vi "Actor Core.vi"(8 "error in":errorcluster, 11 "Inspection Statemachine in":refnum<class "Inspection Statemachine.lvclass">) -> (0 "error out":errorcluster, 3 "Actor out":refnum<class "Actor.lvclass">)   [LabVIEW 2019, in "Inspection Statemachine.lvclass"]
doc: "(<B>Filename</B>: Actor Framework.lvlib:Actor.lvclass:Actor Core.vi)\n\nReceives messages to the actor, reacts to them, and initiates any error handling that may shut the actor down.\n\nDescendant classes may override this VI to append parallel tasks for the actor to complete while it handles messages. Overrides use the Call Parent Method node."
uses:
  Inspection Statemachine.lvclass
  Machine Interface/Machine Interface.lvclass
  <vilib>/ActorFramework/Actor/Actor.lvclass
  Rack Controller/Rack Controller.lvclass
  Inspection Statemachine Messages/ErrorMessage_SM Msg/ErrorMessage_SM Msg.lvclass
  <vilib>/vision/Image Controls.llb/IMAQ Image.ctl
  Inspection Statemachine Messages/ButtonPressed_SM Msg/ButtonPressed_SM Msg.lvclass
  DataLogger/DataLogger/DataLogger.lvclass
  Controls/Result Cluster_SM.ctl
  <vilib>/ActorFramework/Stop Msg/Stop Msg.lvclass
  Common/Controls/Pop-up Input.ctl
  Controls/Output Cluster_SM.ctl
  Common/Controls/Camera Optics Diagnostics Result.ctl
  Common/Controls/AllPartInfo.ctl
  User Interface/User Interface Actor/ZenGage v3.0 UI.lvclass
  Controls/LocalData_SM.ctl
  ZenAnalytics/Zen Analytics/Zen Analytics.lvclass
  <vilib>/event_ctls.llb/usereventprio.ctl
  C:/Program Files/National Instruments/LabVIEW 2019/vi.lib/ActorFramework/Actor/Actor.lvclass
panel:
  in  "Master SamplePass/Fail":bool
  in  "MasterSample/Inspection":bool
  in  "Diagnostics Result":string(combo)
  in  "Software Exit":bool
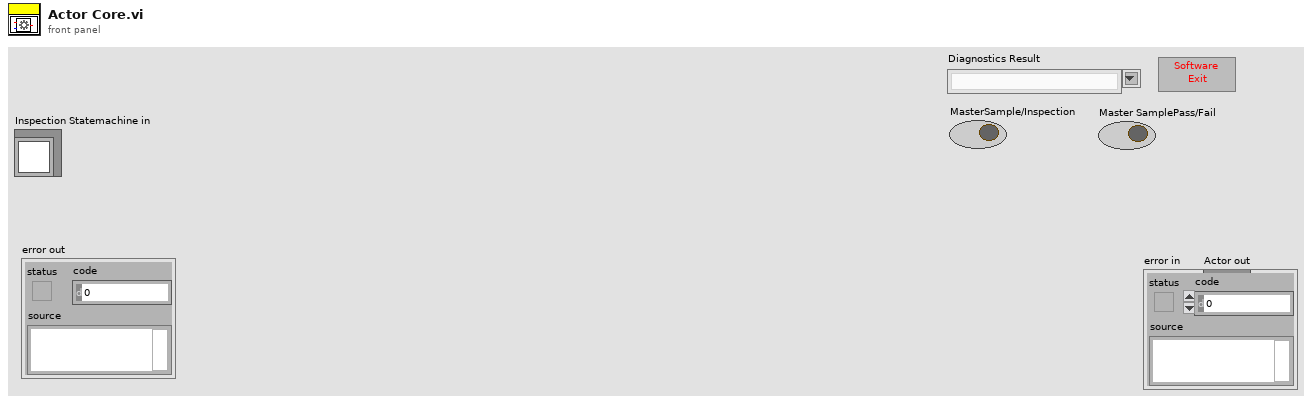
[diagram p1: front panel]
types:
  T1 = typedef "Inspection Statemachine.lvclass/LocalData_SM.ctl" = cluster{"Timeout":i32, "Core":cluster{"Current VI Reference":refnum<vi>, "Close Panel on Exit?":bool}, "Ack":u8, " CurrentState":string, "DirectExit":bool, "SoftwareExit":bool, "SensorDiagnosticsStatus":bool, "OutputCluster":T2, "SelComplete":bool, "ResultToMI":bool, "Exit":bool, "NumberOfActorsLaunched":i32, "BatchStart":bool, "LoadingBarActive":bool, "UpdateInPause":bool, " EventReason":string, "PopUpCategory":string, "PopUpActive":bool, "MasterSampleState":string, "CameraOpticsDiagnosticsStatus":bool, "CameraIndex":i32, "SensorIndex":i32}
  T2 = typedef "Inspection Statemachine.lvclass/Output Cluster_SM.ctl" = cluster{"RackID":u8, "Trigger Light Camera Sequence":cluster{"Light Sequence Trigger":string, "Status":string, "Mode":string}, "Result Cluster":T3, "Analytics VI refnum":refnum<vi>, "Statistical parameters ":string[][], "Sensor Name":string, "Camera Name":string, "PopupInput":T5, "PartInfo":cluster{"PartName":string, "NumberOfRacks":u8, "TotalCount":u64, "ReelCount":u64, "OperatorName":string, "StampingMachineID":u32, "RackID":u8, "Reinitialize":bool, "MeasurementNamesArray":string[], "MeasurementIDArray":u16[], "SpecValuesArray":cluster{"LCL":dbl, "UCL":dbl, "LSL":dbl, "USL":dbl, "Nominal Value":dbl}[], "CameraNamesArray":string[]}, "StateMsgToMI":string, "InspectionStatusToMI":string, "StateMsgToRC":string, "StateMsgToUI":string, "StateMsgToDL":string, "StateMsgToAN":string, "StateMsgToSM":string, "EventData":cluster{"EventName":string, "EventReason":string}, "CameraOpticsDiagnosticsResult":T6, "AllPartInfo":T7, "SystemParameters":cluster{"SystemName":string, "SystemID":string, "CustomerDetails":cluster{"CustomerName":string, "CustomerId":string, "Location":string, "NumberOfShifts":dbl, "ShiftDetails":cluster{"Name":string, "Timing":string}[]}, "InstallationDate":string, "NextServiceDate":string, "NumberOfRacks":u8, "TotalNumberOfCameras":u8, "SoftwareFeatures":cluster{"HardwareEmulated":bool, "PowerOnSelfTest":bool, "DiagnosticsEnable":bool, "AnalyticsEnable":bool, "DefectTrackingEnable":bool, "AutomaticGuideMovement":bool, "DoorPokayokeEnable":bool, "FailCountDisplayEnable":bool, "FailCountReversalEnable":bool, "DataLoggingEnable":bool, "PauseOnReelCountFinish":bool, "StopOnTotalCountFinish":bool, "IoTEnable":bool, "ReportEnable":bool, "DebugLevel":dbl, "PowerOnSelfTestFeatures":cluster{"TimingUnit":bool, "MachinePowerStatusCheck":bool, "GuideMotor":bool, "CameraOptics":bool, "MasterSample":bool}, "DiagnosticsFeatures":cluster{"TimingUnit":bool, "GuideMotor":bool, "CameraOptics":bool, "ReelerMotor":bool, "HardwareButtons":bool, "Sensors":bool, "TowerLamp":bool, "MasterSample":bool}, "UserInterface":cluster{"DynamicImageHandlingEnable":bool, "DoorPokaYokeButtonVisible":bool, "FailCountDisplayButtonVisible":bool, "FailCountReversalButtonVisible":bool}, "PopupOptions":cluster{"ReasonForPause":bool, "ReasonForFail":bool, "ReasonForStop":bool, "CpCpkOnReelFinish":bool}, "DataloggingFeatures":cluster{"EventData":bool, "MeasurementData":bool, "StatisticalData":bool, "ReelData":bool, "FailedMeasurementData":bool, "FailedImages":bool}, "IoT":cluster{"SMSAlertEnable":bool, "EmailAlertEnable":bool}}}, "PartsConfigured":cluster{"Name":string, "NumberOfRack":u8}[], "CameraSequenceList":cluster{"Name":string, "RackID":u8}[], "SensorList":cluster{"Name":string, "RackID":u8}[], "MasterSampleMessages":cluster{"MasterSampleMessage":string, "PartMessage":string}, "SensorDiagnosticsResult":cluster{"Image Array":T4[], "ImageCount":u64}, "IgnoredCountDetails":cluster{"ReelCount":u64, "TotalCount":u64}, "MachineStatusToDL":string, "MasterSamplePartName":string}
  T3 = typedef "Inspection Statemachine.lvclass/Result Cluster_SM.ctl" = cluster{"RackID":u8, "MeasurementValuesArray ":dbl[], "ImagesArray":T4[], "ResultPF":bool, "ProductionCountDetails":cluster{"TotalFail":u64, "TotalPass":u64, "TotalCount":u64}, "ReelCountDetails":cluster{"ReelFail":u64, "ReelPass":u64, "ReelCount":u64}, "ControlPFArray":bool[], "SpecificationPFArray":bool[], "SpecificationFail":bool, "ReelNumber":u64, "Status":string}
  T4 = typedef "IMAQ Image.ctl" = refnum<image>
  T5 = typedef "Pop-up Input.ctl" = cluster{"Pop-up Type":enum16{"Open Logo Display", "Close Logo Display", "Open Loading Bar", "Close Loading Bar", "Open Alert Display", "Close Alert Display", "One button dialog box", "Two button dialog box", "User Authentication"}, "Title":string, "Message":string, "Button 1 Text":string, "Button 2 Text":string, "Show Close? T/F":bool, "Title Blink? T/F":bool, "Title Blink Colour":u32}
  T6 = typedef "Camera Optics Diagnostics Result.ctl" = cluster{"LightCameraName":string, "DiagnosedImage":T4, "DustPercentage":dbl, "Result":bool}
  T7 = typedef "AllPartInfo.ctl" = cluster{"PartName":string, "NumberOfRacks":u8, "MeasurementIDsArray":u16[], "MeasurementNamesArray":string[], "SpecValuesArray":cluster{"LCL":dbl, "UCL":dbl, "LSL":dbl, "USL":dbl, "NominalValue":dbl}[]}[]
  T8 = enum16{"Open Logo Display", "Close Logo Display", "Open Loading Bar", "Close Loading Bar", "Open Alert Display", "Close Alert Display", "One button dialog box", "Two button dialog box", "User Authentication"}
  T9 = enum32{"invalid app kind", "Development System", "Run Time System", "Student Edition", "Embedded LabVIEW", "Evaluation", "Custom"}
  T10 = enum32{"Invalid", "Standard", "Closed", "Hidden", "Minimized", "Maximized"}
  T11 = typedef "usereventprio.ctl" = enum32{"high priority", "normal priority"}
  T12 = cluster{"TotalFail":u64, "TotalPass":u64, "TotalCount":u64}
  T13 = cluster{"ReelFail":u64, "ReelPass":u64, "ReelCount":u64}
  T14 = cluster{"LCL":dbl, "UCL":dbl, "LSL":dbl, "USL":dbl, "NominalValue":dbl}[]
  T15 = cluster{"PartName":string, "NumberOfRacks":u8, "MeasurementIDsArray":u16[], "MeasurementNamesArray":string[], "SpecValuesArray":cluster{"LCL":dbl, "UCL":dbl, "LSL":dbl, "USL":dbl, "NominalValue":dbl}[]}[]
  T16 = cluster{"Current VI Reference":refnum<vi>, "Close Panel on Exit?":bool}
  T17 = cluster{"ZenParamsSpecVersion":string, "SystemParameters":cluster{"SystemName":string, "SystemID":string, "CustomerDetails":cluster{"CustomerName":string, "CustomerId":string, "Location":string, "NumberOfShifts":dbl, "ShiftDetails":cluster{"Name":string, "Timing":string}[]}, "InstallationDate":string, "NextServiceDate":string, "NumberOfRacks":u8, "TotalNumberOfCameras":u8, "SoftwareFeatures":cluster{"HardwareEmulated":bool, "PowerOnSelfTest":bool, "DiagnosticsEnable":bool, "AnalyticsEnable":bool, "DefectTrackingEnable":bool, "AutomaticGuideMovement":bool, "DoorPokayokeEnable":bool, "FailCountDisplayEnable":bool, "FailCountReversalEnable":bool, "DataLoggingEnable":bool, "PauseOnReelCountFinish":bool, "StopOnTotalCountFinish":bool, "IoTEnable":bool, "ReportEnable":bool, "DebugLevel":dbl, "PowerOnSelfTestFeatures":cluster{"TimingUnit":bool, "MachinePowerStatusCheck":bool, "GuideMotor":bool, "CameraOptics":bool, "MasterSample":bool}, "DiagnosticsFeatures":cluster{"TimingUnit":bool, "GuideMotor":bool, "CameraOptics":bool, "ReelerMotor":bool, "HardwareButtons":bool, "Sensors":bool, "TowerLamp":bool, "MasterSample":bool}, "UserInterface":cluster{"DynamicImageHandlingEnable":bool, "DoorPokaYokeButtonVisible":bool, "FailCountDisplayButtonVisible":bool, "FailCountReversalButtonVisible":bool}, "PopupOptions":cluster{"ReasonForPause":bool, "ReasonForFail":bool, "ReasonForStop":bool, "CpCpkOnReelFinish":bool}, "DataloggingFeatures":cluster{"EventData":bool, "MeasurementData":bool, "StatisticalData":bool, "ReelData":bool, "FailedMeasurementData":bool, "FailedImages":bool}, "IoT":cluster{"SMSAlertEnable":bool, "EmailAlertEnable":bool}}}, "PartsConfigured":cluster{"Name":string, "NumberOfRack":u8}[], "CameraSequenceList":cluster{"Name":string, "RackID":u8}[], "SensorList":cluster{"Name":string, "RackID":u8}[]}
  T18 = cluster{"SystemName":string, "SystemID":string, "CustomerDetails":cluster{"CustomerName":string, "CustomerId":string, "Location":string, "NumberOfShifts":dbl, "ShiftDetails":cluster{"Name":string, "Timing":string}[]}, "InstallationDate":string, "NextServiceDate":string, "NumberOfRacks":u8, "TotalNumberOfCameras":u8, "SoftwareFeatures":cluster{"HardwareEmulated":bool, "PowerOnSelfTest":bool, "DiagnosticsEnable":bool, "AnalyticsEnable":bool, "DefectTrackingEnable":bool, "AutomaticGuideMovement":bool, "DoorPokayokeEnable":bool, "FailCountDisplayEnable":bool, "FailCountReversalEnable":bool, "DataLoggingEnable":bool, "PauseOnReelCountFinish":bool, "StopOnTotalCountFinish":bool, "IoTEnable":bool, "ReportEnable":bool, "DebugLevel":dbl, "PowerOnSelfTestFeatures":cluster{"TimingUnit":bool, "MachinePowerStatusCheck":bool, "GuideMotor":bool, "CameraOptics":bool, "MasterSample":bool}, "DiagnosticsFeatures":cluster{"TimingUnit":bool, "GuideMotor":bool, "CameraOptics":bool, "ReelerMotor":bool, "HardwareButtons":bool, "Sensors":bool, "TowerLamp":bool, "MasterSample":bool}, "UserInterface":cluster{"DynamicImageHandlingEnable":bool, "DoorPokaYokeButtonVisible":bool, "FailCountDisplayButtonVisible":bool, "FailCountReversalButtonVisible":bool}, "PopupOptions":cluster{"ReasonForPause":bool, "ReasonForFail":bool, "ReasonForStop":bool, "CpCpkOnReelFinish":bool}, "DataloggingFeatures":cluster{"EventData":bool, "MeasurementData":bool, "StatisticalData":bool, "ReelData":bool, "FailedMeasurementData":bool, "FailedImages":bool}, "IoT":cluster{"SMSAlertEnable":bool, "EmailAlertEnable":bool}}}
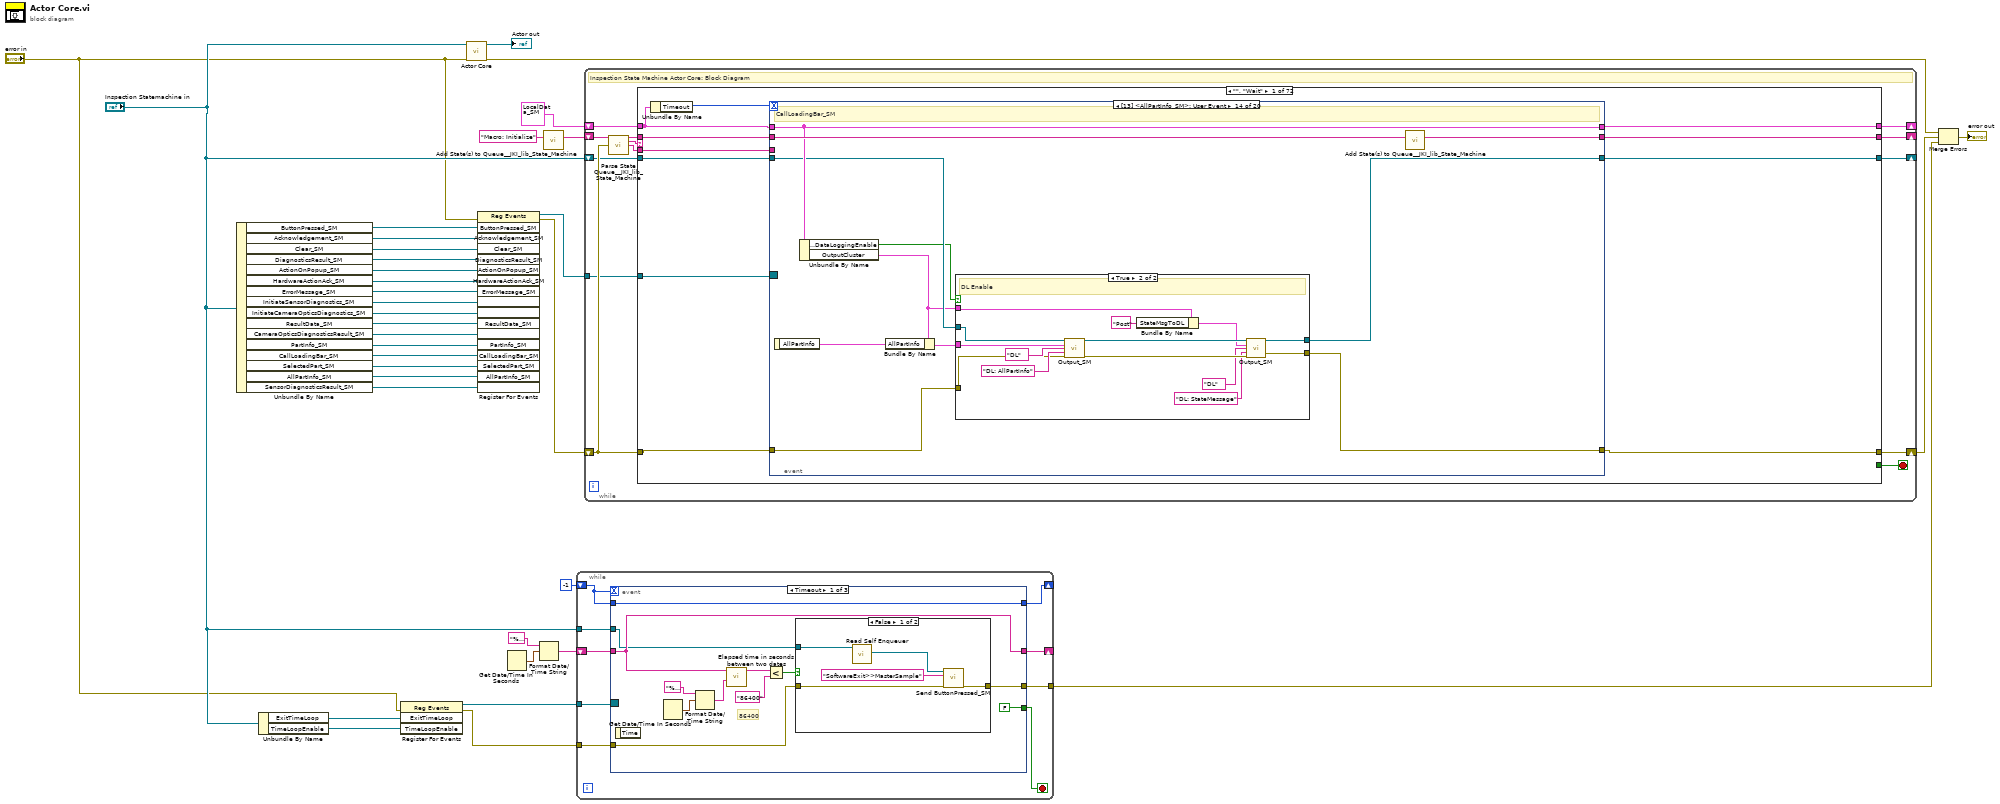
[diagram p0: block diagram]
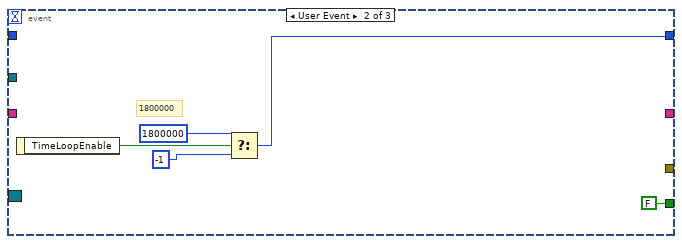
[diagram p3: hidden frame]
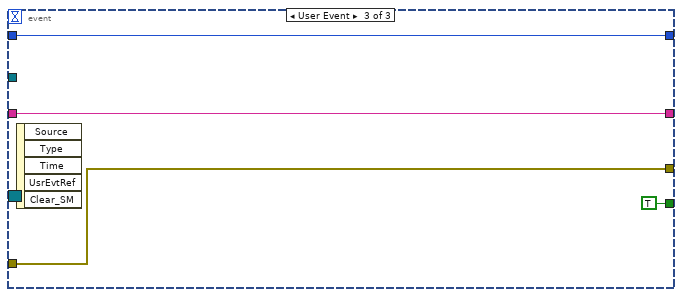
[diagram p4: hidden frame]
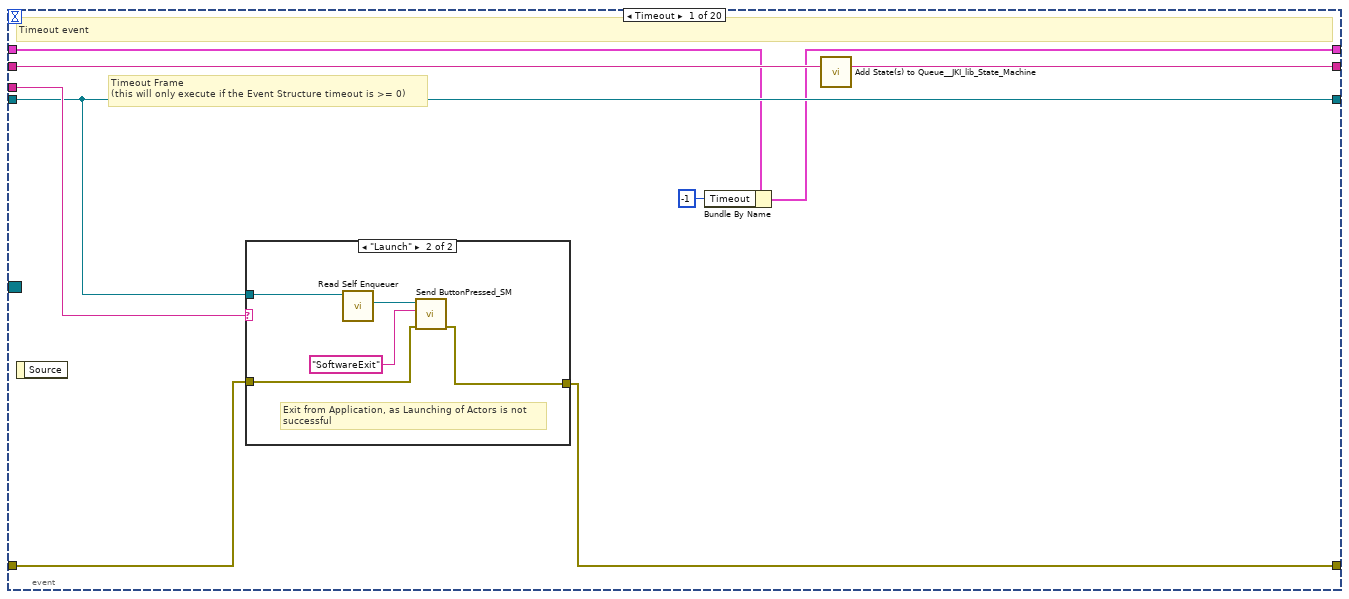
[diagram p5: hidden frame]
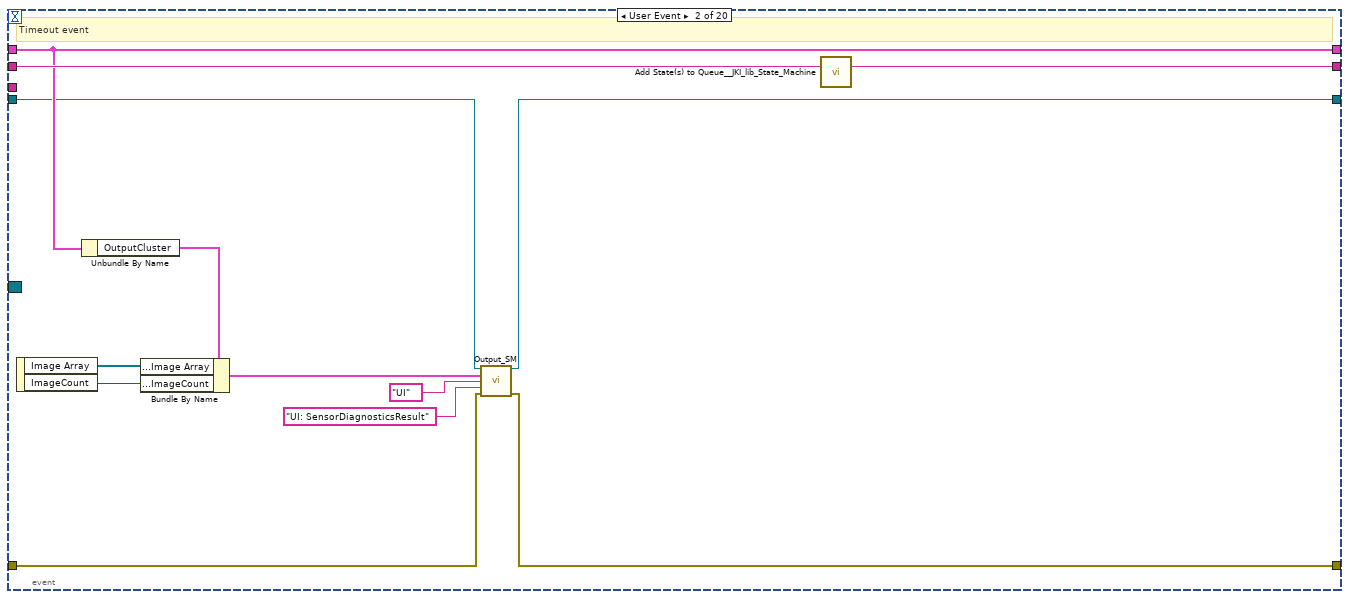
[diagram p7: hidden frame]
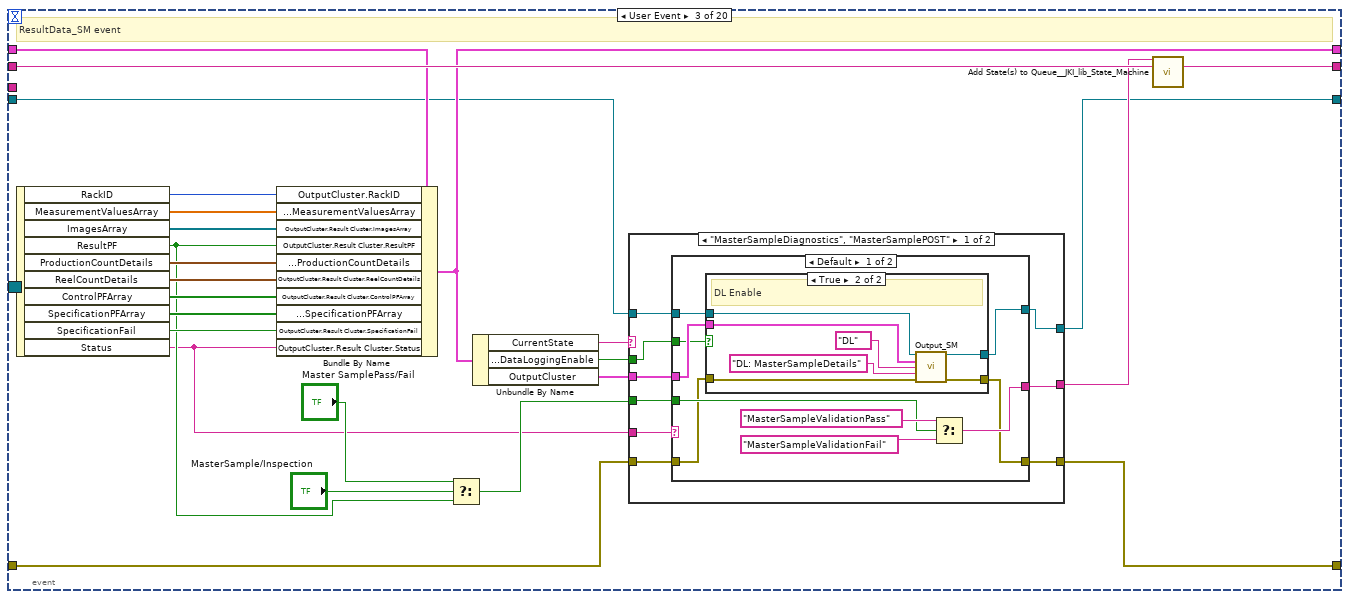
[diagram p8: hidden frame]
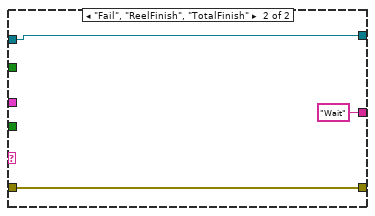
[diagram p10: hidden frame]
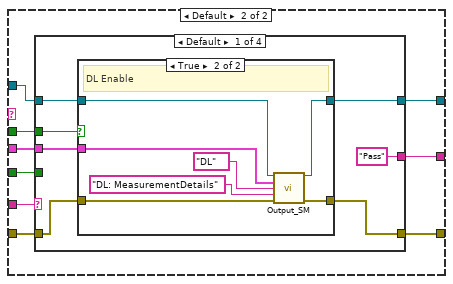
[diagram p11: hidden frame]
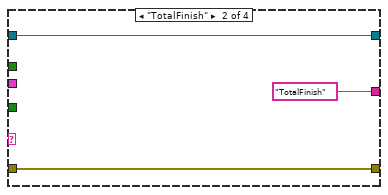
[diagram p13: hidden frame]
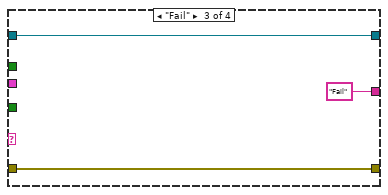
[diagram p14: hidden frame]
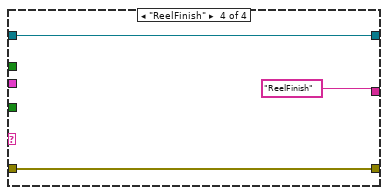
[diagram p15: hidden frame]
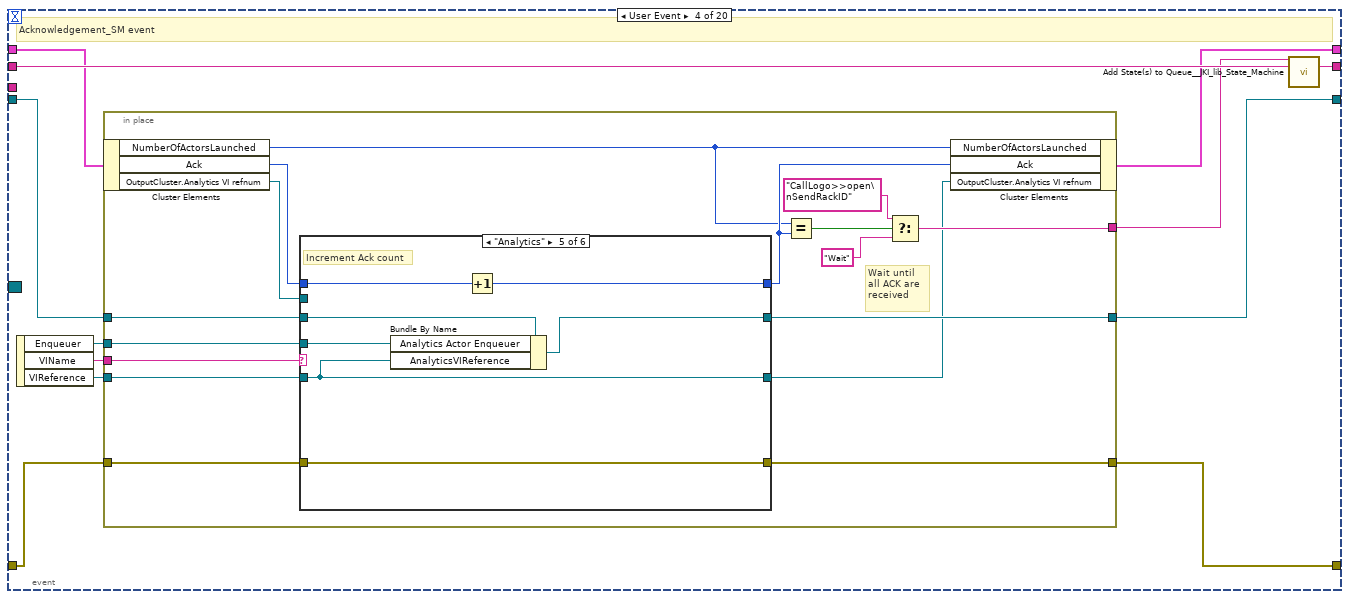
[diagram p16: hidden frame]
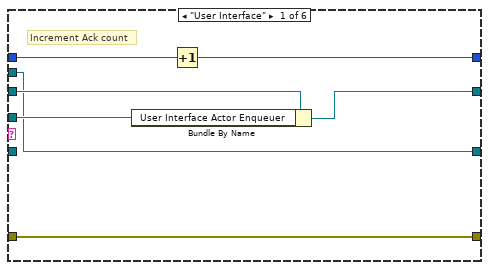
[diagram p17: hidden frame]
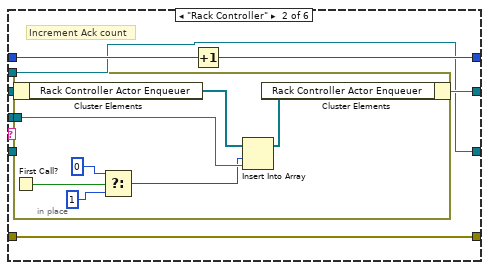
[diagram p18: hidden frame]
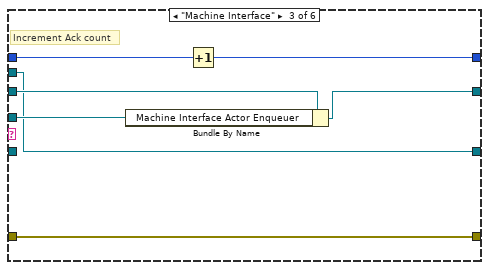
[diagram p19: hidden frame]
diagram:
  n1 = Unbundle By Name("Inspection Statemachine in") -> ("ButtonPressed_SM"=w24:refnum<user-event>, "Acknowledgement_SM"=w25:refnum<user-event>, "Clear_SM"=w26:refnum<user-event>, "DiagnosticsResult_SM"=w27:refnum<user-event>, "ActionOnPopup_SM"=w28:refnum<user-event>, "HardwareActionAck_SM"=w29:refnum<user-event>, "ErrorMessage_SM"=w23:refnum<user-event>, "InitiateSensorDiagnostics_SM"=w22:refnum<user-event>, "InitiateCameraOpticsDiagnostics_SM"=w21:refnum<user-event>, "ResultData_SM"=w20:refnum<user-event>, "CameraOpticsDiagnosticsResult_SM"=w19:refnum<user-event>, "PartInfo_SM"=w18:refnum<user-event>, "CallLoadingBar_SM"=w17:refnum<user-event>, "SelectedPart_SM"=w16:refnum<user-event>, "AllPartInfo_SM"=w14:refnum<user-event>, "SensorDiagnosticsResult_SM"=w12:refnum<user-event>)
  n2 = Unbundle By Name("Inspection Statemachine in") -> ("ExitTimeLoop"=w7:refnum<user-event>, "TimeLoopEnable"=w2:refnum<user-event>)
  n3 = register-events(error in="error in", w7, w2) -> (reference out=w6:refnum<event-registration>, error out=w3:errorcluster)  [unwired: 1 in]
  n4 = call-parent "Actor Core.vi"("error in"="error in", "Actor in"="Inspection Statemachine in") -> ("error out"=w32:errorcluster, "Actor out"=→"Actor out":refnum<class "Actor.lvclass">)  [unwired: 8 in]
  n5 = register-events(error in="error in", w24, w25, w26, w27, w28, w29, w23, w22, w21, w20, w19, w18, w17, w16, w14, w12) -> (reference out=w15:refnum<event-registration>, error out=w30:errorcluster)  [unwired: 1 in]
  n6 = Get Date/Time In Seconds() -> (seconds since 1Jan1904=w11:timestamp)
  n7 = Format Date/Time String(time format string (%c)="%d-%b-%Y %H:%M:%S", seconds (now)=w11) -> (date/time string=w9:string)  [unwired: 1 in]
  n8 = call <vilib>:"Add State(s) to Queue__JKI_lib_State_Machine.vi"("State(s) in (\"\")"="Macro: Initialize") -> ("States Out"=w35:string)  [unwired: 14 in]
  n9 = while {
    shift-right: [w44] -> _
    shift-left: w9 -> [w45]
    shift-right: [w38] -> _
    shift-left: -1 ("milliseconds to wait") -> [w37]
    tunnel: "Inspection Statemachine in" -> [w43]
    tunnel: w3 -> [w42]
    tunnel: [w41] -> w8
    tunnel: w6 -> [w39]
    stop <- w40 stop-if-true
    n10 = event shown="[0] Timeout" {
      selector: w39 -> [_ _ _]
      dyn-events: _ -> [_ _ _]
      timeout: w37 -> [_ _ _]
      tunnel: w45 -> [w57 _ w72]
      tunnel: [w57 _ w72] -> w44
      tunnel: w43 -> [w50 _ _]
      tunnel: w42 -> [w49 _ w70]
      tunnel: [w48 _ w70] -> w41
      tunnel: [FALSE FALSE TRUE] -> w40
      tunnel: [w46 w66 w69] -> w38
      tunnel: w37 -> [w46 _ w69]
      event Timeout {
        # "86400"
        n11 = event-data() -> ()  [unwired: 1 in, 1 out]
        n12 = Get Date/Time In Seconds() -> (seconds since 1Jan1904=w55:timestamp)
        n13 = Format Date/Time String(time format string (%c)="%d-%b-%Y %H:%M:%S", seconds (now)=w55) -> (date/time string=w54:string)  [unwired: 1 in]
        n14 = call "Elapsed time in seconds between two dates.vi"("Start Date/Time"=w57, "End Date/Time"=w54) -> ("Time difference in Seconds"=w53:string)  [unwired: 8 in]
        n15 = Less?(x=w53, y="86400") -> (x < y?=w51:bool)
        n16 = case shown="False" w51 {
          tunnel: w50 -> [w62 _]
          tunnel: w49 -> [w59 w63]
          tunnel: [w58 w63] -> w48
          frame False {
            n17 = call <vilib>:"Read Self Enqueuer.vi"("Actor"=w62) -> ("Self Enqueuer"=w61:refnum<class "Message Enqueuer.lvclass">)  [unwired: 10 in]
            n18 = call "Send ButtonPressed_SM.vi"("error in (no error)"=w59, "ButtonPress"="SoftwareExit>>MasterSample", "Message Enqueuer"=w61) -> ("error out"=w58:errorcluster)  [unwired: 7 in, 1 out]
          }
          frame True {
          }
        }
      }
      event User Event {
        # "1800000"
        n19 = event-data() -> ("TimeLoopEnable"=w68:bool)  [unwired: 1 in]
        n20 = Select(t=1800000 ("milliseconds to wait"), s=w68, f=-1) -> (s? t:f=w66:i32)
      }
      event User Event {
        n21 = event-data() -> ()  [unwired: 1 in, 5 out]
      }
    }
  }
  n22 = while "JKI - String-Based Queued State Machine (Basic) v1.0" {
    shift-right: [w78] -> _
    shift-left: T1 {"Timeout"=0, "Core"={"Current VI Reference"=refnum, "Close Panel on Exit?"=FALSE}, "Ack"=0, " CurrentState"="", "DirectExit"=FALSE, "SoftwareExit"=FALSE, "SensorDiagnosticsStatus"=FALSE, "OutputCluster"={"RackID"=0, "Trigger Light Camera Sequence"={"Light Sequence Trigger"="", "Status"="", "Mode"=""}, "Result Cluster"={"RackID"=0, "MeasurementValuesArray "=[], "ImagesArray"=[], "ResultPF"=FALSE, "ProductionCountDetails"={"TotalFail"=0, "TotalPass"=0, "TotalCount"=0}, "ReelCountDetails"={"ReelFail"=0, "ReelPass"=0, "ReelCount"=0}, "ControlPFArray"=[], "SpecificationPFArray"=[], "SpecificationFail"=FALSE, "ReelNumber"=0, "Status"=""}, "Analytics VI refnum"=refnum, "Statistical parameters "=[], "Sensor Name"="", "Camera Name"="", "PopupInput"={"Pop-up Type"=enum."Open Logo Display", "Title"="", "Message"="", "Button 1 Text"="", "Button 2 Text"="", "Show Close? T/F"=FALSE, "Title Blink? T/F"=FALSE, "Title Blink Colour"=0}, "PartInfo"={"PartName"="", "NumberOfRacks"=0, "TotalCount"=0, "ReelCount"=0, "OperatorName"="", "StampingMachineID"=0, "RackID"=0, "Reinitialize"=FALSE, "MeasurementNamesArray"=[], "MeasurementIDArray"=[], "SpecValuesArray"=[], "CameraNamesArray"=[]}, "StateMsgToMI"="", "InspectionStatusToMI"="", "StateMsgToRC"="", "StateMsgToUI"="", "StateMsgToDL"="", "StateMsgToAN"="", "StateMsgToSM"="", "EventData"={"EventName"="", "EventReason"=""}, "CameraOpticsDiagnosticsResult"={"LightCameraName"="", "DiagnosedImage"=refnum, "DustPercentage"=0.0, "Result"=FALSE}, "AllPartInfo"=[], "SystemParameters"={"SystemName"="", "SystemID"="", "CustomerDetails"={"CustomerName"="", "CustomerId"="", "Location"="", "NumberOfShifts"=0.0, "ShiftDetails"=[]}, "InstallationDate"="", "NextServiceDate"="", "NumberOfRacks"=0, "TotalNumberOfCameras"=0, "SoftwareFeatures"={"HardwareEmulated"=FALSE, "PowerOnSelfTest"=FALSE, "DiagnosticsEnable"=FALSE, "AnalyticsEnable"=FALSE, "DefectTrackingEnable"=FALSE, "AutomaticGuideMovement"=FALSE, "DoorPokayokeEnable"=FALSE, "FailCountDisplayEnable"=FALSE, "FailCountReversalEnable"=FALSE, "DataLoggingEnable"=FALSE, "PauseOnReelCountFinish"=FALSE, "StopOnTotalCountFinish"=FALSE, "IoTEnable"=FALSE, "ReportEnable"=FALSE, "DebugLevel"=0.0, "PowerOnSelfTestFeatures"={"TimingUnit"=FALSE, "MachinePowerStatusCheck"=FALSE, "GuideMotor"=FALSE, "CameraOptics"=FALSE, "MasterSample"=FALSE}, "DiagnosticsFeatures"={"TimingUnit"=FALSE, "GuideMotor"=FALSE, "CameraOptics"=FALSE, "ReelerMotor"=FALSE, "HardwareButtons"=FALSE, "Sensors"=FALSE, "TowerLamp"=FALSE, "MasterSample"=FALSE}, "UserInterface"={"DynamicImageHandlingEnable"=FALSE, "DoorPokaYokeButtonVisible"=FALSE, "FailCountDisplayButtonVisible"=FALSE, "FailCountReversalButtonVisible"=FALSE}, "PopupOptions"={"ReasonForPause"=FALSE, "ReasonForFail"=FALSE, "ReasonForStop"=FALSE, "CpCpkOnReelFinish"=FALSE}, "DataloggingFeatures"={"EventData"=FALSE, "MeasurementData"=FALSE, "StatisticalData"=FALSE, "ReelData"=FALSE, "FailedMeasurementData"=FALSE, "FailedImages"=FALSE}, "IoT"={"SMSAlertEnable"=FALSE, "EmailAlertEnable"=FALSE}}}, "PartsConfigured"=[], "CameraSequenceList"=[], "SensorList"=[], "MasterSampleMessages"={"MasterSampleMessage"="", "PartMessage"=""}, "SensorDiagnosticsResult"={"Image Array"=[], "ImageCount"=0}, "IgnoredCountDetails"={"ReelCount"=0, "TotalCount"=0}, "MachineStatusToDL"="", "MasterSamplePartName"=""}, "SelComplete"=FALSE, "ResultToMI"=FALSE, "Exit"=FALSE, "NumberOfActorsLaunched"=0, "BatchStart"=FALSE, "LoadingBarActive"=FALSE, "UpdateInPause"=FALSE, " EventReason"="", "PopUpCategory"="", "PopUpActive"=FALSE, "MasterSampleState"="", "CameraOpticsDiagnosticsStatus"=FALSE, "CameraIndex"=0, "SensorIndex"=0} ("LocalData_SM") -> [w77]
    shift-right: [w81] -> w31
    shift-left: w30 -> [w76]
    shift-right: [w80] -> _
    shift-left: w35 -> [w82]
    tunnel: w15 -> [w75]
    shift-right: [w73] -> _
    shift-left: "Inspection Statemachine in" -> [w74]
    stop <- w79 stop-if-true
    # "Inspection State Machine Actor Core: Block Diagram"
    n23 = call <vilib>:"Parse State Queue__JKI_lib_State_Machine.vi"("State Queue"=w82, "Error In (no error)"=w76) -> ("Remaining States"=w84:string, "Current State"=w85:string, "Arguments"=w83:string)  [unwired: 11 in]
    n24 = case shown="\"\", \"Wait\"" w85 {
      selector: w85 -> [_ _ w1573 _ _ _ _ _ _ _ _ _ _ _ _ _ _ _ _ _ _ _ _ _ _ _ _ _ _ _ _ _ _ _ _ _ _ _ _ _ _ _ _ _ _ _ _ _ _ _ _ _ _ _ _ _ _ _ _ _ _ _ w4330 _ _ _ _ _ _ _ _ _]
      tunnel: w84 -> [w96 w1571 w1577 w1596 w1611 w1617 w1622 w1663 w1673 w1678 w1683 w1691 w1718 w1724 w1735 w1740 w1751 w1829 w1858 w1889 w1895 w1907 w1930 w1960 w1997 w2124 w2197 w2257 w2276 w2354 w2376 w2440 w2482 w2595 w2636 w2665 w2726 w2787 w2847 w2861 w2902 w2939 w3000 w3029 w3065 w3198 w3206 w3290 w3314 w3352 w3447 w3488 _ w3609 w3646 w3730 w3800 w3820 w4089 w4156 w4240 w4308 w4335 w4392 w4403 w4544 w4604 w4636 w4651 w4795 w4820 w5074]
      tunnel: w83 -> [w89 _ _ _ _ _ _ _ _ _ _ w1685 _ _ _ _ _ _ _ w1881 _ _ _ _ w1995 _ _ _ _ _ _ _ _ _ _ _ _ _ _ _ _ _ _ _ _ _ _ _ _ _ _ _ _ _ _ _ _ _ _ _ _ _ _ _ _ _ _ _ _ _ w4796 _]
      tunnel: w77 -> [w87 w1568 w1575 w1587 w1599 w1615 w1619 _ w1669 w1675 w1681 w1687 w1715 w1721 w1732 w1737 w1742 w1821 w1854 w1880 w1892 w1899 w1926 w1957 w1988 w2119 w2193 w2253 w2273 w2346 w2371 w2438 w2474 w2577 w2630 w2662 w2723 w2784 w2844 w2855 w2890 w2938 w2999 w3018 w3050 w3195 w3202 w3284 w3310 w3349 w3445 w3490 w3497 w3607 w3644 w3729 w3797 w3806 w4086 w4155 w4239 w4301 w4334 w4389 w4401 w4535 w4599 w4629 w4645 w4792 w4806 w5072]
      tunnel: [w88 w1569 w1579 w1593 errorcluster {"status"=FALSE, "code"=0, "source"=""} ("error out") w1614 w1620 w1655 w1670 w1676 w1680 w1688 w1716 w1722 w1733 w1738 w1747 w1811 w1846 w1888 w1893 w1904 w1927 w1954 w1992 w2122 w2195 w2255 w2275 w2347 w2372 w2429 w2471 w2586 w2631 w2664 w2725 w2786 w2845 w2851 w2900 w2935 w2998 w3022 w3052 w3196 w3203 w3286 w3311 w3350 w3441 w3486 w3499 w3605 w3640 w3724 w3798 w3816 w4087 w4151 w4234 w4306 w4331 w4390 w4397 w4539 w4600 w4631 w4642 w4793 w4803 w5058] -> w81
      tunnel: w76 -> [w94 w1569 w1578 w1593 w1606 w1614 w1620 w1659 w1667 w1676 w1680 w1689 w1716 w1722 w1733 w1738 w1748 w1827 w1853 w1878 w1893 w1905 w1928 w1955 w1993 w2120 w2194 w2254 w2274 w2344 w2361 w2424 w2469 w2587 w2635 w2663 w2724 w2785 w2845 w2858 w2898 w2936 w2997 w3026 w3059 w3196 w3204 w3289 w3313 w3351 w3449 w3486 w3500 w3601 w3648 w3727 w3798 w3801 w4088 w4152 w4237 w4307 w4332 w4390 w4396 w4540 w4601 w4630 w4643 w4793 w4804 w5071]
      tunnel: [w95 w1570 w1576 w1595 w1610 w1616 w1621 w1662 w1672 w1677 w1682 w1690 w1717 w1723 w1734 w1739 w1750 w1828 w1857 w1890 w1894 w1906 w1929 w1959 w1996 w2123 w2196 w2258 w2278 w2353 w2378 w2441 w2481 w2594 w2638 w2667 w2728 w2789 w2846 w2862 w2903 w2940 w3002 w3030 w3066 w3197 w3207 w3291 w3315 w3353 w3450 w3489 w3503 w3610 w3649 w3731 w3799 w3821 w4091 w4158 w4241 w4309 w4336 w4391 w4405 w4545 w4605 w4638 w4652 w4794 w4819 w5075] -> w80
      tunnel: [_ _ _ _ _ TRUE _ _ _ _ _ _ _ _ _ _ _ _ _ _ _ _ _ _ _ _ _ _ _ _ _ _ _ _ _ _ _ _ _ _ _ _ _ _ _ _ _ _ _ _ _ _ _ _ _ _ _ _ _ _ _ _ _ _ _ _ _ _ _ _ _ _] -> w79
      tunnel: [w93 w1568 w1575 w1594 w1598 w1615 w1619 w1661 w1669 w1675 w1681 w1687 w1715 w1721 w1732 w1737 w1741 w1822 w1854 w1880 w1892 w1898 w1926 w1957 w1987 w2118 w2192 w2253 w2272 w2349 w2369 w2427 w2473 w2590 w2621 w2661 w2722 w2783 w2844 w2860 w2896 w2938 w2999 w3019 w3049 w3195 w3201 w3284 w3310 w3348 w3434 w3490 w3496 w3607 w3632 w3718 w3797 w3807 w4085 w4150 w4229 w4300 w4334 w4389 w4400 w4534 w4599 w4629 w4644 w4792 w4805 w5072] -> w78
      tunnel: w75 -> [w92 _ _ _ _ _ _ _ w1668 _ _ _ _ _ _ _ _ _ _ _ _ _ _ _ _ _ _ _ _ _ _ _ _ _ _ _ _ _ _ _ _ _ _ _ _ _ _ _ _ _ _ _ _ _ _ _ _ w3814 _ _ _ _ _ _ _ _ _ _ _ _ w4818 _]
      tunnel: w74 -> [w91 w1567 w1572 w1584 w1609 w1612 w1618 w1658 w1665 w1674 w1679 w1684 w1714 w1719 w1725 w1736 w1749 w1816 w1849 w1877 w1891 w1897 w1922 w1953 w1990 w2117 w2191 w2251 w2271 w2345 w2363 w2423 w2468 w2585 w2633 w2660 w2721 w2782 w2843 w2856 w2892 w2931 w2994 w3015 w3058 w3194 w3200 w3283 w3306 w3347 w3436 w3487 w3494 w3602 w3635 w3722 w3796 w3802 w4084 w4154 w4232 w4303 w4329 w4388 w4394 w4538 w4598 w4627 w4641 w4791 w4799 w5056]
      tunnel: [w90 w1567 w1572 w1584 w1609 w1612 w1618 w1658 w1665 w1674 w1679 w1684 w1714 w1719 w1725 w1736 w1746 w1812 w1844 w1884 w1891 w1896 w1921 w1952 w1989 w2116 w2190 w2250 w2270 w2345 w2373 w2428 w2472 w2584 w2632 w2659 w2720 w2781 w2843 w2853 w2891 w2930 w2993 w3016 w3051 w3194 w3199 w3282 w3305 w3346 w3435 w3487 w3495 w3606 w3634 w3721 w3796 w3813 w4083 w4153 w4231 w4302 w4328 w4388 w4393 w4537 w4597 w4626 w4640 w4791 w4802 w5056] -> w73
      frame "", "Wait" {
        n25 = Unbundle By Name(w87) -> ("Timeout"=w86:i32)
        n26 = event shown="[13] <AllPartInfo_SM>: User Event" {
          selector: w92 -> [_ _ _ _ _ _ _ _ _ _ _ _ _ _ _ w1431 _ _ _ _]
          dyn-events: _ -> [_ _ _ _ _ _ _ _ _ _ _ _ _ _ _ _ _ _ _ _]
          timeout: w86 -> [_ _ _ _ _ _ _ _ _ _ _ _ _ _ _ _ _ _ _ _]
          tunnel: w96 -> [w105 w124 w149 w222 w297 w322 w642 w909 w923 w1203 w1326 w1344 w1388 w1399 w1427 w1444 w1450 w1466 w1558 w1566]
          tunnel: [w104 w123 w148 w223 w298 w323 w643 w908 w924 w1204 w1327 w1345 w1389 w1400 w1428 w1445 w1449 w1465 w1557 w1565] -> w95
          tunnel: w87 -> [w99 w116 w147 w215 w293 w318 w638 w904 w915 w1201 w1313 w1335 w1387 w1398 w1419 w1442 w1451 w1461 w1559 w1564]
          tunnel: w94 -> [w102 w120 w136 w226 w295 w321 w641 w906 w922 w1200 w1324 w1337 w1374 w1397 w1420 w1433 w1446 w1459 w1554 w1560]
          tunnel: [w98 w116 w138 w216 w293 w319 w639 w903 w921 w1201 w1316 w1342 w1387 w1398 w1418 w1441 w1451 w1462 w1559 w1564] -> w93
          tunnel: w91 -> [w101 w115 w132 w225 w290 w314 w634 w907 w913 w1196 w1325 w1339 w1372 w1394 w1421 w1443 w1448 w1456 w1556 w1561]
          tunnel: [w101 w114 w131 w224 w289 w312 w628 w907 w912 w1195 w1325 w1338 w1371 w1393 w1421 w1443 w1448 w1455 w1556 w1561] -> w90
          tunnel: w89 -> [w103 _ _ _ _ _ _ _ _ _ _ _ _ _ _ _ _ _ _ _]
          tunnel: [w100 w119 w135 w221 w294 w313 w627 w906 w917 w1199 w1324 w1336 w1373 w1391 w1420 w1432 w1446 w1458 w1554 w1560] -> w88
          event Timeout {
            # "Timeout Frame\n(this will only execute if the Event Structure timeout is >= 0)"
            # "Timeout event"
            n27 = event-data() -> ()  [unwired: 1 in, 1 out]
            n28 = case shown="\"Launch\"" w103 {
              tunnel: w102 -> [w106 w109]
              tunnel: [w106 w108] -> w100
              tunnel: w101 -> [_ w107]
              frame Default {
              }
              frame "Launch" {
                # "Exit from Application, as Launching of Actors is not\nsuccessful"
                n29 = call <vilib>:"Read Self Enqueuer.vi"("Actor"=w107) -> ("Self Enqueuer"=w111:refnum<class "Message Enqueuer.lvclass">)  [unwired: 10 in]
                n30 = call "Send ButtonPressed_SM.vi"("error in (no error)"=w109, "ButtonPress"="SoftwareExit" ("Button Press"), "Message Enqueuer"=w111) -> ("error out"=w108:errorcluster)  [unwired: 7 in, 1 out]
              }
            }
            n31 = Bundle By Name(cluster=w99, "Timeout"=-1) -> (w98:T1)
            n32 = call <vilib>:"Add State(s) to Queue__JKI_lib_State_Machine.vi"("State(s) in (\"\")"=w105) -> ("States Out"=w104:string)  [unwired: 14 in]
          }
          event User Event {
            # "Timeout event"
            n33 = event-data() -> ("Image Array"=w122:T4[], "ImageCount"=w121:u64)  [unwired: 1 in]
            n34 = Unbundle By Name(w116) -> ("OutputCluster"=w118:T2)
            n35 = Bundle By Name(cluster=w118, "SensorDiagnosticsResult.Image Array"=w122, "SensorDiagnosticsResult.ImageCount"=w121) -> (w117:T2)
            n36 = call "Output_SM.vi"("SM Private Data in"=w115, "Output Cluster"=w117, "Receiver Name"="UI", "State"="UI: SensorDiagnosticsResult", "error in (no error)"=w120) -> ("SM Private Data out"=w114:refnum<class "Inspection Statemachine.lvclass">, "error out"=w119:errorcluster)  [unwired: 9 in]
            n37 = call <vilib>:"Add State(s) to Queue__JKI_lib_State_Machine.vi"("State(s) in (\"\")"=w124) -> ("States Out"=w123:string)  [unwired: 14 in]
          }
          event User Event {
            # "ResultData_SM event"
            n38 = event-data() -> ("RackID"=w145:u8, "MeasurementValuesArray"=w144:dbl[], "ImagesArray"=w143:T4[], "ResultPF"=w128:bool, "ProductionCountDetails"=w142:T12, "ReelCountDetails"=w141:T13, "ControlPFArray"=w140:bool[], "SpecificationPFArray"=w130:bool[], "SpecificationFail"=w139:bool, "Status"=w125:string)  [unwired: 1 in]
            n39 = Bundle By Name(cluster=w147, "OutputCluster.RackID"=w145, "OutputCluster.Result Cluster.MeasurementValuesArray"=w144, "OutputCluster.Result Cluster.ImagesArray"=w143, "OutputCluster.Result Cluster.ResultPF"=w128, "OutputCluster.Result Cluster.ProductionCountDetails"=w142, "OutputCluster.Result Cluster.ReelCountDetails"=w141, "OutputCluster.Result Cluster.ControlPFArray"=w140, "OutputCluster.Result Cluster.SpecificationPFArray"=w130, "OutputCluster.Result Cluster.SpecificationFail"=w139, "OutputCluster.Result Cluster.Status"=w125) -> (w138:T1)
            n40 = Select(t="Master SamplePass/Fail", s="MasterSample/Inspection", f=w128) -> (s? t:f=w127:bool)
            n41 = Unbundle By Name(w138) -> ("CurrentState"=w137:string, "OutputCluster.SystemParameters.SoftwareFeatures.DataLoggingEnable"=w134:bool, "OutputCluster"=w133:T2)
            n42 = case shown="\"MasterSampleDiagnostics\", \"MasterSamplePOST\"" w137 {
              tunnel: [w158 w189] -> w146
              tunnel: w125 -> [w156 w188]
              tunnel: w127 -> [w157 w187]
              tunnel: w136 -> [w155 w186]
              tunnel: [w154 w185] -> w135
              tunnel: w132 -> [w153 w184]
              tunnel: w134 -> [w150 w183]
              tunnel: w133 -> [w151 w182]
              tunnel: [w152 w181] -> w131
              frame "MasterSampleDiagnostics", "MasterSamplePOST" {
                n43 = case shown="Default" w156 {
                  tunnel: [w166 "Wait"] -> w158
                  tunnel: w157 -> [w165 _]
                  tunnel: w155 -> [w161 w179]
                  tunnel: [w160 w179] -> w154
                  tunnel: w153 -> [w164 w178]
                  tunnel: [w163 w178] -> w152
                  tunnel: w151 -> [w162 _]
                  tunnel: w150 -> [w159 _]
                  frame Default {
                    n44 = case shown="True" w159 {
                      tunnel: w164 -> [w170 w175]
                      tunnel: [w170 w174] -> w163
                      tunnel: w162 -> [_ w173]
                      tunnel: w161 -> [w169 w172]
                      tunnel: [w169 w171] -> w160
                      frame False {
                        # "DL Disable"
                      }
                      frame True {
                        # "DL Enable"
                        n45 = call "Output_SM.vi"("SM Private Data in"=w175, "Output Cluster"=w173, "Receiver Name"="DL", "State"="DL: MasterSampleDetails", "error in (no error)"=w172) -> ("SM Private Data out"=w174:refnum<class "Inspection Statemachine.lvclass">, "error out"=w171:errorcluster)  [unwired: 9 in]
                      }
                    }
                    n46 = Select(t="MasterSampleValidationPass", s=w165, f="MasterSampleValidationFail") -> (s? t:f=w166:string)
                  }
                  frame "Fail", "ReelFinish", "TotalFinish" {
                  }
                }
              }
              frame Default {
                n47 = case shown="Default" w188 {
                  tunnel: ["Pass" "TotalFinish" "Fail" "ReelFinish"] -> w189
                  tunnel: w187 -> [_ _ _ _]
                  tunnel: w186 -> [w195 w207 w210 w213]
                  tunnel: [w194 w207 w210 w213] -> w185
                  tunnel: w184 -> [w193 w206 w209 w212]
                  tunnel: w183 -> [w192 _ _ _]
                  tunnel: w182 -> [w191 _ _ _]
                  tunnel: [w190 w206 w209 w212] -> w181
                  frame Default {
                    n48 = case shown="True" w192 {
                      tunnel: w195 -> [w198 w205]
                      tunnel: [w198 w204] -> w194
                      tunnel: w193 -> [w197 w203]
                      tunnel: w191 -> [_ w200]
                      tunnel: [w197 w199] -> w190
                      frame False {
                        # "DL Disable"
                      }
                      frame True {
                        # "DL Enable"
                        n49 = call "Output_SM.vi"("SM Private Data in"=w203, "Output Cluster"=w200, "Receiver Name"="DL", "State"="DL: MeasurementDetails", "error in (no error)"=w205) -> ("SM Private Data out"=w199:refnum<class "Inspection Statemachine.lvclass">, "error out"=w204:errorcluster)  [unwired: 9 in]
                      }
                    }
                  }
                  frame "TotalFinish" {
                  }
                  frame "Fail" {
                  }
                  frame "ReelFinish" {
                  }
                }
              }
            }
            n50 = call <vilib>:"Add State(s) to Queue__JKI_lib_State_Machine.vi"("State(s) in Front (\"\")"=w146, "State(s) in (\"\")"=w149) -> ("States Out"=w148:string)  [unwired: 13 in]
          }
          event User Event {
            # "Acknowledgement_SM event"
            n51 = event-data() -> ("Enqueuer"=w219:refnum<class "Message Enqueuer.lvclass">, "VIName"=w218:string, "VIReference"=w217:refnum<vi>)  [unwired: 1 in]
            n52 = in-place {
              in-place-border: w226 -> [w242]
              in-place-border: w225 -> [w241]
              in-place-border: [w240] -> w224
              in-place-border: [w239] -> w221
              in-place-border: [w235] -> w220
              in-place-border: w219 -> [w234]
              in-place-border: w218 -> [w233]
              in-place-border: w217 -> [w232]
              # "Wait until\nall ACK are \nreceived"
              n53 = in-place-cluster #1(w215) -> ("NumberOfActorsLaunched"=w229:i32, "Ack"=w231:u8, "OutputCluster.Analytics VI refnum"=w228:refnum<vi>)
              n54 = case shown="\"Analytics\"" w233 {
                tunnel: w234 -> [w244 w255 w268 _ w279 w286]
                tunnel: w241 -> [w246 w252 w269 w274 w280 w287]
                tunnel: w242 -> [w249 w256 w270 w272 w281 w288]
                tunnel: [w249 w256 w270 w272 w281 w288] -> w239
                tunnel: [w245 w251 w267 w274 w278 w285] -> w240
                tunnel: w231 -> [w248 w254 w266 w273 w277 w284]
                tunnel: [w247 w253 w265 w273 w276 w283] -> w230
                tunnel: w232 -> [_ _ _ _ w275 _]
                tunnel: w228 -> [w243 w250 w264 w271 _ w282]
                tunnel: [w243 w250 w264 w271 w275 w282] -> w227
                frame "User Interface" {
                  # "Increment Ack count"
                  n55 = Bundle By Name(cluster=w246, "User Interface Actor Enqueuer"=w244) -> (w245:refnum<class "Inspection Statemachine.lvclass">)
                  n56 = Increment(x=w248) -> (x+1=w247:u8)
                }
                frame "Rack Controller" {
                  # "Increment Ack count"
                  n57 = in-place {
                    in-place-border: w255 -> [w263]
                    n58 = First Call?() -> (First Call?: T/F=w260:bool)
                    n59 = in-place-cluster #2(w252) -> ("Rack Controller Actor Enqueuer"=w258:refnum<class "Message Enqueuer.lvclass">[])
                    n60 = Select(t=0, s=w260, f=1) -> (s? t:f=w259:i32)
                    n61 = Insert Into Array(array=w258, index=w259, new element=w263) -> (w257:refnum<class "Message Enqueuer.lvclass">[])
                    n62 = in-place-cluster #2("Rack Controller Actor Enqueuer"=w257) -> (w251:refnum<class "Inspection Statemachine.lvclass">)
                  }
                  n63 = Increment(x=w254) -> (x+1=w253:u8)
                }
                frame "Machine Interface" {
                  # "Increment Ack count"
                  n64 = Bundle By Name(cluster=w269, "Machine Interface Actor Enqueuer"=w268) -> (w267:refnum<class "Inspection Statemachine.lvclass">)
                  n65 = Increment(x=w266) -> (x+1=w265:u8)
                }
                frame Default {
                }
                frame "Analytics" {
                  # "Increment Ack count"
                  n66 = Bundle By Name(cluster=w280, "Analytics Actor Enqueuer"=w279, "AnalyticsVIReference"=w275) -> (w278:refnum<class "Inspection Statemachine.lvclass">)
                  n67 = Increment(x=w277) -> (x+1=w276:u8)
                }
                frame "Data Logger" {
                  # "Increment Ack count"
                  n68 = Bundle By Name(cluster=w287, "Data Logger Actor Enqueuer"=w286) -> (w285:refnum<class "Inspection Statemachine.lvclass">)
                  n69 = Increment(x=w284) -> (x+1=w283:u8)
                }
              }
              n70 = Equal?(x=w229, y=w230) -> (x = y?=w238:bool)
              n71 = Select(t="CallLogo>>open\nSendRackID" ("State(s) in Front (\"\")"), s=w238, f="Wait" ("State(s) in Front (\"\")")) -> (s? t:f=w235:string)
              n72 = in-place-cluster #1("NumberOfActorsLaunched"=w229, "Ack"=w230, "OutputCluster.Analytics VI refnum"=w227) -> (w216:T1)
            }
            n73 = call <vilib>:"Add State(s) to Queue__JKI_lib_State_Machine.vi"("State(s) in Front (\"\")"=w220, "State(s) in (\"\")"=w222) -> ("States Out"=w223:string)  [unwired: 13 in]
          }
          event User Event {
            # "Clear_SM event"
            n74 = event-data() -> ("Clear_SM"=w291:bool)  [unwired: 1 in]
            n75 = Unbundle By Name(w293) -> ("OutputCluster"=w292:T2)
            n76 = case shown="False" w291 {
              tunnel: ["Wait" "SendInit"] -> w296
              tunnel: w290 -> [w302 w309]
              tunnel: w295 -> [w304 w311]
              tunnel: [w303 w311] -> w294
              tunnel: w292 -> [w300 _]
              tunnel: [w299 w309] -> w289
              frame False {
                # "Launch not clear"
                n77 = Bundle By Name(cluster=w300, "StateMsgToSM"="SoftwareExit" ("Button Press")) -> (w305:T2)
                n78 = call "Output_SM.vi"("SM Private Data in"=w302, "Output Cluster"=w305, "Receiver Name"="SM", "State"="SM: StateMessage", "error in (no error)"=w304) -> ("SM Private Data out"=w299:refnum<class "Inspection Statemachine.lvclass">, "error out"=w303:errorcluster)  [unwired: 9 in]
              }
              frame True {
                # "Launch clear"
              }
            }
            n79 = call <vilib>:"Add State(s) to Queue__JKI_lib_State_Machine.vi"("State(s) in Front (\"\")"=w296, "State(s) in (\"\")"=w297) -> ("States Out"=w298:string)  [unwired: 13 in]
          }
          event User Event {
            # "DiagnosticsResult_SM"
            n80 = event-data() -> ("Result"=w316:bool, "StateMessage"=w315:string)  [unwired: 1 in]
            n81 = Unbundle By Name(w318) -> ("OutputCluster"=w317:T2)
            n82 = case shown="False" w316 {
              selector: w316 -> [w334 _]
              tunnel: w314 -> [w332 w406]
              tunnel: w321 -> [w333 w414]
              tunnel: [w327 w403] -> w313
              tunnel: [w331 ""] -> w320
              tunnel: w318 -> [w330 w413]
              tunnel: [w330 w412] -> w319
              tunnel: w315 -> [w329 w407]
              tunnel: w317 -> [w324 w405]
              tunnel: [w326 w404] -> w312
              frame True {
                # "Diagnostics Successful"
                n83 = case shown="\"DoorLocked\"" w329 {
                  selector: w329 -> [_ w359 _ w370 w382 _ w397]
                  tunnel: w334 -> [_ _ _ _ _ _ _]
                  tunnel: w333 -> [w348 w351 w363 w375 w385 w390 w400]
                  tunnel: [w348 w350 w363 w374 w386 w390 w401] -> w328
                  tunnel: w332 -> [w346 w353 w361 w373 w384 w388 w399]
                  tunnel: ["StartDiagnostics" ("State(s) at Back (\"\")") w358 "Wait" ("State with Arguments") w369 w381 "EnableSensors" ("State with Arguments") w396] -> w331
                  tunnel: w324 -> [_ w352 _ w367 w378 _ w394]
                  tunnel: [w346 w349 w361 w364 w376 w388 w391] -> w325
                  frame "ComPortAvailable" {
                    # "Start Power ON Disagnostics \nif COM Port available"
                  }
                  frame "MachinePoweredOn" {
                    n84 = Bundle By Name(cluster=w352, "StateMsgToUI"="DiagnosticsPass") -> (w354:T2)
                    n85 = call "Output_SM.vi"("SM Private Data in"=w353, "Output Cluster"=w354, "Receiver Name"="UI", "State"="UI: StateMessage", "error in (no error)"=w351) -> ("SM Private Data out"=w349:refnum<class "Inspection Statemachine.lvclass">, "error out"=w350:errorcluster)  [unwired: 9 in]
                    n86 = call <vilib>:"Build State String with Arguments__JKI_lib_State_Machine.vi"("Arguments (\"\")"=w359, "State"="NextDiagnostics") -> ("State with Arguments"=w358:string)  [unwired: 4 in]
                  }
                  frame Default {
                  }
                  frame "DeviceReady" {
                    n87 = Bundle By Name(cluster=w367, "StateMsgToUI"="DiagnosticsPass") -> (w365:T2)
                    n88 = call "Output_SM.vi"("SM Private Data in"=w373, "Output Cluster"=w365, "Receiver Name"="UI", "State"="UI: StateMessage", "error in (no error)"=w375) -> ("SM Private Data out"=w364:refnum<class "Inspection Statemachine.lvclass">, "error out"=w374:errorcluster)  [unwired: 9 in]
                    n89 = call <vilib>:"Build State String with Arguments__JKI_lib_State_Machine.vi"("Arguments (\"\")"=w370, "State"="NextDiagnostics") -> ("State with Arguments"=w369:string)  [unwired: 4 in]
                  }
                  frame "MotorDiagnosticsDone" {
                    n90 = Bundle By Name(cluster=w378, "StateMsgToUI"="DiagnosticsPass") -> (w377:T2)
                    n91 = call "Output_SM.vi"("SM Private Data in"=w384, "Output Cluster"=w377, "Receiver Name"="UI", "State"="UI: StateMessage", "error in (no error)"=w385) -> ("SM Private Data out"=w376:refnum<class "Inspection Statemachine.lvclass">, "error out"=w386:errorcluster)  [unwired: 9 in]
                    n92 = call <vilib>:"Build State String with Arguments__JKI_lib_State_Machine.vi"("Arguments (\"\")"=w382, "State"="NextDiagnostics") -> ("State with Arguments"=w381:string)  [unwired: 4 in]
                  }
                  frame "DoorLocked" {
                  }
                  frame "AllCamera", "CameraOpticsDiagnosticsDone" {
                    # "DiagnosticsPass"
                    n93 = Bundle By Name(cluster=w394, "StateMsgToUI"="DiagnosticsPass") -> (w393:T2)
                    n94 = call <vilib>:"Build State String with Arguments__JKI_lib_State_Machine.vi"("Arguments (\"\")"=w397, "State"="NextDiagnostics") -> ("State with Arguments"=w396:string)  [unwired: 4 in]
                    n95 = call "Output_SM.vi"("SM Private Data in"=w399, "Output Cluster"=w393, "Receiver Name"="UI", "State"="UI: StateMessage", "error in (no error)"=w400) -> ("SM Private Data out"=w391:refnum<class "Inspection Statemachine.lvclass">, "error out"=w401:errorcluster)  [unwired: 9 in]
                  }
                }
                n96 = case shown="Default" w329 {
                  tunnel: w328 -> [w336 w341]
                  tunnel: [w336 w340] -> w327
                  tunnel: [w335 w338] -> w326
                  tunnel: w325 -> [w335 w339]
                  tunnel: w324 -> [_ w337]
                  frame "DoorLocked" {
                  }
                  frame Default {
                    n97 = Bundle By Name(cluster=w337, "PopupInput.Pop-up Type"=T8."Close Loading Bar") -> (w342:T2)
                    n98 = call "Output_SM.vi"("SM Private Data in"=w339, "Output Cluster"=w342, "Receiver Name"="UI", "State"="UI: DisplayPopup", "error in (no error)"=w341) -> ("SM Private Data out"=w338:refnum<class "Inspection Statemachine.lvclass">, "error out"=w340:errorcluster)  [unwired: 9 in]
                  }
                }
              }
              frame False {
                # "Diagnostics Failed"
                n99 = Match Pattern(string=w407, regular expression="_") -> (before substring=w408:string, after substring=w409:string)  [unwired: 1 in, 2 out]
                n100 = case shown="\"MotorDiagnosticsFailed\"" w408 {
                  tunnel: w406 -> [w425 w457 w489 w521 w538 w618]
                  tunnel: w414 -> [w435 w469 w491 w523 w541 w617]
                  tunnel: w413 -> [w446 w479 w511 w513 w544 w624]
                  tunnel: [w434 w468 w501 w522 w545 w624] -> w412
                  tunnel: w409 -> [w441 w475 w507 _ w540 _]
                  tunnel: w405 -> [w415 w448 w480 w514 w539 w619]
                  tunnel: [w416 w449 w481 w515 w530 w616] -> w403
                  tunnel: [w417 w450 w482 w512 w529 w615] -> w404
                  tunnel: [w415 w448 w480 w514 w533 w619] -> _
                  frame "ComPortNotAvailable" {
                    n101 = Concatenate Strings("Hardware Unavailable!\nCheck Hardware Connection and Restart the System" ("string"), "\n" ("string"), "Error Code: " ("string"), w441) -> (w438:string)
                    n102 = Bundle By Name(cluster=w446, "DirectExit"=TRUE ("Direct Exit")) -> (w434:T1)
                    n103 = Bundle By Name(cluster=w415, "PopupInput.Title"="ALERT!" ("title"), "PopupInput.Message"=w438, "PopupInput.Title Blink? T/F"=TRUE ("title blink?"), "PopupInput.Button 1 Text"="OK", "PopupInput.Pop-up Type"=T8."One button dialog box") -> (w437:T2)
                    n104 = call "Output_SM.vi"("SM Private Data in"=w425, "Output Cluster"=w437, "Receiver Name"="UI", "State"="UI: DisplayPopup ", "error in (no error)"=w435) -> ("SM Private Data out"=w424:refnum<class "Inspection Statemachine.lvclass">, "error out"=w433:errorcluster)  [unwired: 9 in]
                    n105 = Bundle By Name(cluster=w415, "StateMsgToUI"="DiagnosticsFail") -> (w427:T2)
                    n106 = call "Output_SM.vi"("SM Private Data in"=w424, "Output Cluster"=w427, "Receiver Name"="UI", "State"="UI: StateMessage", "error in (no error)"=w433) -> ("SM Private Data out"=w419:refnum<class "Inspection Statemachine.lvclass">, "error out"=w418:errorcluster)  [unwired: 9 in]
                    n107 = Bundle By Name(cluster=w415, "PopupInput.Pop-up Type"=T8."Close Loading Bar") -> (w420:T2)
                    n108 = call "Output_SM.vi"("SM Private Data in"=w419, "Output Cluster"=w420, "Receiver Name"="UI", "State"="UI: DisplayPopup", "error in (no error)"=w418) -> ("SM Private Data out"=w417:refnum<class "Inspection Statemachine.lvclass">, "error out"=w416:errorcluster)  [unwired: 9 in]
                  }
                  frame "DeviceNotReady", Default {
                    n109 = Concatenate Strings("Hardware Unavailable!\nCheck Hardware and Restart the System" ("string"), "\n" ("string"), "Error Code: " ("string"), w475) -> (w472:string)
                    n110 = Bundle By Name(cluster=w479, "DirectExit"=TRUE ("Direct Exit"), "SoftwareExit"=TRUE) -> (w468:T1)
                    n111 = Bundle By Name(cluster=w448, "PopupInput.Title"="ALERT!" ("title"), "PopupInput.Message"=w472, "PopupInput.Title Blink? T/F"=TRUE ("title blink?"), "PopupInput.Button 1 Text"="OK", "PopupInput.Pop-up Type"=T8."One button dialog box") -> (w471:T2)
                    n112 = call "Output_SM.vi"("SM Private Data in"=w457, "Output Cluster"=w471, "Receiver Name"="UI", "State"="UI: DisplayPopup", "error in (no error)"=w469) -> ("SM Private Data out"=w456:refnum<class "Inspection Statemachine.lvclass">, "error out"=w467:errorcluster)  [unwired: 9 in]
                    n113 = Bundle By Name(cluster=w448, "StateMsgToUI"="DiagnosticsFail") -> (w461:T2)
                    n114 = call "Output_SM.vi"("SM Private Data in"=w456, "Output Cluster"=w461, "Receiver Name"="UI", "State"="UI: StateMessage", "error in (no error)"=w467) -> ("SM Private Data out"=w452:refnum<class "Inspection Statemachine.lvclass">, "error out"=w451:errorcluster)  [unwired: 9 in]
                    n115 = Bundle By Name(cluster=w448, "PopupInput.Pop-up Type"=T8."Close Loading Bar") -> (w453:T2)
                    n116 = call "Output_SM.vi"("SM Private Data in"=w452, "Output Cluster"=w453, "Receiver Name"="UI", "State"="UI: DisplayPopup", "error in (no error)"=w451) -> ("SM Private Data out"=w450:refnum<class "Inspection Statemachine.lvclass">, "error out"=w449:errorcluster)  [unwired: 9 in]
                  }
                  frame "MachineNotPoweredOn" {
                    n117 = Bundle By Name(cluster=w511, "DirectExit"=TRUE ("Direct Exit"), "SoftwareExit"=TRUE) -> (w501:T1)
                    n118 = Bundle By Name(cluster=w480, "StateMsgToUI"="DiagnosticsFail") -> (w493:T2)
                    n119 = call "Output_SM.vi"("SM Private Data in"=w489, "Output Cluster"=w493, "Receiver Name"="UI", "State"="UI: StateMessage", "error in (no error)"=w491) -> ("error out"=w490:errorcluster)  [unwired: 9 in, 1 out]
                    n120 = Concatenate Strings("Machine is not powered ON!\nPower ON the system" ("string"), "\n" ("string"), "Error Code: " ("string"), w507) -> (w504:string)
                    n121 = Bundle By Name(cluster=w480, "PopupInput.Title"="ALERT!" ("title"), "PopupInput.Message"=w504, "PopupInput.Title Blink? T/F"=TRUE ("title blink?"), "PopupInput.Button 1 Text"="OK", "PopupInput.Pop-up Type"=T8."One button dialog box") -> (w503:T2)
                    n122 = call "Output_SM.vi"("SM Private Data in"=w489, "Output Cluster"=w503, "Receiver Name"="UI", "State"="UI: DisplayPopup", "error in (no error)"=w490) -> ("SM Private Data out"=w483:refnum<class "Inspection Statemachine.lvclass">, "error out"=w484:errorcluster)  [unwired: 9 in]
                    n123 = Bundle By Name(cluster=w480, "PopupInput.Pop-up Type"=T8."Close Loading Bar") -> (w485:T2)
                    n124 = call "Output_SM.vi"("SM Private Data in"=w483, "Output Cluster"=w485, "Receiver Name"="UI", "State"="UI: DisplayPopup", "error in (no error)"=w484) -> ("SM Private Data out"=w482:refnum<class "Inspection Statemachine.lvclass">, "error out"=w481:errorcluster)  [unwired: 9 in]
                  }
                  frame "DoorNotLocked" {
                    n125 = Bundle By Name(cluster=w513, "DirectExit"=FALSE ("Direct Exit"), "SoftwareExit"=FALSE ("Software Exit?")) -> (w522:T1)
                    n126 = Bundle By Name(cluster=w514, "PopupInput.Title"="ALERT!" ("title"), "PopupInput.Message"="Please close the door and press OK" ("string"), "PopupInput.Title Blink? T/F"=TRUE ("title blink?"), "PopupInput.Button 1 Text"="OK", "PopupInput.Pop-up Type"=T8."One button dialog box") -> (w525:T2)
                    n127 = call "Output_SM.vi"("SM Private Data in"=w521, "Output Cluster"=w525, "Receiver Name"="UI", "State"="UI: DisplayPopup", "error in (no error)"=w523) -> ("SM Private Data out"=w512:refnum<class "Inspection Statemachine.lvclass">, "error out"=w515:errorcluster)  [unwired: 9 in]
                  }
                  frame "MotorDiagnosticsFailed" {
                    n128 = case shown="Default" w540 {
                      selector: w540 -> [w556 w579 w603]
                      tunnel: [w559 w582 w605] -> w531
                      tunnel: w538 -> [w557 w580 w595]
                      tunnel: w541 -> [w558 w581 w604]
                      tunnel: w539 -> [w546 w569 w592]
                      tunnel: [w548 w570 w593] -> w532
                      tunnel: [w546 w569 w592] -> w533
                      frame "0x03000200" {
                        # "Guides failed to open"
                        n129 = Concatenate Strings("Guides Failed to Open!\nCheck Motor" ("string"), "\n" ("string"), "Error Code: " ("string"), w556) -> (w563:string)
                        n130 = Bundle By Name(cluster=w546, "PopupInput.Title"="ALERT!" ("title"), "PopupInput.Message"=w563, "PopupInput.Title Blink? T/F"=TRUE ("title blink?"), "PopupInput.Button 1 Text"="OK", "PopupInput.Pop-up Type"=T8."One button dialog box") -> (w566:T2)
                        n131 = call "Output_SM.vi"("SM Private Data in"=w557, "Output Cluster"=w566, "Receiver Name"="UI", "State"="UI: DisplayPopup", "error in (no error)"=w558) -> ("SM Private Data out"=w547:refnum<class "Inspection Statemachine.lvclass">, "error out"=w561:errorcluster)  [unwired: 9 in]
                        n132 = Bundle By Name(cluster=w546, "StateMsgToUI"="DiagnosticsFail") -> (w551:T2)
                        n133 = call "Output_SM.vi"("SM Private Data in"=w547, "Output Cluster"=w551, "Receiver Name"="UI", "State"="UI: StateMessage", "error in (no error)"=w561) -> ("SM Private Data out"=w548:refnum<class "Inspection Statemachine.lvclass">, "error out"=w559:errorcluster)  [unwired: 9 in]
                      }
                      frame "0x03000300" {
                        # "Guides failed to open"
                        n134 = Concatenate Strings("Guides Failed to Close!\nCheck Motor" ("string"), "\n" ("string"), "Error Code: " ("string"), w579) -> (w586:string)
                        n135 = Bundle By Name(cluster=w569, "PopupInput.Title"="ALERT!" ("title"), "PopupInput.Message"=w586, "PopupInput.Title Blink? T/F"=TRUE ("title blink?"), "PopupInput.Button 1 Text"="OK", "PopupInput.Pop-up Type"=T8."One button dialog box") -> (w589:T2)
                        n136 = call "Output_SM.vi"("SM Private Data in"=w580, "Output Cluster"=w589, "Receiver Name"="UI", "State"="UI: DisplayPopup", "error in (no error)"=w581) -> ("SM Private Data out"=w571:refnum<class "Inspection Statemachine.lvclass">, "error out"=w584:errorcluster)  [unwired: 9 in]
                        n137 = Bundle By Name(cluster=w569, "StateMsgToUI"="DiagnosticsFail") -> (w575:T2)
                        n138 = call "Output_SM.vi"("SM Private Data in"=w571, "Output Cluster"=w575, "Receiver Name"="UI", "State"="UI: StateMessage", "error in (no error)"=w584) -> ("SM Private Data out"=w570:refnum<class "Inspection Statemachine.lvclass">, "error out"=w582:errorcluster)  [unwired: 9 in]
                      }
                      frame Default {
                        n139 = Concatenate Strings("Motor Diagnostics Failed!\nRestart the System" ("string"), "\n" ("string"), "Error Code: " ("string"), w603) -> (w609:string)
                        n140 = Bundle By Name(cluster=w592, "PopupInput.Title"="ALERT!" ("title"), "PopupInput.Message"=w609, "PopupInput.Title Blink? T/F"=TRUE ("title blink?"), "PopupInput.Button 1 Text"="OK", "PopupInput.Pop-up Type"=T8."One button dialog box") -> (w612:T2)
                        n141 = call "Output_SM.vi"("SM Private Data in"=w595, "Output Cluster"=w612, "Receiver Name"="UI", "State"="UI: DisplayPopup", "error in (no error)"=w604) -> ("SM Private Data out"=w594:refnum<class "Inspection Statemachine.lvclass">, "error out"=w607:errorcluster)  [unwired: 9 in]
                        n142 = Bundle By Name(cluster=w592, "StateMsgToUI"="DiagnosticsFail") -> (w599:T2)
                        n143 = call "Output_SM.vi"("SM Private Data in"=w594, "Output Cluster"=w599, "Receiver Name"="UI", "State"="UI: StateMessage", "error in (no error)"=w607) -> ("SM Private Data out"=w593:refnum<class "Inspection Statemachine.lvclass">, "error out"=w605:errorcluster)  [unwired: 9 in]
                      }
                    }
                    n144 = Bundle By Name(cluster=w544, "DirectExit"=TRUE ("Direct Exit"), "SoftwareExit"=TRUE ("Software Exit?")) -> (w545:T1)
                    n145 = Bundle By Name(cluster=w533, "PopupInput.Pop-up Type"=T8."Close Loading Bar") -> (w534:T2)
                    n146 = call "Output_SM.vi"("SM Private Data in"=w532, "Output Cluster"=w534, "Receiver Name"="UI", "State"="UI: DisplayPopup", "error in (no error)"=w531) -> ("SM Private Data out"=w529:refnum<class "Inspection Statemachine.lvclass">, "error out"=w530:errorcluster)  [unwired: 9 in]
                  }
                  frame "AllCameraFailed", "CameraOpticsDiagnosticsFailed" {
                    n147 = Bundle By Name(cluster=w619, "PopupInput.Pop-up Type"=T8."Close Loading Bar") -> (w620:T2)
                    n148 = call "Output_SM.vi"("SM Private Data in"=w618, "Output Cluster"=w620, "Receiver Name"="UI", "State"="UI: DisplayPopup", "error in (no error)"=w617) -> ("SM Private Data out"=w615:refnum<class "Inspection Statemachine.lvclass">, "error out"=w616:errorcluster)  [unwired: 9 in]
                  }
                }
              }
            }
            n149 = call <vilib>:"Add State(s) to Queue__JKI_lib_State_Machine.vi"("State(s) in Front (\"\")"=w320, "State(s) in (\"\")"=w322) -> ("States Out"=w323:string)  [unwired: 13 in]
          }
          event "Diagnostics Result": Value Change {
            # "DiagnosticsResult_SM"
            n150 = event-data() -> ("NewVal"=w636:string)  [unwired: 1 in, 1 out]
            n151 = Unbundle By Name(w638) -> ("OutputCluster"=w637:T2)
            n152 = case shown="False" TRUE {
              selector: TRUE -> [w653 _]
              tunnel: w634 -> [w646 w712]
              tunnel: w641 -> [w652 w720]
              tunnel: [w651 w710] -> w626
              tunnel: [w650 ""] -> w640
              tunnel: w638 -> [w649 w719]
              tunnel: [w649 w718] -> w639
              tunnel: w636 -> [w648 w713]
              tunnel: w637 -> [w647 w711]
              tunnel: [w645 w709] -> w629
              tunnel: [w644 w708] -> w625
              frame True {
                # "Diagnostics Successful"
                n153 = case shown="\"DoorLocked\"" w648 {
                  selector: w648 -> [_ w661 _ w674 w686 _ w702]
                  tunnel: w653 -> [_ _ _ _ _ _ _]
                  tunnel: w652 -> [w657 w663 w667 w679 w689 w695 w705]
                  tunnel: [w657 w663 w667 w678 w690 w695 w706] -> w651
                  tunnel: w646 -> [w655 w659 w665 w677 w688 w693 w704]
                  tunnel: ["StartDiagnostics" ("State(s) at Back (\"\")") w660 "Wait" ("State with Arguments") w673 w685 "EnableSensors" ("State with Arguments") w701] -> w650
                  tunnel: w647 -> [w654 w658 w664 w668 w680 w692 w696]
                  tunnel: [w655 w659 w665 w669 w681 w693 w697] -> w645
                  tunnel: [w654 w658 w664 w668 w680 w692 w696] -> w644
                  frame "ComPortAvailable" {
                    # "Start Power ON Disagnostics \nif COM Port available"
                  }
                  frame "MachinePoweredOn" {
                    n154 = call <vilib>:"Build State String with Arguments__JKI_lib_State_Machine.vi"("Arguments (\"\")"=w661, "State"="NextDiagnostics") -> ("State with Arguments"=w660:string)  [unwired: 4 in]
                  }
                  frame Default {
                  }
                  frame "DeviceReady" {
                    n155 = Bundle By Name(cluster=w668, "StateMsgToUI"="DiagnosticsPass") -> (w670:T2)
                    n156 = call "Output_SM.vi"("SM Private Data in"=w677, "Output Cluster"=w670, "Receiver Name"="UI", "State"="UI: StateMessage", "error in (no error)"=w679) -> ("SM Private Data out"=w669:refnum<class "Inspection Statemachine.lvclass">, "error out"=w678:errorcluster)  [unwired: 9 in]
                    n157 = call <vilib>:"Build State String with Arguments__JKI_lib_State_Machine.vi"("Arguments (\"\")"=w674, "State"="NextDiagnostics") -> ("State with Arguments"=w673:string)  [unwired: 4 in]
                  }
                  frame "MotorDiagnosticsDone" {
                    n158 = Bundle By Name(cluster=w680, "StateMsgToUI"="DiagnosticsPass") -> (w682:T2)
                    n159 = call "Output_SM.vi"("SM Private Data in"=w688, "Output Cluster"=w682, "Receiver Name"="UI", "State"="UI: StateMessage", "error in (no error)"=w689) -> ("SM Private Data out"=w681:refnum<class "Inspection Statemachine.lvclass">, "error out"=w690:errorcluster)  [unwired: 9 in]
                    n160 = call <vilib>:"Build State String with Arguments__JKI_lib_State_Machine.vi"("Arguments (\"\")"=w686, "State"="NextDiagnostics") -> ("State with Arguments"=w685:string)  [unwired: 4 in]
                  }
                  frame "DoorLocked" {
                  }
                  frame "AllCamera", "CameraOpticsDiagnosticsDone" {
                    # "DiagnosticsPass"
                    n161 = Bundle By Name(cluster=w696, "StateMsgToUI"="DiagnosticsPass") -> (w699:T2)
                    n162 = call <vilib>:"Build State String with Arguments__JKI_lib_State_Machine.vi"("Arguments (\"\")"=w702, "State"="NextDiagnostics") -> ("State with Arguments"=w701:string)  [unwired: 4 in]
                    n163 = call "Output_SM.vi"("SM Private Data in"=w704, "Output Cluster"=w699, "Receiver Name"="UI", "State"="UI: StateMessage", "error in (no error)"=w705) -> ("SM Private Data out"=w697:refnum<class "Inspection Statemachine.lvclass">, "error out"=w706:errorcluster)  [unwired: 9 in]
                  }
                }
              }
              frame False {
                # "Diagnostics Failed"
                n164 = Match Pattern(string=w713, regular expression="_") -> (before substring=w714:string, after substring=w715:string)  [unwired: 1 in, 2 out]
                n165 = case shown="\"MotorDiagnosticsFailed\"" w714 {
                  tunnel: w712 -> [w724 w750 w777 w809 w821 w899]
                  tunnel: w720 -> [w735 w763 w790 w811 w824 w900]
                  tunnel: w719 -> [w746 w773 w800 w817 w827 w901]
                  tunnel: [w734 w762 w789 w810 w828 w901] -> w718
                  tunnel: w715 -> [w741 w769 w796 _ w823 _]
                  tunnel: w711 -> [w721 w747 w774 w801 w822 w898]
                  tunnel: [w732 w760 w787 w805 w820 w900] -> w710
                  tunnel: [w722 w748 w775 w802 w819 w899] -> w709
                  tunnel: [w721 w747 w774 w801 w818 w898] -> w708
                  frame "ComPortNotAvailable" {
                    n166 = Concatenate Strings("Hardware Unavailable!\nCheck Hardware Connection and Restart the System" ("string"), "\n" ("string"), "Error Code: " ("string"), w741) -> (w738:string)
                    n167 = Bundle By Name(cluster=w746, "DirectExit"=TRUE ("Direct Exit")) -> (w734:T1)
                    n168 = Bundle By Name(cluster=w721, "PopupInput.Title"="ALERT!" ("title"), "PopupInput.Message"=w738, "PopupInput.Title Blink? T/F"=TRUE ("title blink?"), "PopupInput.Button 1 Text"="OK", "PopupInput.Pop-up Type"=T8."One button dialog box") -> (w737:T2)
                    n169 = call "Output_SM.vi"("SM Private Data in"=w724, "Output Cluster"=w737, "Receiver Name"="UI", "State"=" UI: DisplayPopup ", "error in (no error)"=w735) -> ("SM Private Data out"=w723:refnum<class "Inspection Statemachine.lvclass">, "error out"=w733:errorcluster)  [unwired: 9 in]
                    n170 = Bundle By Name(cluster=w721, "StateMsgToUI"="DiagnosticsFail") -> (w726:T2)
                    n171 = call "Output_SM.vi"("SM Private Data in"=w723, "Output Cluster"=w726, "Receiver Name"="UI", "State"="UI: StateMessage", "error in (no error)"=w733) -> ("SM Private Data out"=w722:refnum<class "Inspection Statemachine.lvclass">, "error out"=w732:errorcluster)  [unwired: 9 in]
                  }
                  frame "DeviceNotReady", Default {
                    n172 = Concatenate Strings("Hardware Unavailable!\nCheck Hardware and Restart the System" ("string"), "\n" ("string"), "Error Code: " ("string"), w769) -> (w766:string)
                    n173 = Bundle By Name(cluster=w773, "DirectExit"=TRUE ("Direct Exit"), "SoftwareExit"=TRUE) -> (w762:T1)
                    n174 = Bundle By Name(cluster=w747, "PopupInput.Title"="ALERT!" ("title"), "PopupInput.Message"=w766, "PopupInput.Title Blink? T/F"=TRUE ("title blink?"), "PopupInput.Button 1 Text"="OK", "PopupInput.Pop-up Type"=T8."One button dialog box") -> (w765:T2)
                    n175 = call "Output_SM.vi"("SM Private Data in"=w750, "Output Cluster"=w765, "Receiver Name"="UI", "State"=" UI: DisplayPopup ", "error in (no error)"=w763) -> ("SM Private Data out"=w749:refnum<class "Inspection Statemachine.lvclass">, "error out"=w761:errorcluster)  [unwired: 9 in]
                    n176 = Bundle By Name(cluster=w747, "StateMsgToUI"="DiagnosticsFail") -> (w754:T2)
                    n177 = call "Output_SM.vi"("SM Private Data in"=w749, "Output Cluster"=w754, "Receiver Name"="UI", "State"="UI: StateMessage", "error in (no error)"=w761) -> ("SM Private Data out"=w748:refnum<class "Inspection Statemachine.lvclass">, "error out"=w760:errorcluster)  [unwired: 9 in]
                  }
                  frame "MachineNotPoweredOn" {
                    n178 = Concatenate Strings("Machine is not powered ON!\nPower ON the system" ("string"), "\n" ("string"), "Error Code: " ("string"), w796) -> (w793:string)
                    n179 = Bundle By Name(cluster=w800, "DirectExit"=TRUE ("Direct Exit"), "SoftwareExit"=TRUE) -> (w789:T1)
                    n180 = Bundle By Name(cluster=w774, "PopupInput.Title"="ALERT!" ("title"), "PopupInput.Message"=w793, "PopupInput.Title Blink? T/F"=TRUE ("title blink?"), "PopupInput.Button 1 Text"="OK", "PopupInput.Pop-up Type"=T8."One button dialog box") -> (w792:T2)
                    n181 = call "Output_SM.vi"("SM Private Data in"=w777, "Output Cluster"=w792, "Receiver Name"="UI", "State"=" UI: DisplayPopup ", "error in (no error)"=w790) -> ("SM Private Data out"=w776:refnum<class "Inspection Statemachine.lvclass">, "error out"=w788:errorcluster)  [unwired: 9 in]
                    n182 = Bundle By Name(cluster=w774, "StateMsgToUI"="DiagnosticsFail") -> (w781:T2)
                    n183 = call "Output_SM.vi"("SM Private Data in"=w776, "Output Cluster"=w781, "Receiver Name"="UI", "State"="UI: StateMessage", "error in (no error)"=w788) -> ("SM Private Data out"=w775:refnum<class "Inspection Statemachine.lvclass">, "error out"=w787:errorcluster)  [unwired: 9 in]
                  }
                  frame "DoorNotLocked" {
                    n184 = Bundle By Name(cluster=w817, "DirectExit"=FALSE ("Direct Exit"), "SoftwareExit"=FALSE ("Software Exit?")) -> (w810:T1)
                    n185 = Bundle By Name(cluster=w801, "PopupInput.Title"="ALERT!" ("title"), "PopupInput.Message"="Please close the door and press OK" ("string"), "PopupInput.Title Blink? T/F"=TRUE ("title blink?"), "PopupInput.Button 1 Text"="OK", "PopupInput.Pop-up Type"=T8."One button dialog box") -> (w813:T2)
                    n186 = call "Output_SM.vi"("SM Private Data in"=w809, "Output Cluster"=w813, "Receiver Name"="UI", "State"=" UI: DisplayPopup ", "error in (no error)"=w811) -> ("SM Private Data out"=w802:refnum<class "Inspection Statemachine.lvclass">, "error out"=w805:errorcluster)  [unwired: 9 in]
                  }
                  frame "MotorDiagnosticsFailed" {
                    n187 = case shown="\"0x03000300\"" w823 {
                      selector: w823 -> [w840 w863 w886]
                      tunnel: [w842 w865 w888] -> w820
                      tunnel: w821 -> [w832 w855 w878]
                      tunnel: w824 -> [w841 w864 w887]
                      tunnel: w822 -> [w829 w852 w875]
                      tunnel: [w830 w853 w876] -> w819
                      tunnel: [w829 w852 w875] -> w818
                      frame "0x03000200" {
                        # "Guides failed to open"
                        n188 = Concatenate Strings("Guides Failed to Open!\nCheck Motor" ("string"), "\n" ("string"), "Error Code: " ("string"), w840) -> (w846:string)
                        n189 = Bundle By Name(cluster=w829, "PopupInput.Title"="ALERT!" ("title"), "PopupInput.Message"=w846, "PopupInput.Title Blink? T/F"=TRUE ("title blink?"), "PopupInput.Button 1 Text"="OK", "PopupInput.Pop-up Type"=T8."One button dialog box") -> (w849:T2)
                        n190 = call "Output_SM.vi"("SM Private Data in"=w832, "Output Cluster"=w849, "Receiver Name"="UI", "State"="UI: DisplayPopup", "error in (no error)"=w841) -> ("SM Private Data out"=w831:refnum<class "Inspection Statemachine.lvclass">, "error out"=w844:errorcluster)  [unwired: 9 in]
                        n191 = Bundle By Name(cluster=w829, "StateMsgToUI"="DiagnosticsFail") -> (w835:T2)
                        n192 = call "Output_SM.vi"("SM Private Data in"=w831, "Output Cluster"=w835, "Receiver Name"="UI", "State"="UI: StateMessage", "error in (no error)"=w844) -> ("SM Private Data out"=w830:refnum<class "Inspection Statemachine.lvclass">, "error out"=w842:errorcluster)  [unwired: 9 in]
                      }
                      frame "0x03000300" {
                        # "Guides failed to open"
                        n193 = Concatenate Strings("Guides Failed to Close!\nCheck Motor" ("string"), "\n" ("string"), "Error Code: " ("string"), w863) -> (w869:string)
                        n194 = Bundle By Name(cluster=w852, "PopupInput.Title"="ALERT!" ("title"), "PopupInput.Message"=w869, "PopupInput.Title Blink? T/F"=TRUE ("title blink?"), "PopupInput.Button 1 Text"="OK", "PopupInput.Pop-up Type"=T8."One button dialog box") -> (w872:T2)
                        n195 = call "Output_SM.vi"("SM Private Data in"=w855, "Output Cluster"=w872, "Receiver Name"="UI", "State"="UI: DisplayPopup", "error in (no error)"=w864) -> ("SM Private Data out"=w854:refnum<class "Inspection Statemachine.lvclass">, "error out"=w867:errorcluster)  [unwired: 9 in]
                        n196 = Bundle By Name(cluster=w852, "StateMsgToUI"="DiagnosticsFail") -> (w859:T2)
                        n197 = call "Output_SM.vi"("SM Private Data in"=w854, "Output Cluster"=w859, "Receiver Name"="UI", "State"="UI: StateMessage", "error in (no error)"=w867) -> ("SM Private Data out"=w853:refnum<class "Inspection Statemachine.lvclass">, "error out"=w865:errorcluster)  [unwired: 9 in]
                      }
                      frame Default {
                        n198 = Concatenate Strings("Motor Diagnostics Failed!\nRestart the System" ("string"), "\n" ("string"), "Error Code: " ("string"), w886) -> (w892:string)
                        n199 = Bundle By Name(cluster=w875, "PopupInput.Title"="ALERT!" ("title"), "PopupInput.Message"=w892, "PopupInput.Title Blink? T/F"=TRUE ("title blink?"), "PopupInput.Button 1 Text"="OK", "PopupInput.Pop-up Type"=T8."One button dialog box") -> (w895:T2)
                        n200 = call "Output_SM.vi"("SM Private Data in"=w878, "Output Cluster"=w895, "Receiver Name"="UI", "State"="UI: DisplayPopup", "error in (no error)"=w887) -> ("SM Private Data out"=w877:refnum<class "Inspection Statemachine.lvclass">, "error out"=w890:errorcluster)  [unwired: 9 in]
                        n201 = Bundle By Name(cluster=w875, "StateMsgToUI"="DiagnosticsFail") -> (w882:T2)
                        n202 = call "Output_SM.vi"("SM Private Data in"=w877, "Output Cluster"=w882, "Receiver Name"="UI", "State"="UI: StateMessage", "error in (no error)"=w890) -> ("SM Private Data out"=w876:refnum<class "Inspection Statemachine.lvclass">, "error out"=w888:errorcluster)  [unwired: 9 in]
                      }
                    }
                    n203 = Bundle By Name(cluster=w827, "DirectExit"=TRUE ("Direct Exit"), "SoftwareExit"=TRUE ("Software Exit?")) -> (w828:T1)
                  }
                  frame "AllCameraFailed", "CameraOpticsDiagnosticsFailed" {
                  }
                }
              }
            }
            n204 = call <vilib>:"Add State(s) to Queue__JKI_lib_State_Machine.vi"("State(s) in Front (\"\")"=w640, "State(s) in (\"\")"=w642) -> ("States Out"=w643:string)  [unwired: 13 in]
            n205 = Bundle By Name(cluster=w625, "PopupInput.Pop-up Type"=T8."Close Loading Bar") -> (w631:T2)
            n206 = call "Output_SM.vi"("SM Private Data in"=w629, "Output Cluster"=w631, "Receiver Name"="UI", "State"="UI: DisplayPopup", "error in (no error)"=w626) -> ("SM Private Data out"=w628:refnum<class "Inspection Statemachine.lvclass">, "error out"=w627:errorcluster)  [unwired: 9 in]
          }
          event User Event {
            # "InitiateSensorDiagnostics_EM event"
            n207 = event-data() -> ("SensorName"=w905:string)  [unwired: 1 in]
            n208 = Bundle By Name(cluster=w904, "OutputCluster.Sensor Name"=w905) -> (w903:T1)
            n209 = call <vilib>:"Add State(s) to Queue__JKI_lib_State_Machine.vi"("State(s) in Front (\"\")"="ObtainSensorIndex" ("State(s) in Front (\"\")"), "State(s) in (\"\")"=w909) -> ("States Out"=w908:string)  [unwired: 13 in]
          }
          event User Event {
            # "DataLogger_FileOpen"
            # "ErrorMessage_SM event"
            n210 = event-data() -> ("ErrorMessage"=w916:string)  [unwired: 1 in]
            n211 = Unbundle By Name(w915) -> ("OutputCluster"=w914:T2, "CurrentState"=w911:string, "OutputCluster.SystemParameters.SoftwareFeatures.PopupOptions.ReasonForStop"=w910:bool)
            n212 = Match Pattern(string=w916, regular expression="_") -> (before substring=w918:string, after substring=w919:string)  [unwired: 1 in, 2 out]
            n213 = case shown="\"Algorithm\"" w918 {
              tunnel: [w933 w953 w1030 w1079 w1100 w1121] -> w917
              tunnel: w922 -> [w934 w951 w1029 w1080 w1101 w1120]
              tunnel: w915 -> [w945 w947 w1027 w1090 w1111 w1112]
              tunnel: [w943 w955 w1028 w1088 w1109 w1113] -> w921
              tunnel: w919 -> [w939 w946 _ w1085 w1106 w1119]
              tunnel: w913 -> [w932 w950 w1025 w1078 w1099 w1117]
              tunnel: w914 -> [w931 w949 w1023 w1077 w1098 w1118]
              tunnel: [w925 w952 w1026 w1070 w1091 w1116] -> w912
              tunnel: w911 -> [_ _ w1024 _ _ _]
              tunnel: w910 -> [_ _ w1022 _ _ _]
              frame "ArduinoDisconnection", "ArduinoError", "TMConfigurationError", Default {
                n214 = Bundle By Name(cluster=w945, "DirectExit"=TRUE ("Direct Exit"), "SoftwareExit"=TRUE ("Software Exit?")) -> (w943:T1)
                n215 = Concatenate Strings("Hardware Error! \nRestart the System" ("string"), "\n" ("string"), "Error Code: " ("string"), w939) -> (w935:string)
                n216 = Bundle By Name(cluster=w931, "PopupInput.Title"="ALERT!" ("title"), "PopupInput.Message"=w935, "PopupInput.Title Blink? T/F"=TRUE ("title blink?"), "PopupInput.Button 1 Text"="OK", "PopupInput.Pop-up Type"=T8."One button dialog box") -> (w928:T2)
                n217 = call "Output_SM.vi"("SM Private Data in"=w932, "Output Cluster"=w928, "Receiver Name"="UI", "State"="UI: DisplayPopup", "error in (no error)"=w934) -> ("SM Private Data out"=w925:refnum<class "Inspection Statemachine.lvclass">, "error out"=w933:errorcluster)  [unwired: 9 in]
              }
              frame "Algorithm" {
                # "0x0700F002=PartNotFound(JSON Error during part selection or inspection)\n0x0700F003=Incorrect Calibaration File Path(JSON Error)\n0x0700F001=Read JSON SubVI Error"
                n218 = case shown="\"0x0700F001\"" w946 {
                  tunnel: [w962 w985] -> w953
                  tunnel: [w963 w984] -> w952
                  tunnel: w951 -> [w961 w978]
                  tunnel: w950 -> [w960 w977]
                  tunnel: w949 -> [w959 w975]
                  tunnel: w946 -> [w958 w974]
                  frame "0x0700F001" {
                    n219 = Concatenate Strings("Error!\nRestart the System" ("string"), "\n" ("string"), "Error Code: " ("string"), w958) -> (w970:string)
                    n220 = Bundle By Name(cluster=w959, "PopupInput.Title"="ALERT!" ("title"), "PopupInput.Message"=w970, "PopupInput.Title Blink? T/F"=TRUE ("title blink?"), "PopupInput.Button 1 Text"="OK", "PopupInput.Pop-up Type"=T8."One button dialog box") -> (w967:T2)
                    n221 = call "Output_SM.vi"("SM Private Data in"=w960, "Output Cluster"=w967, "Receiver Name"="UI", "State"="UI: DisplayPopup", "error in (no error)"=w961) -> ("SM Private Data out"=w963:refnum<class "Inspection Statemachine.lvclass">, "error out"=w962:errorcluster)  [unwired: 9 in]
                  }
                  frame Default {
                    n222 = Bundle By Name(cluster=w975, "PopupInput.Pop-up Type"=T8."Close Loading Bar" ("LoadingBarInput.Pop-up Type")) -> (w982:T2)
                    n223 = call "Output_SM.vi"("SM Private Data in"=w977, "Output Cluster"=w982, "Receiver Name"="UI", "State"="UI: DisplayPopup", "error in (no error)"=w978) -> ("SM Private Data out"=w976:refnum<class "Inspection Statemachine.lvclass">, "error out"=w979:errorcluster)  [unwired: 9 in]
                    n224 = case shown="\"0x0700F002\"" w974 {
                      tunnel: w974 -> [_ w1003 w1020]
                      tunnel: [w986 w999 w1016] -> w985
                      tunnel: [w987 w993 w1010] -> w984
                      tunnel: w979 -> [w986 w991 w1008]
                      tunnel: w976 -> [w987 w990 w1007]
                      tunnel: w975 -> [_ w989 w1006]
                      frame "False", Default {
                      }
                      frame "0x0700F002" {
                        n225 = Concatenate Strings("Error!\nRestart the System" ("string"), "\n" ("string"), "Error Code: " ("string"), w1003) -> (w1000:string)
                        n226 = Bundle By Name(cluster=w989, "PopupInput.Title"="ALERT!" ("title"), "PopupInput.Message"=w1000, "PopupInput.Title Blink? T/F"=TRUE ("title blink?"), "PopupInput.Button 1 Text"="OK", "PopupInput.Pop-up Type"=T8."One button dialog box") -> (w996:T2)
                        n227 = call "Output_SM.vi"("SM Private Data in"=w990, "Output Cluster"=w996, "Receiver Name"="UI", "State"="UI: DisplayPopup", "error in (no error)"=w991) -> ("SM Private Data out"=w993:refnum<class "Inspection Statemachine.lvclass">, "error out"=w999:errorcluster)  [unwired: 9 in]
                      }
                      frame "0x0700F003" {
                        n228 = Concatenate Strings("Error!\nRestart the System" ("string"), "\n" ("string"), "Error Code: " ("string"), w1020) -> (w1017:string)
                        n229 = Bundle By Name(cluster=w1006, "PopupInput.Title"="ALERT!" ("title"), "PopupInput.Message"=w1017, "PopupInput.Title Blink? T/F"=TRUE ("title blink?"), "PopupInput.Button 1 Text"="OK", "PopupInput.Pop-up Type"=T8."One button dialog box") -> (w1013:T2)
                        n230 = call "Output_SM.vi"("SM Private Data in"=w1007, "Output Cluster"=w1013, "Receiver Name"="UI", "State"="UI: DisplayPopup", "error in (no error)"=w1008) -> ("SM Private Data out"=w1010:refnum<class "Inspection Statemachine.lvclass">, "error out"=w1016:errorcluster)  [unwired: 9 in]
                      }
                    }
                  }
                }
                n231 = Bundle By Name(cluster=w947, "DirectExit"=FALSE ("Direct Exit"), "SoftwareExit"=TRUE ("Software Exit?"), "CurrentState"="Error") -> (w955:T1)
              }
              frame "DataLogger" {
                n232 = case shown="Default" w1024 {
                  tunnel: [w1031 w1037 w1052] -> w1030
                  tunnel: w1029 -> [w1031 w1038 w1053]
                  tunnel: [w1032 w1047 w1054] -> w1028
                  tunnel: w1027 -> [w1032 w1047 w1054]
                  tunnel: [w1033 w1035 w1050] -> w1026
                  tunnel: w1025 -> [w1033 w1036 w1051]
                  tunnel: w1023 -> [_ w1034 w1049]
                  tunnel: w1022 -> [_ _ w1048]
                  frame Default {
                  }
                  frame "SoftwareExit" {
                    n233 = Bundle By Name(cluster=w1034, "PopupInput.Title"="ALERT!" ("title"), "PopupInput.Message"="File Open!\nUnable To Write.Please Close Data File." ("string"), "PopupInput.Title Blink? T/F"=TRUE ("title blink?"), "PopupInput.Button 1 Text"="OK", "PopupInput.Pop-up Type"=T8."One button dialog box") -> (w1041:T2)
                    n234 = call "Output_SM.vi"("SM Private Data in"=w1036, "Output Cluster"=w1041, "Receiver Name"="UI", "State"="UI: DisplayPopup", "error in (no error)"=w1038) -> ("SM Private Data out"=w1035:refnum<class "Inspection Statemachine.lvclass">, "error out"=w1037:errorcluster)  [unwired: 9 in]
                  }
                  frame "Stop" {
                    n235 = case shown="True" w1048 {
                      tunnel: w1053 -> [w1059 w1069]
                      tunnel: [w1058 w1069] -> w1052
                      tunnel: w1051 -> [w1057 w1068]
                      tunnel: [w1056 w1068] -> w1050
                      tunnel: w1049 -> [w1055 _]
                      frame False {
                        # "If reason for stop is disabled,then SM will come \nout the Pause subVI.So error handling has to be done outside"
                        # "ReasonForStop Disabled"
                        n236 = Bundle By Name(cluster=w1055, "PopupInput.Title"="ALERT!" ("title"), "PopupInput.Message"="File Open!\nUnable To Write.Please Close Data File." ("string"), "PopupInput.Title Blink? T/F"=TRUE ("title blink?"), "PopupInput.Button 1 Text"="OK", "PopupInput.Pop-up Type"=T8."One button dialog box") -> (w1062:T2)
                        n237 = call "Output_SM.vi"("SM Private Data in"=w1057, "Output Cluster"=w1062, "Receiver Name"="UI", "State"="UI: DisplayPopup", "error in (no error)"=w1059) -> ("SM Private Data out"=w1056:refnum<class "Inspection Statemachine.lvclass">, "error out"=w1058:errorcluster)  [unwired: 9 in]
                      }
                      frame True {
                        # "If reason for stop is enabled,then SM will stay\ninside the Pause subVI.So error handling is done inside pause SubVI."
                        # "ReasonForStop Enabled"
                      }
                    }
                  }
                }
              }
              frame "InspectionSMError", "InspectionUIError", "RackControllerError" {
                # "RackControllerError_0xF500"
                n238 = Bundle By Name(cluster=w1090, "DirectExit"=FALSE ("Direct Exit"), "SoftwareExit"=TRUE ("Software Exit?")) -> (w1088:T1)
                n239 = Concatenate Strings("Error! \nRestart the System" ("string"), "\n" ("string"), "Error Code: " ("string"), w1085) -> (w1081:string)
                n240 = Bundle By Name(cluster=w1077, "PopupInput.Title"="ALERT!" ("title"), "PopupInput.Message"=w1081, "PopupInput.Title Blink? T/F"=TRUE ("title blink?"), "PopupInput.Button 1 Text"="OK", "PopupInput.Pop-up Type"=T8."One button dialog box") -> (w1072:T2)
                n241 = call "Output_SM.vi"("SM Private Data in"=w1078, "Output Cluster"=w1072, "Receiver Name"="UI", "State"="UI: DisplayPopup", "error in (no error)"=w1080) -> ("SM Private Data out"=w1070:refnum<class "Inspection Statemachine.lvclass">, "error out"=w1079:errorcluster)  [unwired: 9 in]
              }
              frame "CameraError", "CameraFailed" {
                n242 = Bundle By Name(cluster=w1111, "DirectExit"=FALSE ("Direct Exit"), "SoftwareExit"=TRUE ("Software Exit?")) -> (w1109:T1)
                n243 = Concatenate Strings("Hardware Error!\nRestart the System" ("string"), "\n" ("string"), "Error Code: " ("string"), w1106) -> (w1102:string)
                n244 = Bundle By Name(cluster=w1098, "PopupInput.Title"="ALERT!" ("title"), "PopupInput.Message"=w1102, "PopupInput.Title Blink? T/F"=TRUE ("title blink?"), "PopupInput.Button 1 Text"="OK", "PopupInput.Pop-up Type"=T8."One button dialog box") -> (w1094:T2)
                n245 = call "Output_SM.vi"("SM Private Data in"=w1099, "Output Cluster"=w1094, "Receiver Name"="UI", "State"="UI: DisplayPopup", "error in (no error)"=w1101) -> ("SM Private Data out"=w1091:refnum<class "Inspection Statemachine.lvclass">, "error out"=w1100:errorcluster)  [unwired: 9 in]
              }
              frame "Motor" {
                n246 = case shown="\"0x03000401\"" w1119 {
                  selector: w1119 -> [w1137 w1154 w1171 w1188]
                  tunnel: [w1127 w1145 w1162 w1179] -> w1121
                  tunnel: w1120 -> [w1128 w1146 w1163 w1180]
                  tunnel: w1118 -> [w1131 w1149 w1166 w1183]
                  tunnel: w1117 -> [w1123 w1141 w1158 w1175]
                  tunnel: [w1122 w1139 w1156 w1173] -> w1116
                  frame "0x03000401" {
                    n247 = Concatenate Strings("Guides Failed to reach 'Inspection' Position!\nRestart the System" ("string"), "\n" ("string"), "Error Code: " ("string"), w1137) -> (w1132:string)
                    n248 = Bundle By Name(cluster=w1131, "PopupInput.Title"="ALERT!" ("title"), "PopupInput.Message"=w1132, "PopupInput.Title Blink? T/F"=TRUE ("title blink?"), "PopupInput.Button 1 Text"="OK", "PopupInput.Pop-up Type"=T8."One button dialog box") -> (w1124:T2)
                    n249 = call "Output_SM.vi"("SM Private Data in"=w1123, "Output Cluster"=w1124, "Receiver Name"="UI", "State"="UI: DisplayPopup", "error in (no error)"=w1128) -> ("SM Private Data out"=w1122:refnum<class "Inspection Statemachine.lvclass">, "error out"=w1127:errorcluster)  [unwired: 9 in]
                  }
                  frame "0x03000201", "0x03000202", "0x03000203" {
                    n250 = Concatenate Strings("Guides Failed to Open!\nCheck Motor" ("string"), "\n" ("string"), "Error Code: " ("string"), w1154) -> (w1150:string)
                    n251 = Bundle By Name(cluster=w1149, "PopupInput.Title"="ALERT!" ("title"), "PopupInput.Message"=w1150, "PopupInput.Title Blink? T/F"=TRUE ("title blink?"), "PopupInput.Button 1 Text"="OK", "PopupInput.Pop-up Type"=T8."One button dialog box") -> (w1142:T2)
                    n252 = call "Output_SM.vi"("SM Private Data in"=w1141, "Output Cluster"=w1142, "Receiver Name"="UI", "State"="UI: DisplayPopup", "error in (no error)"=w1146) -> ("SM Private Data out"=w1139:refnum<class "Inspection Statemachine.lvclass">, "error out"=w1145:errorcluster)  [unwired: 9 in]
                  }
                  frame "0x03000400" {
                    n253 = Concatenate Strings("Guides Failed to reach 'Insert' Position!\nRestart the System" ("string"), "\n" ("string"), "Error Code: " ("string"), w1171) -> (w1167:string)
                    n254 = Bundle By Name(cluster=w1166, "PopupInput.Title"="ALERT!" ("title"), "PopupInput.Message"=w1167, "PopupInput.Title Blink? T/F"=TRUE ("title blink?"), "PopupInput.Button 1 Text"="OK", "PopupInput.Pop-up Type"=T8."One button dialog box") -> (w1159:T2)
                    n255 = call "Output_SM.vi"("SM Private Data in"=w1158, "Output Cluster"=w1159, "Receiver Name"="UI", "State"="UI: DisplayPopup", "error in (no error)"=w1163) -> ("SM Private Data out"=w1156:refnum<class "Inspection Statemachine.lvclass">, "error out"=w1162:errorcluster)  [unwired: 9 in]
                  }
                  frame Default {
                    n256 = Concatenate Strings("Hardware Error!\nRestart the System" ("string"), "\n" ("string"), "Error Code: " ("string"), w1188) -> (w1184:string)
                    n257 = Bundle By Name(cluster=w1183, "PopupInput.Title"="ALERT!" ("title"), "PopupInput.Message"=w1184, "PopupInput.Title Blink? T/F"=TRUE ("title blink?"), "PopupInput.Button 1 Text"="OK", "PopupInput.Pop-up Type"=T8."One button dialog box") -> (w1176:T2)
                    n258 = call "Output_SM.vi"("SM Private Data in"=w1175, "Output Cluster"=w1176, "Receiver Name"="UI", "State"="UI: DisplayPopup", "error in (no error)"=w1180) -> ("SM Private Data out"=w1173:refnum<class "Inspection Statemachine.lvclass">, "error out"=w1179:errorcluster)  [unwired: 9 in]
                  }
                }
                n259 = Bundle By Name(cluster=w1112, "DirectExit"=TRUE ("Direct Exit"), "SoftwareExit"=TRUE ("Software Exit?")) -> (w1113:T1)
              }
            }
            n260 = call <vilib>:"Add State(s) to Queue__JKI_lib_State_Machine.vi"("State(s) in (\"\")"=w923) -> ("States Out"=w924:string)  [unwired: 14 in]
          }
          event User Event {
            # "ActionOnPopup_SM event"
            n261 = event-data() -> ("ActionOnPopup_SM"=w1194:string)  [unwired: 1 in]
            n262 = Unbundle By Name(w1201) -> ("OutputCluster"=w1192:T2, "OutputCluster.SystemParameters.SoftwareFeatures.HardwareEmulated"=w1193:bool, "DirectExit"=w1197:bool, "CurrentState"=w1198:string, "OutputCluster.SystemParameters.SoftwareFeatures.DataLoggingEnable"=w1191:bool, "OutputCluster.SystemParameters.SoftwareFeatures.PopupOptions.ReasonForStop"=w1190:bool)
            n263 = case shown="\"Error\"" w1198 {
              tunnel: [w1207 w1216 w1245 "" "" "MoveToHomePosition" ""] -> w1202
              tunnel: w1196 -> [w1205 w1212 w1241 w1273 w1275 w1295 w1312]
              tunnel: w1200 -> [w1208 w1214 w1243 w1271 w1279 w1297 w1310]
              tunnel: [w1208 w1215 w1244 w1271 w1278 w1296 w1310] -> w1199
              tunnel: w1197 -> [w1206 _ _ _ _ _ _]
              tunnel: [w1205 w1212 w1241 w1273 w1274 w1294 w1312] -> w1195
              tunnel: w1194 -> [_ w1217 w1246 _ _ _ _]
              tunnel: w1193 -> [_ _ _ _ w1277 w1293 _]
              tunnel: w1192 -> [_ w1213 w1242 _ w1276 w1292 _]
              tunnel: w1191 -> [_ w1211 w1240 _ _ _ _]
              tunnel: w1190 -> [_ _ w1239 _ _ _ _]
              frame "Diagnostics" {
                n264 = case shown="True" w1206 {
                  tunnel: ["" "SoftwareExit"] -> w1207
                  frame False {
                    # "DirectExit FALSE"
                  }
                  frame True {
                    # "DirectExit TRUE"
                  }
                }
              }
              frame "SoftwareExit" {
                n265 = case shown="\"Exit Application\"" w1217 {
                  tunnel: ["" "CloseConfirm" "" "HomeReached"] -> w1216
                  tunnel: [w1218 w1220 w1226 w1237] -> w1215
                  tunnel: w1214 -> [w1218 w1220 w1227 w1237]
                  tunnel: w1213 -> [_ _ w1225 _]
                  tunnel: w1212 -> [_ _ w1223 _]
                  tunnel: w1211 -> [_ _ w1222 _]
                  frame "Cancel" {
                  }
                  frame "Continue", Default {
                  }
                  frame "OK" {
                    n266 = case shown="True" w1222 {
                      tunnel: w1227 -> [w1228 w1233]
                      tunnel: [w1228 w1232] -> w1226
                      tunnel: w1225 -> [_ w1230]
                      tunnel: w1223 -> [_ w1229]
                      frame False {
                        # "DL Disable"
                      }
                      frame True {
                        # "OK reply comes for\nerror pop up from DL\nwhen save is sent and \nfile is open during SoftwareExit"
                        # "DL Enable"
                        n267 = Bundle By Name(cluster=w1230, "StateMsgToDL"="Save" ("StateMsgToRC")) -> (w1236:T2)
                        n268 = call "Output_SM.vi"("SM Private Data in"=w1229, "Output Cluster"=w1236, "Receiver Name"="DL", "State"="DL: StateMessage", "error in (no error)"=w1233) -> ("error out"=w1232:errorcluster)  [unwired: 9 in, 1 out]
                      }
                    }
                  }
                  frame "Exit Application" {
                  }
                }
              }
              frame "Stop" {
                n269 = case shown="\"OK\"" w1246 {
                  tunnel: ["" ""] -> w1245
                  tunnel: [w1248 w1254] -> w1244
                  tunnel: w1243 -> [w1248 w1255]
                  tunnel: w1242 -> [_ w1253]
                  tunnel: w1241 -> [_ w1251]
                  tunnel: w1240 -> [_ w1250]
                  tunnel: w1239 -> [_ w1249]
                  frame Default {
                  }
                  frame "OK" {
                    n270 = case shown="False" w1249 {
                      tunnel: w1255 -> [w1260 w1270]
                      tunnel: [w1259 w1270] -> w1254
                      tunnel: w1253 -> [w1258 _]
                      tunnel: w1251 -> [w1257 _]
                      tunnel: w1250 -> [w1256 _]
                      frame False {
                        # "StopReasonDisabled"
                        n271 = case shown="False" w1256 {
                          tunnel: w1260 -> [w1261 w1266]
                          tunnel: [w1261 w1265] -> w1259
                          tunnel: w1258 -> [_ w1263]
                          tunnel: w1257 -> [_ w1262]
                          frame False {
                            # "DL Disable"
                          }
                          frame True {
                            # "OK reply comes for\nerror pop up from DL\nwhen Post is sent and \nfile is open during stop"
                            # "DL Enable"
                            n272 = Bundle By Name(cluster=w1263, "StateMsgToDL"="Post" ("StateMsgToRC")) -> (w1269:T2)
                            n273 = call "Output_SM.vi"("SM Private Data in"=w1262, "Output Cluster"=w1269, "Receiver Name"="DL", "State"="DL: StateMessage", "error in (no error)"=w1266) -> ("error out"=w1265:errorcluster)  [unwired: 9 in, 1 out]
                          }
                        }
                      }
                      frame True {
                        # "StopResaonEnabled"
                      }
                    }
                  }
                }
              }
              frame Default {
              }
              frame "Run" {
                n274 = case shown="False" w1277 {
                  tunnel: w1279 -> [w1289 w1290]
                  tunnel: [w1288 w1290] -> w1278
                  tunnel: w1275 -> [w1287 w1291]
                  tunnel: [w1286 w1291] -> w1274
                  tunnel: w1276 -> [w1285 _]
                  frame False {
                    # "Online"
                    n275 = Bundle By Name(cluster=w1285, "StateMsgToMI"="SelectionComplete") -> (w1284:T2)
                    n276 = call "Output_SM.vi"("SM Private Data in"=w1287, "Output Cluster"=w1284, "Receiver Name"="MI", "State"="MI: StateMessage", "error in (no error)"=w1289) -> ("SM Private Data out"=w1286:refnum<class "Inspection Statemachine.lvclass">, "error out"=w1288:errorcluster)  [unwired: 9 in]
                  }
                  frame True {
                  }
                }
              }
              frame "MasterSampleDiagnostics", "MasterSamplePOST" {
                n277 = case shown="False" w1293 {
                  tunnel: w1297 -> [w1304 w1309]
                  tunnel: w1292 -> [w1302 _]
                  tunnel: [w1299 w1308] -> w1294
                  tunnel: [w1303 w1309] -> w1296
                  tunnel: w1295 -> [w1300 w1308]
                  frame False {
                    # "Online execution"
                    n278 = Bundle By Name(cluster=w1302, "StateMsgToMI"="MasterSample") -> (w1305:T2)
                    n279 = call "Output_SM.vi"("SM Private Data in"=w1300, "Output Cluster"=w1305, "Receiver Name"="MI", "State"="MI: StateMessage", "error in (no error)"=w1304) -> ("SM Private Data out"=w1299:refnum<class "Inspection Statemachine.lvclass">, "error out"=w1303:errorcluster)  [unwired: 9 in]
                  }
                  frame True {
                    # "Offline execution"
                  }
                }
              }
              frame "Error" {
              }
            }
            n280 = call <vilib>:"Add State(s) to Queue__JKI_lib_State_Machine.vi"("State(s) in Front (\"\")"=w1202, "State(s) in (\"\")"=w1203) -> ("States Out"=w1204:string)  [unwired: 13 in]
          }
          event User Event {
            # "PartInfo_SM"
            n281 = event-data() -> ("RackID"=w1322:u8, "MeasurementIDsArray"=w1321:u16[], "MeasurementNamesArray"=w1320:string[], "SpecValuesArray"=w1319:T14, "CameraNamesArray"=w1318:string[])  [unwired: 1 in, 1 out]
            n282 = Unbundle By Name(w1313) -> ("UpdateInPause"=w1315:bool)
            n283 = Not(x=w1315) -> (.not. x?=w1314:bool)
            n284 = Bundle By Name(cluster=w1313, "OutputCluster.RackID"=w1322, "OutputCluster.PartInfo.Reinitialize"=w1314, "OutputCluster.PartInfo.MeasurementIDArray"=w1321, "OutputCluster.PartInfo.MeasurementNamesArray"=w1320, "OutputCluster.PartInfo.SpecValuesArray"=w1319, "OutputCluster.PartInfo.CameraNamesArray"=w1318) -> (w1317:T1)
            n285 = in-place {
              in-place-border: [w1330] -> w1323
              n286 = in-place-cluster #3(w1317) -> ("SelComplete"=w1328:bool)
              n287 = Select(t=w1328, s=w1328, f=TRUE ("SelComplete")) -> (s? t:f=w1329:bool)
              n288 = Select(t="SendPartDetails" ("State(s) in Front (\"\")"), s=w1328, f="Wait" ("State(s) in Front (\"\")")) -> (s? t:f=w1330:string)
              n289 = in-place-cluster #3("SelComplete"=w1329) -> (w1316:T1)
            }
            n290 = call <vilib>:"Add State(s) to Queue__JKI_lib_State_Machine.vi"("State(s) in Front (\"\")"=w1323, "State(s) in (\"\")"=w1326) -> ("States Out"=w1327:string)  [unwired: 13 in]
          }
          event User Event {
            # "InitiateCameraOpticsDiagnostics_SM event"
            n291 = event-data() -> ("CameraName"=w1343:string)  [unwired: 1 in]
            n292 = Bundle By Name(cluster=w1335, "OutputCluster.Camera Name"=w1343, "CurrentState"="CameraOpticsDiagnostics") -> (w1342:T1)
            n293 = Unbundle By Name(w1335) -> ("OutputCluster.Trigger Light Camera Sequence.Status"=w1334:string)
            n294 = case "To Turn Off the Status of Previous Camera" shown="\"On\"" w1334 {
              tunnel: [w1346 w1356] -> w1336
              tunnel: w1337 -> [w1346 w1355]
              tunnel: w1339 -> [w1347 w1354]
              tunnel: [w1347 w1353] -> w1338
              tunnel: w1335 -> [_ w1350]
              frame "Off", Default {
              }
              frame "On" {
                # "Turn Off If the Status is ON"
                n295 = Bundle By Name(cluster=w1350, "OutputCluster.Trigger Light Camera Sequence.Status"="Off", "OutputCluster.Trigger Light Camera Sequence.Mode"="") -> (w1357:T1)
                n296 = Unbundle By Name(w1357) -> ("OutputCluster.SystemParameters.SoftwareFeatures.HardwareEmulated"=w1352:bool, "OutputCluster"=w1351:T2)
                n297 = call "Output_SM.vi"("SM Private Data in"=w1354, "Output Cluster"=w1351, "Receiver Name"="SingleRack", "State"="RC: CameraOpticsDiagnostics", "error in (no error)"=w1355) -> ("SM Private Data out"=w1361:refnum<class "Inspection Statemachine.lvclass">, "error out"=w1360:errorcluster)  [unwired: 9 in]
                n298 = case shown="False" w1352 {
                  tunnel: w1361 -> [w1363 w1370]
                  tunnel: w1360 -> [w1362 w1369]
                  tunnel: [w1362 w1366] -> w1356
                  tunnel: [w1363 w1365] -> w1353
                  tunnel: w1351 -> [_ w1364]
                  frame True {
                    # "Offline execution"
                  }
                  frame False {
                    # "Online execution"
                    n299 = call "Output_SM.vi"("SM Private Data in"=w1370, "Output Cluster"=w1364, "Receiver Name"="MI", "State"="MI: CameraOpticsDiagnostics", "error in (no error)"=w1369) -> ("SM Private Data out"=w1365:refnum<class "Inspection Statemachine.lvclass">, "error out"=w1366:errorcluster)  [unwired: 9 in]
                  }
                }
              }
            }
            n300 = call <vilib>:"Add State(s) to Queue__JKI_lib_State_Machine.vi"("State(s) in Front (\"\")"="ObtainCameraIndex" ("State(s) in Front (\"\")"), "State(s) in (\"\")"=w1344) -> ("States Out"=w1345:string)  [unwired: 13 in]
          }
          event User Event {
            # "CallLoadingBar_SM"
            n301 = event-data() -> ("Pop-up Type"=w1385:T8, "Title"=w1384:string, "Message"=w1383:string, "Button 1 Text"=w1382:string, "Button 2 Text"=w1381:string, "Show Close? T/F"=w1380:bool, "Title Blink? T/F"=w1379:bool, "Title Blink Colour"=w1378:u32)  [unwired: 1 in]
            n302 = Unbundle By Name(w1387) -> ("OutputCluster"=w1386:T2)
            n303 = Bundle By Name(cluster=w1386, "PopupInput.Pop-up Type"=w1385, "PopupInput.Title"=w1384, "PopupInput.Message"=w1383, "PopupInput.Button 1 Text"=w1382, "PopupInput.Button 2 Text"=w1381, "PopupInput.Show Close? T/F"=w1380, "PopupInput.Title Blink? T/F"=w1379, "PopupInput.Title Blink Colour"=w1378) -> (w1377:T2)
            n304 = call "Output_SM.vi"("SM Private Data in"=w1372, "Output Cluster"=w1377, "Receiver Name"="UI", "State"="UI: DisplayPopup", "error in (no error)"=w1374) -> ("SM Private Data out"=w1371:refnum<class "Inspection Statemachine.lvclass">, "error out"=w1373:errorcluster)  [unwired: 9 in]
            n305 = call <vilib>:"Add State(s) to Queue__JKI_lib_State_Machine.vi"("State(s) in (\"\")"=w1388) -> ("States Out"=w1389:string)  [unwired: 14 in]
          }
          event User Event {
            # "CallLoadingBar_SM"
            n306 = event-data() -> ("AllPartInfo"=w1396:T15)  [unwired: 1 in]
            n307 = Unbundle By Name(w1398) -> ("OutputCluster.SystemParameters.SoftwareFeatures.DataLoggingEnable"=w1390:bool, "OutputCluster"=w1392:T2)
            n308 = Bundle By Name(cluster=w1392, "AllPartInfo"=w1396) -> (w1395:T2)
            n309 = case shown="True" w1390 {
              tunnel: w1397 -> [w1402 w1414]
              tunnel: w1395 -> [_ w1413]
              tunnel: w1394 -> [w1401 w1412]
              tunnel: [w1402 w1410] -> w1391
              tunnel: [w1401 w1408] -> w1393
              tunnel: w1392 -> [_ w1407]
              frame False {
                # "DL Disable"
              }
              frame True {
                # "DL Enable"
                n310 = call "Output_SM.vi"("SM Private Data in"=w1412, "Output Cluster"=w1413, "Receiver Name"="DL", "State"="DL: AllPartInfo", "error in (no error)"=w1414) -> ("SM Private Data out"=w1409:refnum<class "Inspection Statemachine.lvclass">, "error out"=w1411:errorcluster)  [unwired: 9 in]
                n311 = Bundle By Name(cluster=w1407, "StateMsgToDL"="Post") -> (w1404:T2)
                n312 = call "Output_SM.vi"("SM Private Data in"=w1409, "Output Cluster"=w1404, "Receiver Name"="DL", "State"="DL: StateMessage", "error in (no error)"=w1411) -> ("SM Private Data out"=w1408:refnum<class "Inspection Statemachine.lvclass">, "error out"=w1410:errorcluster)  [unwired: 9 in]
              }
            }
            n313 = call <vilib>:"Add State(s) to Queue__JKI_lib_State_Machine.vi"("State(s) in (\"\")"=w1399) -> ("States Out"=w1400:string)  [unwired: 14 in]
          }
          event User Event {
            # "CameraOpticsDiagnosticsResult_SM event"
            n314 = event-data() -> ("LightCameraName"=w1423:string, "DiagnosedImage"=w1424:T4, "DustPercentage"=w1425:dbl, "Result"=w1426:bool)  [unwired: 1 in]
            n315 = Bundle By Name(cluster=w1419, "OutputCluster.CameraOpticsDiagnosticsResult.LightCameraName"=w1423, "OutputCluster.CameraOpticsDiagnosticsResult.DiagnosedImage"=w1424, "OutputCluster.CameraOpticsDiagnosticsResult.DustPercentage"=w1425, "OutputCluster.CameraOpticsDiagnosticsResult.Result"=w1426) -> (w1418:T1)
            n316 = Unbundle By Name(w1418) -> ("CameraOpticsDiagnosticsStatus"=w1417:bool)
            n317 = case shown="False" w1417 {
              tunnel: ["" "CameraOpticsAnalysis" ("State(s) in Front (\"\")")] -> w1422
              frame False {
              }
              frame True {
              }
            }
            n318 = call <vilib>:"Add State(s) to Queue__JKI_lib_State_Machine.vi"("State(s) in Front (\"\")"=w1422, "State(s) in (\"\")"=w1427) -> ("States Out"=w1428:string)  [unwired: 13 in]
          }
          event User Event {
            # "SelectedPart_SM event"
            n319 = event-data() -> ("PartName"=w1434:string, "ConnectorsInReel"=w1435:u64, "TotalCount"=w1436:u64, "OperatorName"=w1437:string, "StampingMachineID"=w1438:u8)  [unwired: 1 in]
            n320 = Flush Event Queue(0:w1431, 3:w1433) -> (11:w1432:errorcluster)  [unwired: 4 in, 2 out]
            n321 = Bundle By Name(cluster=w1442, "CurrentState"="Select" ("Previous State"), "OutputCluster.PartInfo.PartName"=w1434, "OutputCluster.PartInfo.ReelCount"=w1435, "OutputCluster.PartInfo.TotalCount"=w1436, "OutputCluster.PartInfo.OperatorName"=w1437, "OutputCluster.PartInfo.StampingMachineID"=w1438) -> (w1441:T1)
            n322 = call <vilib>:"Add State(s) to Queue__JKI_lib_State_Machine.vi"("State(s) in Front (\"\")"="SendPartName" ("State(s) in Front (\"\")"), "State(s) in (\"\")"=w1444) -> ("States Out"=w1445:string)  [unwired: 13 in]
          }
          event User Event {
            # "HardwareActionAck_SM event"
            n323 = event-data() -> ("HardwareActionAck"=w1447:string)  [unwired: 1 in]
            n324 = call <vilib>:"Add State(s) to Queue__JKI_lib_State_Machine.vi"("State(s) in Front (\"\")"=w1447, "State(s) in (\"\")"=w1450) -> ("States Out"=w1449:string)  [unwired: 13 in]
          }
          event User Event {
            # "ButtonPressed_SM event"
            n325 = event-data() -> ("ButtonPress"=w1457:string)  [unwired: 1 in]
            n326 = Unbundle By Name(w1461) -> ("OutputCluster.SystemParameters.SoftwareFeatures.DataLoggingEnable"=w1453:bool, "Exit"=w1463:bool, "LoadingBarActive"=w1460:bool, "OutputCluster"=w1454:T2, "OutputCluster.SystemParameters.SoftwareFeatures.HardwareEmulated"=w1452:bool)
            n327 = case shown="\"SaveAck\"" w1457 {
              selector: w1457 -> [w1470 _ w1487 w1510 _]
              tunnel: [w1470 "" w1488 w1511 "SendPartName"] -> w1464
              tunnel: w1463 -> [_ _ w1489 w1512 _]
              tunnel: [w1469 w1472 w1486 w1509 w1543] -> w1462
              tunnel: w1461 -> [w1469 w1472 w1485 w1508 w1544]
              tunnel: w1460 -> [_ _ _ w1507 _]
              tunnel: w1459 -> [w1468 w1478 w1484 w1506 w1548]
              tunnel: [w1468 w1477 w1484 w1505 w1541] -> w1458
              tunnel: w1456 -> [w1467 w1476 w1483 w1504 w1545]
              tunnel: [w1467 w1475 w1483 w1503 w1540] -> w1455
              tunnel: w1454 -> [_ w1473 _ _ w1546]
              tunnel: w1453 -> [_ _ w1482 _ _]
              tunnel: w1452 -> [_ _ _ _ _]
              frame Default {
              }
              frame "DisableUIButtons" {
                n328 = Bundle By Name(cluster=w1473, "StateMsgToUI"="DisableAllButtons") -> (w1480:T2)
                n329 = call "Output_SM.vi"("SM Private Data in"=w1476, "Output Cluster"=w1480, "Receiver Name"="UI", "State"="UI: StateMessage", "error in (no error)"=w1478) -> ("SM Private Data out"=w1475:refnum<class "Inspection Statemachine.lvclass">, "error out"=w1477:errorcluster)  [unwired: 9 in]
              }
              frame "ExitApplication" {
                n330 = case shown="True" w1482 {
                  tunnel: w1489 -> [_ w1496]
                  tunnel: ["ExitApplication" w1495] -> w1488
                  tunnel: w1487 -> [_ w1494]
                  tunnel: [w1490 w1493] -> w1486
                  tunnel: w1485 -> [w1490 w1492]
                  frame False {
                    # "Dont wait for SaveACK from DL"
                    # "DL Disabled"
                  }
                  frame True {
                    # "DL Enabled"
                    n331 = case shown="True" w1496 {
                      tunnel: ["Wait" "ExitApplication"] -> w1495
                      tunnel: w1494 -> [_ _]
                      tunnel: [w1499 w1502] -> w1493
                      tunnel: w1492 -> [w1498 w1502]
                      frame False {
                        # "SaveAck not received yet"
                        n332 = Bundle By Name(cluster=w1498, "Exit"=TRUE) -> (w1499:T1)
                      }
                      frame True {
                        # "SaveAck received"
                      }
                    }
                  }
                }
              }
              frame "SaveAck" {
                n333 = case shown="True" w1512 {
                  tunnel: ["Wait" "ExitApplication"] -> w1511
                  tunnel: w1510 -> [_ _]
                  tunnel: [w1517 w1520] -> w1509
                  tunnel: w1508 -> [w1516 w1523]
                  tunnel: w1507 -> [_ w1526]
                  tunnel: w1506 -> [w1514 w1525]
                  tunnel: [w1514 w1524] -> w1505
                  tunnel: w1504 -> [w1513 w1522]
                  tunnel: [w1513 w1519] -> w1503
                  frame False {
                    # "ExitApplication is not received yet"
                    n334 = Bundle By Name(cluster=w1516, "Exit"=TRUE) -> (w1517:T1)
                  }
                  frame True {
                    # "ExitApplication received"
                    n335 = case shown="True" w1526 {
                      tunnel: w1525 -> [w1528 w1536]
                      tunnel: [w1528 w1535] -> w1524
                      tunnel: w1523 -> [w1529 w1532]
                      tunnel: w1522 -> [w1527 w1533]
                      tunnel: [w1529 w1532] -> w1520
                      tunnel: [w1527 w1530] -> w1519
                      frame False {
                      }
                      frame True {
                        n336 = Unbundle By Name(w1532) -> ("OutputCluster"=w1534:T2)
                        n337 = Bundle By Name(cluster=w1534, "PopupInput.Pop-up Type"=T8."Close Loading Bar" ("LoadingBarInput.Pop-up Type")) -> (w1538:T2)
                        n338 = call "Output_SM.vi"("SM Private Data in"=w1533, "Output Cluster"=w1538, "Receiver Name"="UI", "State"="UI: DisplayPopup", "error in (no error)"=w1536) -> ("SM Private Data out"=w1530:refnum<class "Inspection Statemachine.lvclass">, "error out"=w1535:errorcluster)  [unwired: 9 in]
                      }
                    }
                  }
                }
              }
              frame "MasterSampleDiagnostics" {
                n339 = Bundle By Name(cluster=w1546, "StateMsgToUI"="InitializeMasterSample") -> (w1542:T2)
                n340 = Bundle By Name(cluster=w1544, "CurrentState"="MasterSampleDiagnostics", "MasterSampleState"="MS:OkValidation" ("CurrentState")) -> (w1543:T1)
                n341 = call "Output_SM.vi"("SM Private Data in"=w1545, "Output Cluster"=w1542, "Receiver Name"="UI", "State"="UI: StateMessage", "error in (no error)"=w1548) -> ("SM Private Data out"=w1540:refnum<class "Inspection Statemachine.lvclass">, "error out"=w1541:errorcluster)  [unwired: 9 in]
              }
            }
            n342 = call <vilib>:"Add State(s) to Queue__JKI_lib_State_Machine.vi"("State(s) in Front (\"\")"=w1464, "State(s) in (\"\")"=w1466) -> ("States Out"=w1465:string)  [unwired: 13 in]
          }
          event "Software Exit": Value Change {
            # "Software Exit Button press from\nInspection Statemachine Front Panel"
            # "Software Exit Value change event"
            n343 = event-data() -> ()  [unwired: 1 in, 6 out]
            n344 = call <vilib>:"Add State(s) to Queue__JKI_lib_State_Machine.vi"("State(s) in Front (\"\")"="ExitApplication" ("State(s) in Front (\"\")"), "State(s) in (\"\")"=w1558) -> ("States Out"=w1557:string)  [unwired: 13 in]
          }
          event Panel Close? {
            # "Discard the event because we'll close the front panel ourselves in Macro: Exit"
            # "Close Panel button (pressed) Event\n(this executes Macro: Exit to terminate the VI)"
            # "Panel Close?"
            n345 = event-data() -> ()  [unwired: 1 in, 1 out]
            n346 = call <vilib>:"Add State(s) to Queue__JKI_lib_State_Machine.vi"("State(s) in Front (\"\")"="Macro: Exit", "State(s) in (\"\")"=w1566) -> ("States Out"=w1565:string)  [unwired: 13 in]
            n347 = event-data("Discard?"=TRUE) -> ()  [unwired: 1 in, 1 out]
          }
        }
      }
      frame "---------- Core ----------" {
        # "Do not put any code in this frame.\n(it is a separator no-op)"
        n348 = call <vilib>:"Add State(s) to Queue__JKI_lib_State_Machine.vi"("State(s) in (\"\")"=w1571) -> ("States Out"=w1570:string)  [unwired: 14 in]
      }
      frame Default {
        w1582 = 42 items=["No error", "Argument error", "Memory is full", "Out of zone", "End of file", "File already open", "Generic file I/O error", "File not found", "File permission error", "Disk is full", "Duplicate path", "Too many files open", "System feature not enabled", "Resource file not found", "Cannot add resource", "Resource not found", "Image not found", "Image memory error", "Pen does not exist", "Config type invalid", "Config token not found", "Config parse error", "Config memory error", "Bad external code format", "Bad external code offset", "External code not present", "Null window", "Destroy window error", "Null menu", "Print aborted", "Bad print record", "Print driver error", "Windows error during printing", "Memory error during printing", "Print dialog error", "Generic print error", "Invalid device refnum", "Device not found", "Device parameter error", "Device unit error", "Cannot open device", "Device call aborted", "Generic error", "Cancelled by user", "Object ID too low", "Object ID too high", "Object not in heap", "Unknown heap", "Unknown object (invalid DefProc)", "Unknown object (DefProc not in table)", "Message out of range", "Invalid (null) method", "Unknown message", "Manager call not supported", "Bad address", "Network operation in progress", "Network operation timed out", "Connection is busy", "Network attribute not supported", "Network error", "Address in use", "System out of memory", "Connection aborted", "Connection refused", "Not connected", "Already connected", "Connection closed", "Initialization error (interapplication manager)", "Bad occurrence", "Wait on unbound occurrence handler", "Occurrence queue overflow", "Datalog type conflict", "Unused", "Unrecognized type (interapplication manager)", "Memory corrupt", "Failed to make temporary DLL", "Old CIN version", "Drag socket not found", "Failed to load drop-object", "Failed to register OLE object", "Failed to release OLE object", "Format specifier type mismatch", "Unknown format specifier", "Too few format specifiers", "Too many format specifiers", "Scan failed", "Newer CIN version", "Error converting to variant", "Runtime menu error", "Password tampered", "Variant attribute not found", "Incompatible variant data type", "Event data is not available", "Event Store is not present", "Occurrence is not found", "Event Queue is not created", "Event info is not available", "Refnum passed is NULL", "Error retrieving Class GUID", "Error retrieving CoClass GUID", "Error retrieving TypeLib GUID.", "Bad built application magic bytes.", "Specific driver is different from the specific driver associated with the Logical Name.", "There is no session opened to the class driver.", "Max Error", "MAX - Error with config objects", "MAX - Error loading configuration", "MAX - Group not supported"]
        # "Current State"
        # "Do not delete, rename, or modify this frame.\n(this is used to capture unhandled states and typos)"
        # "Handle mistyped state name (developer tool)"
        n349 = Format Into String(format string="Software Exception: Unhandled State \"%s\"." ("message"), error in=w1578, w1573) -> (resulting string=w1581:string, error out=w1580:errorcluster)  [unwired: 1 in]
        n350 = call <vilib>:"Error Cluster From Error Code.vi"("show call chain? (False)"=TRUE, "error in (no error)"=w1580, "error message (\"\")"=w1581, "error code (0)"=w1582) -> ("error out"=w1579:errorcluster)  [unwired: 5 in]
        n351 = call <vilib>:"Add State(s) to Queue__JKI_lib_State_Machine.vi"("State(s) in (\"\")"=w1577) -> ("States Out"=w1576:string)  [unwired: 14 in]
      }
      frame "Initialize Core Data" {
        # "Do not delete, rename, or modify this frame.\n(this is used to determine panel behavior on exit)"
        # "originally closed?"
        # "exe?"
        # "If panel starts closed or is an EXE, then close it when we exit"
        n352 = property class="VI"() -> ("Front Panel.Open"=w1592:bool)  [unwired: 2 in, 2 out]
        n353 = property class="App"() -> ("App.Kind"=w1591:T9)  [unwired: 2 in, 2 out]
        n354 = control-ref of="Current VI Reference"() -> (w1585:refnum<vi>)
        n355 = Not(x=w1592) -> (.not. x?=w1589:bool)
        n356 = Equal?(x=w1591, y=T9."Run Time System" ("Application:Kind")) -> (x = y?=w1588:bool)
        n357 = Or(x=w1589, y=w1588) -> (x .or. y?=w1586:bool)
        n358 = Bundle By Name(cluster=w1587, "Core.Current VI Reference"=w1585, "Core.Close Panel on Exit?"=w1586) -> (w1594:T1)
        n359 = call <vilib>:"Add State(s) to Queue__JKI_lib_State_Machine.vi"("State(s) in (\"\")"=w1596) -> ("States Out"=w1595:string)  [unwired: 14 in]
      }
      frame "Error Handler" {
        # "Handle any errors here.\nYou can also output any states to clean-up after errors occur"
        # "Clear error"
        n360 = Unbundle By Name(w1606) -> ("code"=w1605:i32)
        n361 = Number To Decimal String(number=w1605) -> (decimal integer string=w1604:string)  [unwired: 1 in]
        n362 = call <vilib>:"Read Self Enqueuer.vi"("Actor"=w1609) -> ("Self Enqueuer"=w1608:refnum<class "Message Enqueuer.lvclass">)  [unwired: 10 in]
        n363 = Concatenate Strings("InspectionSMError_0xF000" ("Error Message"), w1604) -> (w1603:string)
        n364 = call "Send ErrorMessage_SM.vi"("Error Message"=w1603, "Message Enqueuer"=w1608) -> ()  [unwired: 8 in, 2 out]
        n365 = Bundle By Name(cluster=w1599, "CurrentState"="Error handler" ("Previous State"), "SoftwareExit"=TRUE ("Software Exit?")) -> (w1598:T1)
        n366 = call <vilib>:"Add State(s) to Queue__JKI_lib_State_Machine.vi"("State(s) in Front (\"\")"="/* Post Error States", "State(s) in (\"\")"=w1611) -> ("States Out"=w1610:string)  [unwired: 13 in]
      }
      frame "Exit" {
        # "Do not put any code in this frame.\n(No errors that occur here will be handled.)"
        n367 = call <vilib>:"Add State(s) to Queue__JKI_lib_State_Machine.vi"("State(s) in (\"\")"=w1617) -> ("States Out"=w1616:string)  [unwired: 14 in]
      }
      frame "---------- Data ----------" {
        # "Do not put any code in this frame.\n(It is a separator no-op. You can make a copy of this frame to create a new Data frame)"
        n368 = call <vilib>:"Add State(s) to Queue__JKI_lib_State_Machine.vi"("State(s) in (\"\")"=w1622) -> ("States Out"=w1621:string)  [unwired: 14 in]
      }
      frame "Data: Initialize" {
        w1625 = 0  # SensorIndex
        w1630 = 0  # CameraIndex
        w1631 = FALSE  # CameraOpticsDiagnosticsStatus
        w1634 = FALSE  # PopUpActive
        w1635 = ""  # PopUpCategory
        w1636 = ""  # EventReason
        w1637 = FALSE  # UpdateInPause
        w1639 = TRUE  # LoadingBarActive
        w1640 = TRUE  # BatchStart
        w1641 = u8 1  # NumberOfActorsLaunched
        w1623 = FALSE  # Exit
        w1642 = FALSE  # ResultToMI
        w1643 = FALSE  # SelComplete
        w1649 = T2 {"RackID"=0, "Trigger Light Camera Sequence"={"Light Sequence Trigger"="", "Status"="", "Mode"=""}, "Result Cluster"={"RackID"=0, "MeasurementValuesArray "=[], "ImagesArray"=[], "ResultPF"=FALSE, "ProductionCountDetails"={"TotalFail"=0, "TotalPass"=0, "TotalCount"=0}, "ReelCountDetails"={"ReelFail"=0, "ReelPass"=0, "ReelCount"=0}, "ControlPFArray"=[], "SpecificationPFArray"=[], "SpecificationFail"=FALSE, "ReelNumber"=1, "Status"=""}, "Analytics VI refnum"=refnum, "Statistical parameters "=[], "Sensor Name"="", "Camera Name"="", "PopupInput"={"Pop-up Type"=enum."Open Logo Display", "Title"="", "Message"="", "Button 1 Text"="", "Button 2 Text"="", "Show Close? T/F"=FALSE, "Title Blink? T/F"=FALSE, "Title Blink Colour"=0}, "PartInfo"={"PartName"="", "NumberOfRacks"=0, "TotalCount"=0, "ReelCount"=0, "OperatorName"="", "StampingMachineID"=0, "RackID"=0, "Reinitialize"=FALSE, "MeasurementNamesArray"=[], "MeasurementIDArray"=[], "SpecValuesArray"=[], "CameraNamesArray"=[]}, "StateMsgToMI"="", "InspectionStatusToMI"="", "StateMsgToRC"="", "StateMsgToUI"="", "StateMsgToDL"="", "StateMsgToAN"="", "StateMsgToSM"="", "EventData"={"EventName"="", "EventReason"=""}, "CameraOpticsDiagnosticsResult"={"LightCameraName"="", "DiagnosedImage"=refnum, "DustPercentage"=0.0, "Result"=TRUE}, "AllPartInfo"=[{"PartName"="", "NumberOfRacks"=0, "MeasurementIDsArray"=[], "MeasurementNamesArray"=[], "SpecValuesArray"=[]}], "SystemParameters"={"SystemName"="", "SystemID"="", "CustomerDetails"={"CustomerName"="", "CustomerId"="", "Location"="", "NumberOfShifts"=0.0, "ShiftDetails"=[]}, "InstallationDate"="", "NextServiceDate"="", "NumberOfRacks"=0, "TotalNumberOfCameras"=0, "SoftwareFeatures"={"HardwareEmulated"=FALSE, "PowerOnSelfTest"=FALSE, "DiagnosticsEnable"=FALSE, "AnalyticsEnable"=FALSE, "DefectTrackingEnable"=FALSE, "AutomaticGuideMovement"=FALSE, "DoorPokayokeEnable"=FALSE, "FailCountDisplayEnable"=FALSE, "FailCountReversalEnable"=FALSE, "DataLoggingEnable"=FALSE, "PauseOnReelCountFinish"=FALSE, "StopOnTotalCountFinish"=FALSE, "IoTEnable"=FALSE, "ReportEnable"=FALSE, "DebugLevel"=0.0, "PowerOnSelfTestFeatures"={"TimingUnit"=FALSE, "MachinePowerStatusCheck"=FALSE, "GuideMotor"=FALSE, "CameraOptics"=FALSE, "MasterSample"=FALSE}, "DiagnosticsFeatures"={"TimingUnit"=FALSE, "GuideMotor"=FALSE, "CameraOptics"=FALSE, "ReelerMotor"=FALSE, "HardwareButtons"=FALSE, "Sensors"=FALSE, "TowerLamp"=FALSE, "MasterSample"=FALSE}, "UserInterface"={"DynamicImageHandlingEnable"=FALSE, "DoorPokaYokeButtonVisible"=FALSE, "FailCountDisplayButtonVisible"=FALSE, "FailCountReversalButtonVisible"=FALSE}, "PopupOptions"={"ReasonForPause"=FALSE, "ReasonForFail"=FALSE, "ReasonForStop"=FALSE, "CpCpkOnReelFinish"=FALSE}, "DataloggingFeatures"={"EventData"=FALSE, "MeasurementData"=FALSE, "StatisticalData"=FALSE, "ReelData"=FALSE, "FailedMeasurementData"=FALSE, "FailedImages"=FALSE}, "IoT"={"SMSAlertEnable"=FALSE, "EmailAlertEnable"=FALSE}}}, "PartsConfigured"=[], "CameraSequenceList"=[], "SensorList"=[], "MasterSampleMessages"={"MasterSampleMessage"="", "PartMessage"=""}, "SensorDiagnosticsResult"={"Image Array"=[], "ImageCount"=0}, "IgnoredCountDetails"={"ReelCount"=0, "TotalCount"=0}, "MachineStatusToDL"="", "MasterSamplePartName"=""}  # OutputCluster
        w1644 = FALSE  # SensorDiagnosticsStatus
        w1645 = FALSE  # SoftwareExit
        w1646 = FALSE  # DirectExit
        w1647 = ""  # CurrentState
        w1651 = -1  # Timeout
        w1648 = u8 0  # Ack
        w1660 = T16 {"Current VI Reference"=refnum, "Close Panel on Exit?"=FALSE}  # Core
        # "PopUpCategory: Name of the PopUp dislayed."
        # "PopUpActive:\nTrue: PopUp Active on UI.\nFalse: No PopUp being displayed currently."
        # "Exits the SM only when it receives Ack from both MI and DL.\nTrue=Both ack received.\nFalse=Either one or no Ack received."
        # "Checks whether the previous result was pass or fail.\nTrue=Pass\nFalse=Fail"
        # "Initialize the shift-register data, here.\n(data names are defined by what you wire into the bundle function)"
        n369 = Unbundle By Name(w1658) -> ("GtronSystemJSONDefault"=w1657:path, "GtronSystemJSONOverride"=w1656:path)
        n370 = call "ReadSystemParameters_SM.vi"("error in (no error)"=w1659, "Override File Path"=w1656, "Default File Path"=w1657) -> ("error out"=w1655:errorcluster, "System Parameters"=w1627:T17)  [unwired: 6 in]
        n371 = Unbundle(w1627) -> ("SystemParameters"=w1629:T18, "PartsConfigured"=w1632:cluster{"Name":string, "NumberOfRack":u8}[], "CameraSequenceList"=w1628:cluster{"Name":string, "RackID":u8}[], "SensorList"=w1626:cluster{"Name":string, "RackID":u8}[])  [unwired: 1 out]
        n372 = Unbundle By Name(w1629) -> ("SoftwareFeatures.HardwareEmulated"=w1633:bool)
        n373 = Bundle By Name(cluster=w1649, "SystemParameters"=w1629, "PartsConfigured"=w1632, "Result Cluster.ReelNumber"=u64 1, "CameraSequenceList"=w1628, "SensorList"=w1626) -> (w1624:T2)
        n374 = Select(t="UI: Front Panel State >> Open\nLaunchChildActors" ("State(s) in Front (\"\")"), s=w1633, f="UI: Front Panel State >> Close\nLaunchChildActors" ("State(s) in Front (\"\")")) -> (s? t:f=w1652:string)
        n375 = call <vilib>:"Add State(s) to Queue__JKI_lib_State_Machine.vi"("State(s) in (\"\")"=w1663, "State(s) at Back (\"\")"=w1652) -> ("States Out"=w1662:string)  [unwired: 13 in]
        n376 = Bundle(cluster=T1 {"Timeout"=0, "Core"={"Current VI Reference"=refnum, "Close Panel on Exit?"=FALSE}, "Ack"=0, " CurrentState"="", "DirectExit"=FALSE, "SoftwareExit"=FALSE, "SensorDiagnosticsStatus"=FALSE, "OutputCluster"={"RackID"=0, "Trigger Light Camera Sequence"={"Light Sequence Trigger"="", "Status"="", "Mode"=""}, "Result Cluster"={"RackID"=0, "MeasurementValuesArray "=[], "ImagesArray"=[], "ResultPF"=FALSE, "ProductionCountDetails"={"TotalFail"=0, "TotalPass"=0, "TotalCount"=0}, "ReelCountDetails"={"ReelFail"=0, "ReelPass"=0, "ReelCount"=0}, "ControlPFArray"=[], "SpecificationPFArray"=[], "SpecificationFail"=FALSE, "ReelNumber"=0, "Status"=""}, "Analytics VI refnum"=refnum, "Statistical parameters "=[], "Sensor Name"="", "Camera Name"="", "PopupInput"={"Pop-up Type"=enum."Open Logo Display", "Title"="", "Message"="", "Button 1 Text"="", "Button 2 Text"="", "Show Close? T/F"=FALSE, "Title Blink? T/F"=FALSE, "Title Blink Colour"=0}, "PartInfo"={"PartName"="", "NumberOfRacks"=0, "TotalCount"=0, "ReelCount"=0, "OperatorName"="", "StampingMachineID"=0, "RackID"=0, "Reinitialize"=FALSE, "MeasurementNamesArray"=[], "MeasurementIDArray"=[], "SpecValuesArray"=[], "CameraNamesArray"=[]}, "StateMsgToMI"="", "InspectionStatusToMI"="", "StateMsgToRC"="", "StateMsgToUI"="", "StateMsgToDL"="", "StateMsgToAN"="", "StateMsgToSM"="", "EventData"={"EventName"="", "EventReason"=""}, "CameraOpticsDiagnosticsResult"={"LightCameraName"="", "DiagnosedImage"=refnum, "DustPercentage"=0.0, "Result"=FALSE}, "AllPartInfo"=[], "SystemParameters"={"SystemName"="", "SystemID"="", "CustomerDetails"={"CustomerName"="", "CustomerId"="", "Location"="", "NumberOfShifts"=0.0, "ShiftDetails"=[]}, "InstallationDate"="", "NextServiceDate"="", "NumberOfRacks"=0, "TotalNumberOfCameras"=0, "SoftwareFeatures"={"HardwareEmulated"=FALSE, "PowerOnSelfTest"=FALSE, "DiagnosticsEnable"=FALSE, "AnalyticsEnable"=FALSE, "DefectTrackingEnable"=FALSE, "AutomaticGuideMovement"=FALSE, "DoorPokayokeEnable"=FALSE, "FailCountDisplayEnable"=FALSE, "FailCountReversalEnable"=FALSE, "DataLoggingEnable"=FALSE, "PauseOnReelCountFinish"=FALSE, "StopOnTotalCountFinish"=FALSE, "IoTEnable"=FALSE, "ReportEnable"=FALSE, "DebugLevel"=0.0, "PowerOnSelfTestFeatures"={"TimingUnit"=FALSE, "MachinePowerStatusCheck"=FALSE, "GuideMotor"=FALSE, "CameraOptics"=FALSE, "MasterSample"=FALSE}, "DiagnosticsFeatures"={"TimingUnit"=FALSE, "GuideMotor"=FALSE, "CameraOptics"=FALSE, "ReelerMotor"=FALSE, "HardwareButtons"=FALSE, "Sensors"=FALSE, "TowerLamp"=FALSE, "MasterSample"=FALSE}, "UserInterface"={"DynamicImageHandlingEnable"=FALSE, "DoorPokaYokeButtonVisible"=FALSE, "FailCountDisplayButtonVisible"=FALSE, "FailCountReversalButtonVisible"=FALSE}, "PopupOptions"={"ReasonForPause"=FALSE, "ReasonForFail"=FALSE, "ReasonForStop"=FALSE, "CpCpkOnReelFinish"=FALSE}, "DataloggingFeatures"={"EventData"=FALSE, "MeasurementData"=FALSE, "StatisticalData"=FALSE, "ReelData"=FALSE, "FailedMeasurementData"=FALSE, "FailedImages"=FALSE}, "IoT"={"SMSAlertEnable"=FALSE, "EmailAlertEnable"=FALSE}}}, "PartsConfigured"=[], "CameraSequenceList"=[], "SensorList"=[], "MasterSampleMessages"={"MasterSampleMessage"="", "PartMessage"=""}, "SensorDiagnosticsResult"={"Image Array"=[], "ImageCount"=0}, "IgnoredCountDetails"={"ReelCount"=0, "TotalCount"=0}, "MachineStatusToDL"="", "MasterSamplePartName"=""}, "SelComplete"=FALSE, "ResultToMI"=FALSE, "Exit"=FALSE, "NumberOfActorsLaunched"=0, "BatchStart"=FALSE, "LoadingBarActive"=FALSE, "UpdateInPause"=FALSE, " EventReason"="", "PopUpCategory"="", "PopUpActive"=FALSE, "MasterSampleState"="", "CameraOpticsDiagnosticsStatus"=FALSE, "CameraIndex"=0, "SensorIndex"=0} ("LocalData_SM"), "Timeout"=w1651, "Core"=w1660, "Ack"=w1648, "CurrentState"=w1647, "DirectExit"=w1646, "SoftwareExit"=w1645, "SensorDiagnosticsStatus"=w1644, "OutputCluster"=w1624, "SelComplete"=w1643, "ResultToMI"=w1642, "Exit"=w1623, "NumberOfActorsLaunched"=w1641, "BatchStart"=w1640, "LoadingBarActive"=w1639, "UpdateInPause"=w1637, "EventReason"=w1636, "PopUpCategory"=w1635, "PopUpActive"=w1634, "CameraOpticsDiagnosticsStatus"=w1631, "CameraIndex"=w1630, "SensorIndex"=w1625) -> (w1661:T1)  [unwired: 1 in]
      }
      frame "Data: Cleanup" {
        # "Cleanup any data and references, here.\n(this is called automatically, by the Macro: Exit)"
        n377 = Unbundle By Name(w1669) -> ("Core.Current VI Reference"=w1671:refnum<vi>)
        n378 = Unregister For Events(event registration refnum=w1668, error in=w1667) -> (error out=w1666:errorcluster)
        n379 = call "Destroy User Events_SM.vi"("error in (no error)"=w1666, "Inspection Statemachine in"=w1665) -> ("error out"=w1664:errorcluster)  [unwired: 9 in]
        n380 = Close Reference(reference=w1671, error in (no error)=w1664) -> (error out=w1670:errorcluster)
        n381 = call <vilib>:"Add State(s) to Queue__JKI_lib_State_Machine.vi"("State(s) in (\"\")"=w1673) -> ("States Out"=w1672:string)  [unwired: 14 in]
      }
      frame "---------- UI ----------" {
        # "Do not put any code in this frame.\n(It is a separator no-op. You can make a copy of this frame to create a new UI frame)"
        n382 = call <vilib>:"Add State(s) to Queue__JKI_lib_State_Machine.vi"("State(s) in (\"\")"=w1678) -> ("States Out"=w1677:string)  [unwired: 14 in]
      }
      frame "UI: Initialize" {
        # "Initialize the User Interface, here.\n(this is called automatically, by the Macro: Init)"
        n383 = call <vilib>:"Add State(s) to Queue__JKI_lib_State_Machine.vi"("State(s) in (\"\")"=w1683) -> ("States Out"=w1682:string)  [unwired: 14 in]
      }
      frame "UI: Front Panel State" {
        # "Argument Open/Close"
        # "Set Front Panel Open or Closed\n(Usage: \"UI: Front Panel State >> Open|Close\")"
        n384 = Unbundle By Name(w1687) -> ("Core.Current VI Reference"=w1686:refnum<vi>)
        n385 = case shown="\"Close\"" w1685 {
          tunnel: w1689 -> [w1695 w1708]
          tunnel: [w1697 w1709] -> w1688
          tunnel: w1686 -> [w1696 w1706]
          frame "Open", Default {
            n386 = property class="VI"(reference=w1696, error in=w1695) -> (reference out=w1693:refnum<vi>, error out=w1694:errorcluster, "Front Panel.Open"=w1692:bool)
            n387 = case shown="False" w1692 {
              tunnel: [w1700 w1703] -> w1697
              tunnel: w1694 -> [w1699 w1703]
              tunnel: w1693 -> [w1698 _]
              frame False {
                n388 = invoke class="VI" method="FP.Open"(reference=w1698, error in=w1699, "Activate"=TRUE, "State"=T10."Standard") -> (error out=w1700:errorcluster)  [unwired: 1 in, 4 out]
              }
              frame True {
              }
            }
          }
          frame "Close" {
            n389 = property class="VI"(reference=w1706, error in=w1708) -> (reference out=w1705:refnum<vi>, error out=w1707:errorcluster, "Front Panel.Open"=w1704:bool)
            n390 = case shown="True" w1704 {
              tunnel: [w1710 w1713] -> w1709
              tunnel: w1707 -> [w1710 w1712]
              tunnel: w1705 -> [_ w1711]
              frame False {
              }
              frame True {
                n391 = invoke class="VI" method="FP.Close"(reference=w1711, error in=w1712) -> (error out=w1713:errorcluster)  [unwired: 1 in, 2 out]
              }
            }
          }
        }
        n392 = call <vilib>:"Add State(s) to Queue__JKI_lib_State_Machine.vi"("State(s) in (\"\")"=w1691) -> ("States Out"=w1690:string)  [unwired: 14 in]
      }
      frame "---------- Macro ----------" {
        # "Do not put any code in this frame.\n(It is a separator no-op. You can make a copy of this frame to create a new Macro frame)"
        n393 = call <vilib>:"Add State(s) to Queue__JKI_lib_State_Machine.vi"("State(s) in (\"\")"=w1718) -> ("States Out"=w1717:string)  [unwired: 14 in]
      }
      frame "Macro: Initialize" {
        # "Initialization Macro\n(This is called once, when the VI starts)"
        n394 = call <vilib>:"Add State(s) to Queue__JKI_lib_State_Machine.vi"("State(s) in Front (\"\")"="Data: Initialize\nInitialize Core Data\nUI: Initialize", "State(s) in (\"\")"=w1724) -> ("States Out"=w1723:string)  [unwired: 13 in]
      }
      frame "Macro: Exit" {
        # "Exit Macro\n(This is called once, when the VI exits)"
        n395 = Unbundle By Name(w1732) -> ("Core.Close Panel on Exit?"=w1731:bool)
        n396 = Select(t="UI: Front Panel State >> Close", s=w1731, f="") -> (s? t:f=w1728:string)
        n397 = call <vilib>:"Add State(s) to Queue__JKI_lib_State_Machine.vi"("State(s) in (\"\")"=w1728, "State(s) at Back (\"\")"="Data: Cleanup\nExit") -> ("States Out"=w1726:string)  [unwired: 13 in]
        n398 = call <vilib>:"Add State(s) to Queue__JKI_lib_State_Machine.vi"("State(s) in Front (\"\")"=w1726, "State(s) in (\"\")"=w1735) -> ("States Out"=w1734:string)  [unwired: 13 in]
      }
      frame "---------- Launch ----------" {
        # "Do not put any code in this frame.\n(It is a separator no-op. You can make a copy of this frame to create a new UI frame)"
        n399 = call <vilib>:"Add State(s) to Queue__JKI_lib_State_Machine.vi"("State(s) in (\"\")"=w1740) -> ("States Out"=w1739:string)  [unwired: 14 in]
      }
      frame "LaunchChildActors" {
        # "Wait for Ack"
        n400 = in-place {
          in-place-border: w1749 -> [w1773]
          in-place-border: w1748 -> [w1771]
          in-place-border: [w1761] -> w1747
          in-place-border: [w1760] -> w1746
          # "Launch UI"
          n401 = in-place-cluster #4(w1742) -> ("OutputCluster.SystemParameters.NumberOfRacks"=w1752:u8, "OutputCluster.SystemParameters.SoftwareFeatures.HardwareEmulated"=w1753:bool, "OutputCluster.SystemParameters.SoftwareFeatures.AnalyticsEnable"=w1754:bool, "OutputCluster.SystemParameters.SoftwareFeatures.DataLoggingEnable"=w1755:bool, "NumberOfActorsLaunched"=w1758:i32)  [unwired: 1 out]
          n402 = case shown="True" w1753 {
            tunnel: w1771 -> [w1800 w1804]
            tunnel: [w1799 w1804] -> w1774
            tunnel: w1773 -> [w1798 w1803]
            tunnel: [w1797 w1803] -> w1772
            tunnel: w1758 -> [w1796 w1802]
            tunnel: [w1795 w1802] -> w1768
            frame False {
              # "Online Execution"
              n403 = Increment(x=w1796) -> (x+1=w1795:i32)
              n404 = call <vilib>:"Launch Nested Actor.vi"("error in (no error)"=w1800, "Nested Actor"=refnum<class "Machine Interface.lvclass"> refnum ("Machine Interface Actor.lvclass"), "Caller Actor in"=w1798) -> ("error out"=w1799:errorcluster, "Caller Actor out"=w1797:refnum<class "Inspection Statemachine.lvclass">)  [unwired: 6 in, 1 out]
            }
            frame True {
              # "In offline execution,\nMI actor\nis not launched"
              # "Offline"
            }
          }
          n405 = Add(x=w1752, y=w1768) -> (x+y=w1767:i32)
          n406 = for {
            N: w1752 -> [_]
            tunnel: w1772 -> [w1809]
            tunnel: w1774 -> [w1807]
            tunnel: [w1806] -> w1765
            tunnel: [w1805] -> w1764
            # "Number of Racks times \nlaunch Rack controller Actor.\nNumberOfRacks \nparameter is read from \nSystem Configuration JSON"
            # "This loop iterates \"Number of Racks\" number of times"
            n407 = call <vilib>:"Launch Nested Actor.vi"("error in (no error)"=w1807, "Nested Actor"=refnum<class "Rack Controller.lvclass"> refnum ("Rack Controller.lvclass"), "Caller Actor in"=w1809) -> ("error out"=w1806:errorcluster, "Caller Actor out"=w1805:refnum<class "Inspection Statemachine.lvclass">)  [unwired: 6 in, 1 out]
          }
          n408 = case shown="False" w1754 {
            tunnel: w1764 -> [w1786 w1794]
            tunnel: w1765 -> [w1787 w1793]
            tunnel: [w1787 w1792] -> w1770
            tunnel: [w1786 w1791] -> w1769
            tunnel: w1767 -> [w1785 w1790]
            tunnel: [w1785 w1789] -> w1766
            frame False {
              # "Analytics Disabled"
            }
            frame True {
              # "Analytics Enabled"
              n409 = Increment(x=w1790) -> (x+1=w1789:i32)
              n410 = call <vilib>:"Launch Nested Actor.vi"("error in (no error)"=w1793, "Nested Actor"=refnum<class "Zen Analytics.lvclass"> refnum ("Zen Analytics.lvlib:Zen Analytics.lvclass"), "Caller Actor in"=w1794) -> ("error out"=w1792:errorcluster, "Caller Actor out"=w1791:refnum<class "Inspection Statemachine.lvclass">)  [unwired: 6 in, 1 out]
            }
          }
          n411 = case shown="True" w1755 {
            tunnel: w1770 -> [w1776 w1784]
            tunnel: [w1776 w1783] -> w1763
            tunnel: w1769 -> [w1777 w1782]
            tunnel: [w1777 w1781] -> w1762
            tunnel: w1766 -> [w1775 w1779]
            tunnel: [w1775 w1778] -> w1756
            frame False {
              # "Datalogger disabled"
            }
            frame True {
              # "DataLogger Enabled"
              n412 = Increment(x=w1779) -> (x+1=w1778:i32)
              n413 = call <vilib>:"Launch Nested Actor.vi"("error in (no error)"=w1784, "Nested Actor"=refnum<class "DataLogger.lvclass"> refnum ("DataLogger.lvclass"), "Caller Actor in"=w1782) -> ("error out"=w1783:errorcluster, "Caller Actor out"=w1781:refnum<class "Inspection Statemachine.lvclass">)  [unwired: 6 in, 1 out]
            }
          }
          n414 = in-place-cluster #4("Timeout"=10000, "OutputCluster.SystemParameters.NumberOfRacks"=w1752, "OutputCluster.SystemParameters.SoftwareFeatures.HardwareEmulated"=w1753, "OutputCluster.SystemParameters.SoftwareFeatures.AnalyticsEnable"=w1754, "OutputCluster.SystemParameters.SoftwareFeatures.DataLoggingEnable"=w1755, "NumberOfActorsLaunched"=w1756) -> (w1741:T1)
          n415 = call <vilib>:"Launch Nested Actor.vi"("error in (no error)"=w1763, "Nested Actor"=refnum<class "ZenGage v3.0 UI.lvclass"> refnum ("ZenGage v3.0 UI.lvclass"), "Caller Actor in"=w1762) -> ("error out"=w1761:errorcluster, "Caller Actor out"=w1760:refnum<class "Inspection Statemachine.lvclass">)  [unwired: 6 in, 1 out]
        }
        n416 = call <vilib>:"Build State String with Arguments__JKI_lib_State_Machine.vi"("Arguments (\"\")"="Launch", "State"="Wait" ("State(s) in Front (\"\")")) -> ("State with Arguments"=w1743:string)  [unwired: 4 in]
        n417 = call <vilib>:"Add State(s) to Queue__JKI_lib_State_Machine.vi"("State(s) in Front (\"\")"=w1743, "State(s) in (\"\")"=w1751) -> ("States Out"=w1750:string)  [unwired: 13 in]
      }
      frame "SendRackID" {
        # "Wait for Clear Message from \nRack Controller Actor"
        n418 = Unbundle By Name(w1821) -> ("OutputCluster.SystemParameters.NumberOfRacks"=w1825:u8, "OutputCluster.SystemParameters.SoftwareFeatures.DataLoggingEnable"=w1810:bool)
        n419 = Bundle By Name(cluster=w1821, "OutputCluster.PartInfo.NumberOfRacks"=w1825) -> (w1823:T1)
        n420 = Unbundle By Name(w1823) -> ("OutputCluster"=w1813:T2)
        n421 = Bundle By Name(cluster=w1823, "Timeout"=20000) -> (w1822:T1)
        n422 = call "Output_SM.vi"("SM Private Data in"=w1816, "Output Cluster"=w1813, "Receiver Name"="RC", "State"="RC: RackID", "error in (no error)"=w1827) -> ("SM Private Data out"=w1814:refnum<class "Inspection Statemachine.lvclass">, "error out"=w1815:errorcluster)  [unwired: 9 in]
        n423 = call <vilib>:"Build State String with Arguments__JKI_lib_State_Machine.vi"("Arguments (\"\")"="Launch", "State"="Wait" ("State(s) in Front (\"\")")) -> ("State with Arguments"=w1818:string)  [unwired: 4 in]
        n424 = case shown="False" w1810 {
          tunnel: w1815 -> [w1831 w1836]
          tunnel: w1814 -> [w1830 w1835]
          tunnel: w1813 -> [_ w1834]
          tunnel: [w1830 w1833] -> w1812
          tunnel: [w1831 w1832] -> w1811
          frame False {
            # "DL Disable"
          }
          frame True {
            # "DL Enable"
            n425 = Bundle By Name(cluster=w1834, "EventData.EventName"="Start" ("DataLogger.EventDetails.EventName"), "EventData.EventReason"="Machine Start" ("DataLogger.EventDetails.EventReason")) -> (w1838:T2)
            n426 = call "Output_SM.vi"("SM Private Data in"=w1835, "Output Cluster"=w1838, "Receiver Name"="DL", "State"="DL: EventDetails", "error in (no error)"=w1836) -> ("SM Private Data out"=w1833:refnum<class "Inspection Statemachine.lvclass">, "error out"=w1832:errorcluster)  [unwired: 9 in]
          }
        }
        n427 = call <vilib>:"Add State(s) to Queue__JKI_lib_State_Machine.vi"("State(s) in Front (\"\")"=w1818, "State(s) in (\"\")"=w1829) -> ("States Out"=w1828:string)  [unwired: 13 in]
      }
      frame "SendInit" {
        n428 = Unbundle By Name(w1854) -> ("OutputCluster.SystemParameters.SoftwareFeatures.DataLoggingEnable"=w1842:bool, "OutputCluster"=w1843:T2, "OutputCluster.SystemParameters.SoftwareFeatures.AnalyticsEnable"=w1855:bool)
        n429 = case shown="True" w1855 {
          tunnel: w1853 -> [w1869 w1873]
          tunnel: w1849 -> [w1868 w1876]
          tunnel: w1843 -> [_ w1875]
          tunnel: [w1869 w1872] -> w1852
          tunnel: [w1868 w1870] -> w1848
          frame False {
            # "Analytics Disabled"
          }
          frame True {
            # "Analytics Enabled"
            n430 = call "Output_SM.vi"("SM Private Data in"=w1876, "Output Cluster"=w1875, "Receiver Name"="UI", "State"="UI: AnalyticsRef", "error in (no error)"=w1873) -> ("SM Private Data out"=w1870:refnum<class "Inspection Statemachine.lvclass">, "error out"=w1872:errorcluster)  [unwired: 9 in]
          }
        }
        n431 = call "Output_SM.vi"("SM Private Data in"=w1848, "Output Cluster"=w1843, "Receiver Name"="UI", "State"="UI: SystemInfo", "error in (no error)"=w1852) -> ("SM Private Data out"=w1845:refnum<class "Inspection Statemachine.lvclass">, "error out"=w1847:errorcluster)  [unwired: 9 in]
        n432 = call <vilib>:"Add State(s) to Queue__JKI_lib_State_Machine.vi"("State(s) in Front (\"\")"="CallLogo>>close\nCheckHardware" ("State(s) in Front (\"\")"), "State(s) in (\"\")"=w1858) -> ("States Out"=w1857:string)  [unwired: 13 in]
        n433 = case shown="True" w1842 {
          tunnel: w1847 -> [w1859 w1866]
          tunnel: [w1859 w1865] -> w1846
          tunnel: w1845 -> [w1860 w1863]
          tunnel: [w1860 w1862] -> w1844
          tunnel: w1843 -> [_ w1861]
          frame False {
            # "DL Disable"
          }
          frame True {
            # "DL Enable"
            n434 = call "Output_SM.vi"("SM Private Data in"=w1863, "Output Cluster"=w1861, "Receiver Name"="DL", "State"="DL: SystemInfo", "error in (no error)"=w1866) -> ("SM Private Data out"=w1862:refnum<class "Inspection Statemachine.lvclass">, "error out"=w1865:errorcluster)  [unwired: 9 in]
          }
        }
      }
      frame "CallLogo" {
        (unwired) T2 {"RackID"=0, "Trigger Light Camera Sequence"={"Light Sequence Trigger"="", "Status"="", "Mode"=""}, "Result Cluster"={"RackID"=0, "MeasurementValuesArray "=[], "ImagesArray"=[], "ResultPF"=FALSE, "ProductionCountDetails"={"TotalFail"=0, "TotalPass"=0, "TotalCount"=0}, "ReelCountDetails"={"ReelFail"=0, "ReelPass"=0, "ReelCount"=0}, "ControlPFArray"=[], "SpecificationPFArray"=[], "SpecificationFail"=FALSE, "ReelNumber"=0, "Status"=""}, "Analytics VI refnum"=refnum, "Statistical parameters "=[], "Sensor Name"="", "Camera Name"="", "PopupInput"={"Pop-up Type"=enum."Open Logo Display", "Title"="", "Message"="", "Button 1 Text"="", "Button 2 Text"="", "Show Close? T/F"=FALSE, "Title Blink? T/F"=FALSE, "Title Blink Colour"=0}, "PartInfo"={"PartName"="", "NumberOfRacks"=0, "TotalCount"=0, "ReelCount"=0, "OperatorName"="", "StampingMachineID"=0, "RackID"=0, "Reinitialize"=FALSE, "MeasurementNamesArray"=[], "MeasurementIDArray"=[], "SpecValuesArray"=[], "CameraNamesArray"=[]}, "StateMsgToMI"="", "InspectionStatusToMI"="", "StateMsgToRC"="", "StateMsgToUI"="", "StateMsgToDL"="", "StateMsgToAN"="", "StateMsgToSM"="", "EventData"={"EventName"="", "EventReason"=""}, "CameraOpticsDiagnosticsResult"={"LightCameraName"="", "DiagnosedImage"=refnum, "DustPercentage"=0.0, "Result"=TRUE}, "AllPartInfo"=[{"PartName"="", "NumberOfRacks"=0, "MeasurementIDsArray"=[], "MeasurementNamesArray"=[], "SpecValuesArray"=[]}], "SystemParameters"={"SystemName"="", "SystemID"="", "CustomerDetails"={"CustomerName"="", "CustomerId"="", "Location"="", "NumberOfShifts"=0.0, "ShiftDetails"=[]}, "InstallationDate"="", "NextServiceDate"="", "NumberOfRacks"=0, "TotalNumberOfCameras"=0, "SoftwareFeatures"={"HardwareEmulated"=FALSE, "PowerOnSelfTest"=FALSE, "DiagnosticsEnable"=FALSE, "AnalyticsEnable"=FALSE, "DefectTrackingEnable"=FALSE, "AutomaticGuideMovement"=FALSE, "DoorPokayokeEnable"=FALSE, "FailCountDisplayEnable"=FALSE, "FailCountReversalEnable"=FALSE, "DataLoggingEnable"=FALSE, "PauseOnReelCountFinish"=FALSE, "StopOnTotalCountFinish"=FALSE, "IoTEnable"=FALSE, "ReportEnable"=FALSE, "DebugLevel"=0.0, "PowerOnSelfTestFeatures"={"TimingUnit"=FALSE, "MachinePowerStatusCheck"=FALSE, "GuideMotor"=FALSE, "CameraOptics"=FALSE, "MasterSample"=FALSE}, "DiagnosticsFeatures"={"TimingUnit"=FALSE, "GuideMotor"=FALSE, "CameraOptics"=FALSE, "ReelerMotor"=FALSE, "HardwareButtons"=FALSE, "Sensors"=FALSE, "TowerLamp"=FALSE, "MasterSample"=FALSE}, "UserInterface"={"DynamicImageHandlingEnable"=FALSE, "DoorPokaYokeButtonVisible"=FALSE, "FailCountDisplayButtonVisible"=FALSE, "FailCountReversalButtonVisible"=FALSE}, "PopupOptions"={"ReasonForPause"=FALSE, "ReasonForFail"=FALSE, "ReasonForStop"=FALSE, "CpCpkOnReelFinish"=FALSE}, "DataloggingFeatures"={"EventData"=FALSE, "MeasurementData"=FALSE, "StatisticalData"=FALSE, "ReelData"=FALSE, "FailedMeasurementData"=FALSE, "FailedImages"=FALSE}, "IoT"={"SMSAlertEnable"=FALSE, "EmailAlertEnable"=FALSE}}}, "PartsConfigured"=[], "CameraSequenceList"=[], "SensorList"=[], "MasterSampleMessages"={"MasterSampleMessage"="", "PartMessage"=""}, "SensorDiagnosticsResult"={"Image Array"=[], "ImageCount"=0}, "IgnoredCountDetails"={"ReelCount"=0, "TotalCount"=0}, "MachineStatusToDL"="", "MasterSamplePartName"=""} ("Output Cluster")
        n435 = Unbundle By Name(w1880) -> ("OutputCluster"=w1879:T2)
        n436 = Concatenate Strings("Display zentron stratuplogo>>" ("string"), w1881) -> (w1883:string)
        n437 = Bundle By Name(cluster=w1879, "StateMsgToUI"=w1883) -> (w1885:T2)
        n438 = call "Output_SM.vi"("SM Private Data in"=w1877, "Output Cluster"=w1885, "Receiver Name"="UI", "State"="UI: StateMessage", "error in (no error)"=w1878) -> ("SM Private Data out"=w1884:refnum<class "Inspection Statemachine.lvclass">, "error out"=w1888:errorcluster)  [unwired: 9 in]
        n439 = call <vilib>:"Add State(s) to Queue__JKI_lib_State_Machine.vi"("State(s) in (\"\")"=w1889) -> ("States Out"=w1890:string)  [unwired: 14 in]
      }
      frame "---------- Diagnostics ----------" {
        # "Do not put any code in this frame.\n(It is a separator no-op. You can make a copy of this frame to create a new UI frame)"
        n440 = call <vilib>:"Add State(s) to Queue__JKI_lib_State_Machine.vi"("State(s) in (\"\")"=w1895) -> ("States Out"=w1894:string)  [unwired: 14 in]
      }
      frame "CheckHardware" {
        n441 = Unbundle By Name(w1899) -> ("OutputCluster.SystemParameters.SoftwareFeatures.HardwareEmulated"=w1903:bool, "OutputCluster"=w1901:T2)
        n442 = case shown="True" w1903 {
          tunnel: w1897 -> [w1916 w1918]
          tunnel: w1905 -> [w1914 w1920]
          tunnel: [w1913 w1920] -> w1904
          tunnel: ["Wait" ("State(s) in Front (\"\")") "StartDiagnostics" ("State(s) at Back (\"\")")] -> w1902
          tunnel: w1901 -> [w1912 _]
          tunnel: [w1908 w1918] -> w1896
          frame False {
            # "Wait for COM port \navailability response"
            # "This case is for identifying Arduino Port"
            # "Online Execution"
            n443 = Bundle By Name(cluster=w1912, "StateMsgToMI"="CheckArduinoPort" ("StateMessageToMI")) -> (w1911:T2)
            n444 = call "Output_SM.vi"("SM Private Data in"=w1916, "Output Cluster"=w1911, "Receiver Name"="MI", "State"="MI: StateMessage", "error in (no error)"=w1914) -> ("SM Private Data out"=w1908:refnum<class "Inspection Statemachine.lvclass">, "error out"=w1913:errorcluster)  [unwired: 9 in]
          }
          frame True {
            # "Offline Execution"
          }
        }
        n445 = Bundle By Name(cluster=w1899, "CurrentState"="Diagnostics") -> (w1898:T1)
        n446 = call <vilib>:"Add State(s) to Queue__JKI_lib_State_Machine.vi"("State(s) in Front (\"\")"=w1902, "State(s) in (\"\")"=w1907) -> ("States Out"=w1906:string)  [unwired: 13 in]
      }
      frame "CheckMachinePower" {
        n447 = Unbundle By Name(w1926) -> ("OutputCluster.SystemParameters.SoftwareFeatures.HardwareEmulated"=w1925:bool, "OutputCluster"=w1923:T2)
        n448 = case shown="False" w1925 {
          tunnel: w1922 -> [w1944 w1947]
          tunnel: w1928 -> [w1943 w1951]
          tunnel: [w1938 w1951] -> w1927
          tunnel: ["Wait" ("State(s) in Front (\"\")") w1948] -> w1924
          tunnel: w1923 -> [w1935 _]
          tunnel: [w1936 w1947] -> w1921
          frame False {
            # "Wait for Machine Power \nStatus response"
            # "Online Execution"
            n449 = Bundle By Name(cluster=w1935, "StateMsgToMI"="MachinePowerStatusCheck" ("StateMessageToMI")) -> (w1940:T2)
            n450 = call "Output_SM.vi"("SM Private Data in"=w1944, "Output Cluster"=w1940, "Receiver Name"="MI", "State"="MI: StateMessage", "error in (no error)"=w1943) -> ("SM Private Data out"=w1937:refnum<class "Inspection Statemachine.lvclass">, "error out"=w1939:errorcluster)  [unwired: 9 in]
            n451 = Bundle By Name(cluster=w1935, "StateMsgToUI"="UpdateDiagnosticsStatusString>>Machine Power Status") -> (w1934:T2)
            n452 = call "Output_SM.vi"("SM Private Data in"=w1937, "Output Cluster"=w1934, "Receiver Name"="UI", "State"="UI: StateMessage", "error in (no error)"=w1939) -> ("SM Private Data out"=w1936:refnum<class "Inspection Statemachine.lvclass">, "error out"=w1938:errorcluster)  [unwired: 9 in]
          }
          frame True {
            # "Offline Execution"
            n453 = call <vilib>:"Build State String with Arguments__JKI_lib_State_Machine.vi"("Arguments (\"\")"="MachinePoweredOn" ("Arguments (\"\")"), "State"="NextDiagnostics") -> ("State with Arguments"=w1948:string)  [unwired: 4 in]
          }
        }
        n454 = call <vilib>:"Add State(s) to Queue__JKI_lib_State_Machine.vi"("State(s) in Front (\"\")"=w1924, "State(s) in (\"\")"=w1930) -> ("States Out"=w1929:string)  [unwired: 13 in]
      }
      frame "StartDiagnostics" {
        n455 = Unbundle By Name(w1957) -> ("OutputCluster.SystemParameters.SoftwareFeatures.PowerOnSelfTest"=w1956:bool)
        n456 = case shown="False" w1956 {
          tunnel: [w1961 w1977] -> w1958
          tunnel: w1957 -> [w1965 w1976]
          tunnel: w1955 -> [w1969 w1975]
          tunnel: [w1968 w1975] -> w1954
          tunnel: w1953 -> [w1967 w1974]
          tunnel: [w1966 w1974] -> w1952
          frame False {
            # "POST Disabled"
            n457 = Unbundle By Name(w1965) -> ("OutputCluster"=w1964:T2)
            n458 = Bundle By Name(cluster=w1964, "StateMsgToUI"="DisplayInspectionPage") -> (w1971:T2)
            n459 = call "Output_SM.vi"("SM Private Data in"=w1967, "Output Cluster"=w1971, "Receiver Name"="UI", "State"="UI: StateMessage", "error in (no error)"=w1969) -> ("SM Private Data out"=w1966:refnum<class "Inspection Statemachine.lvclass">, "error out"=w1968:errorcluster)  [unwired: 9 in]
            n460 = call <vilib>:"Build State String with Arguments__JKI_lib_State_Machine.vi"("Arguments (\"\")"="DeviceReady", "State"="NextDiagnostics") -> ("State with Arguments"=w1961:string)  [unwired: 4 in]
          }
          frame True {
            # "Check ArduinoDiagnosticsEnableOnPowerOn parameter from JSON"
            # "POST Enabled"
            n461 = Unbundle By Name(w1976) -> ("OutputCluster.SystemParameters.SoftwareFeatures.PowerOnSelfTestFeatures.TimingUnit"=w1981:bool)
            n462 = call <vilib>:"Build State String with Arguments__JKI_lib_State_Machine.vi"("Arguments (\"\")"="DeviceReady", "State"="NextDiagnostics") -> ("State with Arguments"=w1978:string)  [unwired: 4 in]
            n463 = Select(t="ArduinoDiagnostics", s=w1981, f=w1978) -> (s? t:f=w1977:string)
          }
        }
        n464 = call <vilib>:"Add State(s) to Queue__JKI_lib_State_Machine.vi"("State(s) in Front (\"\")"=w1958, "State(s) in (\"\")"=w1960) -> ("States Out"=w1959:string)  [unwired: 13 in]
      }
      frame "NextDiagnostics" {
        n465 = Unbundle By Name(w1988) -> ("OutputCluster.SystemParameters.SoftwareFeatures.PowerOnSelfTest"=w1983:bool, "CurrentState"=w1986:string, "OutputCluster"=w1991:T2, "OutputCluster.SystemParameters.SoftwareFeatures.PowerOnSelfTestFeatures.MasterSample"=w1985:bool, "OutputCluster.SystemParameters.SoftwareFeatures.HardwareEmulated"=w1984:bool)
        n466 = case shown="\"CameraOpticsDiagnosticsDone\"" w1995 {
          tunnel: ["Wait" w2009 w2037 w2054 w2069] -> w1994
          tunnel: w1991 -> [_ w2003 _ _ w2070]
          tunnel: w1993 -> [w2000 w2004 w2035 w2052 w2073]
          tunnel: [w2000 w2005 w2035 w2052 w2072] -> w1992
          tunnel: w1990 -> [w1999 w2002 w2034 w2051 w2071]
          tunnel: w1988 -> [w1998 w2007 w2033 w2050 w2067]
          tunnel: [w1999 w2002 w2034 w2051 w2068] -> w1989
          tunnel: [w1998 w2007 w2033 w2050 w2066] -> w1987
          tunnel: w1986 -> [_ _ _ _ w2065]
          tunnel: w1985 -> [_ _ _ _ w2064]
          tunnel: w1984 -> [_ _ _ _ w2063]
          tunnel: w1983 -> [_ w2006 _ _ _]
          frame Default {
          }
          frame "DeviceReady" {
            # "If Arduino is connected, move to Motor Diagnostics in case of Power ON.\nOtherwise move to Wait state"
            n467 = First Call?() -> (First Call?: T/F=w2008:bool)
            n468 = case shown="True" w2008 {
              tunnel: ["Wait" w2018] -> w2009
              tunnel: w2007 -> [_ w2023]
              tunnel: w2006 -> [_ w2012]
              tunnel: [w2010 w2016] -> w2005
              tunnel: w2004 -> [w2010 w2015]
              tunnel: w2003 -> [_ w2014]
              tunnel: w2002 -> [_ w2013]
              frame False {
                # "Diagnostics"
              }
              frame True {
                # "POST"
                n469 = Unbundle By Name(w2023) -> ("OutputCluster.SystemParameters.SoftwareFeatures.PowerOnSelfTestFeatures.MachinePowerStatusCheck"=w2022:bool)
                n470 = case shown="True" w2012 {
                  tunnel: [w2027 w2032] -> w2016
                  tunnel: w2015 -> [w2026 w2032]
                  tunnel: w2014 -> [w2025 _]
                  tunnel: w2013 -> [w2024 _]
                  frame False {
                    n471 = Bundle By Name(cluster=w2025, "StateMsgToUI"="DisplayInspectionPage>>Reset") -> (w2029:T2)
                    n472 = call "Output_SM.vi"("SM Private Data in"=w2024, "Output Cluster"=w2029, "Receiver Name"="UI", "State"="UI: StateMessage", "error in (no error)"=w2026) -> ("error out"=w2027:errorcluster)  [unwired: 9 in, 1 out]
                  }
                  frame True {
                    # "POST enabled"
                  }
                }
                n473 = Select(t="Initialization\nCheckMachinePower", s=w2022, f="Initialization\nNextDiagnostics >> MachinePoweredOn") -> (s? t:f=w2019:string)
                n474 = Select(t=w2019, s=w2012, f="Initialization\nSelect") -> (s? t:f=w2018:string)
              }
            }
          }
          frame "MachinePoweredOn" {
            # "If Arduino is connected, move to Motor Diagnostics in case of Power ON.\nOtherwise move to Wait state"
            n475 = First Call?() -> (First Call?: T/F=w2036:bool)
            n476 = case shown="True" w2036 {
              tunnel: ["Wait" w2040] -> w2037
              tunnel: w2033 -> [_ w2042]
              frame False {
                # "Diagnostics"
              }
              frame True {
                # "POST"
                n477 = Unbundle By Name(w2042) -> ("OutputCluster.SystemParameters.SoftwareFeatures.PowerOnSelfTestFeatures.GuideMotor"=w2041:bool, "OutputCluster.SystemParameters.SoftwareFeatures.AutomaticGuideMovement"=w2039:bool)
                n478 = case shown="True" w2041 {
                  tunnel: ["NextDiagnostics >> MotorDiagnosticsDone" w2044] -> w2040
                  tunnel: w2039 -> [_ w2049]
                  frame False {
                    # "Motor POST disabled"
                  }
                  frame True {
                    # "Motor POST enabled"
                    n479 = call <vilib>:"Build State String with Arguments__JKI_lib_State_Machine.vi"("Arguments (\"\")"="MotorDiagnosticsDone" ("Arguments (\"\")"), "State"="NextDiagnostics") -> ("State with Arguments"=w2045:string)  [unwired: 4 in]
                    n480 = Select(t="MotorDiagnostics", s=w2049, f=w2045) -> (s? t:f=w2044:string)
                  }
                }
              }
            }
          }
          frame "MotorDiagnosticsDone" {
            # "If Motor Diagnostics is successfully done, move to Camera Optics Diagnostics in case of Power ON.\nOtherwise move to Wait state."
            n481 = First Call?() -> (First Call?: T/F=w2053:bool)
            n482 = case shown="True" w2053 {
              tunnel: ["Wait" w2056] -> w2054
              tunnel: w2050 -> [_ w2062]
              frame False {
              }
              frame True {
                n483 = Unbundle By Name(w2062) -> ("OutputCluster.SystemParameters.SoftwareFeatures.PowerOnSelfTestFeatures.CameraOptics"=w2061:bool)
                n484 = call <vilib>:"Build State String with Arguments__JKI_lib_State_Machine.vi"("Arguments (\"\")"=" CameraOpticsDiagnosticsDone " ("Arguments (\"\")"), "State"="NextDiagnostics") -> ("State with Arguments"=w2057:string)  [unwired: 4 in]
                n485 = Select(t="CameraOpticsDiagnostics\nStartCameraDiagnostics", s=w2061, f=w2057) -> (s? t:f=w2056:string)
              }
            }
          }
          frame "CameraOpticsDiagnosticsDone" {
            n486 = First Call?() -> (First Call?: T/F=w2074:bool)
            n487 = case shown="True" w2074 {
              tunnel: w2073 -> [w2078 w2081]
              tunnel: [w2078 w2090] -> w2072
              tunnel: w2071 -> [w2076 w2084]
              tunnel: w2070 -> [_ w2089]
              tunnel: ["" w2088] -> w2069
              tunnel: [w2076 w2087] -> w2068
              tunnel: w2067 -> [w2075 w2086]
              tunnel: [w2075 w2085] -> w2066
              tunnel: w2065 -> [_ _]
              tunnel: w2064 -> [_ w2079]
              tunnel: w2063 -> [_ w2082]
              frame False {
                # "Diagnostics"
              }
              frame True {
                # "POST"
                n488 = Unbundle By Name(w2084) -> ("TimeLoopEnable"=w2083:refnum<user-event>)
                n489 = Generate User Event(user event=w2083, event data cluster=w2079, error in=w2081) -> (error out=w2080:errorcluster)  [unwired: 1 in, 1 out]
                n490 = case shown="True" w2079 {
                  tunnel: w2080 -> [w2103 w2114]
                  tunnel: [w2091 w2113] -> w2090
                  tunnel: w2084 -> [w2102 w2112]
                  tunnel: w2089 -> [w2100 w2110]
                  tunnel: ["SendPartName" "Select"] -> w2088
                  tunnel: [w2092 w2106] -> w2087
                  tunnel: w2086 -> [w2097 w2105]
                  tunnel: [w2096 w2105] -> w2085
                  tunnel: w2082 -> [_ _]
                  frame True {
                    # "Master Sample Enabled"
                    n491 = Bundle By Name(cluster=w2100, "StateMsgToUI"="InitializeMasterSample") -> (w2093:T2)
                    n492 = Bundle By Name(cluster=w2097, "CurrentState"="MasterSamplePOST", "MasterSampleState"="MS:OkValidation" ("CurrentState")) -> (w2096:T1)
                    n493 = call "Output_SM.vi"("SM Private Data in"=w2102, "Output Cluster"=w2093, "Receiver Name"="UI", "State"="UI: StateMessage", "error in (no error)"=w2103) -> ("SM Private Data out"=w2092:refnum<class "Inspection Statemachine.lvclass">, "error out"=w2091:errorcluster)  [unwired: 9 in]
                  }
                  frame False {
                    # "Master Sample Not Enabled"
                    n494 = Bundle By Name(cluster=w2110, "StateMsgToUI"="DisplayInspectionPage>>Reset") -> (w2109:T2)
                    n495 = call "Output_SM.vi"("SM Private Data in"=w2112, "Output Cluster"=w2109, "Receiver Name"="UI", "State"="UI: StateMessage", "error in (no error)"=w2114) -> ("SM Private Data out"=w2106:refnum<class "Inspection Statemachine.lvclass">, "error out"=w2113:errorcluster)  [unwired: 9 in]
                  }
                }
              }
            }
          }
        }
        n496 = call <vilib>:"Add State(s) to Queue__JKI_lib_State_Machine.vi"("State(s) in Front (\"\")"=w1994, "State(s) in (\"\")"=w1997) -> ("States Out"=w1996:string)  [unwired: 13 in]
      }
      frame "ArduinoDiagnostics" {
        # "Wait for Diagnostic Result"
        n497 = in-place {
          in-place-border: [w2151] -> w2122
          in-place-border: w2120 -> [w2149]
          in-place-border: w2117 -> [w2133]
          in-place-border: [w2132] -> w2116
          n498 = in-place-cluster #5(w2119) -> ("SensorDiagnosticsStatus"=w2138:bool, "OutputCluster"=w2129:T2, "CameraOpticsDiagnosticsStatus"=w2126:bool)
          n499 = case shown="True" w2138 {
            tunnel: w2133 -> [w2163 w2176]
            tunnel: w2149 -> [w2164 w2177]
            tunnel: [w2164 w2169] -> w2128
            tunnel: w2129 -> [_ w2173]
            tunnel: [w2163 w2171] -> w2130
            frame False {
            }
            frame True {
              # "Stop to Cam Controller"
              n500 = Bundle By Name(cluster=w2173, "StateMsgToRC"="StopSensorDiagnostics", "StateMsgToMI"="HardwareReset") -> (w2165:T2)
              n501 = call "Output_SM.vi"("SM Private Data in"=w2176, "Output Cluster"=w2165, "Receiver Name"="RC", "State"="RC: StateMessge", "error in (no error)"=w2177) -> ("SM Private Data out"=w2172:refnum<class "Inspection Statemachine.lvclass">, "error out"=w2170:errorcluster)  [unwired: 9 in]
              n502 = call "Output_SM.vi"("SM Private Data in"=w2172, "Output Cluster"=w2165, "Receiver Name"="MI", "State"="MI: StateMessage", "error in (no error)"=w2170) -> ("SM Private Data out"=w2171:refnum<class "Inspection Statemachine.lvclass">, "error out"=w2169:errorcluster)  [unwired: 9 in]
            }
          }
          n503 = Unbundle By Name(w2129) -> ("SystemParameters.SoftwareFeatures.HardwareEmulated"=w2136:bool)
          n504 = case shown="True" w2126 {
            tunnel: w2130 -> [w2152 w2160]
            tunnel: w2128 -> [w2153 w2154]
            tunnel: [w2153 w2161] -> w2127
            tunnel: w2129 -> [_ w2157]
            tunnel: [w2152 w2155] -> w2125
            frame False {
            }
            frame True {
              # "Stop to Cam Controller"
              n505 = Bundle By Name(cluster=w2157, "StateMsgToRC"="StopCameraDiagnostics") -> (w2156:T2)
              n506 = call "Output_SM.vi"("SM Private Data in"=w2160, "Output Cluster"=w2156, "Receiver Name"="RC", "State"="RC: StateMessge", "error in (no error)"=w2154) -> ("SM Private Data out"=w2155:refnum<class "Inspection Statemachine.lvclass">, "error out"=w2161:errorcluster)  [unwired: 9 in]
            }
          }
          n507 = Bundle By Name(cluster=w2129, "PopupInput.Pop-up Type"=T8."Open Loading Bar" ("LoadingBarInput.Pop-up Type"), "PopupInput.Message"="Checking Timing Unit..." ("event data")) -> (w2148:T2)
          n508 = call "Output_SM.vi"("SM Private Data in"=w2125, "Output Cluster"=w2148, "Receiver Name"="UI", "State"="UI: DisplayPopup", "error in (no error)"=w2127) -> ("SM Private Data out"=w2134:refnum<class "Inspection Statemachine.lvclass">, "error out"=w2145:errorcluster)  [unwired: 9 in]
          n509 = Bundle By Name(cluster=w2129, "StateMsgToUI"="DisableAllButtons\nUpdateDiagnosticsStatusString>>Timing Unit Status") -> (w2141:T2)
          n510 = call "Output_SM.vi"("SM Private Data in"=w2134, "Output Cluster"=w2141, "Receiver Name"="UI", "State"="UI: StateMessage", "error in (no error)"=w2145) -> ("SM Private Data out"=w2135:refnum<class "Inspection Statemachine.lvclass">, "error out"=w2144:errorcluster)  [unwired: 9 in]
          n511 = case shown="False" w2136 {
            tunnel: [w2184 w2189] -> w2151
            tunnel: w2144 -> [w2186 w2189]
            tunnel: w2135 -> [w2185 w2188]
            tunnel: w2129 -> [w2181 _]
            tunnel: [w2179 w2188] -> w2132
            frame False {
              # "Online Execution"
              n512 = Bundle By Name(cluster=w2181, "StateMsgToMI"="DeviceReadiness" ("StateMessageToMI")) -> (w2180:T2)
              n513 = call "Output_SM.vi"("SM Private Data in"=w2185, "Output Cluster"=w2180, "Receiver Name"="MI", "State"="MI: StateMessage", "error in (no error)"=w2186) -> ("SM Private Data out"=w2179:refnum<class "Inspection Statemachine.lvclass">, "error out"=w2184:errorcluster)  [unwired: 9 in]
            }
            frame True {
              # "Offline Execution"
            }
          }
          n514 = in-place-cluster #5("SensorDiagnosticsStatus"=FALSE, "OutputCluster"=w2129, "CameraOpticsDiagnosticsStatus"=FALSE) -> (w2118:T1)
        }
        n515 = call <vilib>:"Add State(s) to Queue__JKI_lib_State_Machine.vi"("State(s) in Front (\"\")"="Wait" ("State(s) in Front (\"\")"), "State(s) in (\"\")"=w2124) -> ("States Out"=w2123:string)  [unwired: 13 in]
      }
      frame "Logout" {
        n516 = in-place {
          in-place-border: [w2205] -> w2195
          in-place-border: w2194 -> [w2203]
          in-place-border: w2191 -> [w2200]
          in-place-border: [w2204] -> w2190
          # "Sensor Diagnostics"
          n517 = in-place-cluster #6(w2193) -> ("SensorDiagnosticsStatus"=w2198:bool, "OutputCluster"=w2199:T2, "CameraOpticsDiagnosticsStatus"=w2206:bool)
          n518 = case shown="True" w2198 {
            tunnel: w2200 -> [w2209 w2222]
            tunnel: w2203 -> [w2210 w2223]
            tunnel: [w2210 w2215] -> w2202
            tunnel: w2199 -> [_ w2219]
            tunnel: [w2209 w2217] -> w2201
            frame False {
            }
            frame True {
              # "Stop to Cam Controller"
              n519 = Bundle By Name(cluster=w2219, "StateMsgToRC"="StopSensorDiagnostics", "StateMsgToMI"="HardwareReset") -> (w2211:T2)
              n520 = call "Output_SM.vi"("SM Private Data in"=w2222, "Output Cluster"=w2211, "Receiver Name"="RC", "State"="RC: StateMessge", "error in (no error)"=w2223) -> ("SM Private Data out"=w2218:refnum<class "Inspection Statemachine.lvclass">, "error out"=w2216:errorcluster)  [unwired: 9 in]
              n521 = call "Output_SM.vi"("SM Private Data in"=w2218, "Output Cluster"=w2211, "Receiver Name"="MI", "State"="MI: StateMessage", "error in (no error)"=w2216) -> ("SM Private Data out"=w2217:refnum<class "Inspection Statemachine.lvclass">, "error out"=w2215:errorcluster)  [unwired: 9 in]
            }
          }
          n522 = case shown="True" w2206 {
            tunnel: w2201 -> [w2225 w2239]
            tunnel: w2202 -> [w2226 w2235]
            tunnel: [w2226 w2231] -> w2205
            tunnel: w2199 -> [_ w2228]
            tunnel: [w2225 w2232] -> w2204
            frame False {
            }
            frame True {
              # "Stop to Cam Controller"
              n523 = Bundle By Name(cluster=w2228, "StateMsgToRC"="StopCameraDiagnostics") -> (w2236:T2)
              n524 = Bundle By Name(cluster=w2228, "Trigger Light Camera Sequence.Status"="Off") -> (w2229:T2)
              n525 = call "Output_SM.vi"("SM Private Data in"=w2239, "Output Cluster"=w2236, "Receiver Name"="RC", "State"="RC: StateMessge", "error in (no error)"=w2235) -> ("SM Private Data out"=w2234:refnum<class "Inspection Statemachine.lvclass">, "error out"=w2233:errorcluster)  [unwired: 9 in]
              n526 = Unbundle By Name(w2228) -> ("SystemParameters.SoftwareFeatures.HardwareEmulated"=w2227:bool)
              n527 = case shown="False" w2227 {
                tunnel: [w2245 w2249] -> w2231
                tunnel: w2233 -> [w2243 w2249]
                tunnel: w2234 -> [w2244 w2248]
                tunnel: [w2242 w2248] -> w2232
                tunnel: w2229 -> [w2241 _]
                frame False {
                  # "Online Execution"
                  n528 = call "Output_SM.vi"("SM Private Data in"=w2244, "Output Cluster"=w2241, "Receiver Name"="MI", "State"="MI: CameraOpticsDiagnostics", "error in (no error)"=w2243) -> ("SM Private Data out"=w2242:refnum<class "Inspection Statemachine.lvclass">, "error out"=w2245:errorcluster)  [unwired: 9 in]
                }
                frame True {
                  # "Offline Execution"
                }
              }
            }
          }
          n529 = in-place-cluster #6("SensorDiagnosticsStatus"=FALSE, "OutputCluster"=w2199, "CameraOpticsDiagnosticsStatus"=FALSE) -> (w2192:T1)
        }
        n530 = call <vilib>:"Add State(s) to Queue__JKI_lib_State_Machine.vi"("State(s) in (\"\")"=w2197) -> ("States Out"=w2196:string)  [unwired: 14 in]
      }
      frame "Initialization" {
        n531 = Unbundle By Name(w2253) -> ("OutputCluster.SystemParameters.SoftwareFeatures.HardwareEmulated"=w2256:bool, "OutputCluster"=w2252:T2)
        n532 = case shown="False" w2256 {
          tunnel: w2254 -> [w2264 w2269]
          tunnel: [w2265 w2269] -> w2255
          tunnel: w2251 -> [w2266 w2268]
          tunnel: w2252 -> [w2261 _]
          tunnel: [w2259 w2268] -> w2250
          frame False {
            # "Online Execution"
            n533 = Bundle By Name(cluster=w2261, "StateMsgToMI"="Initialization" ("StateMessageToMI")) -> (w2260:T2)
            n534 = call "Output_SM.vi"("SM Private Data in"=w2266, "Output Cluster"=w2260, "Receiver Name"="MI", "State"="MI: StateMessage", "error in (no error)"=w2264) -> ("SM Private Data out"=w2259:refnum<class "Inspection Statemachine.lvclass">, "error out"=w2265:errorcluster)  [unwired: 9 in]
          }
          frame True {
            # "Offline Execution"
          }
        }
        n535 = call <vilib>:"Add State(s) to Queue__JKI_lib_State_Machine.vi"("State(s) in (\"\")"=w2257) -> ("States Out"=w2258:string)  [unwired: 14 in]
      }
      frame "MotorDiagnostics" {
        n536 = in-place {
          in-place-border: [w2305] -> w2275
          in-place-border: w2274 -> [w2282]
          in-place-border: w2271 -> [w2281]
          in-place-border: [w2289] -> w2270
          # "Camera Diagnostics"
          # "Sensor Diagnostics"
          n537 = in-place-cluster #7(w2273) -> ("SensorDiagnosticsStatus"=w2279:bool, "OutputCluster"=w2280:T2, "CameraOpticsDiagnosticsStatus"=w2285:bool)
          n538 = case shown="True" w2279 {
            tunnel: w2281 -> [w2306 w2319]
            tunnel: w2282 -> [w2307 w2320]
            tunnel: [w2307 w2312] -> w2284
            tunnel: w2280 -> [_ w2316]
            tunnel: [w2306 w2314] -> w2283
            frame False {
            }
            frame True {
              # "Stop to Cam Controller"
              n539 = Bundle By Name(cluster=w2316, "StateMsgToRC"="StopSensorDiagnostics", "StateMsgToMI"="HardwareReset") -> (w2308:T2)
              n540 = call "Output_SM.vi"("SM Private Data in"=w2319, "Output Cluster"=w2308, "Receiver Name"="RC", "State"="RC: StateMessge", "error in (no error)"=w2320) -> ("SM Private Data out"=w2315:refnum<class "Inspection Statemachine.lvclass">, "error out"=w2313:errorcluster)  [unwired: 9 in]
              n541 = call "Output_SM.vi"("SM Private Data in"=w2315, "Output Cluster"=w2308, "Receiver Name"="MI", "State"="MI: StateMessage", "error in (no error)"=w2313) -> ("SM Private Data out"=w2314:refnum<class "Inspection Statemachine.lvclass">, "error out"=w2312:errorcluster)  [unwired: 9 in]
            }
          }
          n542 = Unbundle By Name(w2280) -> ("SystemParameters.SoftwareFeatures.HardwareEmulated"=w2292:bool)
          n543 = case shown="True" w2285 {
            tunnel: w2283 -> [w2322 w2329]
            tunnel: w2284 -> [w2323 w2330]
            tunnel: [w2323 w2331] -> w2286
            tunnel: w2280 -> [_ w2326]
            tunnel: [w2322 w2324] -> w2287
            frame False {
            }
            frame True {
              # "Stop to Cam Controller"
              n544 = Bundle By Name(cluster=w2326, "StateMsgToRC"="StopCameraDiagnostics") -> (w2325:T2)
              n545 = call "Output_SM.vi"("SM Private Data in"=w2329, "Output Cluster"=w2325, "Receiver Name"="RC", "State"="RC: StateMessge", "error in (no error)"=w2330) -> ("SM Private Data out"=w2324:refnum<class "Inspection Statemachine.lvclass">, "error out"=w2331:errorcluster)  [unwired: 9 in]
            }
          }
          n546 = Bundle By Name(cluster=w2280, "PopupInput.Pop-up Type"=T8."Open Loading Bar" ("LoadingBarInput.Pop-up Type"), "PopupInput.Message"="Checking Motor..." ("event data")) -> (w2304:T2)
          n547 = call "Output_SM.vi"("SM Private Data in"=w2287, "Output Cluster"=w2304, "Receiver Name"="UI", "State"="UI: DisplayPopup", "error in (no error)"=w2286) -> ("SM Private Data out"=w2291:refnum<class "Inspection Statemachine.lvclass">, "error out"=w2300:errorcluster)  [unwired: 9 in]
          n548 = Bundle By Name(cluster=w2280, "StateMsgToUI"="DisableAllButtons\nUpdateDiagnosticsStatusString>>Guide Motor Status") -> (w2295:T2)
          n549 = call "Output_SM.vi"("SM Private Data in"=w2291, "Output Cluster"=w2295, "Receiver Name"="UI", "State"="UI: StateMessage", "error in (no error)"=w2300) -> ("SM Private Data out"=w2290:refnum<class "Inspection Statemachine.lvclass">, "error out"=w2299:errorcluster)  [unwired: 9 in]
          n550 = case shown="False" w2292 {
            tunnel: [w2340 w2343] -> w2305
            tunnel: w2299 -> [w2339 w2343]
            tunnel: w2290 -> [w2338 w2342]
            tunnel: w2280 -> [w2335 _]
            tunnel: [w2333 w2342] -> w2289
            frame False {
              # "Online Execution"
              n551 = Bundle By Name(cluster=w2335, "StateMsgToMI"="MotorDiagnostics" ("StateMessageToMI")) -> (w2334:T2)
              n552 = call "Output_SM.vi"("SM Private Data in"=w2338, "Output Cluster"=w2334, "Receiver Name"="MI", "State"="MI: StateMessage", "error in (no error)"=w2339) -> ("SM Private Data out"=w2333:refnum<class "Inspection Statemachine.lvclass">, "error out"=w2340:errorcluster)  [unwired: 9 in]
            }
            frame True {
              # "Offline Execution"
            }
          }
          n553 = in-place-cluster #7("SensorDiagnosticsStatus"=FALSE, "OutputCluster"=w2280, "CameraOpticsDiagnosticsStatus"=FALSE) -> (w2272:T1)
        }
        n554 = call <vilib>:"Add State(s) to Queue__JKI_lib_State_Machine.vi"("State(s) in Front (\"\")"="Wait" ("State(s) in Front (\"\")"), "State(s) in (\"\")"=w2276) -> ("States Out"=w2278:string)  [unwired: 13 in]
      }
      frame "ObtainCameraIndex" {
        # "Do not put any code in this frame.\n(It is a separator no-op. You can make a copy of this frame to create a new UI frame)"
        # "Used Only During User Initiated Diagnostics"
        n555 = Unbundle By Name(w2346) -> ("OutputCluster.Camera Name"=w2350:string, "OutputCluster.CameraSequenceList"=w2351:cluster{"Name":string, "RackID":u8}[])
        n556 = for {
          tunnel: w2350 -> [w2357]
          tunnel: [w2360] -> w2352 if=w2359
          tunnel: w2351 -> [w2358] mode=indexing
          tunnel: w2344 -> [w2355]
          tunnel: [w2355] -> w2347
          i -> [w2360]
          stop <- w2359 stop-if-true
          # "Obtain Camera Index Value Based On User Input"
          n557 = Unbundle By Name(w2358) -> ("Name"=w2356:string)
          n558 = Equal?(x=w2357, y=w2356) -> (x = y?=w2359:bool)
        }
        n559 = Bundle By Name(cluster=w2346, "CameraIndex"=w2352) -> (w2349:T1)
        n560 = call <vilib>:"Add State(s) to Queue__JKI_lib_State_Machine.vi"("State(s) in Front (\"\")"="StartCameraDiagnostics" ("State(s) in Front (\"\")"), "State(s) in (\"\")"=w2354) -> ("States Out"=w2353:string)  [unwired: 13 in]
      }
      frame "StartCameraDiagnostics" {
        # "Wait for Diagnostic Result"
        # "Send Camera Details To UI, MI and RC"
        n561 = Unbundle By Name(w2371) -> ("OutputCluster.CameraSequenceList"=w2368:cluster{"Name":string, "RackID":u8}[], "CameraIndex"=w2365:i32, "OutputCluster.SystemParameters.SoftwareFeatures.HardwareEmulated"=w2367:bool, "OutputCluster"=w2364:T2)
        n562 = flat-sequence {
          tunnel: [w2380] -> w2362
          tunnel: w2361 -> [w2380]
          frame #0 {
            n563 = Wait (ms)(milliseconds to wait=1000) -> ()  [unwired: 1 out]
          }
        }
        n564 = Bundle By Name(cluster=w2371, "SensorDiagnosticsStatus"=FALSE) -> (w2370:T1)
        n565 = Array Size(array=w2368) -> (size(s)=w2366:i32)
        n566 = Equal?(x=w2366, y=w2365) -> (x = y?=w2374:bool)
        n567 = case shown="False" w2374 {
          tunnel: [w2384 w2411] -> w2372
          tunnel: [w2386 w2410] -> w2373
          tunnel: w2363 -> [w2387 w2392]
          tunnel: w2362 -> [w2385 w2393]
          tunnel: w2368 -> [_ w2402]
          tunnel: w2367 -> [_ w2401]
          tunnel: w2365 -> [_ w2400]
          tunnel: w2364 -> [w2383 w2398]
          tunnel: w2370 -> [w2390 w2397]
          tunnel: [w2388 w2395] -> w2369
          frame True {
            # "Camera Optics Diagnostics Done\nmessage to State message"
            # "Last Element of Camera Sequence List"
            n568 = call "Output_SM.vi"("SM Private Data in"=w2387, "Output Cluster"=w2383, "Receiver Name"="SM", "State"="SM: CamOpticsDiagnosticsResult", "error in (no error)"=w2385) -> ("SM Private Data out"=w2386:refnum<class "Inspection Statemachine.lvclass">, "error out"=w2384:errorcluster)  [unwired: 9 in]
            n569 = Bundle By Name(cluster=w2390, "CameraOpticsDiagnosticsStatus"=FALSE) -> (w2388:T1)
          }
          frame False {
            # "Have to Include a state for Sending Cam details to UI"
            # "Not the Last Element of Camera Sequence List"
            n570 = Index Array(array=w2402, index=w2400) -> (element=w2399:cluster{"Name":string, "RackID":u8})
            n571 = Unbundle By Name(w2399) -> ("Name"=w2406:string, "RackID"=w2405:u8)
            n572 = Bundle By Name(cluster=w2398, "Trigger Light Camera Sequence.Light Sequence Trigger"=w2406, "RackID"=w2405, "Trigger Light Camera Sequence.Status"="On", "Trigger Light Camera Sequence.Mode"="Continuous") -> (w2391:T2)
            n573 = case shown="False" w2401 {
              tunnel: [w2416 w2420] -> w2407
              tunnel: w2393 -> [w2414 w2420]
              tunnel: w2392 -> [w2415 w2419]
              tunnel: [w2413 w2419] -> w2408
              tunnel: w2391 -> [w2412 _]
              frame False {
                # "Online Execution"
                n574 = call "Output_SM.vi"("SM Private Data in"=w2415, "Output Cluster"=w2412, "Receiver Name"="MI", "State"="MI: CameraOpticsDiagnostics", "error in (no error)"=w2414) -> ("SM Private Data out"=w2413:refnum<class "Inspection Statemachine.lvclass">, "error out"=w2416:errorcluster)  [unwired: 9 in]
              }
              frame True {
                # "Offline Execution"
              }
            }
            n575 = Bundle By Name(cluster=w2397, "CameraOpticsDiagnosticsStatus"=TRUE, "OutputCluster"=w2391) -> (w2395:T1)
            n576 = call "Output_SM.vi"("SM Private Data in"=w2408, "Output Cluster"=w2391, "Receiver Name"="SingleRack", "State"="RC: CameraOpticsDiagnostics", "error in (no error)"=w2407) -> ("SM Private Data out"=w2410:refnum<class "Inspection Statemachine.lvclass">, "error out"=w2411:errorcluster)  [unwired: 9 in]
          }
        }
        n577 = call <vilib>:"Add State(s) to Queue__JKI_lib_State_Machine.vi"("State(s) in Front (\"\")"="Wait" ("State(s) in Front (\"\")"), "State(s) in (\"\")"=w2376) -> ("States Out"=w2378:string)  [unwired: 13 in]
      }
      frame "CameraOpticsDiagnostics" {
        # "Have to Include a state for Sending Cam details to UI"
        # "Send Camera Details To UI, MI and RC"
        n578 = Unbundle By Name(w2438) -> ("OutputCluster.SystemParameters.SoftwareFeatures.HardwareEmulated"=w2437:bool, "SensorDiagnosticsStatus"=w2421:bool, "OutputCluster"=w2422:T2)
        n579 = case shown="True" w2421 {
          tunnel: w2423 -> [w2442 w2455]
          tunnel: w2424 -> [w2443 w2456]
          tunnel: [w2443 w2448] -> w2426
          tunnel: w2422 -> [_ w2452]
          tunnel: [w2442 w2450] -> w2425
          frame False {
          }
          frame True {
            # "Stop to Cam Controller"
            n580 = Bundle By Name(cluster=w2452, "StateMsgToRC"="StopSensorDiagnostics", "StateMsgToMI"="HardwareReset") -> (w2444:T2)
            n581 = call "Output_SM.vi"("SM Private Data in"=w2455, "Output Cluster"=w2444, "Receiver Name"="RC", "State"="RC: StateMessge", "error in (no error)"=w2456) -> ("SM Private Data out"=w2451:refnum<class "Inspection Statemachine.lvclass">, "error out"=w2449:errorcluster)  [unwired: 9 in]
            n582 = call "Output_SM.vi"("SM Private Data in"=w2451, "Output Cluster"=w2444, "Receiver Name"="MI", "State"="MI: StateMessage", "error in (no error)"=w2449) -> ("SM Private Data out"=w2450:refnum<class "Inspection Statemachine.lvclass">, "error out"=w2448:errorcluster)  [unwired: 9 in]
          }
        }
        n583 = Bundle By Name(cluster=w2438, "SensorDiagnosticsStatus"=FALSE) -> (w2427:T1)
        n584 = Bundle By Name(cluster=w2422, "StateMsgToMI"="CameraOpticsDiagnostics", "StateMsgToUI"="UpdateDiagnosticsStatusString>>Camera Optics Diagnostics Status") -> (w2432:T2)
        n585 = call "Output_SM.vi"("SM Private Data in"=w2425, "Output Cluster"=w2432, "Receiver Name"="UI", "State"="UI: StateMessage", "error in (no error)"=w2426) -> ("SM Private Data out"=w2434:refnum<class "Inspection Statemachine.lvclass">, "error out"=w2435:errorcluster)  [unwired: 9 in]
        n586 = case shown="False" w2437 {
          tunnel: [w2462 w2466] -> w2429
          tunnel: w2435 -> [w2460 w2466]
          tunnel: w2434 -> [w2461 w2465]
          tunnel: [w2459 w2465] -> w2428
          tunnel: w2432 -> [w2458 _]
          frame False {
            # "Online Execution"
            n587 = call "Output_SM.vi"("SM Private Data in"=w2461, "Output Cluster"=w2458, "Receiver Name"="MI", "State"="MI: StateMessage", "error in (no error)"=w2460) -> ("SM Private Data out"=w2459:refnum<class "Inspection Statemachine.lvclass">, "error out"=w2462:errorcluster)  [unwired: 9 in]
          }
          frame True {
            # "Offline Execution"
          }
        }
        n588 = call <vilib>:"Add State(s) to Queue__JKI_lib_State_Machine.vi"("State(s) in (\"\")"=w2440) -> ("States Out"=w2441:string)  [unwired: 14 in]
      }
      frame "CameraOpticsAnalysis" {
        # "Display The Diagnostics Result"
        n589 = Unbundle By Name(w2474) -> ("OutputCluster.SystemParameters.SoftwareFeatures.HardwareEmulated"=w2470:bool, "CameraIndex"=w2477:i32, "OutputCluster.CameraOpticsDiagnosticsResult.Result"=w2476:bool, "CurrentState"=w2480:string, "OutputCluster"=w2467:T2)
        n590 = case shown="\"POST\", Default" w2480 {
          tunnel: w2476 -> [w2484 w2532]
          tunnel: w2477 -> [w2493 w2539]
          tunnel: [w2492 w2531] -> w2478
          tunnel: ["StartCameraDiagnostics" w2538] -> w2475
          tunnel: w2467 -> [w2490 w2536]
          tunnel: w2468 -> [w2489 w2537]
          tunnel: [w2488 w2535] -> w2472
          tunnel: w2469 -> [w2487 w2534]
          tunnel: [w2486 w2533] -> w2471
          tunnel: [w2485 w2530] -> w2479
          tunnel: w2470 -> [w2483 w2529]
          frame "POST", Default {
            n591 = case shown="False" w2484 {
              tunnel: w2493 -> [w2495 w2510]
              tunnel: [w2495 w2519] -> w2492
              tunnel: w2490 -> [w2494 w2509]
              tunnel: w2489 -> [w2499 w2518]
              tunnel: [w2498 w2507] -> w2488
              tunnel: w2487 -> [w2497 w2515]
              tunnel: [w2496 w2505] -> w2486
              tunnel: [w2494 w2504] -> w2485
              tunnel: w2483 -> [_ w2503]
              frame False {
                # "The same Camera is Triggered"
                n592 = call "Output_SM.vi"("SM Private Data in"=w2499, "Output Cluster"=w2494, "Receiver Name"="UI", "State"="UI: CameraOpticsDiagnosticsResult", "error in (no error)"=w2497) -> ("SM Private Data out"=w2498:refnum<class "Inspection Statemachine.lvclass">, "error out"=w2496:errorcluster)  [unwired: 9 in]
              }
              frame True {
                # "Goes to Next Camera in the Camera Sequence List"
                n593 = Bundle By Name(cluster=w2509, "Trigger Light Camera Sequence.Status"="Off" ("Status")) -> (w2504:T2)
                n594 = call "Output_SM.vi"("SM Private Data in"=w2518, "Output Cluster"=w2504, "Receiver Name"="UI", "State"="UI: CameraOpticsDiagnosticsResult", "error in (no error)"=w2515) -> ("SM Private Data out"=w2514:refnum<class "Inspection Statemachine.lvclass">, "error out"=w2513:errorcluster)  [unwired: 9 in]
                n595 = Increment(x=w2510) -> (x+1=w2519:i32)
                n596 = call "Output_SM.vi"("SM Private Data in"=w2514, "Output Cluster"=w2504, "Receiver Name"="SingleRack", "State"="RC: CameraOpticsDiagnostics", "error in (no error)"=w2513) -> ("SM Private Data out"=w2508:refnum<class "Inspection Statemachine.lvclass">, "error out"=w2506:errorcluster)  [unwired: 9 in]
                n597 = case shown="False" w2503 {
                  tunnel: w2508 -> [w2521 w2528]
                  tunnel: [w2521 w2527] -> w2507
                  tunnel: w2506 -> [w2520 w2526]
                  tunnel: [w2520 w2525] -> w2505
                  tunnel: w2504 -> [_ w2524]
                  frame True {
                    # "Offline Execution"
                  }
                  frame False {
                    # "Online Execution"
                    n598 = call "Output_SM.vi"("SM Private Data in"=w2528, "Output Cluster"=w2524, "Receiver Name"="MI", "State"="MI: CameraOpticsDiagnostics", "error in (no error)"=w2526) -> ("SM Private Data out"=w2527:refnum<class "Inspection Statemachine.lvclass">, "error out"=w2525:errorcluster)  [unwired: 9 in]
                  }
                }
              }
            }
          }
          frame "CameraOpticsDiagnostics" {
            n599 = case shown="True" w2532 {
              tunnel: w2539 -> [w2548 w2567]
              tunnel: [w2548 w2567] -> w2531
              tunnel: ["Wait" "Wait"] -> w2538
              tunnel: w2537 -> [w2546 w2557]
              tunnel: w2536 -> [w2540 w2558]
              tunnel: [w2543 w2554] -> w2535
              tunnel: w2534 -> [w2542 w2563]
              tunnel: [w2541 w2555] -> w2533
              tunnel: [w2540 w2551] -> w2530
              tunnel: w2529 -> [_ w2552]
              frame False {
                # "Triggers the Same Camera"
                n600 = call "Output_SM.vi"("SM Private Data in"=w2546, "Output Cluster"=w2540, "Receiver Name"="UI", "State"="UI: CameraOpticsDiagnosticsResult", "error in (no error)"=w2542) -> ("SM Private Data out"=w2543:refnum<class "Inspection Statemachine.lvclass">, "error out"=w2541:errorcluster)  [unwired: 9 in]
              }
              frame True {
                # "Waits For User To Choose the Next Camera"
                n601 = Bundle By Name(cluster=w2558, "Trigger Light Camera Sequence.Status"="Off" ("Status"), "Trigger Light Camera Sequence.Mode"="") -> (w2551:T2)
                n602 = call "Output_SM.vi"("SM Private Data in"=w2557, "Output Cluster"=w2551, "Receiver Name"="UI", "State"="UI: CameraOpticsDiagnosticsResult", "error in (no error)"=w2563) -> ("SM Private Data out"=w2562:refnum<class "Inspection Statemachine.lvclass">, "error out"=w2561:errorcluster)  [unwired: 9 in]
                n603 = call "Output_SM.vi"("SM Private Data in"=w2562, "Output Cluster"=w2551, "Receiver Name"="SingleRack", "State"="RC: CameraOpticsDiagnostics", "error in (no error)"=w2561) -> ("SM Private Data out"=w2556:refnum<class "Inspection Statemachine.lvclass">, "error out"=w2553:errorcluster)  [unwired: 9 in]
                n604 = case shown="False" w2552 {
                  tunnel: w2556 -> [w2569 w2576]
                  tunnel: [w2568 w2575] -> w2555
                  tunnel: [w2569 w2574] -> w2554
                  tunnel: w2553 -> [w2568 w2573]
                  tunnel: w2551 -> [_ w2572]
                  frame True {
                    # "Offline Execution"
                  }
                  frame False {
                    # "Online Execution"
                    n605 = call "Output_SM.vi"("SM Private Data in"=w2576, "Output Cluster"=w2572, "Receiver Name"="MI", "State"="MI: CameraOpticsDiagnostics", "error in (no error)"=w2573) -> ("SM Private Data out"=w2574:refnum<class "Inspection Statemachine.lvclass">, "error out"=w2575:errorcluster)  [unwired: 9 in]
                  }
                }
              }
            }
          }
        }
        n606 = Bundle By Name(cluster=w2474, "CameraIndex"=w2478, "OutputCluster"=w2479) -> (w2473:T1)
        n607 = call <vilib>:"Add State(s) to Queue__JKI_lib_State_Machine.vi"("State(s) in Front (\"\")"=w2475, "State(s) in (\"\")"=w2482) -> ("States Out"=w2481:string)  [unwired: 13 in]
      }
      frame "ObtainSensorIndex" {
        n608 = Unbundle By Name(w2577) -> ("OutputCluster.SystemParameters.SoftwareFeatures.HardwareEmulated"=w2579:bool, "OutputCluster"=w2578:T2)
        n609 = call "Output_SM.vi"("SM Private Data in"=w2585, "Output Cluster"=w2578, "Receiver Name"="RC", "State"="RC: SensorDiagnostics", "error in (no error)"=w2587) -> ("SM Private Data out"=w2583:refnum<class "Inspection Statemachine.lvclass">, "error out"=w2582:errorcluster)  [unwired: 9 in]
        n610 = case shown="False" w2579 {
          tunnel: w2583 -> [w2597 w2604]
          tunnel: w2582 -> [w2596 w2603]
          tunnel: [w2596 w2600] -> w2588
          tunnel: [w2597 w2599] -> w2584
          tunnel: w2578 -> [_ w2598]
          frame True {
            # "Offline execution"
          }
          frame False {
            # "Online execution"
            n611 = call "Output_SM.vi"("SM Private Data in"=w2604, "Output Cluster"=w2598, "Receiver Name"="MI", "State"="MI: SensorDiagnostics", "error in (no error)"=w2603) -> ("SM Private Data out"=w2599:refnum<class "Inspection Statemachine.lvclass">, "error out"=w2600:errorcluster)  [unwired: 9 in]
          }
        }
        n612 = Unbundle By Name(w2577) -> ("OutputCluster.Sensor Name"=w2591:string, "OutputCluster.SensorList"=w2592:cluster{"Name":string, "RackID":u8}[])
        n613 = for {
          tunnel: w2591 -> [w2607]
          tunnel: [w2610] -> w2593 if=w2609
          tunnel: w2592 -> [w2608] mode=indexing
          shift-right: [w2605] -> w2586
          shift-left: w2588 -> [w2605]
          i -> [w2610]
          stop <- w2609 stop-if-true
          # "Obtain Sensor Index Value Based On User Input"
          n614 = Unbundle By Name(w2608) -> ("Name"=w2606:string)
          n615 = Equal?(x=w2607, y=w2606) -> (x = y?=w2609:bool)
        }
        n616 = Bundle By Name(cluster=w2577, "SensorIndex"=w2593) -> (w2590:T1)
        n617 = call <vilib>:"Add State(s) to Queue__JKI_lib_State_Machine.vi"("State(s) in Front (\"\")"="StartSensorDiagnostics" ("State(s) in Front (\"\")"), "State(s) in (\"\")"=w2595) -> ("States Out"=w2594:string)  [unwired: 13 in]
      }
      frame "StartSensorDiagnostics" {
        # "Wait for Diagnostic Result"
        # "Send Sensor Details To UI, MI and RC"
        n618 = Unbundle By Name(w2630) -> ("OutputCluster.SystemParameters.SoftwareFeatures.HardwareEmulated"=w2619:bool, "OutputCluster.SensorList"=w2618:cluster{"Name":string, "RackID":u8}[], "SensorIndex"=w2617:i32, "CameraOpticsDiagnosticsStatus"=w2629:bool, "OutputCluster"=w2613:T2)
        n619 = case shown="True" w2629 {
          tunnel: w2635 -> [w2649 w2657]
          tunnel: [w2649 w2656] -> w2611
          tunnel: w2633 -> [w2648 w2658]
          tunnel: w2613 -> [_ w2651]
          tunnel: [w2648 w2655] -> w2612
          frame False {
          }
          frame True {
            # "Stop to Cam Controller"
            n620 = Bundle By Name(cluster=w2651, "StateMsgToRC"="StopCameraDiagnostics") -> (w2652:T2)
            n621 = call "Output_SM.vi"("SM Private Data in"=w2658, "Output Cluster"=w2652, "Receiver Name"="SingleRack", "State"="RC: StateMessage", "error in (no error)"=w2657) -> ("SM Private Data out"=w2655:refnum<class "Inspection Statemachine.lvclass">, "error out"=w2656:errorcluster)  [unwired: 9 in]
          }
        }
        n622 = Index Array(array=w2618, index=w2617) -> (element=w2616:cluster{"Name":string, "RackID":u8})
        n623 = Bundle By Name(cluster=w2630, "CameraOpticsDiagnosticsStatus"=FALSE ("SensorDiagnosticsStatus"), "SensorDiagnosticsStatus"=TRUE ("CameraOpticsDiagnosticsStatus")) -> (w2621:T1)
        n624 = Unbundle By Name(w2616) -> ("Name"=w2615:string, "RackID"=w2614:u8)
        n625 = Bundle By Name(cluster=w2613, "Sensor Name"=w2615, "RackID"=w2614) -> (w2620:T2)
        n626 = case shown="False" w2619 {
          tunnel: [w2643 w2647] -> w2626
          tunnel: w2611 -> [w2641 w2647]
          tunnel: w2612 -> [w2642 w2646]
          tunnel: [w2640 w2646] -> w2627
          tunnel: w2620 -> [w2639 _]
          frame False {
            # "Online Execution"
            n627 = call "Output_SM.vi"("SM Private Data in"=w2642, "Output Cluster"=w2639, "Receiver Name"="MI", "State"="MI: SensorDiagnostics", "error in (no error)"=w2641) -> ("SM Private Data out"=w2640:refnum<class "Inspection Statemachine.lvclass">, "error out"=w2643:errorcluster)  [unwired: 9 in]
          }
          frame True {
            # "Offline Execution"
          }
        }
        n628 = call <vilib>:"Add State(s) to Queue__JKI_lib_State_Machine.vi"("State(s) in Front (\"\")"="Wait" ("State(s) in Front (\"\")"), "State(s) in (\"\")"=w2636) -> ("States Out"=w2638:string)  [unwired: 13 in]
        n629 = Bundle By Name(cluster=w2620, "StateMsgToRC"="SensorDiagnostics" ("StateMessageToMI")) -> (w2624:T2)
        n630 = call "Output_SM.vi"("SM Private Data in"=w2627, "Output Cluster"=w2624, "Receiver Name"="SingleRack", "State"="RC: StateMessage", "error in (no error)"=w2626) -> ("SM Private Data out"=w2632:refnum<class "Inspection Statemachine.lvclass">, "error out"=w2631:errorcluster)  [unwired: 9 in]
      }
      frame "ReelerMotor" {
        n631 = in-place {
          in-place-border: [w2681] -> w2664
          in-place-border: w2663 -> [w2671]
          in-place-border: w2660 -> [w2670]
          in-place-border: [w2678] -> w2659
          n632 = in-place-cluster #8(w2662) -> ("SensorDiagnosticsStatus"=w2668:bool, "OutputCluster"=w2669:T2, "CameraOpticsDiagnosticsStatus"=w2675:bool)
          n633 = case shown="True" w2668 {
            tunnel: w2670 -> [w2682 w2695]
            tunnel: w2671 -> [w2683 w2696]
            tunnel: [w2683 w2688] -> w2673
            tunnel: w2669 -> [_ w2692]
            tunnel: [w2682 w2690] -> w2672
            frame False {
            }
            frame True {
              # "Stop to Cam Controller"
              n634 = Bundle By Name(cluster=w2692, "StateMsgToRC"="StopSensorDiagnostics", "StateMsgToMI"="HardwareReset") -> (w2684:T2)
              n635 = call "Output_SM.vi"("SM Private Data in"=w2695, "Output Cluster"=w2684, "Receiver Name"="RC", "State"="RC: StateMessge", "error in (no error)"=w2696) -> ("SM Private Data out"=w2691:refnum<class "Inspection Statemachine.lvclass">, "error out"=w2689:errorcluster)  [unwired: 9 in]
              n636 = call "Output_SM.vi"("SM Private Data in"=w2691, "Output Cluster"=w2684, "Receiver Name"="MI", "State"="MI: StateMessage", "error in (no error)"=w2689) -> ("SM Private Data out"=w2690:refnum<class "Inspection Statemachine.lvclass">, "error out"=w2688:errorcluster)  [unwired: 9 in]
            }
          }
          n637 = Unbundle By Name(w2669) -> ("SystemParameters.SoftwareFeatures.HardwareEmulated"=w2679:bool)
          n638 = case shown="True" w2675 {
            tunnel: w2672 -> [w2698 w2705]
            tunnel: w2673 -> [w2699 w2706]
            tunnel: [w2699 w2707] -> w2676
            tunnel: w2669 -> [_ w2702]
            tunnel: [w2698 w2700] -> w2677
            frame False {
            }
            frame True {
              # "Stop to Cam Controller"
              n639 = Bundle By Name(cluster=w2702, "StateMsgToRC"="StopCameraDiagnostics") -> (w2701:T2)
              n640 = call "Output_SM.vi"("SM Private Data in"=w2705, "Output Cluster"=w2701, "Receiver Name"="RC", "State"="RC: StateMessge", "error in (no error)"=w2706) -> ("SM Private Data out"=w2700:refnum<class "Inspection Statemachine.lvclass">, "error out"=w2707:errorcluster)  [unwired: 9 in]
            }
          }
          n641 = case shown="False" w2679 {
            tunnel: [w2710 w2719] -> w2681
            tunnel: w2676 -> [w2713 w2719]
            tunnel: w2677 -> [w2711 w2718]
            tunnel: w2669 -> [w2712 _]
            tunnel: [w2709 w2718] -> w2678
            frame False {
              # "Online Execution"
              n642 = Bundle By Name(cluster=w2712, "StateMsgToMI"="RotateReelerMotor" ("StateMessageToMI")) -> (w2714:T2)
              n643 = call "Output_SM.vi"("SM Private Data in"=w2711, "Output Cluster"=w2714, "Receiver Name"="MI", "State"="MI: StateMessage", "error in (no error)"=w2713) -> ("SM Private Data out"=w2709:refnum<class "Inspection Statemachine.lvclass">, "error out"=w2710:errorcluster)  [unwired: 9 in]
            }
            frame True {
              # "Offline Execution"
            }
          }
          n644 = in-place-cluster #8("SensorDiagnosticsStatus"=FALSE, "OutputCluster"=w2669, "CameraOpticsDiagnosticsStatus"=FALSE) -> (w2661:T1)
        }
        n645 = call <vilib>:"Add State(s) to Queue__JKI_lib_State_Machine.vi"("State(s) in Front (\"\")"="Wait" ("State(s) in Front (\"\")"), "State(s) in (\"\")"=w2665) -> ("States Out"=w2667:string)  [unwired: 13 in]
      }
      frame "TowerLampDiagnostics" {
        n646 = in-place {
          in-place-border: [w2742] -> w2725
          in-place-border: w2724 -> [w2731]
          in-place-border: w2721 -> [w2732]
          in-place-border: [w2739] -> w2720
          # "Camera Diagnostics"
          n647 = in-place-cluster #9(w2723) -> ("SensorDiagnosticsStatus"=w2729:bool, "OutputCluster"=w2730:T2, "CameraOpticsDiagnosticsStatus"=w2735:bool)
          n648 = case shown="True" w2729 {
            tunnel: w2732 -> [w2743 w2756]
            tunnel: w2731 -> [w2744 w2757]
            tunnel: [w2744 w2749] -> w2733
            tunnel: w2730 -> [_ w2753]
            tunnel: [w2743 w2751] -> w2734
            frame False {
            }
            frame True {
              # "Stop to Cam Controller"
              n649 = Bundle By Name(cluster=w2753, "StateMsgToRC"="StopSensorDiagnostics", "StateMsgToMI"="HardwareReset") -> (w2745:T2)
              n650 = call "Output_SM.vi"("SM Private Data in"=w2756, "Output Cluster"=w2745, "Receiver Name"="RC", "State"="RC: StateMessge", "error in (no error)"=w2757) -> ("SM Private Data out"=w2752:refnum<class "Inspection Statemachine.lvclass">, "error out"=w2750:errorcluster)  [unwired: 9 in]
              n651 = call "Output_SM.vi"("SM Private Data in"=w2752, "Output Cluster"=w2745, "Receiver Name"="MI", "State"="MI: StateMessage", "error in (no error)"=w2750) -> ("SM Private Data out"=w2751:refnum<class "Inspection Statemachine.lvclass">, "error out"=w2749:errorcluster)  [unwired: 9 in]
            }
          }
          n652 = Unbundle By Name(w2730) -> ("SystemParameters.SoftwareFeatures.HardwareEmulated"=w2740:bool)
          n653 = case shown="True" w2735 {
            tunnel: w2734 -> [w2759 w2766]
            tunnel: w2733 -> [w2760 w2767]
            tunnel: [w2760 w2768] -> w2736
            tunnel: w2730 -> [_ w2763]
            tunnel: [w2759 w2761] -> w2737
            frame False {
            }
            frame True {
              # "Stop to Cam Controller"
              n654 = Bundle By Name(cluster=w2763, "StateMsgToRC"="StopCameraDiagnostics") -> (w2762:T2)
              n655 = call "Output_SM.vi"("SM Private Data in"=w2766, "Output Cluster"=w2762, "Receiver Name"="RC", "State"="RC: StateMessge", "error in (no error)"=w2767) -> ("SM Private Data out"=w2761:refnum<class "Inspection Statemachine.lvclass">, "error out"=w2768:errorcluster)  [unwired: 9 in]
            }
          }
          n656 = case shown="False" w2740 {
            tunnel: [w2774 w2780] -> w2742
            tunnel: w2736 -> [w2773 w2780]
            tunnel: w2737 -> [w2771 w2779]
            tunnel: w2730 -> [w2772 _]
            tunnel: [w2770 w2779] -> w2739
            frame False {
              # "Online Execution"
              n657 = Bundle By Name(cluster=w2772, "StateMsgToMI"="TowerLampDiagnostics" ("StateMessageToMI")) -> (w2775:T2)
              n658 = call "Output_SM.vi"("SM Private Data in"=w2771, "Output Cluster"=w2775, "Receiver Name"="MI", "State"="MI: StateMessage", "error in (no error)"=w2773) -> ("SM Private Data out"=w2770:refnum<class "Inspection Statemachine.lvclass">, "error out"=w2774:errorcluster)  [unwired: 9 in]
            }
            frame True {
              # "Offline Execution"
            }
          }
          n659 = in-place-cluster #9("SensorDiagnosticsStatus"=FALSE, "OutputCluster"=w2730, "CameraOpticsDiagnosticsStatus"=FALSE) -> (w2722:T1)
        }
        n660 = call <vilib>:"Add State(s) to Queue__JKI_lib_State_Machine.vi"("State(s) in Front (\"\")"="Wait" ("State(s) in Front (\"\")"), "State(s) in (\"\")"=w2726) -> ("States Out"=w2728:string)  [unwired: 13 in]
      }
      frame "HardwareButtonDiagnostics" {
        n661 = in-place {
          in-place-border: [w2804] -> w2786
          in-place-border: w2785 -> [w2794]
          in-place-border: w2782 -> [w2793]
          in-place-border: [w2800] -> w2781
          n662 = in-place-cluster #10(w2784) -> ("SensorDiagnosticsStatus"=w2791:bool, "OutputCluster"=w2792:T2, "CameraOpticsDiagnosticsStatus"=w2796:bool)  [unwired: 1 out]
          n663 = Unbundle By Name(w2792) -> ("SystemParameters.SoftwareFeatures.HardwareEmulated"=w2801:bool)
          n664 = case shown="True" w2791 {
            tunnel: w2793 -> [w2805 w2818]
            tunnel: w2794 -> [w2806 w2819]
            tunnel: [w2806 w2811] -> w2790
            tunnel: w2792 -> [_ w2815]
            tunnel: [w2805 w2813] -> w2795
            frame False {
            }
            frame True {
              # "Stop to Cam Controller"
              n665 = Bundle By Name(cluster=w2815, "StateMsgToRC"="StopSensorDiagnostics", "StateMsgToMI"="HardwareReset") -> (w2807:T2)
              n666 = call "Output_SM.vi"("SM Private Data in"=w2818, "Output Cluster"=w2807, "Receiver Name"="RC", "State"="RC: StateMessge", "error in (no error)"=w2819) -> ("SM Private Data out"=w2814:refnum<class "Inspection Statemachine.lvclass">, "error out"=w2812:errorcluster)  [unwired: 9 in]
              n667 = call "Output_SM.vi"("SM Private Data in"=w2814, "Output Cluster"=w2807, "Receiver Name"="MI", "State"="MI: StateMessage", "error in (no error)"=w2812) -> ("SM Private Data out"=w2813:refnum<class "Inspection Statemachine.lvclass">, "error out"=w2811:errorcluster)  [unwired: 9 in]
            }
          }
          n668 = case shown="True" w2796 {
            tunnel: w2795 -> [w2821 w2828]
            tunnel: w2790 -> [w2822 w2829]
            tunnel: [w2822 w2830] -> w2797
            tunnel: w2792 -> [_ w2825]
            tunnel: [w2821 w2823] -> w2798
            frame False {
            }
            frame True {
              # "Stop to Cam Controller"
              n669 = Bundle By Name(cluster=w2825, "StateMsgToRC"="StopCameraDiagnostics") -> (w2824:T2)
              n670 = call "Output_SM.vi"("SM Private Data in"=w2828, "Output Cluster"=w2824, "Receiver Name"="RC", "State"="RC: StateMessge", "error in (no error)"=w2829) -> ("SM Private Data out"=w2823:refnum<class "Inspection Statemachine.lvclass">, "error out"=w2830:errorcluster)  [unwired: 9 in]
            }
          }
          n671 = case shown="False" w2801 {
            tunnel: [w2836 w2842] -> w2804
            tunnel: w2797 -> [w2835 w2842]
            tunnel: w2798 -> [w2834 w2841]
            tunnel: w2792 -> [w2833 _]
            tunnel: [w2832 w2841] -> w2800
            frame False {
              # "Online Execution"
              n672 = Bundle By Name(cluster=w2833, "StateMsgToMI"="HardwareButtonDiagnostics" ("StateMessageToMI")) -> (w2837:T2)
              n673 = call "Output_SM.vi"("SM Private Data in"=w2834, "Output Cluster"=w2837, "Receiver Name"="MI", "State"="MI: StateMessage", "error in (no error)"=w2835) -> ("SM Private Data out"=w2832:refnum<class "Inspection Statemachine.lvclass">, "error out"=w2836:errorcluster)  [unwired: 9 in]
            }
            frame True {
              # "Offline Execution"
            }
          }
          n674 = in-place-cluster #10("SensorDiagnosticsStatus"=FALSE, "OutputCluster"=w2792, "CurrentState"="HardwareButtonDiagnostics" ("Previous State"), "CameraOpticsDiagnosticsStatus"=FALSE) -> (w2783:T1)
        }
        n675 = call <vilib>:"Add State(s) to Queue__JKI_lib_State_Machine.vi"("State(s) in Front (\"\")"="Wait" ("State(s) in Front (\"\")"), "State(s) in (\"\")"=w2787) -> ("States Out"=w2789:string)  [unwired: 13 in]
      }
      frame "---------- Select State ----------" {
        # "Do not put any code in this frame.\n(It is a separator no-op. You can make a copy of this frame to create a new UI frame)"
        n676 = call <vilib>:"Add State(s) to Queue__JKI_lib_State_Machine.vi"("State(s) in (\"\")"=w2847) -> ("States Out"=w2846:string)  [unwired: 14 in]
      }
      frame "Select" {
        n677 = Unbundle By Name(w2855) -> ("OutputCluster.SystemParameters.SoftwareFeatures.DataLoggingEnable"=w2848:bool, "OutputCluster.SystemParameters.SoftwareFeatures.HardwareEmulated"=w2857:bool, "OutputCluster"=w2850:T2)
        n678 = case shown="False" w2857 {
          tunnel: w2858 -> [w2877 w2885]
          tunnel: [w2876 w2885] -> w2852
          tunnel: w2856 -> [w2879 w2884]
          tunnel: w2850 -> [w2878 _]
          tunnel: [w2875 w2884] -> w2854
          frame False {
            # "Online Execution"
            n679 = Bundle By Name(cluster=w2878, "StateMsgToMI"="Select" ("StateMessageToMI")) -> (w2880:T2)
            n680 = call "Output_SM.vi"("SM Private Data in"=w2879, "Output Cluster"=w2880, "Receiver Name"="MI", "State"="MI: StateMessage", "error in (no error)"=w2877) -> ("SM Private Data out"=w2875:refnum<class "Inspection Statemachine.lvclass">, "error out"=w2876:errorcluster)  [unwired: 9 in]
          }
          frame True {
            # "Offline Execution"
          }
        }
        n681 = case shown="True" w2848 {
          tunnel: w2854 -> [w2863 w2870]
          tunnel: [w2863 w2869] -> w2853
          tunnel: w2852 -> [w2864 w2868]
          tunnel: [w2864 w2867] -> w2851
          tunnel: w2850 -> [_ w2865]
          frame False {
            # "DL Disable"
          }
          frame True {
            # "DL Enable"
            n682 = Bundle By Name(cluster=w2865, "EventData.EventName"="Ready" ("DataLogger.EventDetails.EventName"), "EventData.EventReason"="Inspection Ready" ("DataLogger.EventDetails.EventReason")) -> (w2866:T2)
            n683 = call "Output_SM.vi"("SM Private Data in"=w2870, "Output Cluster"=w2866, "Receiver Name"="DL", "State"="DL: EventDetails", "error in (no error)"=w2868) -> ("SM Private Data out"=w2869:refnum<class "Inspection Statemachine.lvclass">, "error out"=w2867:errorcluster)  [unwired: 9 in]
          }
        }
        n684 = Bundle By Name(cluster=w2855, "CurrentState"="Select" ("Previous State"), "OutputCluster.PartInfo.PartName"="") -> (w2860:T1)
        n685 = call <vilib>:"Add State(s) to Queue__JKI_lib_State_Machine.vi"("State(s) in (\"\")"=w2861) -> ("States Out"=w2862:string)  [unwired: 14 in]
      }
      frame "SendPartName" {
        n686 = Unbundle By Name(w2890) -> ("CurrentState"=w2889:string, "OutputCluster.SystemParameters.SoftwareFeatures.HardwareEmulated"=w2886:bool)
        n687 = case shown="Default" w2889 {
          tunnel: ["Master Sample" ("PartName") w2906] -> w2888
          tunnel: w2890 -> [_ w2911]
          tunnel: [u8 1 w2907] -> w2887
          frame "MasterSampleDiagnostics", "MasterSamplePOST" {
            # "Master Sample"
          }
          frame Default {
            n688 = Unbundle By Name(w2911) -> ("OutputCluster.PartsConfigured"=w2909:cluster{"Name":string, "NumberOfRack":u8}[], "OutputCluster.PartInfo.PartName"=w2908:string)
            n689 = for {
              tunnel: w2909 -> [w2920] mode=indexing
              tunnel: w2908 -> [w2918]
              tunnel: w2909 -> [w2916]
              tunnel: [w2913] -> w2910
              i -> [w2915]
              stop <- w2912 stop-if-true
              n690 = Unbundle By Name(w2920) -> ("Name"=w2919:string)
              n691 = Equal?(x=w2919, y=w2918) -> (x = y?=w2912:bool)
              n692 = Index Array(array=w2916, index=w2915) -> (element=w2914:cluster{"Name":string, "NumberOfRack":u8})
              n693 = Select(t=w2914, s=w2912, f=cluster{"Name":string, "NumberOfRack":i32} {"Name"="", "NumberOfRack"=0} ("Cluster")) -> (s? t:f=w2913:cluster{"Name":string, "NumberOfRack":i32})
            }
            n694 = Unbundle By Name(w2910) -> ("Name"=w2906:string, "NumberOfRack"=w2907:i32)
          }
        }
        n695 = Bundle By Name(cluster=w2890, "OutputCluster.PartInfo.PartName"=w2888, "OutputCluster.PartInfo.NumberOfRacks"=w2887) -> (w2896:T1)
        n696 = Unbundle By Name(w2896) -> ("OutputCluster"=w2895:T2)
        n697 = case shown="True" w2886 {
          tunnel: w2895 -> [w2923 _]
          tunnel: w2898 -> [w2927 w2929]
          tunnel: [w2926 w2929] -> w2897
          tunnel: w2892 -> [w2925 w2928]
          tunnel: [w2921 w2928] -> w2893
          frame False {
            # "Online Execution"
            n698 = call "Output_SM.vi"("SM Private Data in"=w2925, "Output Cluster"=w2923, "Receiver Name"="MI", "State"="MI: PartName", "error in (no error)"=w2927) -> ("SM Private Data out"=w2921:refnum<class "Inspection Statemachine.lvclass">, "error out"=w2926:errorcluster)  [unwired: 9 in]
          }
          frame True {
            # "Offline Execution"
          }
        }
        n699 = call "Output_SM.vi"("SM Private Data in"=w2893, "Output Cluster"=w2895, "Receiver Name"="RC", "State"="RC: SelectedPartInfo", "error in (no error)"=w2897) -> ("SM Private Data out"=w2891:refnum<class "Inspection Statemachine.lvclass">, "error out"=w2900:errorcluster)  [unwired: 9 in]
        n700 = call <vilib>:"Add State(s) to Queue__JKI_lib_State_Machine.vi"("State(s) in Front (\"\")"="MoveGuides" ("State(s) in Front (\"\")"), "State(s) in (\"\")"=w2902) -> ("States Out"=w2903:string)  [unwired: 13 in]
      }
      frame "MoveGuides" {
        n701 = Unbundle By Name(w2938) -> ("OutputCluster.SystemParameters.SoftwareFeatures.HardwareEmulated"=w2934:bool, "OutputCluster.SystemParameters.SoftwareFeatures.AutomaticGuideMovement"=w2937:bool, "OutputCluster"=w2932:T2)
        n702 = case shown="False" w2937 {
          tunnel: w2936 -> [w2947 w2978]
          tunnel: [w2946 w2972] -> w2935
          tunnel: w2934 -> [w2944 w2970]
          tunnel: [w2945 w2971] -> w2933
          tunnel: w2931 -> [w2943 w2962]
          tunnel: w2932 -> [w2942 w2969]
          tunnel: [w2941 w2963] -> w2930
          frame False {
            # "No Automatic Guide Movement"
            n703 = case shown="True" w2944 {
              tunnel: w2947 -> [w2952 w2960]
              tunnel: [w2951 w2960] -> w2946
              tunnel: w2943 -> [w2950 w2958]
              tunnel: ["Wait" ("State(s) in Front (\"\")") "SelectDone" ("State(s) in Front (\"\")")] -> w2945
              tunnel: w2942 -> [w2949 _]
              tunnel: [w2948 w2958] -> w2941
              frame False {
                # "Online Execution"
                n704 = Bundle By Name(cluster=w2949, "StateMsgToMI"="SetIndex" ("StateMessageToMI")) -> (w2953:T2)
                n705 = call "Output_SM.vi"("SM Private Data in"=w2950, "Output Cluster"=w2953, "Receiver Name"="MI", "State"="MI: StateMessage", "error in (no error)"=w2952) -> ("SM Private Data out"=w2948:refnum<class "Inspection Statemachine.lvclass">, "error out"=w2951:errorcluster)  [unwired: 9 in]
              }
              frame True {
                # "Offline Execution"
              }
            }
          }
          frame True {
            # "Automatic Guide Movement Enabled"
            n706 = Bundle By Name(cluster=w2969, "StateMsgToUI"="DisableAllButtons") -> (w2968:T2)
            n707 = call "Output_SM.vi"("SM Private Data in"=w2962, "Output Cluster"=w2968, "Receiver Name"="UI", "State"="UI: StateMessage" ("Functionality name"), "error in (no error)"=w2978) -> ("error out"=w2976:errorcluster)  [unwired: 9 in, 1 out]
            n708 = Bundle By Name(cluster=w2969, "PopupInput.Pop-up Type"=T8."Open Loading Bar" ("LoadingBarInput.Pop-up Type"), "PopupInput.Message"="Moving guides...Please wait..." ("Loading Bar Display")) -> (w2975:T2)
            n709 = call "Output_SM.vi"("SM Private Data in"=w2962, "Output Cluster"=w2975, "Receiver Name"="UI", "State"="UI: DisplayPopup", "error in (no error)"=w2976) -> ("SM Private Data out"=w2961:refnum<class "Inspection Statemachine.lvclass">, "error out"=w2973:errorcluster)  [unwired: 9 in]
            n710 = case shown="False" w2970 {
              tunnel: w2973 -> [w2984 w2992]
              tunnel: [w2983 w2992] -> w2972
              tunnel: w2961 -> [w2981 w2990]
              tunnel: ["Wait" ("State(s) in Front (\"\")") "SelectDone" ("State(s) in Front (\"\")")] -> w2971
              tunnel: w2969 -> [w2982 _]
              tunnel: [w2980 w2990] -> w2963
              frame False {
                # "Online Execution"
                n711 = Bundle By Name(cluster=w2982, "StateMsgToMI"="StartMotorReadyToInsert" ("StateMessageToMI")) -> (w2985:T2)
                n712 = call "Output_SM.vi"("SM Private Data in"=w2981, "Output Cluster"=w2985, "Receiver Name"="MI", "State"="MI: StateMessage", "error in (no error)"=w2984) -> ("SM Private Data out"=w2980:refnum<class "Inspection Statemachine.lvclass">, "error out"=w2983:errorcluster)  [unwired: 9 in]
              }
              frame True {
                # "Offline Execution"
              }
            }
          }
        }
        n713 = call <vilib>:"Add State(s) to Queue__JKI_lib_State_Machine.vi"("State(s) in Front (\"\")"=w2933, "State(s) in (\"\")"=w2939) -> ("States Out"=w2940:string)  [unwired: 13 in]
      }
      frame "ReadyToInsert" {
        # "Wait for SelectDone"
        n714 = Unbundle By Name(w2999) -> ("OutputCluster.SystemParameters.SoftwareFeatures.HardwareEmulated"=w2996:bool, "OutputCluster"=w2995:T2)
        n715 = case shown="True" w2996 {
          tunnel: w2997 -> [w3005 w3013]
          tunnel: [w3004 w3013] -> w2998
          tunnel: w2994 -> [w3007 w3012]
          tunnel: w2995 -> [w3006 _]
          tunnel: [w3003 w3012] -> w2993
          frame False {
            # "Online Execution"
            n716 = Bundle By Name(cluster=w3006, "StateMsgToMI"="SetIndex" ("StateMessageToMI")) -> (w3008:T2)
            n717 = call "Output_SM.vi"("SM Private Data in"=w3007, "Output Cluster"=w3008, "Receiver Name"="MI", "State"="MI: StateMessage", "error in (no error)"=w3005) -> ("SM Private Data out"=w3003:refnum<class "Inspection Statemachine.lvclass">, "error out"=w3004:errorcluster)  [unwired: 9 in]
          }
          frame True {
            # "Offline Execution"
          }
        }
        n718 = call <vilib>:"Add State(s) to Queue__JKI_lib_State_Machine.vi"("State(s) in Front (\"\")"="Wait" ("State(s) in Front (\"\")"), "State(s) in (\"\")"=w3000) -> ("States Out"=w3002:string)  [unwired: 13 in]
      }
      frame "SelectDone" {
        n719 = Unbundle By Name(w3018) -> ("OutputCluster"=w3017:T2)
        n720 = in-place {
          in-place-border: [w3033] -> w3025
          in-place-border: [w3031] -> w3021
          n721 = in-place-cluster #11(w3018) -> ("SelComplete"=w3031:bool)
          n722 = Select(t=w3031, s=w3031, f=TRUE ("SelComplete")) -> (s? t:f=w3032:bool)
          n723 = Select(t="SendPartDetails" ("State(s) in Front (\"\")"), s=w3031, f="Wait" ("State(s) in Front (\"\")")) -> (s? t:f=w3033:string)
          n724 = in-place-cluster #11("SelComplete"=w3032) -> (w3019:T1)
        }
        n725 = Bundle By Name(cluster=w3017, "PopupInput.Pop-up Type"=T8."Close Loading Bar" ("LoadingBarInput.Pop-up Type")) -> (w3027:T2)
        n726 = call "Output_SM.vi"("SM Private Data in"=w3015, "Output Cluster"=w3027, "Receiver Name"="UI", "State"="UI: DisplayPopup", "error in (no error)"=w3026) -> ("SM Private Data out"=w3014:refnum<class "Inspection Statemachine.lvclass">, "error out"=w3023:errorcluster)  [unwired: 9 in]
        n727 = case shown="False" w3021 {
          tunnel: w3023 -> [w3043 w3048]
          tunnel: [w3042 w3048] -> w3022
          tunnel: w3017 -> [w3041 _]
          tunnel: w3014 -> [w3040 w3047]
          tunnel: [w3037 w3047] -> w3016
          frame False {
            # "Selection completed"
            n728 = Bundle By Name(cluster=w3041, "PopupInput.Pop-up Type"=T8."Open Loading Bar" ("LoadingBarInput.Pop-up Type"), "PopupInput.Message"="Loading Part Details..." ("LoadingBarInput.LoadingString")) -> (w3045:T2)
            n729 = call "Output_SM.vi"("SM Private Data in"=w3040, "Output Cluster"=w3045, "Receiver Name"="UI", "State"="UI: DisplayPopup", "error in (no error)"=w3043) -> ("SM Private Data out"=w3037:refnum<class "Inspection Statemachine.lvclass">, "error out"=w3042:errorcluster)  [unwired: 9 in]
          }
          frame True {
            # "Selection not completed"
          }
        }
        n730 = call <vilib>:"Add State(s) to Queue__JKI_lib_State_Machine.vi"("State(s) in Front (\"\")"=w3025, "State(s) in (\"\")"=w3029) -> ("States Out"=w3030:string)  [unwired: 13 in]
      }
      frame "SendPartDetails" {
        n731 = Unbundle By Name(w3050) -> ("UpdateInPause"=w3057:bool, "OutputCluster.SystemParameters.SoftwareFeatures.HardwareEmulated"=w3053:bool, "OutputCluster"=w3061:T2, "CurrentState"=w3056:string, "OutputCluster.SystemParameters.SoftwareFeatures.AnalyticsEnable"=w3055:bool, "OutputCluster.SystemParameters.SoftwareFeatures.DataLoggingEnable"=w3054:bool)
        n732 = call "Output_SM.vi"("SM Private Data in"=w3058, "Output Cluster"=w3061, "Receiver Name"="UI", "State"="UI: PartInfo", "error in (no error)"=w3059) -> ("SM Private Data out"=w3060:refnum<class "Inspection Statemachine.lvclass">, "error out"=w3063:errorcluster)  [unwired: 9 in]
        n733 = case shown="Default" w3056 {
          tunnel: w3063 -> [w3092 w3132]
          tunnel: w3061 -> [w3077 w3119]
          tunnel: w3060 -> [w3091 w3127]
          tunnel: [w3100 w3121] -> w3051
          tunnel: [w3099 w3122] -> w3052
          tunnel: w3057 -> [_ w3126]
          tunnel: w3055 -> [_ w3125]
          tunnel: w3054 -> [_ w3124]
          tunnel: w3053 -> [w3070 w3118]
          tunnel: w3050 -> [w3069 w3117]
          tunnel: [w3067 w3117] -> w3049
          frame "MasterSampleDiagnostics", "MasterSamplePOST" {
            # "Disable hardware buttons during master sample validation"
            n734 = Bundle By Name(cluster=w3077, "PopupInput.Pop-up Type"=T8."Close Loading Bar" ("LoadingBarInput.Pop-up Type")) -> (w3094:T2)
            n735 = Bundle By Name(cluster=w3077, "StateMsgToUI"="ReadyToInsert") -> (w3106:T2)
            n736 = call "Output_SM.vi"("SM Private Data in"=w3091, "Output Cluster"=w3094, "Receiver Name"="UI", "State"="UI: DisplayPopup", "error in (no error)"=w3092) -> ("SM Private Data out"=w3090:refnum<class "Inspection Statemachine.lvclass">, "error out"=w3089:errorcluster)  [unwired: 9 in]
            n737 = call "Output_SM.vi"("SM Private Data in"=w3090, "Output Cluster"=w3106, "Receiver Name"="UI", "State"="UI: StateMessage", "error in (no error)"=w3089) -> ("SM Private Data out"=w3083:refnum<class "Inspection Statemachine.lvclass">, "error out"=w3084:errorcluster)  [unwired: 9 in]
            n738 = Bundle By Name(cluster=w3077, "StateMsgToUI"="ReadyToRun" ("StateMsgToRC")) -> (w3085:T2)
            n739 = call "Output_SM.vi"("SM Private Data in"=w3083, "Output Cluster"=w3085, "Receiver Name"="UI", "State"="UI: StateMessage", "error in (no error)"=w3084) -> ("SM Private Data out"=w3079:refnum<class "Inspection Statemachine.lvclass">, "error out"=w3078:errorcluster)  [unwired: 9 in]
            n740 = Bundle By Name(cluster=w3077, "StateMsgToMI"="SelectionComplete\nHardwareReset", "StateMsgToUI"="MoveToNextSample") -> (w3071:T2)
            n741 = call "Output_SM.vi"("SM Private Data in"=w3079, "Output Cluster"=w3071, "Receiver Name"="UI", "State"="UI: StateMessage", "error in (no error)"=w3078) -> ("SM Private Data out"=w3072:refnum<class "Inspection Statemachine.lvclass">, "error out"=w3075:errorcluster)  [unwired: 9 in]
            n742 = case shown="False" w3070 {
              tunnel: [w3110 w3116] -> w3074
              tunnel: w3075 -> [w3112 w3116]
              tunnel: w3072 -> [w3111 w3115]
              tunnel: w3071 -> [w3108 _]
              tunnel: [w3109 w3115] -> w3073
              frame False {
                # "Online Execution"
                n743 = call "Output_SM.vi"("SM Private Data in"=w3111, "Output Cluster"=w3108, "Receiver Name"="MI", "State"="MI: StateMessage", "error in (no error)"=w3112) -> ("SM Private Data out"=w3109:refnum<class "Inspection Statemachine.lvclass">, "error out"=w3110:errorcluster)  [unwired: 9 in]
              }
              frame True {
                # "Offline Execution"
              }
            }
            n744 = Bundle By Name(cluster=w3077, "MasterSampleMessages.MasterSampleMessage"="Please place the OK sample and press NEXT button for validation" ("StateMsgToUI"), "MasterSampleMessages.PartMessage"="OK\nSAMPLE\nVALIDATION") -> (w3101:T2)
            n745 = call "Output_SM.vi"("SM Private Data in"=w3073, "Output Cluster"=w3101, "Receiver Name"="UI", "State"="UI: MasterSampleMessages", "error in (no error)"=w3074) -> ("SM Private Data out"=w3100:refnum<class "Inspection Statemachine.lvclass">, "error out"=w3099:errorcluster)  [unwired: 9 in]
            n746 = Bundle By Name(cluster=w3069, "OutputCluster.MasterSamplePartName"="MasterSample: Ok Sample") -> (w3067:T1)
          }
          frame Default {
            n747 = case shown="True" w3125 {
              tunnel: w3132 -> [w3153 w3160]
              tunnel: [w3153 w3159] -> w3131
              tunnel: w3119 -> [_ w3157]
              tunnel: [w3154 w3156] -> w3128
              tunnel: w3127 -> [w3154 w3155]
              frame False {
              }
              frame True {
                n748 = call "Output_SM.vi"("SM Private Data in"=w3155, "Output Cluster"=w3157, "Receiver Name"="AN", "State"="AN: PartInfo", "error in (no error)"=w3160) -> ("SM Private Data out"=w3156:refnum<class "Inspection Statemachine.lvclass">, "error out"=w3159:errorcluster)  [unwired: 9 in]
              }
            }
            n749 = case shown="True" w3124 {
              tunnel: w3131 -> [w3145 w3151]
              tunnel: [w3145 w3150] -> w3130
              tunnel: w3119 -> [_ w3148]
              tunnel: [w3144 w3147] -> w3129
              tunnel: w3128 -> [w3144 w3146]
              frame False {
                # "DL Disable"
              }
              frame True {
                # "DL Enable"
                n750 = call "Output_SM.vi"("SM Private Data in"=w3146, "Output Cluster"=w3148, "Receiver Name"="DL", "State"="DL: PartInfo", "error in (no error)"=w3151) -> ("SM Private Data out"=w3147:refnum<class "Inspection Statemachine.lvclass">, "error out"=w3150:errorcluster)  [unwired: 9 in]
              }
            }
            n751 = case shown="False" w3126 {
              tunnel: w3130 -> [w3162 w3165]
              tunnel: [w3162 w3175] -> w3123
              tunnel: w3119 -> [_ w3166]
              tunnel: [w3163 w3177] -> w3120
              tunnel: w3129 -> [w3163 w3167]
              tunnel: w3124 -> [_ w3164]
              frame True {
              }
              frame False {
                n752 = Bundle By Name(cluster=w3166, "PopupInput.Pop-up Type"=T8."Close Loading Bar" ("LoadingBarInput.Pop-up Type")) -> (w3171:T2)
                n753 = call "Output_SM.vi"("SM Private Data in"=w3167, "Output Cluster"=w3171, "Receiver Name"="UI", "State"="UI: DisplayPopup", "error in (no error)"=w3165) -> ("SM Private Data out"=w3168:refnum<class "Inspection Statemachine.lvclass">, "error out"=w3169:errorcluster)  [unwired: 9 in]
                n754 = case shown="True" w3164 {
                  tunnel: [w3183 w3188] -> w3176
                  tunnel: [w3182 w3187] -> w3174
                  tunnel: w3169 -> [w3182 w3186]
                  tunnel: w3168 -> [w3183 w3185]
                  tunnel: w3166 -> [_ w3184]
                  frame False {
                    # "DL Disable"
                  }
                  frame True {
                    # "DL Enable"
                    n755 = Bundle By Name(cluster=w3184, "EventData.EventName"="Select" ("DataLogger.EventDetails.EventName"), "EventData.EventReason"="Part Select" ("DataLogger.EventDetails.EventReason")) -> (w3191:T2)
                    n756 = call "Output_SM.vi"("SM Private Data in"=w3185, "Output Cluster"=w3191, "Receiver Name"="DL", "State"="DL: EventDetails", "error in (no error)"=w3186) -> ("SM Private Data out"=w3188:refnum<class "Inspection Statemachine.lvclass">, "error out"=w3187:errorcluster)  [unwired: 9 in]
                  }
                }
                n757 = Bundle By Name(cluster=w3166, "StateMsgToUI"="ReadyToInsert") -> (w3180:T2)
                n758 = call "Output_SM.vi"("SM Private Data in"=w3176, "Output Cluster"=w3180, "Receiver Name"="UI", "State"="UI: StateMessage", "error in (no error)"=w3174) -> ("SM Private Data out"=w3177:refnum<class "Inspection Statemachine.lvclass">, "error out"=w3175:errorcluster)  [unwired: 9 in]
              }
            }
            n759 = case shown="False" w3118 {
              tunnel: [w3134 w3143] -> w3122
              tunnel: w3123 -> [w3137 w3143]
              tunnel: w3120 -> [w3135 w3142]
              tunnel: w3119 -> [w3136 _]
              tunnel: [w3133 w3142] -> w3121
              frame False {
                # "Online Execution"
                n760 = Bundle By Name(cluster=w3136, "StateMsgToMI"="SelectionComplete" ("StateMessageToMI")) -> (w3138:T2)
                n761 = call "Output_SM.vi"("SM Private Data in"=w3135, "Output Cluster"=w3138, "Receiver Name"="MI", "State"="MI: StateMessage", "error in (no error)"=w3137) -> ("SM Private Data out"=w3133:refnum<class "Inspection Statemachine.lvclass">, "error out"=w3134:errorcluster)  [unwired: 9 in]
              }
              frame True {
                # "Offline Execution"
              }
            }
          }
        }
        n762 = call <vilib>:"Add State(s) to Queue__JKI_lib_State_Machine.vi"("State(s) in (\"\")"=w3065) -> ("States Out"=w3066:string)  [unwired: 14 in]
      }
      frame "---------- Run State ----------" {
        # "Do not put any code in this frame.\n(It is a separator no-op. You can make a copy of this frame to create a new UI frame)"
        n763 = call <vilib>:"Add State(s) to Queue__JKI_lib_State_Machine.vi"("State(s) in (\"\")"=w3198) -> ("States Out"=w3197:string)  [unwired: 14 in]
      }
      frame "Run" {
        n764 = in-place {
          in-place-border: [w3217] -> w3205
          in-place-border: w3200 -> [w3216]
          in-place-border: w3204 -> [w3215]
          in-place-border: [w3214] -> w3203
          in-place-border: [w3210] -> w3199
          n765 = in-place-cluster #12(w3202) -> ("CurrentState"=w3213:string, "OutputCluster"=w3208:T2)
          n766 = Unbundle By Name(w3208) -> ("SystemParameters.SoftwareFeatures.HardwareEmulated"=w3211:bool, "SystemParameters.SoftwareFeatures.AutomaticGuideMovement"=w3212:bool)
          n767 = case shown="\"HardwareButtonDiagnostics\"" w3213 {
            selector: w3213 -> [_ _ w3271]
            tunnel: w3216 -> [w3228 w3260 w3278]
            tunnel: w3215 -> [w3233 w3264 w3280]
            tunnel: [w3218 w3261 w3279] -> w3214
            tunnel: w3211 -> [w3232 w3263 _]
            tunnel: [w3230 w3262 "" ("State(s) in Front (\"\")")] -> w3217
            tunnel: w3212 -> [w3231 _ _]
            tunnel: w3208 -> [w3229 w3259 w3275]
            tunnel: [w3220 w3258 w3272] -> w3210
            tunnel: ["Run" ("Previous State") "Run" ("Previous State") w3271] -> w3209
            tunnel: w3208 -> [w3222 _ _]
            frame "Select", Default {
              n768 = case shown="False" w3232 {
                tunnel: w3233 -> [w3240 w3256]
                tunnel: [w3239 w3256] -> w3219
                tunnel: w3231 -> [w3238 _]
                tunnel: [w3237 "RunPositionReached" ("State(s) in Front (\"\")")] -> w3230
                tunnel: w3228 -> [w3236 w3254]
                tunnel: w3229 -> [w3235 _]
                tunnel: [w3234 w3254] -> w3221
                frame False {
                  # "Online execution"
                  n769 = case shown="True" w3238 {
                    tunnel: w3240 -> [w3243 w3249]
                    tunnel: [w3243 w3244] -> w3239
                    tunnel: ["RunPositionReached" ("State(s) in Front (\"\")") "" ("State(s) in Front (\"\")")] -> w3237
                    tunnel: w3236 -> [w3241 w3247]
                    tunnel: w3235 -> [_ w3248]
                    tunnel: [w3241 w3245] -> w3234
                    frame False {
                      # "Automatic Guide Movement disabled"
                    }
                    frame True {
                      # "Automatic Guide Movement Enabled"
                      n770 = Bundle By Name(cluster=w3248, "StateMsgToMI"="StartMotorReadyToRun" ("StateMessageToMI")) -> (w3246:T2)
                      n771 = call "Output_SM.vi"("SM Private Data in"=w3247, "Output Cluster"=w3246, "Receiver Name"="MI", "State"="MI: StateMessage", "error in (no error)"=w3249) -> ("SM Private Data out"=w3245:refnum<class "Inspection Statemachine.lvclass">, "error out"=w3244:errorcluster)  [unwired: 9 in]
                    }
                  }
                }
                frame True {
                }
              }
              n772 = Bundle By Name(cluster=w3222, "StateMsgToUI"="DisplayInspectionPage>>Images" ("StateMsgToRC")) -> (w3223:T2)
              n773 = call "Output_SM.vi"("SM Private Data in"=w3221, "Output Cluster"=w3223, "Receiver Name"="UI", "State"="UI: StateMessage", "error in (no error)"=w3219) -> ("SM Private Data out"=w3220:refnum<class "Inspection Statemachine.lvclass">, "error out"=w3218:errorcluster)  [unwired: 9 in]
            }
            frame "Pause", "PauseOnFail", "PauseOnReelFinish", "Run" {
              n774 = case shown="False" w3263 {
                tunnel: w3264 -> [w3266 w3270]
                tunnel: [w3266 w3270] -> w3261
                tunnel: ["RunPositionReached" ("State(s) in Front (\"\")") "ReadyToRun" ("State(s) in Front (\"\")")] -> w3262
                tunnel: w3260 -> [w3265 w3268]
                tunnel: w3259 -> [_ _]
                tunnel: [w3265 w3268] -> w3258
                frame False {
                  # "Online Execution"
                }
                frame True {
                  # "Offline Execution"
                }
              }
            }
            frame "HardwareButtonDiagnostics" {
              n775 = Bundle By Name(cluster=w3275, "StateMsgToUI"="Run") -> (w3274:T2)
              n776 = call "Output_SM.vi"("SM Private Data in"=w3278, "Output Cluster"=w3274, "Receiver Name"="UI", "State"="UI: StateMessage", "error in (no error)"=w3280) -> ("SM Private Data out"=w3272:refnum<class "Inspection Statemachine.lvclass">, "error out"=w3279:errorcluster)  [unwired: 9 in]
            }
          }
          n777 = in-place-cluster #12("CurrentState"=w3209, "OutputCluster"=w3208) -> (w3201:T1)
        }
        n778 = call <vilib>:"Add State(s) to Queue__JKI_lib_State_Machine.vi"("State(s) in Front (\"\")"=w3205, "State(s) in (\"\")"=w3206) -> ("States Out"=w3207:string)  [unwired: 13 in]
      }
      frame "EnableSensors" {
        n779 = Unbundle By Name(w3284) -> ("OutputCluster.SystemParameters.SoftwareFeatures.HardwareEmulated"=w3288:bool, "OutputCluster"=w3285:T2)
        n780 = case shown="False" w3288 {
          tunnel: w3289 -> [w3296 w3304]
          tunnel: [w3295 w3304] -> w3286
          tunnel: ["" ("State(s) in Front (\"\")") "ReadyToRun" ("State(s) in Front (\"\")")] -> w3287
          tunnel: w3283 -> [w3294 w3302]
          tunnel: w3285 -> [w3293 _]
          tunnel: [w3292 w3302] -> w3282
          frame False {
            # "Online Execution"
            n781 = Bundle By Name(cluster=w3293, "StateMsgToMI"="EnableSensor" ("StateMessageToMI")) -> (w3297:T2)
            n782 = call "Output_SM.vi"("SM Private Data in"=w3294, "Output Cluster"=w3297, "Receiver Name"="MI", "State"="MI: StateMessage", "error in (no error)"=w3296) -> ("SM Private Data out"=w3292:refnum<class "Inspection Statemachine.lvclass">, "error out"=w3295:errorcluster)  [unwired: 9 in]
          }
          frame True {
            # "Offline Execution"
          }
        }
        n783 = call <vilib>:"Add State(s) to Queue__JKI_lib_State_Machine.vi"("State(s) in Front (\"\")"=w3287, "State(s) in (\"\")"=w3290) -> ("States Out"=w3291:string)  [unwired: 13 in]
      }
      frame "RunPositionReached" {
        # "DisableDoorLimitSwitch"
        n784 = Unbundle By Name(w3310) -> ("OutputCluster.SystemParameters.SoftwareFeatures.HardwareEmulated"=w3309:bool, "OutputCluster.SystemParameters.SoftwareFeatures.DoorPokayokeEnable"=w3307:bool, "OutputCluster"=w3308:T2)
        n785 = case shown="False" w3309 {
          tunnel: w3313 -> [w3322 w3344]
          tunnel: [w3321 "ReadyToRun" ("State(s) in Front (\"\")")] -> w3312
          tunnel: [w3320 w3344] -> w3311
          tunnel: w3306 -> [w3319 w3343]
          tunnel: w3308 -> [w3318 _]
          tunnel: w3307 -> [w3317 _]
          tunnel: [w3316 w3343] -> w3305
          frame False {
            # "Online execution"
            n786 = case shown="True" w3317 {
              tunnel: w3322 -> [w3327 w3338]
              tunnel: [w3326 w3337] -> w3320
              tunnel: ["Wait" ("State(s) in Front (\"\")") "EnableSensors" ("State(s) in Front (\"\")")] -> w3321
              tunnel: w3319 -> [w3325 w3336]
              tunnel: w3318 -> [w3324 w3335]
              tunnel: [w3323 w3334] -> w3316
              frame True {
                # "Door Pokayoke enabled"
                n787 = Bundle By Name(cluster=w3324, "StateMsgToMI"="PreRun\nHardwareReset\nDisableDoorLimitSwitch\nEnableDoorLimitSwitch\nDoorLockStatusCheck" ("StateMessageToMI")) -> (w3328:T2)
                n788 = call "Output_SM.vi"("SM Private Data in"=w3325, "Output Cluster"=w3328, "Receiver Name"="MI", "State"="MI: StateMessage", "error in (no error)"=w3327) -> ("SM Private Data out"=w3323:refnum<class "Inspection Statemachine.lvclass">, "error out"=w3326:errorcluster)  [unwired: 9 in]
              }
              frame False {
                # "Door Pokayoke disabled"
                n789 = Bundle By Name(cluster=w3335, "StateMsgToMI"="DisableDoorLimitSwitch" ("StateMessageToMI")) -> (w3339:T2)
                n790 = call "Output_SM.vi"("SM Private Data in"=w3336, "Output Cluster"=w3339, "Receiver Name"="MI", "State"="MI: StateMessage", "error in (no error)"=w3338) -> ("SM Private Data out"=w3334:refnum<class "Inspection Statemachine.lvclass">, "error out"=w3337:errorcluster)  [unwired: 9 in]
              }
            }
          }
          frame True {
            # "Offline execution"
          }
        }
        n791 = call <vilib>:"Add State(s) to Queue__JKI_lib_State_Machine.vi"("State(s) in Front (\"\")"=w3312, "State(s) in (\"\")"=w3314) -> ("States Out"=w3315:string)  [unwired: 13 in]
      }
      frame "ReadyToRun" {
        n792 = in-place {
          in-place-border: w3351 -> [w3363]
          in-place-border: [w3354] -> w3350
          in-place-border: w3347 -> [w3361]
          in-place-border: [w3355] -> w3346
          n793 = in-place-cluster #13(w3349) -> ("EventReason"=w3360:string, "CurrentState"=w3359:string, "BatchStart"=w3362:bool, "OutputCluster"=w3357:T2)
          n794 = Unbundle By Name(w3357) -> ("SystemParameters.SoftwareFeatures.DataLoggingEnable"=w3358:bool)
          n795 = case shown="Default" w3359 {
            tunnel: w3363 -> [w3365 w3383]
            tunnel: [w3365 w3370] -> w3354
            tunnel: w3362 -> [w3364 w3387]
            tunnel: [w3366 w3371] -> w3355
            tunnel: w3361 -> [w3366 w3384]
            tunnel: w3357 -> [_ w3368]
            tunnel: w3360 -> [_ w3386]
            tunnel: w3358 -> [_ w3385]
            tunnel: [w3364 FALSE ("ReelInfo.BatchStartOrNot")] -> w3356
            frame "MS:NotOkValidated", "MS:NotOkValidation", "MS:OkValidated", "MS:OkValidation" {
            }
            frame Default {
              n796 = case shown="True" w3385 {
                tunnel: [w3389 w3405] -> w3372
                tunnel: w3387 -> [_ w3401]
                tunnel: [w3388 w3399] -> w3367
                tunnel: w3386 -> [_ w3398]
                tunnel: w3383 -> [w3389 _]
                tunnel: w3384 -> [w3388 w3391]
                tunnel: w3368 -> [_ w3390]
                frame False {
                  # "DL Disable"
                }
                frame True {
                  # "DL Enable"
                  n797 = Bundle By Name(cluster=w3390, "MachineStatusToDL"="Inspection" ("StateMsgToDL")) -> (w3394:T2)
                  n798 = call "Output_SM.vi"("SM Private Data in"=w3391, "Output Cluster"=w3394, "Receiver Name"="DL", "State"="DL: MachineStatus") -> ("SM Private Data out"=w3392:refnum<class "Inspection Statemachine.lvclass">, "error out"=w3393:errorcluster)  [unwired: 10 in]
                  n799 = Bundle By Name(cluster=w3390, "StateMsgToDL"="StopPost") -> (w3403:T2)
                  n800 = call "Output_SM.vi"("SM Private Data in"=w3392, "Output Cluster"=w3403, "Receiver Name"="DL", "State"="DL: StateMessage", "error in (no error)"=w3393) -> ("SM Private Data out"=w3400:refnum<class "Inspection Statemachine.lvclass">, "error out"=w3406:errorcluster)  [unwired: 9 in]
                  n801 = case shown="False" w3401 {
                    tunnel: w3400 -> [w3417 w3419]
                    tunnel: w3406 -> [w3415 w3431]
                    tunnel: w3390 -> [w3416 w3422]
                    tunnel: [w3414 w3424] -> w3405
                    tunnel: [w3413 w3420] -> w3399
                    tunnel: w3398 -> [w3412 _]
                    frame False {
                      # "Not Batch start"
                      n802 = Bundle By Name(cluster=w3416, "EventData.EventName"="Run" ("DataLogger.EventDetails.EventName"), "EventData.EventReason"=w3412) -> (w3409:T2)
                      n803 = call "Output_SM.vi"("SM Private Data in"=w3417, "Output Cluster"=w3409, "Receiver Name"="DL", "State"="DL: EventDetails", "error in (no error)"=w3415) -> ("SM Private Data out"=w3413:refnum<class "Inspection Statemachine.lvclass">, "error out"=w3414:errorcluster)  [unwired: 9 in]
                    }
                    frame True {
                      # "Batch Start"
                      n804 = call "Output_SM.vi"("SM Private Data in"=w3419, "Output Cluster"=w3422, "Receiver Name"="DL", "State"="DL: ReelInfo", "error in (no error)"=w3431) -> ("SM Private Data out"=w3418:refnum<class "Inspection Statemachine.lvclass">, "error out"=w3430:errorcluster)  [unwired: 9 in]
                      n805 = Bundle By Name(cluster=w3422, "EventData.EventName"="BatchStart" ("DataLogger.EventDetails.EventName"), "EventData.EventReason"="Batch Start" ("DataLogger.EventDetails.EventReason")) -> (w3425:T2)
                      n806 = call "Output_SM.vi"("SM Private Data in"=w3418, "Output Cluster"=w3425, "Receiver Name"="DL", "State"="DL: EventDetails", "error in (no error)"=w3430) -> ("SM Private Data out"=w3420:refnum<class "Inspection Statemachine.lvclass">, "error out"=w3424:errorcluster)  [unwired: 9 in]
                    }
                  }
                }
              }
              n807 = Bundle By Name(cluster=w3368, "StateMsgToRC"="Run") -> (w3375:T2)
              n808 = call "Output_SM.vi"("SM Private Data in"=w3367, "Output Cluster"=w3375, "Receiver Name"="RC", "State"="RC: StateMessage", "error in (no error)"=w3372) -> ("SM Private Data out"=w3381:refnum<class "Inspection Statemachine.lvclass">, "error out"=w3369:errorcluster)  [unwired: 9 in]
              n809 = Bundle By Name(cluster=w3368, "StateMsgToUI"="ReadyToRun" ("StateMsgToRC")) -> (w3380:T2)
              n810 = call "Output_SM.vi"("SM Private Data in"=w3381, "Output Cluster"=w3380, "Receiver Name"="UI", "State"="UI: StateMessage", "error in (no error)"=w3369) -> ("SM Private Data out"=w3371:refnum<class "Inspection Statemachine.lvclass">, "error out"=w3370:errorcluster)  [unwired: 9 in]
            }
          }
          n811 = in-place-cluster #13("EventReason"=w3360, "CurrentState"=w3359, "BatchStart"=w3356, "OutputCluster"=w3357) -> (w3348:T1)
        }
        n812 = call <vilib>:"Add State(s) to Queue__JKI_lib_State_Machine.vi"("State(s) in (\"\")"=w3352) -> ("States Out"=w3353:string)  [unwired: 14 in]
      }
      frame "Pass" {
        n813 = Unbundle By Name(w3445) -> ("OutputCluster.SystemParameters.SoftwareFeatures.AnalyticsEnable"=w3432:bool, "CurrentState"=w3433:string, "OutputCluster.SystemParameters.SoftwareFeatures.HardwareEmulated"=w3448:bool, "ResultToMI"=w3446:bool, "OutputCluster"=w3440:T2)
        n814 = case shown="False" w3448 {
          tunnel: w3449 -> [w3465 w3485]
          tunnel: [w3466 w3485] -> w3442
          tunnel: w3446 -> [w3467 _]
          tunnel: w3445 -> [w3464 w3484]
          tunnel: [w3463 w3484] -> w3434
          tunnel: w3436 -> [w3462 w3483]
          tunnel: w3440 -> [w3461 _]
          tunnel: [w3460 w3483] -> w3437
          tunnel: w3433 -> [_ _]
          frame False {
            # "Online Execution"
            n815 = case shown="False" w3467 {
              tunnel: [w3470 w3471] -> w3466
              tunnel: w3465 -> [w3470 w3481]
              tunnel: w3464 -> [w3469 w3480]
              tunnel: [w3469 w3478] -> w3463
              tunnel: w3462 -> [w3468 w3477]
              tunnel: w3461 -> [_ w3475]
              tunnel: [w3468 w3472] -> w3460
              frame True {
                # "Result status is already sent to MI"
              }
              frame False {
                # "Result status sent to MI"
                n816 = Bundle By Name(cluster=w3475, "InspectionStatusToMI"="Pass") -> (w3473:T2)
                n817 = Bundle By Name(cluster=w3480, "ResultToMI"=TRUE ("PrevResultStatus")) -> (w3478:T1)
                n818 = call "Output_SM.vi"("SM Private Data in"=w3477, "Output Cluster"=w3473, "Receiver Name"="MI", "State"="MI: InspectionStatus", "error in (no error)"=w3481) -> ("SM Private Data out"=w3472:refnum<class "Inspection Statemachine.lvclass">, "error out"=w3471:errorcluster)  [unwired: 9 in]
              }
            }
          }
          frame True {
            # "Offline Execution"
          }
        }
        n819 = call "Output_SM.vi"("SM Private Data in"=w3437, "Output Cluster"=w3440, "Receiver Name"="UI", "State"="UI: ResultData", "error in (no error)"=w3442) -> ("SM Private Data out"=w3438:refnum<class "Inspection Statemachine.lvclass">, "error out"=w3443:errorcluster)  [unwired: 9 in]
        n820 = case shown="True" w3432 {
          tunnel: w3443 -> [w3451 w3459]
          tunnel: [w3451 w3458] -> w3441
          tunnel: w3440 -> [_ w3457]
          tunnel: w3438 -> [w3452 w3456]
          tunnel: [w3452 w3455] -> w3435
          frame False {
          }
          frame True {
            n821 = call "Output_SM.vi"("SM Private Data in"=w3456, "Output Cluster"=w3457, "Receiver Name"="AN", "State"="AN: ResultData", "error in (no error)"=w3459) -> ("SM Private Data out"=w3455:refnum<class "Inspection Statemachine.lvclass">, "error out"=w3458:errorcluster)  [unwired: 9 in]
          }
        }
        n822 = call <vilib>:"Add State(s) to Queue__JKI_lib_State_Machine.vi"("State(s) in (\"\")"=w3447) -> ("States Out"=w3450:string)  [unwired: 14 in]
      }
      frame "----------MasterSampleValidation----------" {
        n823 = call <vilib>:"Add State(s) to Queue__JKI_lib_State_Machine.vi"("State(s) in (\"\")"=w3488) -> ("States Out"=w3489:string)  [unwired: 14 in]
      }
      frame "Next" {
        n824 = Unbundle By Name(w3497) -> ("OutputCluster"=w3501:T2, "MasterSampleState"=w3502:string, "OutputCluster.SystemParameters.SoftwareFeatures.HardwareEmulated"=w3493:bool, "CurrentState"=w3492:string, "OutputCluster.SystemParameters.SoftwareFeatures.AutomaticGuideMovement"=w3491:bool)
        n825 = case shown="\"MS:NotOkValidated\"" w3502 {
          tunnel: w3501 -> [w3516 w3550 w3579 _]
          tunnel: w3500 -> [w3523 w3554 w3581 w3600]
          tunnel: [w3511 w3553 w3588 w3600] -> w3499
          tunnel: ["" "Wait" "Wait" ""] -> w3498
          tunnel: w3497 -> [w3506 w3556 w3596 w3598]
          tunnel: [w3505 w3556 w3594 w3598] -> w3496
          tunnel: [w3512 w3552 w3587 w3599] -> w3495
          tunnel: w3494 -> [w3522 w3551 w3580 w3599]
          tunnel: w3493 -> [_ w3549 _ _]
          tunnel: w3492 -> [_ _ _ _]
          tunnel: w3491 -> [w3521 _ _ _]
          frame "MS:NotOkValidated" {
            n826 = case shown="False" w3521 {
              tunnel: [w3532 w3545] -> w3518
              tunnel: w3523 -> [w3533 w3543]
              tunnel: w3522 -> [w3534 w3544]
              tunnel: w3516 -> [w3529 w3541]
              tunnel: [w3525 w3537] -> w3517
              frame True {
                # "Automatic Guide Movement Enabled"
                n827 = Bundle By Name(cluster=w3529, "PopupInput.Title"="MESSAGE" ("Dialog Box Input"), "PopupInput.Message"="Please remove the Master Sample before the guides are opened" ("Message Input"), "PopupInput.Button 1 Text"="Continue" ("Boolean Text.Text"), "PopupInput.Pop-up Type"=T8."One button dialog box") -> (w3531:T2)
                n828 = call "Output_SM.vi"("SM Private Data in"=w3534, "Output Cluster"=w3531, "Receiver Name"="UI", "State"="UI: DisplayPopup", "error in (no error)"=w3533) -> ("SM Private Data out"=w3525:refnum<class "Inspection Statemachine.lvclass">, "error out"=w3532:errorcluster)  [unwired: 9 in]
              }
              frame False {
                # "Automatic Guide Movement disabled"
                n829 = Bundle By Name(cluster=w3541, "PopupInput.Title"="MESSAGE" ("Dialog Box Input"), "PopupInput.Message"="Please remove the Master Sample" ("Message Input"), "PopupInput.Button 1 Text"="Continue" ("Boolean Text.Text"), "PopupInput.Pop-up Type"=T8."One button dialog box") -> (w3547:T2)
                n830 = call "Output_SM.vi"("SM Private Data in"=w3544, "Output Cluster"=w3547, "Receiver Name"="UI", "State"="UI: DisplayPopup", "error in (no error)"=w3543) -> ("SM Private Data out"=w3537:refnum<class "Inspection Statemachine.lvclass">, "error out"=w3545:errorcluster)  [unwired: 9 in]
              }
            }
            n831 = Bundle By Name(cluster=w3516, "StateMsgToUI"="Initialize images", "StateMsgToRC"="Stop") -> (w3508:T2)
            n832 = call "Output_SM.vi"("SM Private Data in"=w3517, "Output Cluster"=w3508, "Receiver Name"="RC", "State"="RC: StateMessage", "error in (no error)"=w3518) -> ("SM Private Data out"=w3510:refnum<class "Inspection Statemachine.lvclass">, "error out"=w3509:errorcluster)  [unwired: 9 in]
            n833 = Bundle By Name(cluster=w3506, "SelComplete"=FALSE) -> (w3505:T1)
            n834 = call "Output_SM.vi"("SM Private Data in"=w3510, "Output Cluster"=w3508, "Receiver Name"="UI", "State"="UI: StateMessage", "error in (no error)"=w3509) -> ("SM Private Data out"=w3512:refnum<class "Inspection Statemachine.lvclass">, "error out"=w3511:errorcluster)  [unwired: 9 in]
          }
          frame "MS:NotOkValidation", "MS:OkValidation" {
            n835 = case shown="False" w3549 {
              tunnel: w3554 -> [w3557 w3574]
              tunnel: [w3562 w3574] -> w3553
              tunnel: [w3563 w3575] -> w3552
              tunnel: w3551 -> [w3558 w3575]
              tunnel: w3550 -> [w3559 _]
              frame False {
                # "Online execution"
                n836 = Bundle By Name(cluster=w3559, "Trigger Light Camera Sequence.Light Sequence Trigger"="AllLightCameraSequence" ("Light Camera Info.Light Camera Name"), "Trigger Light Camera Sequence.Status"="On" ("Light Camera Info.State"), "Trigger Light Camera Sequence.Mode"="OneShot") -> (w3571:T2)
                n837 = call "Output_SM.vi"("SM Private Data in"=w3558, "Output Cluster"=w3571, "Receiver Name"="MI", "State"="MI: CameraOpticsDiagnostics", "error in (no error)"=w3557) -> ("SM Private Data out"=w3561:refnum<class "Inspection Statemachine.lvclass">, "error out"=w3560:errorcluster)  [unwired: 9 in]
                n838 = Bundle By Name(cluster=w3559, "StateMsgToRC"="Run") -> (w3565:T2)
                n839 = call "Output_SM.vi"("SM Private Data in"=w3561, "Output Cluster"=w3565, "Receiver Name"="RC", "State"="RC: StateMessage", "error in (no error)"=w3560) -> ("SM Private Data out"=w3563:refnum<class "Inspection Statemachine.lvclass">, "error out"=w3562:errorcluster)  [unwired: 9 in]
              }
              frame True {
                # "Offline execution"
              }
            }
          }
          frame "MS:OkValidated" {
            n840 = Bundle By Name(cluster=w3579, "StateMsgToUI"="MoveToNextSample") -> (w3583:T2)
            n841 = call "Output_SM.vi"("SM Private Data in"=w3580, "Output Cluster"=w3583, "Receiver Name"="UI", "State"="UI: StateMessage", "error in (no error)"=w3581) -> ("SM Private Data out"=w3577:refnum<class "Inspection Statemachine.lvclass">, "error out"=w3578:errorcluster)  [unwired: 9 in]
            n842 = Bundle By Name(cluster=w3579, "MasterSampleMessages.MasterSampleMessage"="Please place the NOT OK sample and press NEXT button for validation" ("StateMsgToUI"), "MasterSampleMessages.PartMessage"="NOT OK\nSAMPLE\nVALIDATION") -> (w3590:T2)
            n843 = call "Output_SM.vi"("SM Private Data in"=w3577, "Output Cluster"=w3590, "Receiver Name"="UI", "State"="UI: MasterSampleMessages", "error in (no error)"=w3578) -> ("SM Private Data out"=w3587:refnum<class "Inspection Statemachine.lvclass">, "error out"=w3588:errorcluster)  [unwired: 9 in]
            n844 = Bundle By Name(cluster=w3596, "MasterSampleState"="MS:NotOkValidation" ("CurrentState"), "OutputCluster.MasterSamplePartName"="MasterSample: NotOk Sample") -> (w3594:T1)
          }
          frame Default {
          }
        }
        n845 = call <vilib>:"Add State(s) to Queue__JKI_lib_State_Machine.vi"("State(s) in (\"\")"=w3498) -> ("States Out"=w3503:string)  [unwired: 14 in]
      }
      frame "Repeat" {
        n846 = Unbundle By Name(w3607) -> ("OutputCluster"=w3604:T2, "OutputCluster.SystemParameters.SoftwareFeatures.HardwareEmulated"=w3603:bool)
        n847 = case shown="False" w3603 {
          tunnel: w3601 -> [w3627 w3628]
          tunnel: [w3614 w3628] -> w3605
          tunnel: [w3615 w3629] -> w3606
          tunnel: w3602 -> [w3626 w3629]
          tunnel: w3604 -> [w3611 _]
          frame False {
            # "Online execution"
            n848 = Bundle By Name(cluster=w3611, "Trigger Light Camera Sequence.Light Sequence Trigger"="AllLightCameraSequence" ("Light Camera Info.Light Camera Name"), "Trigger Light Camera Sequence.Status"="On" ("Light Camera Info.State"), "Trigger Light Camera Sequence.Mode"="OneShot") -> (w3623:T2)
            n849 = call "Output_SM.vi"("SM Private Data in"=w3626, "Output Cluster"=w3623, "Receiver Name"="MI", "State"="MI: CameraOpticsDiagnostics", "error in (no error)"=w3627) -> ("SM Private Data out"=w3613:refnum<class "Inspection Statemachine.lvclass">, "error out"=w3612:errorcluster)  [unwired: 9 in]
            n850 = Bundle By Name(cluster=w3611, "StateMsgToRC"="Run") -> (w3617:T2)
            n851 = call "Output_SM.vi"("SM Private Data in"=w3613, "Output Cluster"=w3617, "Receiver Name"="RC", "State"="RC: StateMessage", "error in (no error)"=w3612) -> ("SM Private Data out"=w3615:refnum<class "Inspection Statemachine.lvclass">, "error out"=w3614:errorcluster)  [unwired: 9 in]
          }
          frame True {
            # "Offline execution"
          }
        }
        n852 = call <vilib>:"Add State(s) to Queue__JKI_lib_State_Machine.vi"("State(s) in Front (\"\")"="Wait" ("State(s) in Front (\"\")"), "State(s) in (\"\")"=w3609) -> ("States Out"=w3610:string)  [unwired: 13 in]
      }
      frame "MasterSampleValidationPass" {
        n853 = Unbundle By Name(w3644) -> ("MasterSampleState"=w3631:string, "OutputCluster.SystemParameters.SoftwareFeatures.HardwareEmulated"=w3647:bool, "ResultToMI"=w3645:bool, "OutputCluster"=w3639:T2)
        n854 = case shown="False" w3647 {
          tunnel: w3648 -> [w3694 w3714]
          tunnel: [w3695 w3714] -> w3641
          tunnel: w3645 -> [w3696 _]
          tunnel: w3644 -> [w3693 w3713]
          tunnel: [w3692 w3713] -> w3633
          tunnel: w3635 -> [w3691 w3712]
          tunnel: w3639 -> [w3690 _]
          tunnel: [w3689 w3712] -> w3636
          frame False {
            # "Online Execution"
            n855 = case shown="False" w3696 {
              tunnel: [w3699 w3700] -> w3695
              tunnel: w3694 -> [w3699 w3710]
              tunnel: w3693 -> [w3698 w3709]
              tunnel: [w3698 w3707] -> w3692
              tunnel: w3691 -> [w3697 w3706]
              tunnel: w3690 -> [_ w3704]
              tunnel: [w3697 w3701] -> w3689
              frame True {
                # "Result status is already sent to MI"
              }
              frame False {
                # "Result status sent to MI"
                n856 = Bundle By Name(cluster=w3704, "InspectionStatusToMI"="Pass") -> (w3702:T2)
                n857 = Bundle By Name(cluster=w3709, "ResultToMI"=TRUE ("PrevResultStatus")) -> (w3707:T1)
                n858 = call "Output_SM.vi"("SM Private Data in"=w3706, "Output Cluster"=w3702, "Receiver Name"="MI", "State"="MI: InspectionStatus", "error in (no error)"=w3710) -> ("SM Private Data out"=w3701:refnum<class "Inspection Statemachine.lvclass">, "error out"=w3700:errorcluster)  [unwired: 9 in]
              }
            }
          }
          frame True {
            # "Offline Execution"
          }
        }
        n859 = call "Output_SM.vi"("SM Private Data in"=w3636, "Output Cluster"=w3639, "Receiver Name"="UI", "State"="UI: ResultData", "error in (no error)"=w3641) -> ("SM Private Data out"=w3637:refnum<class "Inspection Statemachine.lvclass">, "error out"=w3642:errorcluster)  [unwired: 9 in]
        n860 = case shown="\"MS:NotOkValidated\", \"MS:NotOkValidation\"" w3631 {
          tunnel: w3642 -> [w3668 w3685 w3686]
          tunnel: [w3661 w3678 w3686] -> w3640
          tunnel: w3639 -> [w3654 w3673 _]
          tunnel: w3637 -> [w3667 w3684 w3687]
          tunnel: [w3659 w3676 w3687] -> w3634
          tunnel: w3633 -> [w3658 w3675 w3688]
          tunnel: [w3657 w3675 w3688] -> w3632
          frame "MS:OkValidated", "MS:OkValidation" {
            n861 = Bundle By Name(cluster=w3654, "StateMsgToUI"="MasterSampleValidationPass" ("State")) -> (w3653:T2)
            n862 = call "Output_SM.vi"("SM Private Data in"=w3667, "Output Cluster"=w3653, "Receiver Name"="UI", "State"="UI: StateMessage", "error in (no error)"=w3668) -> ("SM Private Data out"=w3660:refnum<class "Inspection Statemachine.lvclass">, "error out"=w3662:errorcluster)  [unwired: 9 in]
            n863 = Bundle By Name(cluster=w3658, "MasterSampleState"="MS:OkValidated" ("CurrentState")) -> (w3657:T1)
            n864 = Bundle By Name(cluster=w3654, "MasterSampleMessages.MasterSampleMessage"="OK sample validation is successful.\nPress NEXT button for NOT OK sample validation or press REPEAT button to repeat OK sample validation." ("StateMsgToUI"), "MasterSampleMessages.PartMessage"="OK\nSAMPLE\nVALIDATION") -> (w3663:T2)
            n865 = call "Output_SM.vi"("SM Private Data in"=w3660, "Output Cluster"=w3663, "Receiver Name"="UI", "State"="UI: MasterSampleMessages", "error in (no error)"=w3662) -> ("SM Private Data out"=w3659:refnum<class "Inspection Statemachine.lvclass">, "error out"=w3661:errorcluster)  [unwired: 9 in]
          }
          frame "MS:NotOkValidated", "MS:NotOkValidation" {
            n866 = Bundle By Name(cluster=w3673, "StateMsgToUI"="MasterSampleValidationFail" ("State")) -> (w3672:T2)
            n867 = call "Output_SM.vi"("SM Private Data in"=w3684, "Output Cluster"=w3672, "Receiver Name"="UI", "State"="UI: StateMessage", "error in (no error)"=w3685) -> ("SM Private Data out"=w3677:refnum<class "Inspection Statemachine.lvclass">, "error out"=w3679:errorcluster)  [unwired: 9 in]
            n868 = Bundle By Name(cluster=w3673, "MasterSampleMessages.MasterSampleMessage"="NOT OK sample validation has failed.\nPress REPEAT button to repeat NOT OK sample validation or contact Zentron Labs." ("StateMsgToUI"), "MasterSampleMessages.PartMessage"="NOT OK\nSAMPLE\nVALIDATION") -> (w3680:T2)
            n869 = call "Output_SM.vi"("SM Private Data in"=w3677, "Output Cluster"=w3680, "Receiver Name"="UI", "State"="UI: MasterSampleMessages", "error in (no error)"=w3679) -> ("SM Private Data out"=w3676:refnum<class "Inspection Statemachine.lvclass">, "error out"=w3678:errorcluster)  [unwired: 9 in]
          }
          frame Default {
          }
        }
        n870 = call <vilib>:"Add State(s) to Queue__JKI_lib_State_Machine.vi"("State(s) in Front (\"\")"="Wait" ("State(s) in Front (\"\")"), "State(s) in (\"\")"=w3646) -> ("States Out"=w3649:string)  [unwired: 13 in]
      }
      frame "MasterSampleValidationFail" {
        n871 = Unbundle By Name(w3729) -> ("MasterSampleState"=w3716:string, "OutputCluster.SystemParameters.SoftwareFeatures.PopupOptions.ReasonForFail"=w3719:bool, "OutputCluster.SystemParameters.SoftwareFeatures.HardwareEmulated"=w3726:bool, "ResultToMI"=w3728:bool, "OutputCluster"=w3720:T2)
        n872 = case shown="False" w3726 {
          tunnel: w3727 -> [w3790 w3795]
          tunnel: [w3786 w3795] -> w3725
          tunnel: w3729 -> [w3782 w3794]
          tunnel: [w3781 w3794] -> w3717
          tunnel: w3728 -> [w3785 _]
          tunnel: w3722 -> [w3792 w3793]
          tunnel: w3720 -> [w3791 _]
          tunnel: [w3780 w3793] -> w3723
          tunnel: w3719 -> [_ _]
          tunnel: w3716 -> [_ _]
          frame False {
            # "Online Execution"
            n873 = Bundle By Name(cluster=w3791, "InspectionStatusToMI"="Fail_T") -> (w3788:T2)
            n874 = Bundle By Name(cluster=w3782, "ResultToMI"=FALSE ("PrevResultStatus")) -> (w3783:T1)
            n875 = Select(t=w3783, s=w3785, f=w3782) -> (s? t:f=w3781:T1)
            n876 = call "Output_SM.vi"("SM Private Data in"=w3792, "Output Cluster"=w3788, "Receiver Name"="MI", "State"="MI: InspectionStatus", "error in (no error)"=w3790) -> ("SM Private Data out"=w3780:refnum<class "Inspection Statemachine.lvclass">, "error out"=w3786:errorcluster)  [unwired: 9 in]
          }
          frame True {
            # "Offline Execution"
          }
        }
        n877 = case shown="\"MS:NotOkValidated\", \"MS:NotOkValidation\"" w3716 {
          tunnel: w3725 -> [w3752 w3773 w3777]
          tunnel: [w3743 w3766 w3777] -> w3724
          tunnel: w3723 -> [w3751 w3772 w3776]
          tunnel: [w3744 w3767 w3776] -> w3721
          tunnel: w3720 -> [w3735 w3757 _]
          tunnel: w3719 -> [_ _ _]
          tunnel: [w3739 w3771 w3778] -> w3718
          tunnel: w3717 -> [w3740 w3771 w3778]
          frame "MS:NotOkValidated", "MS:NotOkValidation" {
            n878 = call "Output_SM.vi"("SM Private Data in"=w3751, "Output Cluster"=w3735, "Receiver Name"="UI", "State"="UI: ResultData", "error in (no error)"=w3752) -> ("SM Private Data out"=w3748:refnum<class "Inspection Statemachine.lvclass">, "error out"=w3749:errorcluster)  [unwired: 9 in]
            n879 = Bundle By Name(cluster=w3740, "MasterSampleState"="MS:NotOkValidated" ("CurrentState")) -> (w3739:T1)
            n880 = Bundle By Name(cluster=w3735, "StateMsgToUI"="MasterSampleValidationPass" ("State")) -> (w3734:T2)
            n881 = call "Output_SM.vi"("SM Private Data in"=w3748, "Output Cluster"=w3734, "Receiver Name"="UI", "State"="UI: StateMessage", "error in (no error)"=w3749) -> ("SM Private Data out"=w3741:refnum<class "Inspection Statemachine.lvclass">, "error out"=w3742:errorcluster)  [unwired: 9 in]
            n882 = Bundle By Name(cluster=w3735, "MasterSampleMessages.PartMessage"="NOT OK\nSAMPLE\nVALIDATION", "MasterSampleMessages.MasterSampleMessage"="NOT OK sample validation is successful.\nPress NEXT button to start terminal inspection or press REPEAT button to repeat NOT OK sample validation." ("StateMsgToUI")) -> (w3745:T2)
            n883 = call "Output_SM.vi"("SM Private Data in"=w3741, "Output Cluster"=w3745, "Receiver Name"="UI", "State"="UI: MasterSampleMessages", "error in (no error)"=w3742) -> ("SM Private Data out"=w3744:refnum<class "Inspection Statemachine.lvclass">, "error out"=w3743:errorcluster)  [unwired: 9 in]
          }
          frame "MS:OkValidated", "MS:OkValidation" {
            n884 = call "Output_SM.vi"("SM Private Data in"=w3772, "Output Cluster"=w3757, "Receiver Name"="UI", "State"="UI: ResultData", "error in (no error)"=w3773) -> ("SM Private Data out"=w3759:refnum<class "Inspection Statemachine.lvclass">, "error out"=w3758:errorcluster)  [unwired: 9 in]
            n885 = Bundle By Name(cluster=w3757, "StateMsgToUI"="MasterSampleValidationFail" ("State")) -> (w3764:T2)
            n886 = call "Output_SM.vi"("SM Private Data in"=w3759, "Output Cluster"=w3764, "Receiver Name"="UI", "State"="UI: StateMessage", "error in (no error)"=w3758) -> ("SM Private Data out"=w3761:refnum<class "Inspection Statemachine.lvclass">, "error out"=w3760:errorcluster)  [unwired: 9 in]
            n887 = Bundle By Name(cluster=w3757, "MasterSampleMessages.PartMessage"="OK\nSAMPLE\nVALIDATION", "MasterSampleMessages.MasterSampleMessage"="OK sample validation has failed.\nPress REPEAT button to repeat OK sample validation or contact Zentron Labs." ("StateMsgToUI")) -> (w3768:T2)
            n888 = call "Output_SM.vi"("SM Private Data in"=w3761, "Output Cluster"=w3768, "Receiver Name"="UI", "State"="UI: MasterSampleMessages", "error in (no error)"=w3760) -> ("SM Private Data out"=w3767:refnum<class "Inspection Statemachine.lvclass">, "error out"=w3766:errorcluster)  [unwired: 9 in]
          }
          frame Default {
          }
        }
        n889 = call <vilib>:"Add State(s) to Queue__JKI_lib_State_Machine.vi"("State(s) in Front (\"\")"="Wait" ("State(s) in Front (\"\")"), "State(s) in (\"\")"=w3730) -> ("States Out"=w3731:string)  [unwired: 13 in]
      }
      frame "---------- Pause State ----------" {
        # "Do not put any code in this frame.\n(It is a separator no-op. You can make a copy of this frame to create a new UI frame)"
        n890 = call <vilib>:"Add State(s) to Queue__JKI_lib_State_Machine.vi"("State(s) in (\"\")"=w3800) -> ("States Out"=w3799:string)  [unwired: 14 in]
      }
      frame "Pause" {
        n891 = Unbundle By Name(w3806) -> ("OutputCluster.SystemParameters.SoftwareFeatures.PopupOptions.ReasonForPause"=w3809:bool, "OutputCluster.SystemParameters.SoftwareFeatures.HardwareEmulated"=w3817:bool, "CurrentState"=w3812:string, "OutputCluster"=w3804:T2, "OutputCluster.SystemParameters.SoftwareFeatures.DataLoggingEnable"=w3803:bool)
        n892 = case shown="Default" w3812 {
          selector: w3812 -> [w3836 _ w3959 w3986 w4026 w4055]
          tunnel: w3801 -> [w3838 w3870 w3954 w3985 w4025 w4050]
          tunnel: [w3837 w3857 w3949 w3983 w4024 w4054] -> w3819
          tunnel: [w3836 "Pause" ("Previous State") w3959 w3986 w4026 w4055] -> w3815
          tunnel: w3804 -> [w3839 w3864 w3957 w3981 w4023 w4044]
          tunnel: w3802 -> [w3840 w3869 w3955 w3982 w4022 w4047]
          tunnel: w3817 -> [_ w3846 w3952 w3984 _ w4046]
          tunnel: [w3835 w3856 w3950 w3978 w4021 w4053] -> w3813
          tunnel: w3809 -> [_ w3849 _ _ _ _]
          tunnel: w3806 -> [w3834 w3848 w3958 w3977 w4020 w4052]
          tunnel: [w3834 w3847 w3958 w3977 w4020 w4052] -> w3805
          tunnel: w3803 -> [_ w3845 _ w3976 w4019 w4045]
          frame "HardwareButtonDiagnostics" {
            n893 = Bundle By Name(cluster=w3839, "StateMsgToUI"="Pause") -> (w3841:T2)
            n894 = call "Output_SM.vi"("SM Private Data in"=w3840, "Output Cluster"=w3841, "Receiver Name"="UI", "State"="UI: StateMessage", "error in (no error)"=w3838) -> ("SM Private Data out"=w3835:refnum<class "Inspection Statemachine.lvclass">, "error out"=w3837:errorcluster)  [unwired: 9 in]
          }
          frame Default {
            n895 = Bundle By Name(cluster=w3864, "StateMsgToRC"="Pause") -> (w3863:T2)
            n896 = call "Output_SM.vi"("SM Private Data in"=w3869, "Output Cluster"=w3863, "Receiver Name"="RC", "State"="RC: StateMessage", "error in (no error)"=w3870) -> ("SM Private Data out"=w3855:refnum<class "Inspection Statemachine.lvclass">, "error out"=w3868:errorcluster)  [unwired: 9 in]
            n897 = case shown="False" w3846 {
              tunnel: w3868 -> [w3942 w3948]
              tunnel: w3864 -> [w3940 w3947]
              tunnel: [w3937 w3946] -> w3858
              tunnel: [w3941 w3948] -> w3866
              tunnel: [w3940 w3947] -> w3859
              tunnel: w3855 -> [w3938 w3946]
              frame False {
                # "Online execution"
                n898 = Bundle By Name(cluster=w3940, "StateMsgToMI"="Pause") -> (w3943:T2)
                n899 = call "Output_SM.vi"("SM Private Data in"=w3938, "Output Cluster"=w3943, "Receiver Name"="MI", "State"="MI: StateMessage", "error in (no error)"=w3942) -> ("SM Private Data out"=w3937:refnum<class "Inspection Statemachine.lvclass">, "error out"=w3941:errorcluster)  [unwired: 9 in]
              }
              frame True {
                # "Offline execution"
              }
            }
            n900 = Bundle By Name(cluster=w3859, "StateMsgToUI"="Pause") -> (w3850:T2)
            n901 = call "Output_SM.vi"("SM Private Data in"=w3858, "Output Cluster"=w3850, "Receiver Name"="UI", "State"="UI: StateMessage", "error in (no error)"=w3866) -> ("SM Private Data out"=w3852:refnum<class "Inspection Statemachine.lvclass">, "error out"=w3851:errorcluster)  [unwired: 9 in]
            n902 = case shown="False" w3849 {
              tunnel: w3851 -> [w3894 w3915]
              tunnel: [w3895 w3924] -> w3854
              tunnel: w3850 -> [w3893 w3916]
              tunnel: w3852 -> [w3897 w3917]
              tunnel: [w3896 w3920] -> w3853
              tunnel: w3848 -> [w3891 w3919]
              tunnel: [w3890 w3919] -> w3847
              tunnel: w3846 -> [_ w3918]
              tunnel: w3845 -> [w3892 _]
              frame False {
                n903 = case shown="True" w3892 {
                  tunnel: w3897 -> [w3899 w3908]
                  tunnel: [w3899 w3907] -> w3896
                  tunnel: [w3900 w3906] -> w3895
                  tunnel: w3894 -> [w3900 w3905]
                  tunnel: w3893 -> [_ w3904]
                  tunnel: w3891 -> [w3898 w3902]
                  tunnel: [w3898 w3901] -> w3890
                  frame False {
                    # "DL Disable"
                  }
                  frame True {
                    w3903 = "Not Listed: Pause" ("EventData.EventReason")
                    # "DL Enable"
                    n904 = Bundle By Name(cluster=w3904, "EventData.EventName"="Pause" ("DataLogger.EventDetails.EventName"), "EventData.EventReason"=w3903) -> (w3910:T2)
                    n905 = Bundle By Name(cluster=w3902, "EventReason"=w3903) -> (w3901:T1)
                    n906 = call "Output_SM.vi"("SM Private Data in"=w3908, "Output Cluster"=w3910, "Receiver Name"="DL", "State"="DL: EventDetails", "error in (no error)"=w3905) -> ("SM Private Data out"=w3907:refnum<class "Inspection Statemachine.lvclass">, "error out"=w3906:errorcluster)  [unwired: 9 in]
                  }
                }
              }
              frame True {
                n907 = case shown="True" w3918 {
                  tunnel: w3917 -> [w3931 w3935]
                  tunnel: w3916 -> [w3929 _]
                  tunnel: w3915 -> [w3928 w3936]
                  tunnel: [w3927 w3936] -> w3914
                  tunnel: [w3926 w3935] -> w3913
                  frame False {
                    n908 = Bundle By Name(cluster=w3929, "StateMsgToMI"="HardwareReset") -> (w3930:T2)
                    n909 = call "Output_SM.vi"("SM Private Data in"=w3931, "Output Cluster"=w3930, "Receiver Name"="MI", "State"="MI: StateMessage", "error in (no error)"=w3928) -> ("SM Private Data out"=w3926:refnum<class "Inspection Statemachine.lvclass">, "error out"=w3927:errorcluster)  [unwired: 9 in]
                  }
                  frame True {
                  }
                }
                n910 = Bundle By Name(cluster=w3916, "StateMsgToUI"="Pause") -> (w3922:T2)
                n911 = call "Output_SM.vi"("SM Private Data in"=w3913, "Output Cluster"=w3922, "Receiver Name"="UI", "State"="UI: AskEventReason", "error in (no error)"=w3914) -> ("SM Private Data out"=w3920:refnum<class "Inspection Statemachine.lvclass">, "error out"=w3924:errorcluster)  [unwired: 9 in]
              }
            }
            n912 = case shown="True" w3845 {
              tunnel: [w3873 w3889] -> w3857
              tunnel: [w3874 w3888] -> w3856
              tunnel: w3854 -> [w3873 w3881]
              tunnel: w3853 -> [w3874 w3879]
              tunnel: w3850 -> [_ w3880]
              frame False {
                # "DL Disable"
              }
              frame True {
                # "DL Enable"
                n913 = Bundle By Name(cluster=w3880, "MachineStatusToDL"="Pause" ("StateMsgToDL")) -> (w3885:T2)
                n914 = call "Output_SM.vi"("SM Private Data in"=w3879, "Output Cluster"=w3885, "Receiver Name"="DL", "State"="DL: MachineStatus", "error in (no error)"=w3881) -> ("SM Private Data out"=w3883:refnum<class "Inspection Statemachine.lvclass">, "error out"=w3882:errorcluster)  [unwired: 9 in]
                n915 = Bundle By Name(cluster=w3880, "StateMsgToDL"="Post") -> (w3876:T2)
                n916 = call "Output_SM.vi"("SM Private Data in"=w3883, "Output Cluster"=w3876, "Receiver Name"="DL", "State"="DL: StateMessage", "error in (no error)"=w3882) -> ("SM Private Data out"=w3888:refnum<class "Inspection Statemachine.lvclass">, "error out"=w3889:errorcluster)  [unwired: 9 in]
              }
            }
          }
          frame "Stop" {
            n917 = case shown="False" w3952 {
              tunnel: w3957 -> [w3965 w3975]
              tunnel: [w3968 w3974] -> w3956
              tunnel: w3955 -> [w3964 w3974]
              tunnel: w3954 -> [w3967 w3973]
              tunnel: [w3966 w3973] -> w3953
              tunnel: [w3965 w3975] -> w3951
              frame False {
                n918 = Bundle By Name(cluster=w3965, "StateMsgToMI"="Stop") -> (w3970:T2)
                n919 = call "Output_SM.vi"("SM Private Data in"=w3964, "Output Cluster"=w3970, "Receiver Name"="MI", "State"="MI: StateMessage", "error in (no error)"=w3967) -> ("SM Private Data out"=w3968:refnum<class "Inspection Statemachine.lvclass">, "error out"=w3966:errorcluster)  [unwired: 9 in]
              }
              frame True {
              }
            }
            n920 = Bundle By Name(cluster=w3951, "StateMsgToUI"="Pause") -> (w3960:T2)
            n921 = call "Output_SM.vi"("SM Private Data in"=w3956, "Output Cluster"=w3960, "Receiver Name"="UI", "State"="UI: StateMessage", "error in (no error)"=w3953) -> ("SM Private Data out"=w3950:refnum<class "Inspection Statemachine.lvclass">, "error out"=w3949:errorcluster)  [unwired: 9 in]
          }
          frame "PauseOnReelFinish" {
            n922 = case shown="False" w3984 {
              tunnel: w3982 -> [w4011 w4017]
              tunnel: w3985 -> [w4013 w4018]
              tunnel: w3981 -> [w4010 _]
              tunnel: [w4012 w4018] -> w3980
              tunnel: [w4008 w4017] -> w3979
              frame False {
                # "Online execution"
                n923 = Bundle By Name(cluster=w4010, "StateMsgToMI"="Pause") -> (w4014:T2)
                n924 = call "Output_SM.vi"("SM Private Data in"=w4011, "Output Cluster"=w4014, "Receiver Name"="MI", "State"="MI: StateMessage", "error in (no error)"=w4013) -> ("SM Private Data out"=w4008:refnum<class "Inspection Statemachine.lvclass">, "error out"=w4012:errorcluster)  [unwired: 9 in]
              }
              frame True {
                # "Offline execution"
              }
            }
            n925 = case shown="True" w3976 {
              tunnel: [w3987 w4003] -> w3983
              tunnel: w3981 -> [_ w3989]
              tunnel: w3980 -> [w3987 w3992]
              tunnel: w3979 -> [w3988 w3991]
              tunnel: [w3988 w3998] -> w3978
              frame False {
                # "DL Disable"
              }
              frame True {
                # "DL Enable"
                n926 = Bundle By Name(cluster=w3989, "MachineStatusToDL"="PauseOnReelFinish" ("StateMsgToDL")) -> (w3996:T2)
                n927 = call "Output_SM.vi"("SM Private Data in"=w3991, "Output Cluster"=w3996, "Receiver Name"="DL", "State"="DL: MachineStatus", "error in (no error)"=w3992) -> ("SM Private Data out"=w3990:refnum<class "Inspection Statemachine.lvclass">, "error out"=w3993:errorcluster)  [unwired: 9 in]
                n928 = call "Output_SM.vi"("SM Private Data in"=w3990, "Output Cluster"=w3989, "Receiver Name"="DL", "State"="DL: BatchDetails", "error in (no error)"=w3993) -> ("SM Private Data out"=w3999:refnum<class "Inspection Statemachine.lvclass">, "error out"=w4001:errorcluster)  [unwired: 9 in]
                n929 = Bundle By Name(cluster=w3989, "StateMsgToDL"="Post") -> (w4005:T2)
                n930 = call "Output_SM.vi"("SM Private Data in"=w3999, "Output Cluster"=w4005, "Receiver Name"="DL", "State"="DL: StateMessage", "error in (no error)"=w4001) -> ("SM Private Data out"=w3998:refnum<class "Inspection Statemachine.lvclass">, "error out"=w4003:errorcluster)  [unwired: 9 in]
              }
            }
          }
          frame "PauseOnFail" {
            n931 = case shown="True" w4019 {
              tunnel: w4025 -> [w4027 w4032]
              tunnel: [w4027 w4041] -> w4024
              tunnel: w4023 -> [_ w4033]
              tunnel: w4022 -> [w4028 w4030]
              tunnel: [w4028 w4038] -> w4021
              frame False {
                # "DL Disable"
              }
              frame True {
                # "DL Enable"
                n932 = Bundle By Name(cluster=w4033, "MachineStatusToDL"="PauseOnFail" ("StateMsgToDL")) -> (w4036:T2)
                n933 = call "Output_SM.vi"("SM Private Data in"=w4030, "Output Cluster"=w4036, "Receiver Name"="DL", "State"="DL: MachineStatus", "error in (no error)"=w4032) -> ("SM Private Data out"=w4031:refnum<class "Inspection Statemachine.lvclass">, "error out"=w4029:errorcluster)  [unwired: 9 in]
                n934 = Bundle By Name(cluster=w4033, "StateMsgToDL"="Post") -> (w4040:T2)
                n935 = call "Output_SM.vi"("SM Private Data in"=w4031, "Output Cluster"=w4040, "Receiver Name"="DL", "State"="DL: StateMessage", "error in (no error)"=w4029) -> ("SM Private Data out"=w4038:refnum<class "Inspection Statemachine.lvclass">, "error out"=w4041:errorcluster)  [unwired: 9 in]
              }
            }
          }
          frame "TotalFinish" {
            n936 = case shown="False" w4046 {
              tunnel: w4044 -> [w4072 w4082]
              tunnel: [w4075 w4081] -> w4048
              tunnel: w4047 -> [w4071 w4081]
              tunnel: w4050 -> [w4074 w4080]
              tunnel: [w4073 w4080] -> w4051
              tunnel: [w4072 w4082] -> w4049
              frame False {
                n937 = Bundle By Name(cluster=w4072, "StateMsgToMI"="Stop") -> (w4077:T2)
                n938 = call "Output_SM.vi"("SM Private Data in"=w4071, "Output Cluster"=w4077, "Receiver Name"="MI", "State"="MI: StateMessage", "error in (no error)"=w4074) -> ("SM Private Data out"=w4075:refnum<class "Inspection Statemachine.lvclass">, "error out"=w4073:errorcluster)  [unwired: 9 in]
              }
              frame True {
              }
            }
            n939 = case shown="True" w4045 {
              tunnel: [w4056 w4068] -> w4054
              tunnel: [w4057 w4067] -> w4053
              tunnel: w4051 -> [w4056 w4059]
              tunnel: w4049 -> [_ _]
              tunnel: w4048 -> [w4057 w4060]
              tunnel: w4044 -> [_ w4058]
              frame False {
                # "DL Disable"
              }
              frame True {
                # "DL Enable"
                n940 = Bundle By Name(cluster=w4058, "MachineStatusToDL"="PauseOnTotalFinish" ("StateMsgToDL")) -> (w4065:T2)
                n941 = call "Output_SM.vi"("SM Private Data in"=w4060, "Output Cluster"=w4065, "Receiver Name"="DL", "State"="DL: MachineStatus", "error in (no error)"=w4059) -> ("SM Private Data out"=w4061:refnum<class "Inspection Statemachine.lvclass">, "error out"=w4062:errorcluster)  [unwired: 9 in]
                n942 = call "Output_SM.vi"("SM Private Data in"=w4061, "Output Cluster"=w4058, "Receiver Name"="DL", "State"="DL: BatchDetails", "error in (no error)"=w4062) -> ("SM Private Data out"=w4067:refnum<class "Inspection Statemachine.lvclass">, "error out"=w4068:errorcluster)  [unwired: 9 in]
              }
            }
          }
        }
        n943 = Bundle By Name(cluster=w3805, "CurrentState"=w3815, "ResultToMI"=FALSE, "UpdateInPause"=TRUE ("ResultToMI")) -> (w3808:T1)
        n944 = case shown="Default" w3812 {
          tunnel: w3819 -> [w3823 w3833]
          tunnel: ["" w3832] -> w3818
          tunnel: [w3823 w3831] -> w3816
          tunnel: w3815 -> [_ w3830]
          tunnel: w3804 -> [_ w3829]
          tunnel: w3814 -> [_ w3828]
          tunnel: w3813 -> [_ w3827]
          tunnel: w3808 -> [w3824 w3826]
          tunnel: [w3824 w3825] -> w3807
          frame "HardwareButtonDiagnostics" {
          }
          frame Default {
            n945 = call "EventInPause_SM.vi"("SM Private Data"=w3827, "LocalData_SM in"=w3826, "Event Registration Refnum"=w3828, "CurrentState"=w3830, "Output Cluster"=w3829, "error in (no error)"=w3833) -> ("LocalData_SM out"=w3825:T1, "NextState"=w3832:string, "error out"=w3831:errorcluster)  [unwired: 7 in]
          }
        }
        n946 = call <vilib>:"Add State(s) to Queue__JKI_lib_State_Machine.vi"("State(s) in Front (\"\")"=w3818, "State(s) in (\"\")"=w3820) -> ("States Out"=w3821:string)  [unwired: 13 in]
      }
      frame "ReelFinish" {
        n947 = in-place {
          in-place-border: w4088 -> [w4119]
          in-place-border: w4084 -> [w4104]
          in-place-border: [w4115] -> w4087
          in-place-border: [w4107] -> w4083
          n948 = in-place-cluster #14(w4086) -> ("OutputCluster"=w4093:T2)  [unwired: 2 out]
          n949 = Unbundle By Name(w4093) -> ("SystemParameters.SoftwareFeatures.DataLoggingEnable"=w4092:bool)
          n950 = case shown="True" w4092 {
            tunnel: w4119 -> [w4121 w4134]
            tunnel: [w4121 w4131] -> w4106
            tunnel: [w4120 w4125] -> w4105
            tunnel: w4104 -> [w4120 w4124]
            tunnel: w4093 -> [_ w4122]
            frame False {
              # "DL Disable"
            }
            frame True {
              # "DL Enable"
              n951 = Bundle By Name(cluster=w4122, "EventData.EventName"="BatchEnd" ("DataLogger.EventDetails.EventName"), "EventData.EventReason"="Batch End" ("DataLogger.EventDetails.EventReason")) -> (w4135:T2)
              n952 = call "Output_SM.vi"("SM Private Data in"=w4124, "Output Cluster"=w4135, "Receiver Name"="DL", "State"="DL: EventDetails", "error in (no error)"=w4134) -> ("SM Private Data out"=w4123:refnum<class "Inspection Statemachine.lvclass">, "error out"=w4132:errorcluster)  [unwired: 9 in]
              n953 = Bundle By Name(cluster=w4122, "EventData.EventName"="Pause" ("DataLogger.EventDetails.EventName"), "EventData.EventReason"="Batch End" ("DataLogger.EventDetails.EventReason")) -> (w4127:T2)
              n954 = call "Output_SM.vi"("SM Private Data in"=w4123, "Output Cluster"=w4127, "Receiver Name"="DL", "State"="DL: EventDetails", "error in (no error)"=w4132) -> ("SM Private Data out"=w4125:refnum<class "Inspection Statemachine.lvclass">, "error out"=w4131:errorcluster)  [unwired: 9 in]
            }
          }
          n955 = Bundle By Name(cluster=w4093, "StateMsgToUI"="Pause") -> (w4097:T2)
          n956 = Unbundle By Name(w4093) -> ("SystemParameters.SoftwareFeatures.AnalyticsEnable"=w4094:bool)
          n957 = call "Output_SM.vi"("SM Private Data in"=w4105, "Output Cluster"=w4097, "Receiver Name"="UI", "State"="UI: StateMessage", "error in (no error)"=w4106) -> ("SM Private Data out"=w4108:refnum<class "Inspection Statemachine.lvclass">, "error out"=w4116:errorcluster)  [unwired: 9 in]
          n958 = in-place {
            n959 = in-place-cluster #15(w4093) -> ("Result Cluster.ReelNumber"=w4149:u64)
            n960 = Increment(x=w4149) -> (x+1=w4148:u64)
            n961 = in-place-cluster #15("Result Cluster.ReelNumber"=w4148) -> (w4111:T2)
          }
          n962 = call "Output_SM.vi"("SM Private Data in"=w4108, "Output Cluster"=w4097, "Receiver Name"="UI", "State"="UI: ResultData", "error in (no error)"=w4116) -> ("SM Private Data out"=w4101:refnum<class "Inspection Statemachine.lvclass">, "error out"=w4100:errorcluster)  [unwired: 9 in]
          n963 = Bundle By Name(cluster=w4097, "StateMsgToUI"="Complete>>Reel") -> (w4099:T2)
          n964 = call "Output_SM.vi"("SM Private Data in"=w4101, "Output Cluster"=w4099, "Receiver Name"="UI", "State"="UI: StateMessage", "error in (no error)"=w4100) -> ("SM Private Data out"=w4098:refnum<class "Inspection Statemachine.lvclass">, "error out"=w4095:errorcluster)  [unwired: 9 in]
          n965 = case shown="True" w4094 {
            tunnel: [w4139 w4146] -> w4115
            tunnel: [w4140 w4144] -> w4107
            tunnel: w4098 -> [w4140 w4143]
            tunnel: w4097 -> [_ w4142]
            tunnel: w4095 -> [w4139 w4141]
            frame False {
            }
            frame True {
              n966 = call "Output_SM.vi"("SM Private Data in"=w4143, "Output Cluster"=w4142, "Receiver Name"="AN", "State"="AN: GetStatisticalparameters", "error in (no error)"=w4141) -> ("SM Private Data out"=w4144:refnum<class "Inspection Statemachine.lvclass">, "error out"=w4146:errorcluster)  [unwired: 9 in]
            }
          }
          n967 = in-place-cluster #14("BatchStart"=TRUE ("ReelInfo.BatchStartOrNot"), "CurrentState"="PauseOnReelFinish", "OutputCluster"=w4111) -> (w4085:T1)
        }
        n968 = call <vilib>:"Add State(s) to Queue__JKI_lib_State_Machine.vi"("State(s) in Front (\"\")"="Pause" ("State(s) in Front (\"\")"), "State(s) in (\"\")"=w4089) -> ("States Out"=w4091:string)  [unwired: 13 in]
      }
      frame "TotalFinish" {
        n969 = in-place {
          in-place-border: w4152 -> [w4184]
          in-place-border: w4154 -> [w4172]
          in-place-border: [w4181] -> w4151
          in-place-border: [w4175] -> w4153
          n970 = in-place-cluster #16(w4155) -> ("OutputCluster"=w4160:T2)  [unwired: 1 out]
          n971 = Unbundle By Name(w4160) -> ("SystemParameters.SoftwareFeatures.DataLoggingEnable"=w4159:bool)
          n972 = case shown="True" w4159 {
            tunnel: w4184 -> [w4186 w4199]
            tunnel: [w4186 w4191] -> w4174
            tunnel: [w4185 w4190] -> w4173
            tunnel: w4172 -> [w4185 w4189]
            tunnel: w4160 -> [_ w4187]
            frame False {
              # "DL Disable"
            }
            frame True {
              # "DL Enable"
              n973 = Bundle By Name(cluster=w4187, "EventData.EventName"="BatchEnd" ("DataLogger.EventDetails.EventName"), "EventData.EventReason"="Batch End" ("DataLogger.EventDetails.EventReason")) -> (w4200:T2)
              n974 = call "Output_SM.vi"("SM Private Data in"=w4189, "Output Cluster"=w4200, "Receiver Name"="DL", "State"="DL: EventDetails", "error in (no error)"=w4199) -> ("SM Private Data out"=w4188:refnum<class "Inspection Statemachine.lvclass">, "error out"=w4192:errorcluster)  [unwired: 9 in]
              n975 = Bundle By Name(cluster=w4187, "EventData.EventName"="Stop" ("DataLogger.EventDetails.EventName"), "EventData.EventReason"="Production End" ("DataLogger.EventDetails.EventReason")) -> (w4194:T2)
              n976 = call "Output_SM.vi"("SM Private Data in"=w4188, "Output Cluster"=w4194, "Receiver Name"="DL", "State"="DL: EventDetails", "error in (no error)"=w4192) -> ("SM Private Data out"=w4190:refnum<class "Inspection Statemachine.lvclass">, "error out"=w4191:errorcluster)  [unwired: 9 in]
            }
          }
          n977 = Bundle By Name(cluster=w4160, "StateMsgToUI"="Pause") -> (w4162:T2)
          n978 = call "Output_SM.vi"("SM Private Data in"=w4173, "Output Cluster"=w4162, "Receiver Name"="UI", "State"="UI: StateMessage", "error in (no error)"=w4174) -> ("SM Private Data out"=w4176:refnum<class "Inspection Statemachine.lvclass">, "error out"=w4182:errorcluster)  [unwired: 9 in]
          n979 = Unbundle By Name(w4160) -> ("SystemParameters.SoftwareFeatures.AnalyticsEnable"=w4161:bool)
          n980 = call "Output_SM.vi"("SM Private Data in"=w4176, "Output Cluster"=w4162, "Receiver Name"="UI", "State"="UI: ResultData", "error in (no error)"=w4182) -> ("SM Private Data out"=w4164:refnum<class "Inspection Statemachine.lvclass">, "error out"=w4165:errorcluster)  [unwired: 9 in]
          n981 = Bundle By Name(cluster=w4162, "StateMsgToUI"="Complete>>Production") -> (w4168:T2)
          n982 = call "Output_SM.vi"("SM Private Data in"=w4164, "Output Cluster"=w4168, "Receiver Name"="UI", "State"="UI: StateMessage", "error in (no error)"=w4165) -> ("SM Private Data out"=w4166:refnum<class "Inspection Statemachine.lvclass">, "error out"=w4163:errorcluster)  [unwired: 9 in]
          n983 = case shown="True" w4161 {
            tunnel: [w4204 w4211] -> w4181
            tunnel: [w4205 w4209] -> w4175
            tunnel: w4166 -> [w4205 w4208]
            tunnel: w4163 -> [w4204 w4207]
            tunnel: w4162 -> [_ w4206]
            frame False {
            }
            frame True {
              n984 = call "Output_SM.vi"("SM Private Data in"=w4208, "Output Cluster"=w4206, "Receiver Name"="AN", "State"="AN: GetStatisticalparameters", "error in (no error)"=w4207) -> ("SM Private Data out"=w4209:refnum<class "Inspection Statemachine.lvclass">, "error out"=w4211:errorcluster)  [unwired: 9 in]
            }
          }
          n985 = in-place-cluster #16("CurrentState"="TotalFinish", "OutputCluster"=w4160) -> (w4150:T1)
        }
        n986 = call <vilib>:"Add State(s) to Queue__JKI_lib_State_Machine.vi"("State(s) in Front (\"\")"="Stop" ("State(s) in Front (\"\")"), "State(s) in (\"\")"=w4156) -> ("States Out"=w4158:string)  [unwired: 13 in]
      }
      frame "Fail" {
        n987 = Unbundle By Name(w4239) -> ("OutputCluster.SystemParameters.SoftwareFeatures.PopupOptions.ReasonForFail"=w4230:bool, "OutputCluster.SystemParameters.SoftwareFeatures.HardwareEmulated"=w4236:bool, "ResultToMI"=w4238:bool, "OutputCluster"=w4216:T2)  [unwired: 1 out]
        n988 = case shown="False" w4236 {
          tunnel: w4237 -> [w4294 w4299]
          tunnel: [w4290 w4299] -> w4235
          tunnel: w4239 -> [w4286 w4298]
          tunnel: [w4285 w4298] -> w4228
          tunnel: w4238 -> [w4289 _]
          tunnel: w4232 -> [w4296 w4297]
          tunnel: w4216 -> [w4295 _]
          tunnel: [w4284 w4297] -> w4233
          tunnel: w4230 -> [w4283 _]
          frame False {
            # "Online Execution"
            n989 = Select(t="Fail_T" ("InspectionStatusToMI"), s=w4283, f="Fail_F" ("InspectionStatusToMI")) -> (s? t:f=w4282:string)
            n990 = Bundle By Name(cluster=w4295, "InspectionStatusToMI"=w4282) -> (w4292:T2)
            n991 = Bundle By Name(cluster=w4286, "ResultToMI"=FALSE ("PrevResultStatus")) -> (w4287:T1)
            n992 = Select(t=w4287, s=w4289, f=w4286) -> (s? t:f=w4285:T1)
            n993 = call "Output_SM.vi"("SM Private Data in"=w4296, "Output Cluster"=w4292, "Receiver Name"="MI", "State"="MI: InspectionStatus", "error in (no error)"=w4294) -> ("SM Private Data out"=w4284:refnum<class "Inspection Statemachine.lvclass">, "error out"=w4290:errorcluster)  [unwired: 9 in]
          }
          frame True {
            # "Offline Execution"
          }
        }
        n994 = Bundle By Name(cluster=w4216, "StateMsgToUI"="Pause") -> (w4221:T2)
        n995 = call "Output_SM.vi"("SM Private Data in"=w4233, "Output Cluster"=w4221, "Receiver Name"="UI", "State"="UI: StateMessage", "error in (no error)"=w4235) -> ("SM Private Data out"=w4218:refnum<class "Inspection Statemachine.lvclass">, "error out"=w4224:errorcluster)  [unwired: 9 in]
        n996 = Unbundle By Name(w4216) -> ("SystemParameters.SoftwareFeatures.DataLoggingEnable"=w4215:bool)
        n997 = call "Output_SM.vi"("SM Private Data in"=w4218, "Output Cluster"=w4216, "Receiver Name"="UI", "State"="UI: ResultData", "error in (no error)"=w4224) -> ("SM Private Data out"=w4214:refnum<class "Inspection Statemachine.lvclass">, "error out"=w4213:errorcluster)  [unwired: 9 in]
        n998 = Bundle By Name(cluster=w4228, "CurrentState"="PauseOnFail") -> (w4217:T1)
        n999 = case shown="False" w4230 {
          tunnel: w4213 -> [w4248 w4272]
          tunnel: [w4243 w4278] -> w4234
          tunnel: w4216 -> [w4247 w4271]
          tunnel: w4214 -> [w4249 w4273]
          tunnel: [w4244 w4274] -> w4231
          tunnel: w4217 -> [w4246 w4270]
          tunnel: [w4245 w4270] -> w4229
          tunnel: w4215 -> [w4242 _]
          frame False {
            # "Fail Reason Disabled"
            n1000 = case shown="True" w4242 {
              tunnel: w4249 -> [w4252 w4254]
              tunnel: w4248 -> [w4251 w4256]
              tunnel: w4247 -> [_ w4266]
              tunnel: w4246 -> [w4250 w4253]
              tunnel: [w4250 w4263] -> w4245
              tunnel: [w4252 w4261] -> w4244
              tunnel: [w4251 w4262] -> w4243
              frame False {
                # "DL Disable"
              }
              frame True {
                w4265 = "Not Listed: Fail" ("EventData.EventReason")
                # "DL Enable"
                n1001 = Unbundle By Name(w4253) -> ("OutputCluster"=w4258:T2)
                n1002 = call "Output_SM.vi"("SM Private Data in"=w4254, "Output Cluster"=w4258, "Receiver Name"="DL", "State"="DL: FailureDetails", "error in (no error)"=w4256) -> ("SM Private Data out"=w4255:refnum<class "Inspection Statemachine.lvclass">, "error out"=w4257:errorcluster)  [unwired: 9 in]
                n1003 = Bundle By Name(cluster=w4266, "EventData.EventName"="FailPause" ("DataLogger.EventDetails.EventName"), "EventData.EventReason"=w4265) -> (w4264:T2)
                n1004 = Bundle By Name(cluster=w4253, "EventReason"=w4265) -> (w4263:T1)
                n1005 = call "Output_SM.vi"("SM Private Data in"=w4255, "Output Cluster"=w4264, "Receiver Name"="DL", "State"="DL: EventDetails", "error in (no error)"=w4257) -> ("SM Private Data out"=w4261:refnum<class "Inspection Statemachine.lvclass">, "error out"=w4262:errorcluster)  [unwired: 9 in]
              }
            }
          }
          frame True {
            # "Fail Reason Enabled"
            n1006 = Bundle By Name(cluster=w4271, "StateMsgToUI"="Fail") -> (w4276:T2)
            n1007 = call "Output_SM.vi"("SM Private Data in"=w4273, "Output Cluster"=w4276, "Receiver Name"="UI", "State"="UI: AskEventReason", "error in (no error)"=w4272) -> ("SM Private Data out"=w4274:refnum<class "Inspection Statemachine.lvclass">, "error out"=w4278:errorcluster)  [unwired: 9 in]
          }
        }
        n1008 = call <vilib>:"Add State(s) to Queue__JKI_lib_State_Machine.vi"("State(s) in Front (\"\")"="Pause" ("State(s) in Front (\"\")"), "State(s) in (\"\")"=w4240) -> ("States Out"=w4241:string)  [unwired: 13 in]
      }
      frame "Update" {
        n1009 = Unbundle By Name(w4301) -> ("OutputCluster"=w4304:T2, "CurrentState"=w4305:string)
        n1010 = case shown="\"Pause\", \"PauseOnFail\", \"PauseOnReelFinish\"" w4305 {
          tunnel: w4307 -> [w4312 w4325]
          tunnel: [w4312 w4318] -> w4306
          tunnel: w4303 -> [w4311 w4324]
          tunnel: w4304 -> [_ w4323]
          tunnel: [w4311 w4316] -> w4302
          tunnel: w4301 -> [w4310 w4314]
          tunnel: [w4310 w4313] -> w4300
          frame "Pause", "PauseOnFail", "PauseOnReelFinish" {
          }
          frame Default {
            n1011 = Bundle By Name(cluster=w4323, "StateMsgToRC"="Update") -> (w4322:T2)
            n1012 = call "Output_SM.vi"("SM Private Data in"=w4324, "Output Cluster"=w4322, "Receiver Name"="RC", "State"="RC: StateMessage", "error in (no error)"=w4325) -> ("SM Private Data out"=w4316:refnum<class "Inspection Statemachine.lvclass">, "error out"=w4317:errorcluster)  [unwired: 9 in]
            n1013 = Unbundle By Name(w4316) -> ("GtronSystemJSONOverride"=w4315:path)
            n1014 = call "UpdateSystemParams_SM.vi"("error in (no error)"=w4317, "Override File Path"=w4315, "Cluster In"=w4314) -> ("error out"=w4318:errorcluster, "Cluster Out"=w4313:T1)  [unwired: 7 in]
          }
        }
        n1015 = call <vilib>:"Add State(s) to Queue__JKI_lib_State_Machine.vi"("State(s) in (\"\")"=w4308) -> ("States Out"=w4309:string)  [unwired: 14 in]
      }
      frame "Analytics", "Images" {
        n1016 = Unbundle By Name(w4334) -> ("OutputCluster"=w4333:T2, "CurrentState"=w4327:string, "OutputCluster.SystemParameters.SoftwareFeatures.AnalyticsEnable"=w4326:bool)
        n1017 = case shown="\"Pause\", \"PauseOnFail\", \"Run\"" w4327 {
          tunnel: w4329 -> [w4337 w4345]
          tunnel: w4333 -> [_ w4344]
          tunnel: w4332 -> [w4338 w4343]
          tunnel: [w4338 w4342] -> w4331
          tunnel: w4330 -> [_ w4341]
          tunnel: [w4337 w4340] -> w4328
          tunnel: w4326 -> [_ w4339]
          frame Default {
          }
          frame "Pause", "PauseOnFail", "Run" {
            n1018 = case shown="\"Analytics\"" w4341 {
              tunnel: w4345 -> [w4349 w4370]
              tunnel: w4344 -> [w4351 w4372]
              tunnel: w4343 -> [w4357 w4378]
              tunnel: [w4354 w4375] -> w4342
              tunnel: [w4347 w4368] -> w4340
              tunnel: w4339 -> [w4346 w4367]
              frame "Images", Default {
                n1019 = case shown="True" w4346 {
                  tunnel: w4357 -> [w4358 w4364]
                  tunnel: [w4358 w4363] -> w4355
                  tunnel: w4351 -> [_ w4362]
                  tunnel: w4349 -> [w4359 w4361]
                  tunnel: [w4359 w4360] -> w4348
                  frame False {
                  }
                  frame True {
                    n1020 = call "Output_SM.vi"("SM Private Data in"=w4361, "Output Cluster"=w4362, "Receiver Name"="AN", "State"="AN: ToImages", "error in (no error)"=w4364) -> ("SM Private Data out"=w4360:refnum<class "Inspection Statemachine.lvclass">, "error out"=w4363:errorcluster)  [unwired: 9 in]
                  }
                }
                n1021 = Bundle By Name(cluster=w4351, "StateMsgToUI"="DisplayImages") -> (w4350:T2)
                n1022 = call "Output_SM.vi"("SM Private Data in"=w4348, "Output Cluster"=w4350, "Receiver Name"="UI", "State"="UI: StateMessage", "error in (no error)"=w4355) -> ("SM Private Data out"=w4347:refnum<class "Inspection Statemachine.lvclass">, "error out"=w4354:errorcluster)  [unwired: 9 in]
              }
              frame "Analytics" {
                n1023 = case shown="False" w4367 {
                  tunnel: w4378 -> [w4380 w4385]
                  tunnel: [w4380 w4384] -> w4376
                  tunnel: w4372 -> [_ w4383]
                  tunnel: w4370 -> [w4379 w4382]
                  tunnel: [w4379 w4381] -> w4369
                  frame False {
                  }
                  frame True {
                    n1024 = call "Output_SM.vi"("SM Private Data in"=w4382, "Output Cluster"=w4383, "Receiver Name"="AN", "State"="AN: ToAnalytics", "error in (no error)"=w4385) -> ("SM Private Data out"=w4381:refnum<class "Inspection Statemachine.lvclass">, "error out"=w4384:errorcluster)  [unwired: 9 in]
                  }
                }
                n1025 = Bundle By Name(cluster=w4372, "StateMsgToUI"="DisplayAnalyticsGraphs") -> (w4371:T2)
                n1026 = call "Output_SM.vi"("SM Private Data in"=w4369, "Output Cluster"=w4371, "Receiver Name"="UI", "State"="UI: StateMessage", "error in (no error)"=w4376) -> ("SM Private Data out"=w4368:refnum<class "Inspection Statemachine.lvclass">, "error out"=w4375:errorcluster)  [unwired: 9 in]
              }
            }
          }
        }
        n1027 = call <vilib>:"Add State(s) to Queue__JKI_lib_State_Machine.vi"("State(s) in (\"\")"=w4335) -> ("States Out"=w4336:string)  [unwired: 14 in]
      }
      frame "---------- Stop State ----------" {
        # "Do not put any code in this frame.\n(It is a separator no-op. You can make a copy of this frame to create a new UI frame)"
        n1028 = call <vilib>:"Add State(s) to Queue__JKI_lib_State_Machine.vi"("State(s) in (\"\")"=w4392) -> ("States Out"=w4391:string)  [unwired: 14 in]
      }
      frame "Stop" {
        n1029 = Unbundle By Name(w4401) -> ("OutputCluster.SystemParameters.SoftwareFeatures.HardwareEmulated"=w4402:bool, "CurrentState"=w4399:string, "OutputCluster.SystemParameters.SoftwareFeatures.AutomaticGuideMovement"=w4398:bool, "OutputCluster"=w4395:T2)
        n1030 = case shown="\"Pause\", Default" w4399 {
          selector: w4399 -> [_ w4418]
          tunnel: w4396 -> [w4410 w4433]
          tunnel: w4402 -> [_ w4430]
          tunnel: w4401 -> [w4415 w4416]
          tunnel: [w4415 w4417] -> w4400
          tunnel: [w4409 w4432] -> w4397
          tunnel: w4398 -> [_ w4431]
          tunnel: w4394 -> [w4408 w4421]
          tunnel: w4395 -> [w4407 w4426]
          tunnel: [w4406 w4419] -> w4393
          frame "HardwareButtonDiagnostics" {
            n1031 = Bundle By Name(cluster=w4407, "StateMsgToUI"="Stop") -> (w4411:T2)
            n1032 = call "Output_SM.vi"("SM Private Data in"=w4408, "Output Cluster"=w4411, "Receiver Name"="UI", "State"="UI: StateMessage", "error in (no error)"=w4410) -> ("SM Private Data out"=w4406:refnum<class "Inspection Statemachine.lvclass">, "error out"=w4409:errorcluster)  [unwired: 9 in]
          }
          frame "Pause", Default {
            n1033 = case shown="Default" w4418 {
              tunnel: w4433 -> [w4509 w4521]
              tunnel: [w4509 w4513] -> w4429
              tunnel: w4421 -> [w4508 w4512]
              tunnel: w4430 -> [_ w4518]
              tunnel: w4426 -> [_ w4514]
              tunnel: [w4508 w4510] -> w4422
              frame "Pause" {
              }
              frame Default {
                n1034 = Bundle By Name(cluster=w4514, "StateMsgToRC"="Pause") -> (w4516:T2)
                n1035 = call "Output_SM.vi"("SM Private Data in"=w4512, "Output Cluster"=w4516, "Receiver Name"="RC", "State"="RC: StateMessage", "error in (no error)"=w4521) -> ("SM Private Data out"=w4511:refnum<class "Inspection Statemachine.lvclass">, "error out"=w4519:errorcluster)  [unwired: 9 in]
                n1036 = case shown="False" w4518 {
                  tunnel: w4511 -> [w4525 w4531]
                  tunnel: w4519 -> [w4527 w4532]
                  tunnel: w4514 -> [w4524 _]
                  tunnel: [w4526 w4532] -> w4513
                  tunnel: [w4522 w4531] -> w4510
                  frame False {
                    # "Online execution"
                    n1037 = Bundle By Name(cluster=w4524, "StateMsgToMI"="Pause") -> (w4528:T2)
                    n1038 = call "Output_SM.vi"("SM Private Data in"=w4525, "Output Cluster"=w4528, "Receiver Name"="MI", "State"="MI: StateMessage", "error in (no error)"=w4527) -> ("SM Private Data out"=w4522:refnum<class "Inspection Statemachine.lvclass">, "error out"=w4526:errorcluster)  [unwired: 9 in]
                  }
                  frame True {
                    # "Offline execution"
                  }
                }
              }
            }
            n1039 = Bundle By Name(cluster=w4426, "StateMsgToUI"="DisableAllButtons") -> (w4425:T2)
            n1040 = call "Output_SM.vi"("SM Private Data in"=w4422, "Output Cluster"=w4425, "Receiver Name"="UI", "State"="UI: StateMessage" ("Functionality name"), "error in (no error)"=w4429) -> ("SM Private Data out"=w4420:refnum<class "Inspection Statemachine.lvclass">, "error out"=w4428:errorcluster)  [unwired: 9 in]
            n1041 = case shown="\"TotalFinish\"" w4418 {
              tunnel: [w4436 w4483] -> w4432
              tunnel: w4431 -> [w4443 w4482]
              tunnel: w4428 -> [w4442 w4481]
              tunnel: w4425 -> [w4441 w4480]
              tunnel: w4420 -> [w4444 w4479]
              tunnel: [w4445 w4478] -> w4419
              tunnel: [w4438 w4475] -> w4417
              tunnel: w4416 -> [w4437 w4474]
              frame Default {
                n1042 = case shown="True" w4443 {
                  tunnel: [w4454 w4468] -> w4436
                  tunnel: w4442 -> [w4455 w4466]
                  tunnel: w4444 -> [w4456 w4467]
                  tunnel: w4441 -> [w4451 w4464]
                  tunnel: [w4446 w4459] -> w4445
                  frame True {
                    # "Automatic Guide Movement Enabled"
                    n1043 = Bundle By Name(cluster=w4451, "PopupInput.Title"="MESSAGE" ("Dialog Box Input"), "PopupInput.Message"="Please remove the terminals before the guides are opened" ("Message Input"), "PopupInput.Button 1 Text"="Continue" ("Boolean Text.Text"), "PopupInput.Pop-up Type"=T8."Two button dialog box", "PopupInput.Button 2 Text"="Cancel" ("buttons.Button 2 label")) -> (w4453:T2)
                    n1044 = call "Output_SM.vi"("SM Private Data in"=w4456, "Output Cluster"=w4453, "Receiver Name"="UI", "State"="UI: DisplayPopup", "error in (no error)"=w4455) -> ("SM Private Data out"=w4446:refnum<class "Inspection Statemachine.lvclass">, "error out"=w4454:errorcluster)  [unwired: 9 in]
                  }
                  frame False {
                    # "Automatic Guide Movement Disabled"
                    n1045 = Bundle By Name(cluster=w4464, "PopupInput.Title"="MESSAGE" ("Dialog Box Input"), "PopupInput.Message"="Please remove the terminals" ("Message Input"), "PopupInput.Button 1 Text"="Continue" ("Boolean Text.Text"), "PopupInput.Pop-up Type"=T8."Two button dialog box", "PopupInput.Button 2 Text"="Cancel" ("buttons.Button 2 label")) -> (w4470:T2)
                    n1046 = call "Output_SM.vi"("SM Private Data in"=w4467, "Output Cluster"=w4470, "Receiver Name"="UI", "State"="UI: DisplayPopup", "error in (no error)"=w4466) -> ("SM Private Data out"=w4459:refnum<class "Inspection Statemachine.lvclass">, "error out"=w4468:errorcluster)  [unwired: 9 in]
                  }
                }
                n1047 = Bundle By Name(cluster=w4437, "CurrentState"="Stop" ("Previous State"), "SoftwareExit"=FALSE ("Software Exit?"), "PopUpCategory"="Stop", "PopUpActive"=TRUE) -> (w4438:T1)
              }
              frame "TotalFinish" {
                n1048 = case shown="True" w4482 {
                  tunnel: [w4491 w4504] -> w4483
                  tunnel: w4481 -> [w4492 w4502]
                  tunnel: w4479 -> [w4493 w4503]
                  tunnel: w4480 -> [w4488 w4500]
                  tunnel: [w4484 w4496] -> w4478
                  frame True {
                    # "Automatic Guide Movement Enabled"
                    n1049 = Bundle By Name(cluster=w4488, "PopupInput.Title"="MESSAGE" ("Dialog Box Input"), "PopupInput.Message"="Please remove the terminals before the guides are opened" ("Message Input"), "PopupInput.Button 1 Text"="Continue" ("Boolean Text.Text"), "PopupInput.Pop-up Type"=T8."One button dialog box") -> (w4490:T2)
                    n1050 = call "Output_SM.vi"("SM Private Data in"=w4493, "Output Cluster"=w4490, "Receiver Name"="UI", "State"="UI: DisplayPopup", "error in (no error)"=w4492) -> ("SM Private Data out"=w4484:refnum<class "Inspection Statemachine.lvclass">, "error out"=w4491:errorcluster)  [unwired: 9 in]
                  }
                  frame False {
                    # "Automatic Guide Movement Disabled"
                    n1051 = Bundle By Name(cluster=w4500, "PopupInput.Title"="MESSAGE" ("Dialog Box Input"), "PopupInput.Message"="Please remove the terminals" ("Message Input"), "PopupInput.Button 1 Text"="Continue" ("Boolean Text.Text"), "PopupInput.Pop-up Type"=T8."One button dialog box") -> (w4506:T2)
                    n1052 = call "Output_SM.vi"("SM Private Data in"=w4503, "Output Cluster"=w4506, "Receiver Name"="UI", "State"="UI: DisplayPopup", "error in (no error)"=w4502) -> ("SM Private Data out"=w4496:refnum<class "Inspection Statemachine.lvclass">, "error out"=w4504:errorcluster)  [unwired: 9 in]
                  }
                }
                n1053 = Bundle By Name(cluster=w4474, "CurrentState"="TotalFinish" ("Previous State"), "SoftwareExit"=FALSE ("Software Exit?"), "PopUpCategory"="TotalFinish", "PopUpActive"=TRUE) -> (w4475:T1)
              }
            }
          }
        }
        n1054 = call <vilib>:"Add State(s) to Queue__JKI_lib_State_Machine.vi"("State(s) in Front (\"\")"="Pause" ("State(s) in Front (\"\")"), "State(s) in (\"\")"=w4403) -> ("States Out"=w4405:string)  [unwired: 13 in]
      }
      frame "CloseConfirm" {
        n1055 = Unbundle By Name(w4535) -> ("OutputCluster.SystemParameters.SoftwareFeatures.HardwareEmulated"=w4542:bool, "CurrentState"=w4536:string, "OutputCluster"=w4543:T2, "OutputCluster.SystemParameters.SoftwareFeatures.DataLoggingEnable"=w4533:bool)
        n1056 = case shown="\"SoftwareExit\"" w4536 {
          tunnel: w4540 -> [w4549 w4552 w4578]
          tunnel: w4538 -> [w4547 w4551 w4572]
          tunnel: w4543 -> [_ _ w4568]
          tunnel: [w4549 w4552 w4570] -> w4539
          tunnel: w4542 -> [_ w4556 w4569]
          tunnel: ["" ("State(s) in Front (\"\")") w4553 w4567] -> w4541
          tunnel: [w4547 w4551 w4564] -> w4537
          tunnel: w4535 -> [w4546 w4550 w4563]
          tunnel: [w4546 w4550 w4562] -> w4534
          tunnel: w4533 -> [_ _ w4557]
          frame Default {
          }
          frame "SoftwareExit" {
            n1057 = Select(t="HomeReached", s=w4556, f="MoveToHomePosition") -> (s? t:f=w4553:string)
          }
          frame "Stop", "TotalFinish" {
            n1058 = case shown="True" w4557 {
              tunnel: w4578 -> [w4579 w4589]
              tunnel: [w4579 w4584] -> w4573
              tunnel: w4572 -> [w4580 w4583]
              tunnel: w4568 -> [_ w4582]
              tunnel: [w4580 w4581] -> w4566
              frame False {
                # "DL Disable"
              }
              frame True {
                # "DL Enable"
                n1059 = Bundle By Name(cluster=w4582, "StateMsgToDL"="Post" ("StateMessageToMI")) -> (w4587:T2)
                n1060 = call "Output_SM.vi"("SM Private Data in"=w4583, "Output Cluster"=w4587, "Receiver Name"="DL", "State"="DL: StateMessage", "error in (no error)"=w4589) -> ("SM Private Data out"=w4581:refnum<class "Inspection Statemachine.lvclass">, "error out"=w4584:errorcluster)  [unwired: 9 in]
              }
            }
            n1061 = Bundle By Name(cluster=w4568, "StateMsgToRC"="Stop" ("StateMessageToMI")) -> (w4575:T2)
            n1062 = Bundle By Name(cluster=w4563, "OutputCluster.Result Cluster.ReelNumber"=u64 1, "BatchStart"=TRUE, "UpdateInPause"=FALSE, "SelComplete"=FALSE) -> (w4562:T1)
            n1063 = call "Output_SM.vi"("SM Private Data in"=w4566, "Output Cluster"=w4575, "Receiver Name"="RC", "State"="RC: StateMessage", "error in (no error)"=w4573) -> ("SM Private Data out"=w4565:refnum<class "Inspection Statemachine.lvclass">, "error out"=w4571:errorcluster)  [unwired: 9 in]
            n1064 = case shown="True" w4569 {
              tunnel: w4571 -> [w4590 w4594]
              tunnel: ["MoveToHomePosition" ("State(s) in Front (\"\")") "HomeReached" ("State(s) in Front (\"\")")] -> w4567
              tunnel: [w4590 w4594] -> w4570
              tunnel: w4568 -> [_ _]
              tunnel: w4565 -> [w4591 w4593]
              tunnel: [w4591 w4593] -> w4564
              frame False {
                # "Online execution"
              }
              frame True {
                # "Offline execution"
              }
            }
          }
        }
        n1065 = call <vilib>:"Add State(s) to Queue__JKI_lib_State_Machine.vi"("State(s) in Front (\"\")"=w4541, "State(s) in (\"\")"=w4544) -> ("States Out"=w4545:string)  [unwired: 13 in]
      }
      frame "MoveToHomePosition" {
        n1066 = Unbundle By Name(w4599) -> ("OutputCluster.SystemParameters.SoftwareFeatures.AutomaticGuideMovement"=w4596:bool, "OutputCluster"=w4603:T2)
        n1067 = case shown="True" w4596 {
          tunnel: w4601 -> [w4617 w4625]
          tunnel: w4598 -> [w4616 w4623]
          tunnel: w4603 -> [w4610 _]
          tunnel: [w4613 w4625] -> w4600
          tunnel: ["Wait" ("State(s) in Front (\"\")") "HomeReached" ("State(s) in Front (\"\")")] -> w4602
          tunnel: [w4611 w4623] -> w4597
          frame True {
            # "Automatic guide movement enabled"
            n1068 = Bundle By Name(cluster=w4610, "PopupInput.Pop-up Type"=T8."Open Loading Bar" ("LoadingBarInput.Pop-up Type"), "PopupInput.Message"="Moving guides...Please wait..." ("Loading Bar Display")) -> (w4620:T2)
            n1069 = call "Output_SM.vi"("SM Private Data in"=w4616, "Output Cluster"=w4620, "Receiver Name"="UI", "State"="UI: DisplayPopup", "error in (no error)"=w4617) -> ("SM Private Data out"=w4612:refnum<class "Inspection Statemachine.lvclass">, "error out"=w4614:errorcluster)  [unwired: 9 in]
            n1070 = Bundle By Name(cluster=w4610, "StateMsgToMI"="MoveMotorToHomePosition") -> (w4609:T2)
            n1071 = call "Output_SM.vi"("SM Private Data in"=w4612, "Output Cluster"=w4609, "Receiver Name"="MI", "State"="MI: StateMessage", "error in (no error)"=w4614) -> ("SM Private Data out"=w4611:refnum<class "Inspection Statemachine.lvclass">, "error out"=w4613:errorcluster)  [unwired: 9 in]
          }
          frame False {
            # "Automatic guide movement disabled"
          }
        }
        n1072 = call <vilib>:"Add State(s) to Queue__JKI_lib_State_Machine.vi"("State(s) in Front (\"\")"=w4602, "State(s) in (\"\")"=w4604) -> ("States Out"=w4605:string)  [unwired: 13 in]
      }
      frame "BuzzerOff" {
        n1073 = Unbundle By Name(w4629) -> ("OutputCluster"=w4628:T2)
        n1074 = Bundle By Name(cluster=w4628, "StateMsgToUI"="BuzzerOff") -> (w4633:T2)
        n1075 = call "Output_SM.vi"("SM Private Data in"=w4627, "Output Cluster"=w4633, "Receiver Name"="UI", "State"="UI: StateMessage", "error in (no error)"=w4630) -> ("SM Private Data out"=w4626:refnum<class "Inspection Statemachine.lvclass">, "error out"=w4631:errorcluster)  [unwired: 9 in]
        n1076 = call <vilib>:"Add State(s) to Queue__JKI_lib_State_Machine.vi"("State(s) in Front (\"\")"="Wait" ("State(s) in Front (\"\")"), "State(s) in (\"\")"=w4636) -> ("States Out"=w4638:string)  [unwired: 13 in]
      }
      frame "HomeReached" {
        n1077 = Unbundle By Name(w4645) -> ("OutputCluster.SystemParameters.SoftwareFeatures.DataLoggingEnable"=w4639:bool, "Exit"=w4647:bool, "OutputCluster.SystemParameters.SoftwareFeatures.HardwareEmulated"=w4648:bool, "CurrentState"=w4650:string, "OutputCluster"=w4649:T2)
        n1078 = case shown="\"SoftwareExit\"" w4650 {
          tunnel: w4649 -> [_ w4668 w4686 w4701 w4784]
          tunnel: w4641 -> [w4653 w4669 w4687 w4695 w4775]
          tunnel: w4643 -> [w4656 w4670 w4688 w4706 w4783]
          tunnel: w4648 -> [_ _ _ w4705 _]
          tunnel: w4647 -> [_ _ _ w4704 _]
          tunnel: ["" "Select" "" w4702 "Wait"] -> w4646
          tunnel: [w4656 w4661 w4676 w4700 w4780] -> w4642
          tunnel: w4645 -> [w4654 w4658 w4675 w4699 w4779]
          tunnel: [w4654 w4658 w4675 w4698 w4779] -> w4644
          tunnel: [w4653 w4659 w4677 w4696 w4776] -> w4640
          tunnel: w4639 -> [_ _ _ w4693 _]
          frame Default {
          }
          frame "MasterSamplePOST" {
            n1079 = Bundle By Name(cluster=w4668, "StateMsgToUI"="DisplayInspectionPage>>Reset") -> (w4673:T2)
            n1080 = call "Output_SM.vi"("SM Private Data in"=w4669, "Output Cluster"=w4673, "Receiver Name"="UI", "State"="UI: StateMessage", "error in (no error)"=w4670) -> ("SM Private Data out"=w4660:refnum<class "Inspection Statemachine.lvclass">, "error out"=w4662:errorcluster)  [unwired: 9 in]
            n1081 = Unbundle By Name(w4658) -> ("OutputCluster"=w4657:T2)
            n1082 = Bundle By Name(cluster=w4657, "PopupInput.Pop-up Type"=T8."Close Loading Bar" ("LoadingBarInput.Pop-up Type")) -> (w4666:T2)
            n1083 = call "Output_SM.vi"("SM Private Data in"=w4660, "Output Cluster"=w4666, "Receiver Name"="UI", "State"="UI: DisplayPopup", "error in (no error)"=w4662) -> ("SM Private Data out"=w4659:refnum<class "Inspection Statemachine.lvclass">, "error out"=w4661:errorcluster)  [unwired: 9 in]
          }
          frame "MasterSampleDiagnostics" {
            n1084 = Bundle By Name(cluster=w4686, "StateMsgToUI"="DisplayDiagnosticsPage") -> (w4691:T2)
            n1085 = call "Output_SM.vi"("SM Private Data in"=w4687, "Output Cluster"=w4691, "Receiver Name"="UI", "State"="UI: StateMessage", "error in (no error)"=w4688) -> ("SM Private Data out"=w4678:refnum<class "Inspection Statemachine.lvclass">, "error out"=w4679:errorcluster)  [unwired: 9 in]
            n1086 = Unbundle By Name(w4675) -> ("OutputCluster"=w4680:T2)
            n1087 = Bundle By Name(cluster=w4680, "PopupInput.Pop-up Type"=T8."Close Loading Bar" ("LoadingBarInput.Pop-up Type")) -> (w4684:T2)
            n1088 = call "Output_SM.vi"("SM Private Data in"=w4678, "Output Cluster"=w4684, "Receiver Name"="UI", "State"="UI: DisplayPopup", "error in (no error)"=w4679) -> ("SM Private Data out"=w4677:refnum<class "Inspection Statemachine.lvclass">, "error out"=w4676:errorcluster)  [unwired: 9 in]
          }
          frame "SoftwareExit" {
            n1089 = Bundle By Name(cluster=w4701, "PopupInput.Pop-up Type"=T8."Close Loading Bar" ("LoadingBarInput.Pop-up Type")) -> (w4709:T2)
            n1090 = call "Output_SM.vi"("SM Private Data in"=w4695, "Output Cluster"=w4709, "Receiver Name"="UI", "State"="UI: DisplayPopup", "error in (no error)"=w4706) -> ("SM Private Data out"=w4694:refnum<class "Inspection Statemachine.lvclass">, "error out"=w4703:errorcluster)  [unwired: 9 in]
            n1091 = case shown="False" w4704 {
              tunnel: w4705 -> [w4718 w4760]
              tunnel: w4703 -> [w4721 w4757]
              tunnel: w4694 -> [w4714 w4758]
              tunnel: [w4716 w4759] -> w4702
              tunnel: w4701 -> [w4717 w4756]
              tunnel: [w4719 w4755] -> w4700
              tunnel: w4699 -> [w4710 w4754]
              tunnel: [w4711 w4754] -> w4698
              tunnel: [w4715 w4753] -> w4696
              tunnel: w4693 -> [w4712 _]
              frame False {
                # "SaveAck not received yet"
                n1092 = case shown="True" w4712 {
                  tunnel: w4721 -> [w4725 w4736]
                  tunnel: [w4725 w4734] -> w4720
                  tunnel: w4717 -> [_ w4733]
                  tunnel: w4714 -> [w4726 w4731]
                  tunnel: [w4726 w4730] -> w4713
                  tunnel: [w4723 w4728] -> w4711
                  tunnel: w4710 -> [w4724 w4727]
                  frame False {
                    # "DL Disabled"
                    n1093 = Bundle By Name(cluster=w4724, "Exit"=TRUE ("LoadingBarActive")) -> (w4723:T1)
                  }
                  frame True {
                    # "DL Enabled"
                    n1094 = Bundle By Name(cluster=w4727, "LoadingBarActive"=TRUE) -> (w4728:T1)
                    n1095 = Bundle By Name(cluster=w4733, "PopupInput.Pop-up Type"=T8."Open Loading Bar" ("LoadingBarInput.Pop-up Type"), "PopupInput.Title"="Saving Data..." ("LoadingBarInput.LoadingString")) -> (w4739:T2)
                    n1096 = call "Output_SM.vi"("SM Private Data in"=w4731, "Output Cluster"=w4739, "Receiver Name"="UI", "State"="UI: DisplayPopup", "error in (no error)"=w4736) -> ("SM Private Data out"=w4730:refnum<class "Inspection Statemachine.lvclass">, "error out"=w4734:errorcluster)  [unwired: 9 in]
                  }
                }
                n1097 = case shown="False" w4718 {
                  tunnel: ["Wait" "Wait"] -> w4716
                  tunnel: w4713 -> [w4746 w4750]
                  tunnel: w4720 -> [w4745 w4751]
                  tunnel: w4717 -> [w4744 _]
                  tunnel: [w4742 w4751] -> w4719
                  tunnel: [w4740 w4750] -> w4715
                  frame False {
                    # "Online"
                    n1098 = Bundle By Name(cluster=w4744, "StateMsgToMI"="Shutdown") -> (w4749:T2)
                    n1099 = call "Output_SM.vi"("SM Private Data in"=w4746, "Output Cluster"=w4749, "Receiver Name"="MI", "State"="MI: StateMessage", "error in (no error)"=w4745) -> ("SM Private Data out"=w4740:refnum<class "Inspection Statemachine.lvclass">, "error out"=w4742:errorcluster)  [unwired: 9 in]
                  }
                  frame True {
                    # "Offline"
                  }
                }
              }
              frame True {
                # "SaveAck received"
                n1100 = case shown="False" w4760 {
                  tunnel: ["Wait" "ExitApplication"] -> w4759
                  tunnel: w4758 -> [w4767 w4771]
                  tunnel: w4757 -> [w4766 w4772]
                  tunnel: w4756 -> [w4765 _]
                  tunnel: [w4763 w4772] -> w4755
                  tunnel: [w4761 w4771] -> w4753
                  frame False {
                    # "Online"
                    n1101 = Bundle By Name(cluster=w4765, "StateMsgToMI"="Shutdown") -> (w4770:T2)
                    n1102 = call "Output_SM.vi"("SM Private Data in"=w4767, "Output Cluster"=w4770, "Receiver Name"="MI", "State"="MI: StateMessage", "error in (no error)"=w4766) -> ("SM Private Data out"=w4761:refnum<class "Inspection Statemachine.lvclass">, "error out"=w4763:errorcluster)  [unwired: 9 in]
                  }
                  frame True {
                    # "Offline"
                  }
                }
              }
            }
          }
          frame "Stop", "TotalFinish" {
            n1103 = Bundle By Name(cluster=w4784, "StateMsgToUI"="Stop") -> (w4790:T2)
            n1104 = call "Output_SM.vi"("SM Private Data in"=w4775, "Output Cluster"=w4790, "Receiver Name"="UI", "State"="UI: StateMessage", "error in (no error)"=w4783) -> ("SM Private Data out"=w4774:refnum<class "Inspection Statemachine.lvclass">, "error out"=w4782:errorcluster)  [unwired: 9 in]
            n1105 = Bundle By Name(cluster=w4784, "PopupInput.Pop-up Type"=T8."Close Loading Bar" ("LoadingBarInput.Pop-up Type")) -> (w4787:T2)
            n1106 = call "Output_SM.vi"("SM Private Data in"=w4774, "Output Cluster"=w4787, "Receiver Name"="UI", "State"="UI: DisplayPopup", "error in (no error)"=w4782) -> ("SM Private Data out"=w4776:refnum<class "Inspection Statemachine.lvclass">, "error out"=w4780:errorcluster)  [unwired: 9 in]
          }
        }
        n1107 = call <vilib>:"Add State(s) to Queue__JKI_lib_State_Machine.vi"("State(s) in Front (\"\")"=w4646, "State(s) in (\"\")"=w4651) -> ("States Out"=w4652:string)  [unwired: 13 in]
      }
      frame "---------- Software Exit State ----------" {
        # "Do not put any code in this frame.\n(It is a separator no-op. You can make a copy of this frame to create a new UI frame)"
        n1108 = call <vilib>:"Add State(s) to Queue__JKI_lib_State_Machine.vi"("State(s) in (\"\")"=w4795) -> ("States Out"=w4794:string)  [unwired: 14 in]
      }
      frame "SoftwareExit" {
        n1109 = Flush Event Queue(0:w4818, 3:w4804) -> (11:w4814:errorcluster)  [unwired: 4 in, 2 out]
        n1110 = Unbundle By Name(w4806) -> ("OutputCluster.SystemParameters.SoftwareFeatures.DataLoggingEnable"=w4797:bool, "OutputCluster.SystemParameters.SoftwareFeatures.AutomaticGuideMovement"=w4807:bool, "DirectExit"=w4808:bool, "OutputCluster.SystemParameters.SoftwareFeatures.HardwareEmulated"=w4811:bool, "OutputCluster"=w4798:T2)
        n1111 = Bundle By Name(cluster=w4798, "StateMsgToRC"="Stop") -> (w4817:T2)
        n1112 = call "Output_SM.vi"("SM Private Data in"=w4799, "Output Cluster"=w4817, "Receiver Name"="RC", "State"="RC: StateMessage", "error in (no error)"=w4814) -> ("SM Private Data out"=w4800:refnum<class "Inspection Statemachine.lvclass">, "error out"=w4812:errorcluster)  [unwired: 9 in]
        n1113 = case shown="True" w4797 {
          tunnel: w4812 -> [w4821 w4825]
          tunnel: [w4821 w4842] -> w4810
          tunnel: [w4822 w4841] -> w4801
          tunnel: w4800 -> [w4822 w4826]
          tunnel: w4798 -> [_ w4823]
          frame False {
            # "DL Disable"
          }
          frame True {
            # "DL Enable"
            n1114 = Bundle By Name(cluster=w4823, "MachineStatusToDL"="SoftwareExit" ("StateMsgToDL")) -> (w4829:T2)
            n1115 = call "Output_SM.vi"("SM Private Data in"=w4826, "Output Cluster"=w4829, "Receiver Name"="DL", "State"="DL: MachineStatus", "error in (no error)"=w4825) -> ("SM Private Data out"=w4827:refnum<class "Inspection Statemachine.lvclass">, "error out"=w4824:errorcluster)  [unwired: 9 in]
            n1116 = Bundle By Name(cluster=w4823, "StateMsgToDL"="StopPost" ("StateMsgToRC")) -> (w4850:T2)
            n1117 = call "Output_SM.vi"("SM Private Data in"=w4827, "Output Cluster"=w4850, "Receiver Name"="DL", "State"="DL: StateMessage", "error in (no error)"=w4824) -> ("SM Private Data out"=w4832:refnum<class "Inspection Statemachine.lvclass">, "error out"=w4835:errorcluster)  [unwired: 9 in]
            n1118 = Bundle By Name(cluster=w4823, "EventData.EventName"="Exit" ("DataLogger.EventDetails.EventName"), "EventData.EventReason"="Software Exit" ("DataLogger.EventDetails.EventReason")) -> (w4838:T2)
            n1119 = call "Output_SM.vi"("SM Private Data in"=w4832, "Output Cluster"=w4838, "Receiver Name"="DL", "State"="DL: EventDetails", "error in (no error)"=w4835) -> ("SM Private Data out"=w4833:refnum<class "Inspection Statemachine.lvclass">, "error out"=w4834:errorcluster)  [unwired: 9 in]
            n1120 = Bundle By Name(cluster=w4823, "StateMsgToDL"="Save" ("StateMsgToRC")) -> (w4846:T2)
            n1121 = call "Output_SM.vi"("SM Private Data in"=w4833, "Output Cluster"=w4846, "Receiver Name"="DL", "State"="DL: StateMessage", "error in (no error)"=w4834) -> ("SM Private Data out"=w4841:refnum<class "Inspection Statemachine.lvclass">, "error out"=w4842:errorcluster)  [unwired: 9 in]
          }
        }
        n1122 = case shown="False" w4811 {
          tunnel: w4810 -> [w4857 w5029]
          tunnel: w4798 -> [w4861 w5026]
          tunnel: w4806 -> [w4860 w5027]
          tunnel: [w4859 w5017] -> w4805
          tunnel: w4801 -> [w4862 w5021]
          tunnel: [w4858 w5016] -> w4809
          tunnel: [w4856 w5022] -> w4803
          tunnel: w4808 -> [w4854 _]
          tunnel: w4807 -> [w4855 _]
          tunnel: [w4853 w5019] -> w4802
          tunnel: w4797 -> [w4852 w5015]
          tunnel: w4796 -> [w4851 _]
          frame False {
            # "Online"
            n1123 = case shown="False" w4854 {
              tunnel: w4862 -> [w4866 w4988]
              tunnel: w4861 -> [w4868 w4980]
              tunnel: w4860 -> [w4870 w4990]
              tunnel: [w4869 w4982] -> w4859
              tunnel: [w4867 w4981] -> w4858
              tunnel: w4857 -> [w4878 w4989]
              tunnel: [w4872 w4987] -> w4856
              tunnel: w4855 -> [w4873 _]
              tunnel: [w4864 w4986] -> w4853
              tunnel: w4852 -> [_ w4979]
              tunnel: w4851 -> [w4863 _]
              frame False {
                # "No direct exit"
                n1124 = Bundle By Name(cluster=w4868, "StateMsgToMI"="SoftwareExit") -> (w4881:T2)
                n1125 = Unbundle By Name(w4868) -> ("PartInfo.PartName"=w4876:string)
                n1126 = call "Output_SM.vi"("SM Private Data in"=w4866, "Output Cluster"=w4881, "Receiver Name"="MI", "State"="MI: StateMessage", "error in (no error)"=w4878) -> ("SM Private Data out"=w4865:refnum<class "Inspection Statemachine.lvclass">, "error out"=w4871:errorcluster)  [unwired: 9 in]
                n1127 = Not Equal?(x=w4876, y="") -> (x != y?=w4874:bool)
                n1128 = case shown="False" w4874 {
                  tunnel: w4873 -> [_ w4916]
                  tunnel: [w4887 w4918] -> w4872
                  tunnel: w4871 -> [w4888 w4917]
                  tunnel: w4870 -> [w4891 w4913]
                  tunnel: [w4890 w4912] -> w4869
                  tunnel: w4868 -> [w4884 w4915]
                  tunnel: w4865 -> [w4885 w4914]
                  tunnel: [w4882 ""] -> w4867
                  tunnel: [w4886 w4909] -> w4864
                  tunnel: w4863 -> [w4883 w4908]
                  frame False {
                    # "Part not selected"
                    n1129 = case shown="\"MasterSample\"" w4883 {
                      tunnel: w4888 -> [w4896 w4905]
                      tunnel: w4884 -> [w4894 _]
                      tunnel: w4885 -> [w4895 w4906]
                      tunnel: [w4898 w4905] -> w4887
                      tunnel: [w4897 w4906] -> w4886
                      tunnel: ["" "HomeReached"] -> w4882
                      frame "MasterSample" {
                        # "Software Exit due to master sample"
                        n1130 = Bundle By Name(cluster=w4894, "PopupInput.Title"="MESSAGE" ("Dialog Box Input"), "PopupInput.Message"="Software is exiting for Master Sample validation" ("Message Input"), "PopupInput.Button 1 Text"="Exit Application" ("Boolean Text.Text"), "PopupInput.Pop-up Type"=T8."One button dialog box") -> (w4903:T2)
                        n1131 = call "Output_SM.vi"("SM Private Data in"=w4895, "Output Cluster"=w4903, "Receiver Name"="UI", "State"="UI: DisplayPopup", "error in (no error)"=w4896) -> ("SM Private Data out"=w4897:refnum<class "Inspection Statemachine.lvclass">, "error out"=w4898:errorcluster)  [unwired: 9 in]
                      }
                      frame Default {
                        # "Software Exit due to button press"
                      }
                    }
                    n1132 = Bundle By Name(cluster=w4891, "CurrentState"="SoftwareExit") -> (w4890:T1)
                  }
                  frame True {
                    # "Part selected"
                    n1133 = case shown="True" w4916 {
                      tunnel: [w4921 w4951] -> w4918
                      tunnel: w4917 -> [w4924 w4954]
                      tunnel: w4915 -> [w4923 w4953]
                      tunnel: w4914 -> [w4922 w4952]
                      tunnel: [w4920 w4950] -> w4909
                      tunnel: w4908 -> [w4919 w4949]
                      frame False {
                        # "Automatic guide movement disabled"
                        n1134 = case shown="\"MasterSample\"" w4919 {
                          tunnel: w4924 -> [w4927 w4942]
                          tunnel: w4923 -> [w4925 w4941]
                          tunnel: w4922 -> [w4926 w4940]
                          tunnel: [w4929 w4939] -> w4921
                          tunnel: [w4928 w4937] -> w4920
                          frame "MasterSample" {
                            # "Software Exit due to master sample"
                            n1135 = Bundle By Name(cluster=w4925, "PopupInput.Title"="MESSAGE" ("Dialog Box Input"), "PopupInput.Message"="Software is exiting for Master Sample validation.\nPlease remove the terminals." ("Message Input"), "PopupInput.Button 1 Text"="Continue" ("Boolean Text.Text"), "PopupInput.Pop-up Type"=T8."One button dialog box") -> (w4935:T2)
                            n1136 = call "Output_SM.vi"("SM Private Data in"=w4926, "Output Cluster"=w4935, "Receiver Name"="UI", "State"="UI: DisplayPopup", "error in (no error)"=w4927) -> ("SM Private Data out"=w4928:refnum<class "Inspection Statemachine.lvclass">, "error out"=w4929:errorcluster)  [unwired: 9 in]
                          }
                          frame Default {
                            # "Software Exit due to button press"
                            n1137 = Bundle By Name(cluster=w4941, "PopupInput.Title"="MESSAGE" ("Dialog Box Input"), "PopupInput.Message"="Please remove the terminals" ("Message Input"), "PopupInput.Button 1 Text"="Continue" ("Boolean Text.Text"), "PopupInput.Pop-up Type"=T8."One button dialog box") -> (w4947:T2)
                            n1138 = call "Output_SM.vi"("SM Private Data in"=w4940, "Output Cluster"=w4947, "Receiver Name"="UI", "State"="UI: DisplayPopup", "error in (no error)"=w4942) -> ("SM Private Data out"=w4937:refnum<class "Inspection Statemachine.lvclass">, "error out"=w4939:errorcluster)  [unwired: 9 in]
                          }
                        }
                      }
                      frame True {
                        # "Automatic guide movement enabled"
                        n1139 = case shown="\"MasterSample\"" w4949 {
                          tunnel: w4954 -> [w4957 w4972]
                          tunnel: w4953 -> [w4955 w4971]
                          tunnel: w4952 -> [w4956 w4970]
                          tunnel: [w4959 w4969] -> w4951
                          tunnel: [w4958 w4967] -> w4950
                          frame "MasterSample" {
                            # "Software Exit due to master sample"
                            n1140 = Bundle By Name(cluster=w4955, "PopupInput.Title"="MESSAGE" ("Dialog Box Input"), "PopupInput.Message"="Software is exiting for Master Sample validation.\nPlease remove the terminals before guides are opened." ("Message Input"), "PopupInput.Button 1 Text"="Continue" ("Boolean Text.Text"), "PopupInput.Pop-up Type"=T8."One button dialog box") -> (w4965:T2)
                            n1141 = call "Output_SM.vi"("SM Private Data in"=w4956, "Output Cluster"=w4965, "Receiver Name"="UI", "State"="UI: DisplayPopup", "error in (no error)"=w4957) -> ("SM Private Data out"=w4958:refnum<class "Inspection Statemachine.lvclass">, "error out"=w4959:errorcluster)  [unwired: 9 in]
                          }
                          frame Default {
                            # "Software Exit due to button press"
                            n1142 = Bundle By Name(cluster=w4971, "PopupInput.Title"="MESSAGE" ("Dialog Box Input"), "PopupInput.Message"="Please remove the terminals before guides are opened" ("Message Input"), "PopupInput.Button 1 Text"="Continue" ("Boolean Text.Text"), "PopupInput.Pop-up Type"=T8."One button dialog box") -> (w4977:T2)
                            n1143 = call "Output_SM.vi"("SM Private Data in"=w4970, "Output Cluster"=w4977, "Receiver Name"="UI", "State"="UI: DisplayPopup", "error in (no error)"=w4972) -> ("SM Private Data out"=w4967:refnum<class "Inspection Statemachine.lvclass">, "error out"=w4969:errorcluster)  [unwired: 9 in]
                          }
                        }
                      }
                    }
                    n1144 = Bundle By Name(cluster=w4913, "CurrentState"="SoftwareExit") -> (w4912:T1)
                  }
                }
              }
              frame True {
                w4992 = TRUE ("LoadingBarActive")
                # "Direct Exit without communication with hardware"
                n1145 = Bundle By Name(cluster=w4980, "StateMsgToUI"="DisableAllButtons") -> (w4996:T2)
                n1146 = Bundle By Name(cluster=w4990, "LoadingBarActive"=w4992, "Exit"=w4992, "CurrentState"="SoftwareExit") -> (w4983:T1)
                n1147 = call "Output_SM.vi"("SM Private Data in"=w4988, "Output Cluster"=w4996, "Receiver Name"="UI", "State"="UI: StateMessage", "error in (no error)"=w4989) -> ("SM Private Data out"=w4985:refnum<class "Inspection Statemachine.lvclass">, "error out"=w4984:errorcluster)  [unwired: 9 in]
                n1148 = case shown="True" w4979 {
                  tunnel: w4980 -> [_ w5010]
                  tunnel: w4984 -> [w4998 w5009]
                  tunnel: [w4998 w5008] -> w4987
                  tunnel: w4985 -> [w4999 w5006]
                  tunnel: [w4999 w5005] -> w4986
                  tunnel: w4983 -> [w5000 w5003]
                  tunnel: [w5000 w5001] -> w4982
                  tunnel: ["ExitApplication" ""] -> w4981
                  frame False {
                    # "DL Disable"
                  }
                  frame True {
                    w5004 = TRUE ("LoadingBarActive")
                    # "DL Enable"
                    n1149 = Bundle By Name(cluster=w5003, "LoadingBarActive"=w5004, "Exit"=w5004) -> (w5001:T1)
                    n1150 = Bundle By Name(cluster=w5010, "PopupInput.Pop-up Type"=T8."Open Loading Bar" ("LoadingBarInput.Pop-up Type"), "PopupInput.Message"="Saving Data..." ("LoadingBarInput.LoadingString")) -> (w5014:T2)
                    n1151 = call "Output_SM.vi"("SM Private Data in"=w5006, "Output Cluster"=w5014, "Receiver Name"="UI", "State"="UI: DisplayPopup", "error in (no error)"=w5009) -> ("SM Private Data out"=w5005:refnum<class "Inspection Statemachine.lvclass">, "error out"=w5008:errorcluster)  [unwired: 9 in]
                  }
                }
              }
            }
          }
          frame True {
            w5024 = TRUE ("LoadingBarActive")
            # "Offline"
            n1152 = Bundle By Name(cluster=w5026, "StateMsgToUI"="DisableAllButtons") -> (w5032:T2)
            n1153 = Bundle By Name(cluster=w5027, "LoadingBarActive"=w5024, "Exit"=w5024, "CurrentState"="SoftwareExit") -> (w5018:T1)
            n1154 = call "Output_SM.vi"("SM Private Data in"=w5021, "Output Cluster"=w5032, "Receiver Name"="UI", "State"="UI: StateMessage", "error in (no error)"=w5029) -> ("SM Private Data out"=w5020:refnum<class "Inspection Statemachine.lvclass">, "error out"=w5025:errorcluster)  [unwired: 9 in]
            n1155 = case shown="True" w5015 {
              tunnel: w5026 -> [_ w5046]
              tunnel: w5025 -> [w5034 w5045]
              tunnel: [w5034 w5044] -> w5022
              tunnel: w5020 -> [w5035 w5042]
              tunnel: [w5035 w5041] -> w5019
              tunnel: w5018 -> [w5036 w5039]
              tunnel: [w5036 w5037] -> w5017
              tunnel: ["ExitApplication" ""] -> w5016
              frame False {
                # "DL Disable"
              }
              frame True {
                w5040 = TRUE ("LoadingBarActive")
                # "DL Enable"
                n1156 = Bundle By Name(cluster=w5039, "LoadingBarActive"=w5040, "Exit"=w5040) -> (w5037:T1)
                n1157 = Bundle By Name(cluster=w5046, "PopupInput.Pop-up Type"=T8."Open Loading Bar" ("LoadingBarInput.Pop-up Type"), "PopupInput.Message"="Saving Data..." ("LoadingBarInput.LoadingString")) -> (w5050:T2)
                n1158 = call "Output_SM.vi"("SM Private Data in"=w5042, "Output Cluster"=w5050, "Receiver Name"="UI", "State"="UI: DisplayPopup", "error in (no error)"=w5045) -> ("SM Private Data out"=w5041:refnum<class "Inspection Statemachine.lvclass">, "error out"=w5044:errorcluster)  [unwired: 9 in]
              }
            }
          }
        }
        n1159 = call <vilib>:"Add State(s) to Queue__JKI_lib_State_Machine.vi"("State(s) in Front (\"\")"=w4809, "State(s) in (\"\")"=w4820) -> ("States Out"=w4819:string)  [unwired: 13 in]
      }
      frame "ExitApplication" {
        n1160 = Unbundle By Name(w5072) -> ("OutputCluster.SystemParameters.NumberOfRacks"=w5067:u8, "OutputCluster.SystemParameters.SoftwareFeatures.AnalyticsEnable"=w5070:bool, "OutputCluster.SystemParameters.SoftwareFeatures.HardwareEmulated"=w5073:bool, "OutputCluster.SystemParameters.SoftwareFeatures.DataLoggingEnable"=w5057:bool)
        n1161 = Unbundle By Name(w5056) -> ("Analytics Actor Enqueuer"=w5060:refnum<class "Message Enqueuer.lvclass">, "Data Logger Actor Enqueuer"=w5062:refnum<class "Message Enqueuer.lvclass">, "User Interface Actor Enqueuer"=w5064:refnum<class "Message Enqueuer.lvclass">, "Rack Controller Actor Enqueuer"=w5066:refnum<class "Message Enqueuer.lvclass">[], "Machine Interface Actor Enqueuer"=w5069:refnum<class "Message Enqueuer.lvclass">)
        n1162 = case shown="False" w5073 {
          tunnel: w5071 -> [w5089 w5090]
          tunnel: [w5088 w5090] -> w5068
          tunnel: w5069 -> [w5087 _]
          frame False {
            # "Online Execution"
            n1163 = call <vilib>:"Send Normal Stop.vi"("error in (no error)"=w5089, "Message Enqueuer"=w5087) -> ("error out"=w5088:errorcluster)  [unwired: 9 in]
          }
          frame True {
            # "Offline Execution"
          }
        }
        n1164 = for {
          N: w5067 -> [_]
          tunnel: w5068 -> [w5082]
          tunnel: w5066 -> [w5081] mode=indexing
          tunnel: [w5080] -> w5065
          n1165 = call <vilib>:"Send Normal Stop.vi"("error in (no error)"=w5082, "Message Enqueuer"=w5081) -> ("error out"=w5080:errorcluster)  [unwired: 9 in]
        }
        n1166 = call <vilib>:"Send Normal Stop.vi"("error in (no error)"=w5065, "Message Enqueuer"=w5064) -> ("error out"=w5063:errorcluster)  [unwired: 9 in]
        n1167 = case shown="False" w5057 {
          tunnel: w5063 -> [w5076 w5079]
          tunnel: w5062 -> [_ w5078]
          tunnel: [w5076 w5077] -> w5061
          frame False {
            # "DL Disable"
          }
          frame True {
            # "DL Enable"
            n1168 = call <vilib>:"Send Normal Stop.vi"("error in (no error)"=w5079, "Message Enqueuer"=w5078) -> ("error out"=w5077:errorcluster)  [unwired: 9 in]
          }
        }
        n1169 = call <vilib>:"Add State(s) to Queue__JKI_lib_State_Machine.vi"("State(s) in (\"\")"=w5074) -> ("States Out"=w5075:string)  [unwired: 14 in]
        n1170 = case shown="True" w5070 {
          tunnel: w5061 -> [w5083 w5086]
          tunnel: [w5083 w5085] -> w5054
          tunnel: w5060 -> [_ w5084]
          frame False {
            # "Analytics disabled"
          }
          frame True {
            # "Analytics Enabled"
            n1171 = call <vilib>:"Send Normal Stop.vi"("error in (no error)"=w5086, "Message Enqueuer"=w5084) -> ("error out"=w5085:errorcluster)  [unwired: 9 in]
          }
        }
        n1172 = call <vilib>:"Read Self Enqueuer.vi"("Actor"=w5056) -> ("Self Enqueuer"=w5059:refnum<class "Message Enqueuer.lvclass">)  [unwired: 10 in]
        n1173 = Unbundle By Name(w5056) -> ("ExitTimeLoop"=w5055:refnum<user-event>)
        n1174 = Generate User Event(priority (normal)=usereventprio."high priority", user event=w5055, event data cluster=FALSE ("event data"), error in=w5054) -> (error out=w5053:errorcluster)  [unwired: 1 out]
        n1175 = call <vilib>:"Send Normal Stop.vi"("error in (no error)"=w5053, "Message Enqueuer"=w5059) -> ("error out"=w5058:errorcluster)  [unwired: 9 in]
      }
    }
  }
  n1176 = Merge Errors(w32, w31, w8) -> (→"error out":errorcluster)
